vi "MAIN TASK TLB V1.vi"() -> ()   [LabVIEW 2018]
uses:
  TLB Type Definitions/Intruction Type Definitions.ctl
  TLB Type Definitions/State Type Definitions, for 0.26g versions and later 3.ctl
  <vilib>/Studica/Studica Toolkit/NavX/TypeDefs/Flags/Z900_navX_Flags_OpStatusTypeDef.ctl
  <vilib>/Studica/Studica Toolkit/NavX/TypeDefs/Flags/Z900_navX_Flags_CalibrationStatusTypeDef.ctl
  TLB Type Definitions/Vision cluster.ctl
  TLB Type Definitions/PING CLUSTER.ctl
  TLB Type Definitions/Encoder cluster.ctl
  TLB Type Definitions/Stepper cluster.ctl
  TLB Type Definitions/Yaw Cluster.ctl
  TLB Type Definitions/IR Sensor Type Def.ctl
  TLB Type Definitions/Line Sensor Cluster.ctl
  TLB Type Definitions/Time cluster.ctl
  TLB Type Definitions/Box Colour Detection Cluster (0.26d and above).ctl
  Underlying VI's/FGV's/Box FGV/Box Colour FGV Colours.ctl
  <vilib>/Studica/Studica Toolkit/Background/DIO Channel.ctl
  TLB Type Definitions/Y Stepper cluster.ctl
  TLB Type Definitions/Motor Speed Cluster.ctl
  <vilib>/Studica/Studica Toolkit/Background/PWM Channel.ctl
  Underlying VI's/NavX VI/navX type def.ctl
  <vilib>/Studica/Studica Toolkit/Background/I2C Channel.ctl
  Underlying VI's/I2C Master VI/Arduino_Interfacing.ctl
  Labview Training Phase 2/Enum Controls/States for Action Engine.ctl
  Underlying VI's/Motor Control VI with PID/MOTOR CONTROL WITH PID AE DATA MODE TYPE DEF.ctl
  Underlying VI's/Motor Control VI with PID/MOTOR CONTROL WITH PID AE DIRECTION TYPE DEF.ctl
  Experimental VI's/Archived VI's/MOTOR CONTROL NO PID Type Def.ctl
  <vilib>/myRIO/Common/Instrument Driver Framework/myRIO v1.0/AI/typedefs/AI Channels List.ctl
  <vilib>/myRIO/Common/Instrument Driver Framework/myRIO v1.0/AI/typedefs/AI Channels Enum.ctl
  Underlying VI's/Line Sensor AE/Line Sensor AE Type Def.ctl
  Underlying VI's/I2C Master VI/I2C MASTER Type Def.ctl
  Underlying VI's/Elasped Timer/Elapsed timer control.ctl
  Underlying VI's/IMAQ Create Reference AE/IMAQ Reference AE.ctl
  Underlying VI's/FGV's/Box FGV/Box Colour FGV States.ctl
  Underlying VI's/I2C Master VI/I2C_MASTER_WRITE_NEW Type Def.ctl
  Underlying VI's/FGV's/Servo State FGV/Servo States FGV Enum.ctl
  Underlying VI's/Modified webcam FGV/Webcam AE.ctl
  <vilib>/userdefined/High Color/IMAQdx.ctl
  <vilib>/Studica/Studica Toolkit/NavX/NavX.lvlib
panel:
  out "Same colour?":bool
  out "Distance to move":dbl
  out "Box Colour Detection":T1
  out "Errors detected":bool
  out "Robot ready":bool
  out "Time cluster":T3
  out "Table IR obstruct":bool
  out "Front IR obstruct":bool
  out "Line sensors":T4
  out "IR Sensors":T5
  out "NAVX Values":T6
  out "Stepper position values":T7
  out "Encoder values":T8
  out "Ultrasonic sensors":T9
  out "Selected Task":T10=enum."Start Task 9"
  out "Object recognition mode":enum16{"Ball", "Soap", "Gel", "Pipe", "None"}(ring)
  out "Image Processing Error":errorcluster
  out "Object Detection":T11
  out "Status":T14 {"OP Status" items=["INITIALIZING", "SELFTEST_IN_PROGRESS", "ERROR", "IMU_AUTOCAL_IN_PROGRESS", "NORMAL"]; "Calibration Status" items=["IMU_CAL_STATE_MASK"=3, "IMU_CAL_STATE_INPROGRESS"=0, "IMU_CAL_STATE_ACCUMULATE"=1, "IMU_CAL_STATE_COMPLETE"=2]}
  out "General Errors":errorcluster
  in  "Red LED":bool
  out "Front Ultrasonic obstruct":bool
  out "Speed & distance":T15
  out "Task selection":u8
  out "NavX Readings":T16
  out "Arduino Data":T17
  out "TASK ENABLE":bool
  out "Rising Edge":bool
  in  "Green LED":bool
  out "State Logic":T18=enum."Startup"
  out "elements":T10[](array[typedef])
  in  "STOP TASK":bool
  in  "OK Button":bool
  in  "STOP":bool
  out "Queue Errors":errorcluster
  out "Action Queue Items":i32
  out "State Logic Queue Items":i32
  out "Action Queues items":string[](array[string])=["Hardware reset", "Software reset", ""]
  out "Action State":string
  # "TLB FRAMEWORK STATUS"
  # "System Health Status Update"
  # "Test Programme written by Calvin Loke    Dated: 28 Aug 2019\nTest Programme revised by Dr Alex See   Dated 30 Aug 2019\n\nRevision date: 20/03/2020\nProgramme version:   TLB Native Dynamic Events ver 0.19a"
  # "0: Task 1\n1: Task 2\n2: Task 3\n3: Task 4\n4: Task 5\n5: Task 6\n6: Task 7\n7: Task 8 Ball\n8: Task 8 Soap\n9: Task 8 Gel\n10: Task 8 Pipe\n11: Task 9 Blue\n12: Task 9 Black\n13: Task 9 Green\n14: Task 9 Red\n15: Task 9 Yellow"
  # "Ball: Right\nSoap: Left\nGel: Reverse\nPipe: Forward"
  # "VISION"
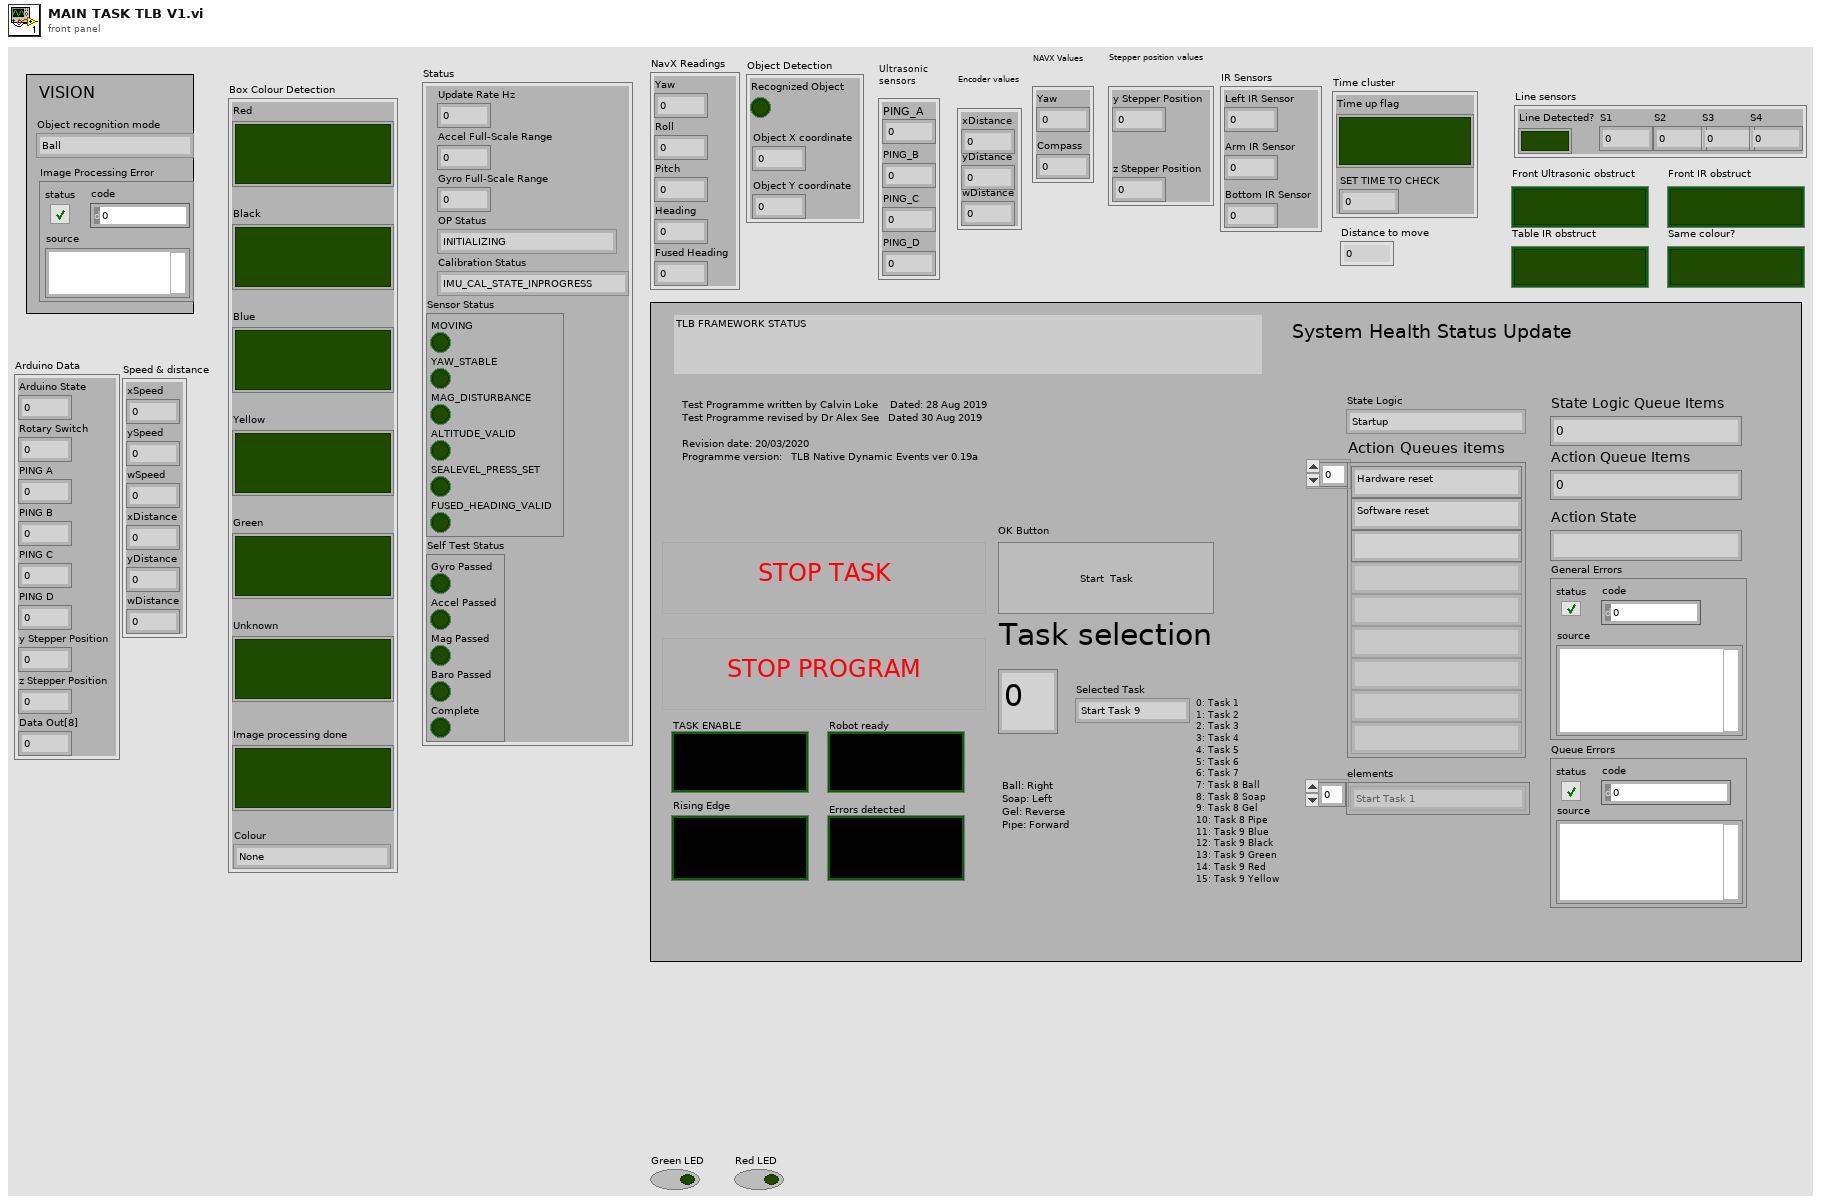
[diagram p1: front panel]
types:
  T1 = typedef "Box Colour Detection Cluster (0.26d and above).ctl" = cluster{"Red":bool, "Black":bool, "Blue":bool, "Yellow":bool, "Green":bool, "Unknown":bool, "Image processing done":bool, "Colour":T2}
  T2 = typedef "Box Colour FGV Colours.ctl" = enum16{"None", "Black", "Blue", "Green", "Red", "Yellow"}
  T3 = typedef "Time cluster.ctl" = cluster{"Time up flag":bool, "SET TIME TO CHECK":dbl}
  T4 = typedef "Line Sensor Cluster.ctl" = cluster{"Line Detected?":bool, "S1":dbl, "S2":dbl, "S3":dbl, "S4":dbl}
  T5 = typedef "IR Sensor Type Def.ctl" = cluster{"Left IR Sensor":dbl, "Arm IR Sensor":dbl, "Bottom IR Sensor":dbl}
  T6 = typedef "Yaw Cluster.ctl" = cluster{"Yaw":dbl, "Compass":dbl}
  T7 = typedef "Stepper cluster.ctl" = cluster{"y Stepper Position":u8, "z Stepper Position":u8}
  T8 = typedef "Encoder cluster.ctl" = cluster{"xDistance":dbl, "yDistance":dbl, "wDistance":dbl}
  T9 = typedef "PING CLUSTER.ctl" = cluster{"PING_A":u8, "PING_B":u8, "PING_C":u8, "PING_D":u8}
  T10 = typedef "Intruction Type Definitions.ctl" = enum16{"None", "Start Task 1", "Start Task 2", "Start Task 3", "Start Task 4", "Start Task 5", "Start Task 6", "Start Task 7", "Start Task 8 - BALL", "Start Task 8 - Gel", "Start Task 8 - Pipe", "Start Task 8 - Soap", "Start Task 9", "Start Task A", "Start Task B", "Exit"}
  T11 = typedef "Vision cluster.ctl" = cluster{"Recognized Object":bool, "Object X coordinate":dbl, "Object Y coordinate":dbl}
  T12 = typedef "NavX.lvlib/Z900_navX_Flags_OpStatusTypeDef.ctl" = u8
  T13 = typedef "NavX.lvlib/Z900_navX_Flags_CalibrationStatusTypeDef.ctl" = u8
  T14 = cluster{"Update Rate Hz":u8, "Accel Full-Scale Range":u8, "Gyro Full-Scale Range":u16, "OP Status":T12, "Calibration Status":T13, "Sensor Status":cluster{"MOVING":bool, "YAW_STABLE":bool, "MAG_DISTURBANCE":bool, "ALTITUDE_VALID":bool, "SEALEVEL_PRESS_SET":bool, "FUSED_HEADING_VALID":bool}, "Self Test Status":cluster{"Gyro Passed":bool, "Accel Passed":bool, "Mag Passed":bool, "Baro Passed":bool, "Complete":bool}}
  T15 = cluster{"xSpeed":dbl, "ySpeed":dbl, "wSpeed":dbl, "xDistance":dbl, "yDistance":dbl, "wDistance":dbl}
  T16 = cluster{"Yaw":dbl, "Roll":dbl, "Pitch":dbl, "Heading":dbl, "Fused Heading":dbl}
  T17 = cluster{"Arduino State":u8, "Rotary Switch":u8, "PING A":u8, "PING B":u8, "PING C":u8, "PING D":u8, "y Stepper Position":u8, "z Stepper Position":u8, "Data Out[8]":u8}
  T18 = typedef "State Type Definitions, for 0.26g versions and later 3.ctl" = enum16{"None", "Startup", "Move to Angle", "True Stop", "Idle", "Shutdown", "Task 1A", "Task 1B", "Task 2:Raise Arm", "Task 2:Sensor Mode", "Task 2:Reverse Mode", "Task 3: Rotate 360", "Task 4_A", "Task 4_B", "Task 4_C", "Task 4_D", "Task 5A: RAISING ARM", "Task 5B: STILL WAITING", "Task 5C: GOING DOWN", "Task 5D: GRAB", "Task 5E: GOING UP", "Task 5F: ARM GRAB HEIGHT", "Task 5G: CLOSE CLAW", "Task 5H: RAISE ARM", "Task 6A: RAISE ARM", "Task 6B: CAM BURST", "Task 6C: PROCESS IMAGE", "Task 6D: BALL BUSTER", "Task 6E: STILL WAITING", "Task 6F: CAM BURST 2", "Task 6G: PROCESS IMAGE 2", "Task 6H: SKADI SOAPS", "Task 6I: STILL WAITING 2", "Task 6J: CAM BURST 3", "Task 6K: PROCESS IMAGE 3", "Task 6L: JAM IT IN", "Task 6M: STILL WAITING 3", "Task 6N: CAM BURST 4", "Task 6O: PROCESS IMAGE 4", "Task 6P: PIPE BOMB", "Task 7", "Task 8A: RAISE ARM", "Task 8B: MOVE TO BOX", "Task 8C: CAM BURST", "Task 8D: PROCESS IMAGE", "Task 8E: ROBOT ADJUST", "Task 8F: CAM BURST 2", "Task 8G: PROCESS IMAGE 2", "Task 8H: ARM ADJUST", "Task 8I: ARM GRAB HEIGHT", "Task 8J: CLOSE CLAW", "Task 8K: RAISE MY SWORD", "Task 8I: STILL WAITING", "Task 8L: Return to position", "Task 9A: Raise Arm", "Task 9B: Rotate to Angle", "Task 9C: Detect Box", "Task 9D: MOVE FORWARD", "Task 9D2: ANGLE CORRECTION", "Task 9E: MOVE LEFT", "Task 9E2: MOVE RIGHT", "Task 9F: SCAN BOX", "Task 9G: MOVE RIGHT", "Task 9H: SCAN BOX 2", "Task 9I: ROTATE 90 CW", "Task 9J: FORWARD", "Task 9J2: ANGLE CORRECTION", "Task 9K: RAM WALL", "Task 9L: MOVE RIGHT", "Task 9M: SCAN BOX 3", "Task 9N: MOVE RIGHT", "Task 9O: SCAN BOX 4", "Task A1: RAISE ARM", "Task A2: ROTATE TO ANGLE", "Task A3: MOVE TO BL BOX", "Task A4: MOVE FORWARD", "Task A5: Stop", "Task A6: ROTATE CW 90", "Task A7: FORWARD", "Task A8: LEFT UNTIL LINE", "Task A9: REVERSE", "Task A10: ROTATE TO ANGLE", "Task A11: ARM DROP HEIGHT", "Task A12: EXTEND ARM", "Task A12: DROP"}
  T19 = typedef "PWM Channel.ctl" = enum16{"Not Connected", "A/PWM0", "A/PWM1", "A/PWM2", "A/PWM3", "A/PWM4", "B/PWM0", "B/PWM1", "B/PWM2", "B/PWM3", "B/PWM4", "C/PWM0", "C/PWM1"}
  T20 = typedef "Motor Speed Cluster.ctl" = cluster{"ySpeed":dbl, "xSpeed":dbl, "wSpeed":dbl}
  T21 = typedef "Y Stepper cluster.ctl" = cluster{"yStepper desired":u8}
  T22 = typedef "DIO Channel.ctl" = enum16{"Not Connected", "A/DIO1", "A/DIO2", "A/DIO3", "A/DIO4", "A/DIO5", "A/DIO6", "A/DIO7", "A/DIO13", "B/DIO1", "B/DIO2", "B/DIO3", "B/DIO4", "B/DIO5", "B/DIO6", "B/DIO7", "B/DIO13", "C/DIO0", "C/DIO1", "C/DIO2", "C/DIO3", "C/DIO4", "C/DIO5", "C/DIO6", "C/DIO7"}
  T23 = cluster{"PWM Channel":T19, "FPGA VI Reference Out":refnum<k20>}
  T24 = cluster{"DIO Channel":T22, "FPGA VI Reference Out":refnum<k20>}
  T25 = typedef "States for Action Engine.ctl" = enum16{"Initialize", "Write", "Read"}
  T26 = typedef "MOTOR CONTROL WITH PID AE DATA MODE TYPE DEF.ctl" = enum16{"Init AE", "Write to AE", "Read from AE"}
  T27 = typedef "navX type def.ctl" = enum16{"Get i2C reference", "Read Values", "Zero Yaw"}
  T28 = typedef "Arduino_Interfacing.ctl" = enum16{"Initialize", "Write to Arduino", "Read From Arduino"}
  T29 = typedef "I2C Channel.ctl" = enum16{"Not Connected", "A", "B"}
  T30 = cluster{"I2C Ref Out":cluster{"I2C Channel":T29, "FPGA VI Reference Out":refnum<k20>}, "Connected":bool, "Slave Address (7-bit)":u8, "Registry":u8[]}
  T31 = typedef "Box Colour FGV States.ctl" = enum16{"Initialize", "Read", "Write"}
  T32 = typedef "MOTOR CONTROL WITH PID AE DIRECTION TYPE DEF.ctl" = enum16{"y-axis movement", "x-axis movement", "rotation", "stop", "reset encoders"}
  T33 = typedef "Line Sensor AE Type Def.ctl" = enum16{"INIT AE", "READ FROM LINE SENSORS"}
  T34 = typedef "IMAQ Reference AE.ctl" = enum16{"Initialize AE", "Get IMAQ Reference", "Dispose Processing Buffer"}
  T35 = typedef "Elapsed timer control.ctl" = enum16{"Start", "Pause", "Initialize"}
  T36 = typedef "I2C_MASTER_WRITE_NEW Type Def.ctl" = enum16{"Ultrasonic sensors", "Stepper origin", "zStepper 13.3k", "zStepper 13k", "zStepper 12k", "zStepper 11k", "zStepper 10k", "zStepper 9k", "zStepper 8k", "zStepper 7k", "zStepper 6k", "zStepper 5k", "zStepper 4k", "zStepper 3k", "zStepper 2k", "zStepper 1k", "zStepper 900", "zStepper 800", "zStepper 700", "zStepper 600", "zStepper 500", "zStepper 400", "zStepper 300", "zStepper 200", "zStepper 100", "zStepper 0", "yStepper control", "Open Claw", "Close Claw", "Soft Reset"}
  T37 = typedef "Servo States FGV Enum.ctl" = enum16{"Open Claw", "Close claw"}
  T38 = typedef "Webcam AE.ctl" = enum16{"Initialize Camera", "Open Camera", "Continuous Acquisition", "Close Camera", "Retrieve Image", "Dispose Camera Image Buffer"}
  T39 = typedef "IMAQdx.ctl" = refnum<k21>
  T40 = typedef "MOTOR CONTROL NO PID Type Def.ctl" = enum16{"Init", "Front Back", "Left Right", "Rotate", "Stop", "Latch"}
  T41 = typedef "AI Channels List.ctl" = T42[]
  T42 = typedef "AI Channels Enum.ctl" = enum16{"Not Connected", "AudioIn/Left", "AudioIn/Right", "C/AI0", "C/AI1", "A/AI0", "A/AI1", "A/AI2", "A/AI3", "A/AI4", "A/AI5", "A/AI6", "A/AI7", "B/AI0", "B/AI1", "B/AI2", "B/AI3", "B/AI4", "B/AI5", "B/AI6", "B/AI7", "AI/AI0", "AI/AI1", "AI/AI2", "AI/AI3", "A/AI0 (DIFF)", "A/AI1 (DIFF)", "A/AI2 (DIFF)", "A/AI3 (DIFF)", "B/AI0 (DIFF)", "B/AI1 (DIFF)", "B/AI2 (DIFF)", "B/AI3 (DIFF)"}
  T43 = cluster{"S1":dbl, "S2":dbl, "S3":dbl, "S4":dbl, "Array[4]":dbl, "Array[5]":dbl, "Array[6]":dbl, "Array[7]":dbl, "Array[8]":dbl}
  T44 = typedef "I2C MASTER Type Def.ctl" = enum16{"Last State", "Mode 0", "Mode 1", "Mode 2", "Mode 3", "Mode 4", "Mode 5", "Mode 6", "Mode 7", "Mode 8", "Mode 9", "Mode 10"}
  T45 = typedef "IMAQ Image.ctl" = refnum<image>
  T46 = cluster{"Number of Matches":i32, "Object detected?":bool}
  T47 = cluster{"Red":bool, "Black":bool, "Blue":bool, "Yellow":bool, "Green":bool, "No recognizable coolour":bool}
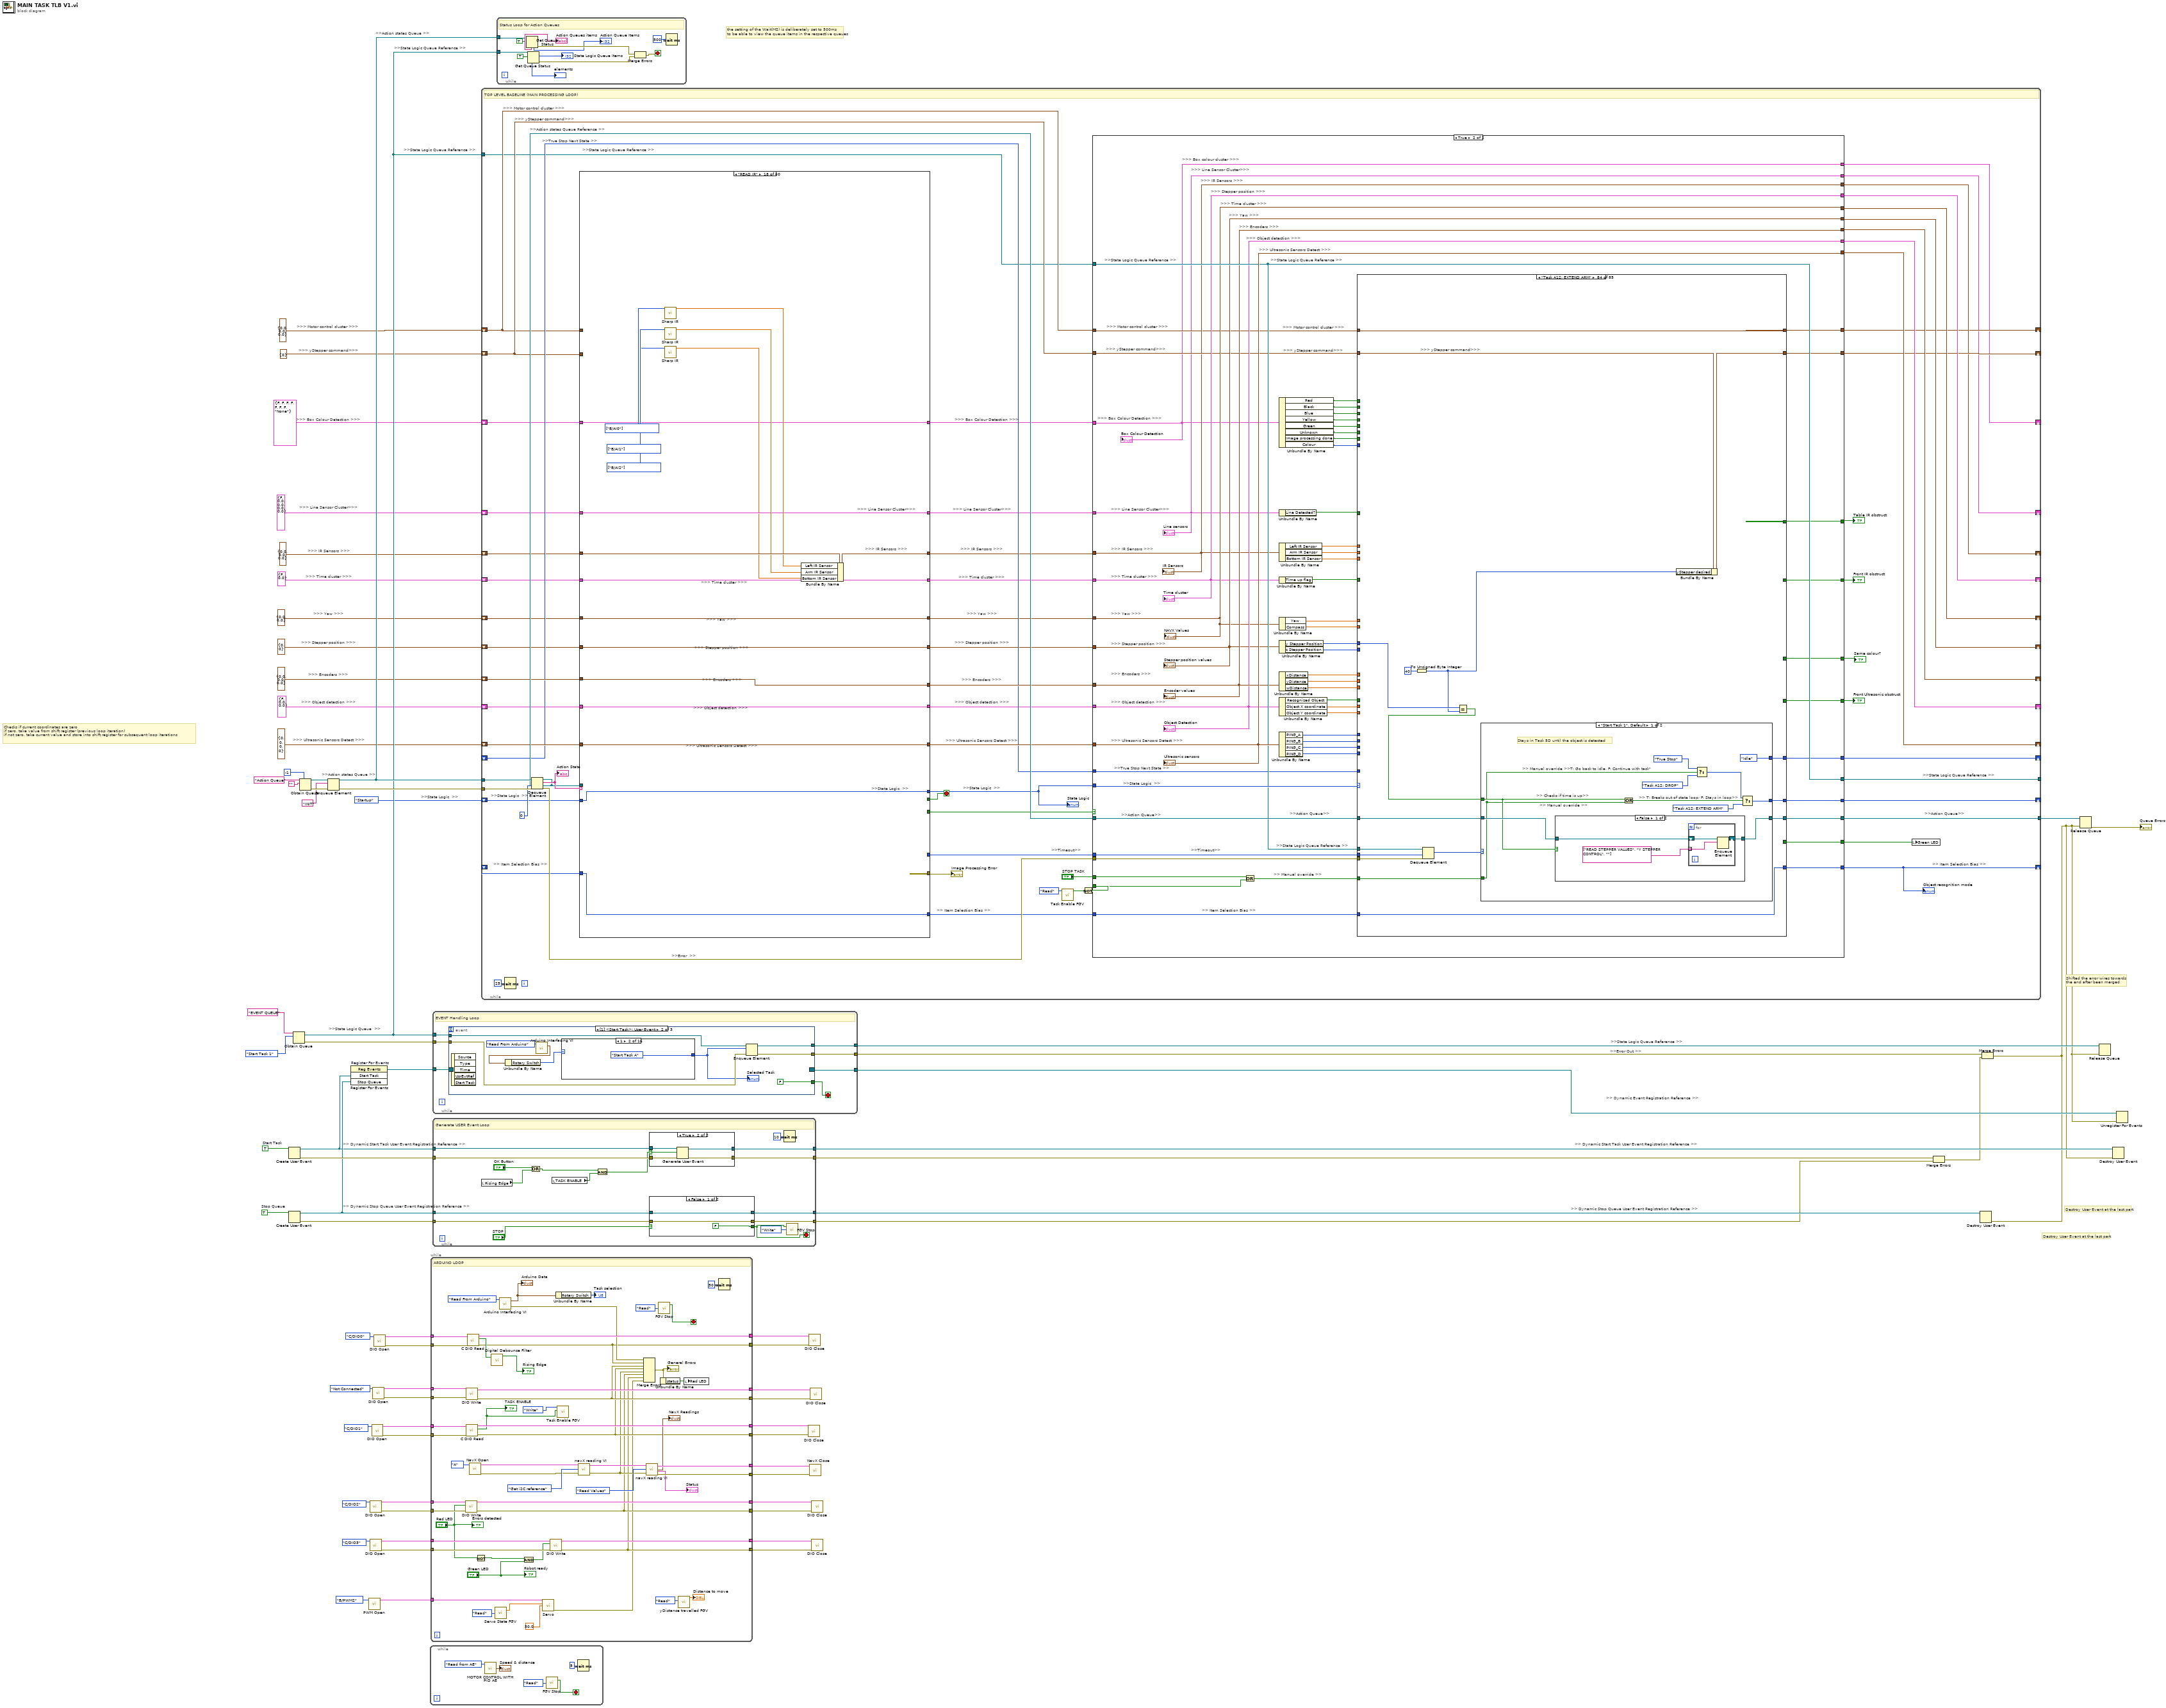
[diagram p0: block diagram]
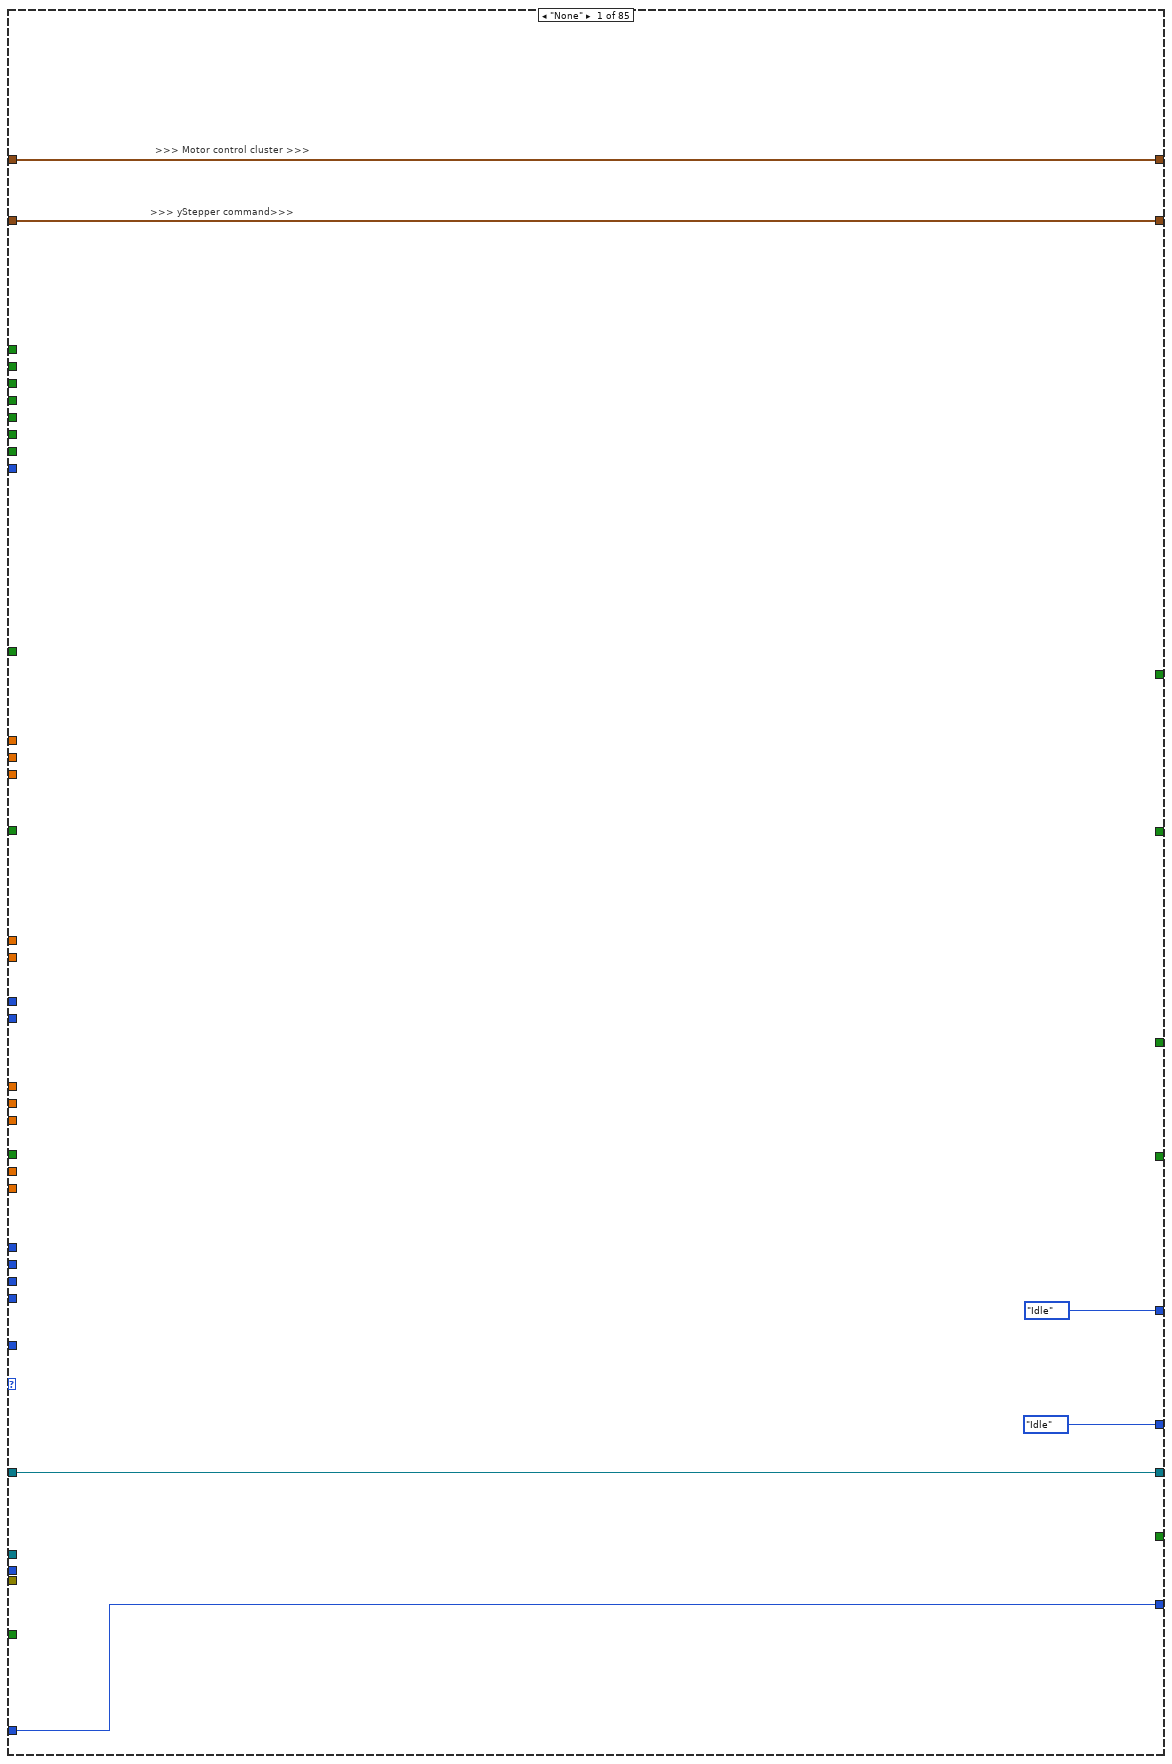
[diagram p3: hidden frame]
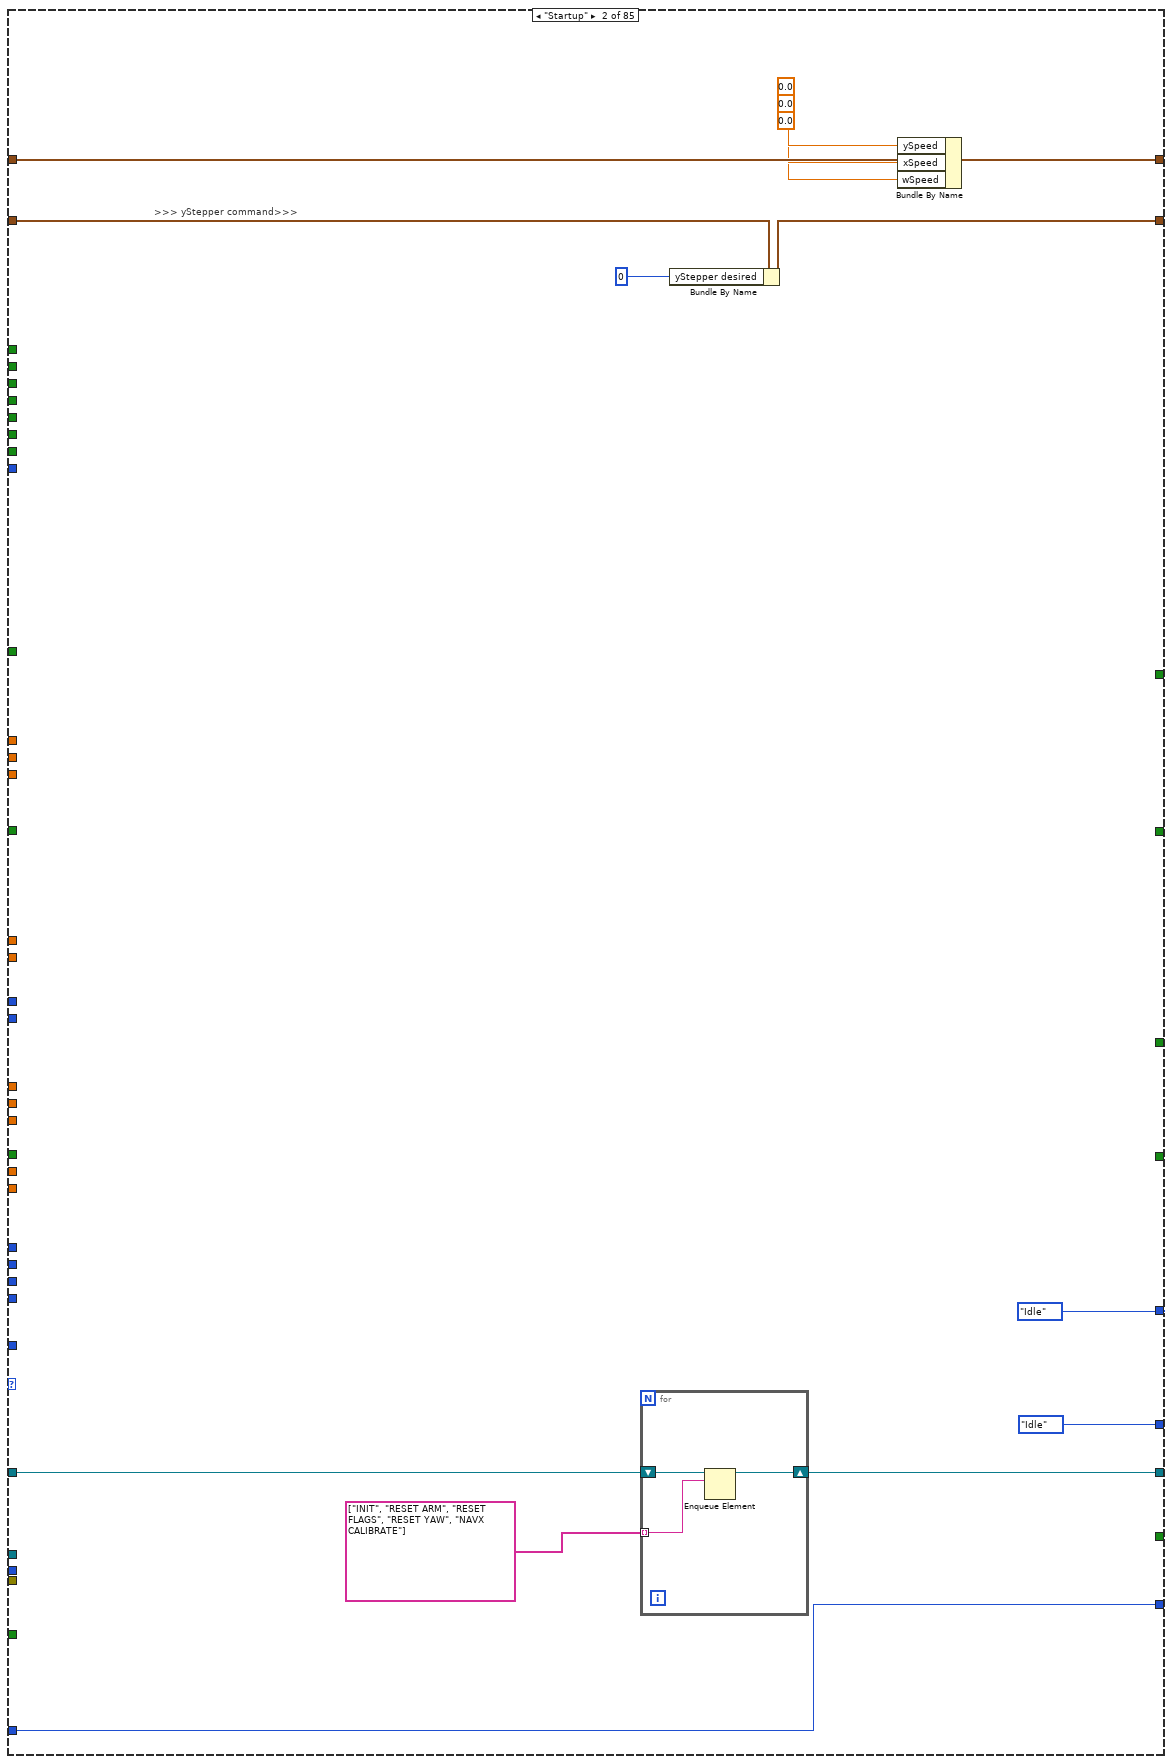
[diagram p4: hidden frame]
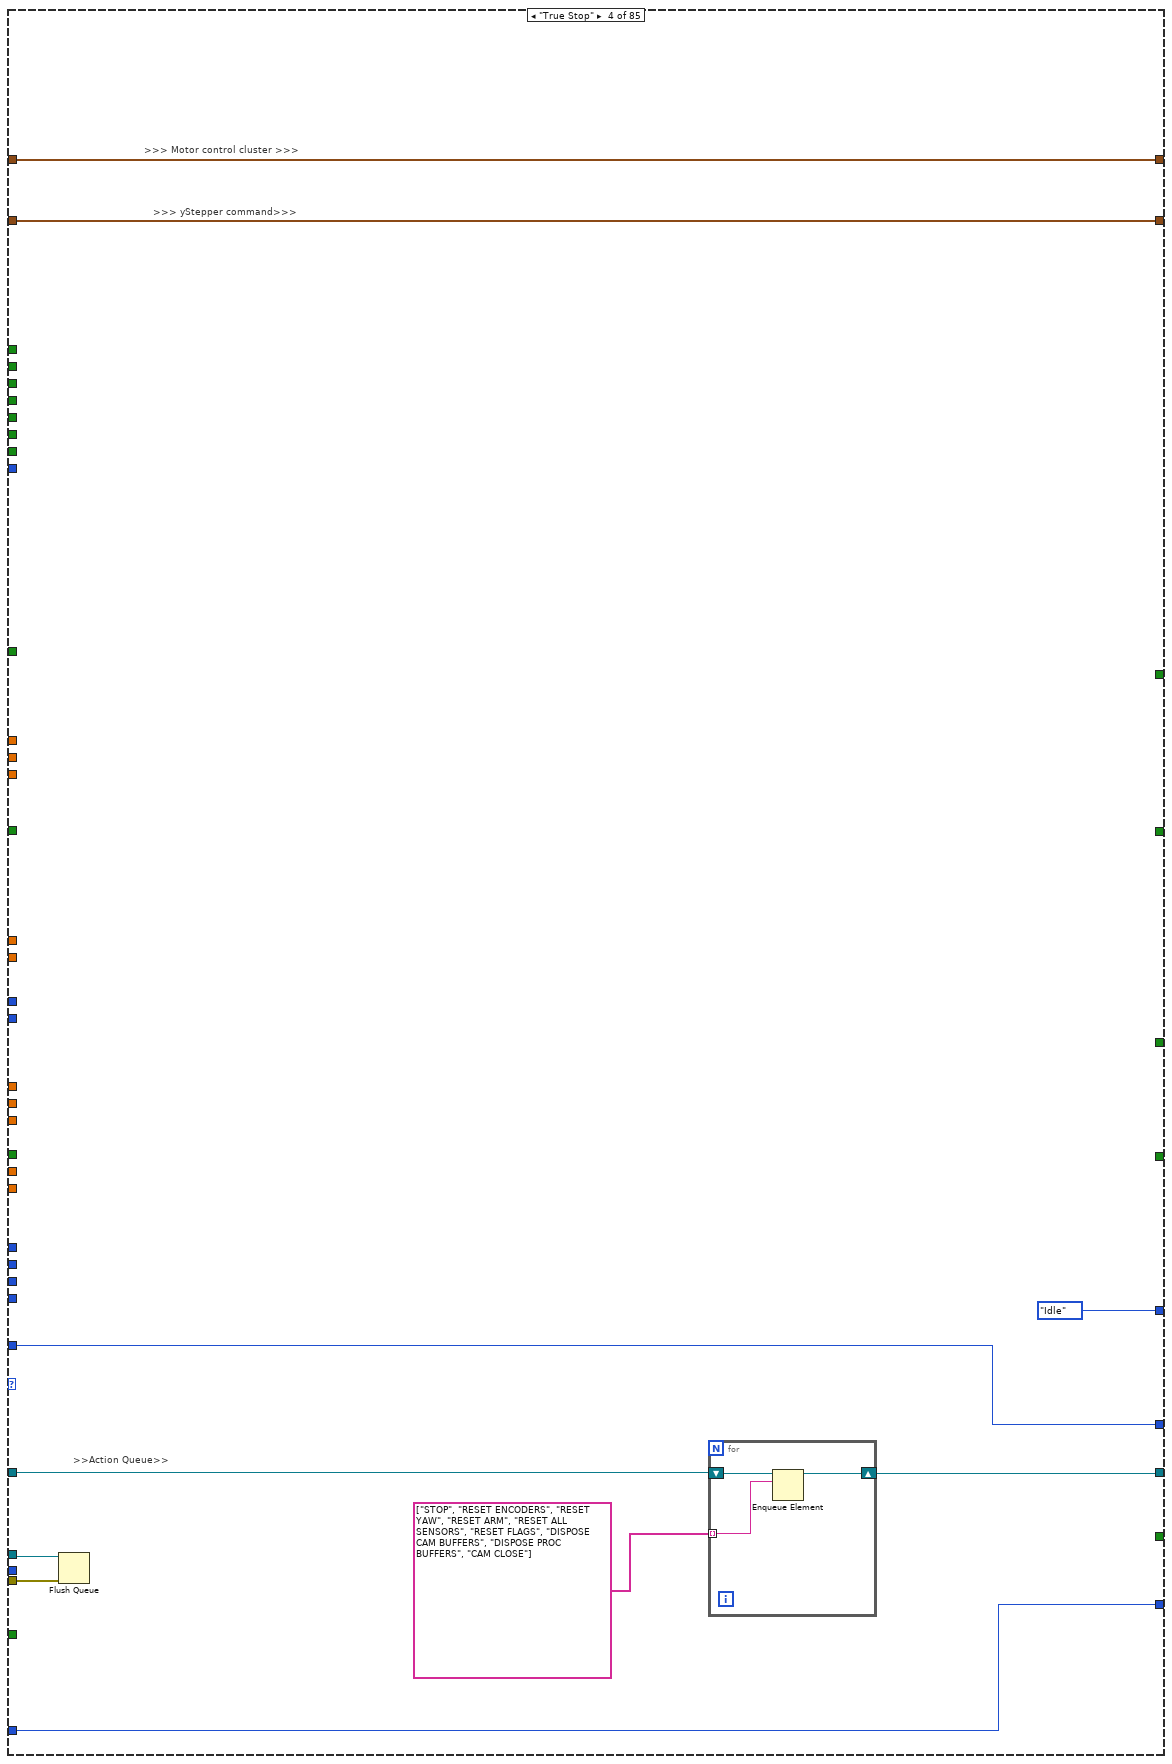
[diagram p6: hidden frame]
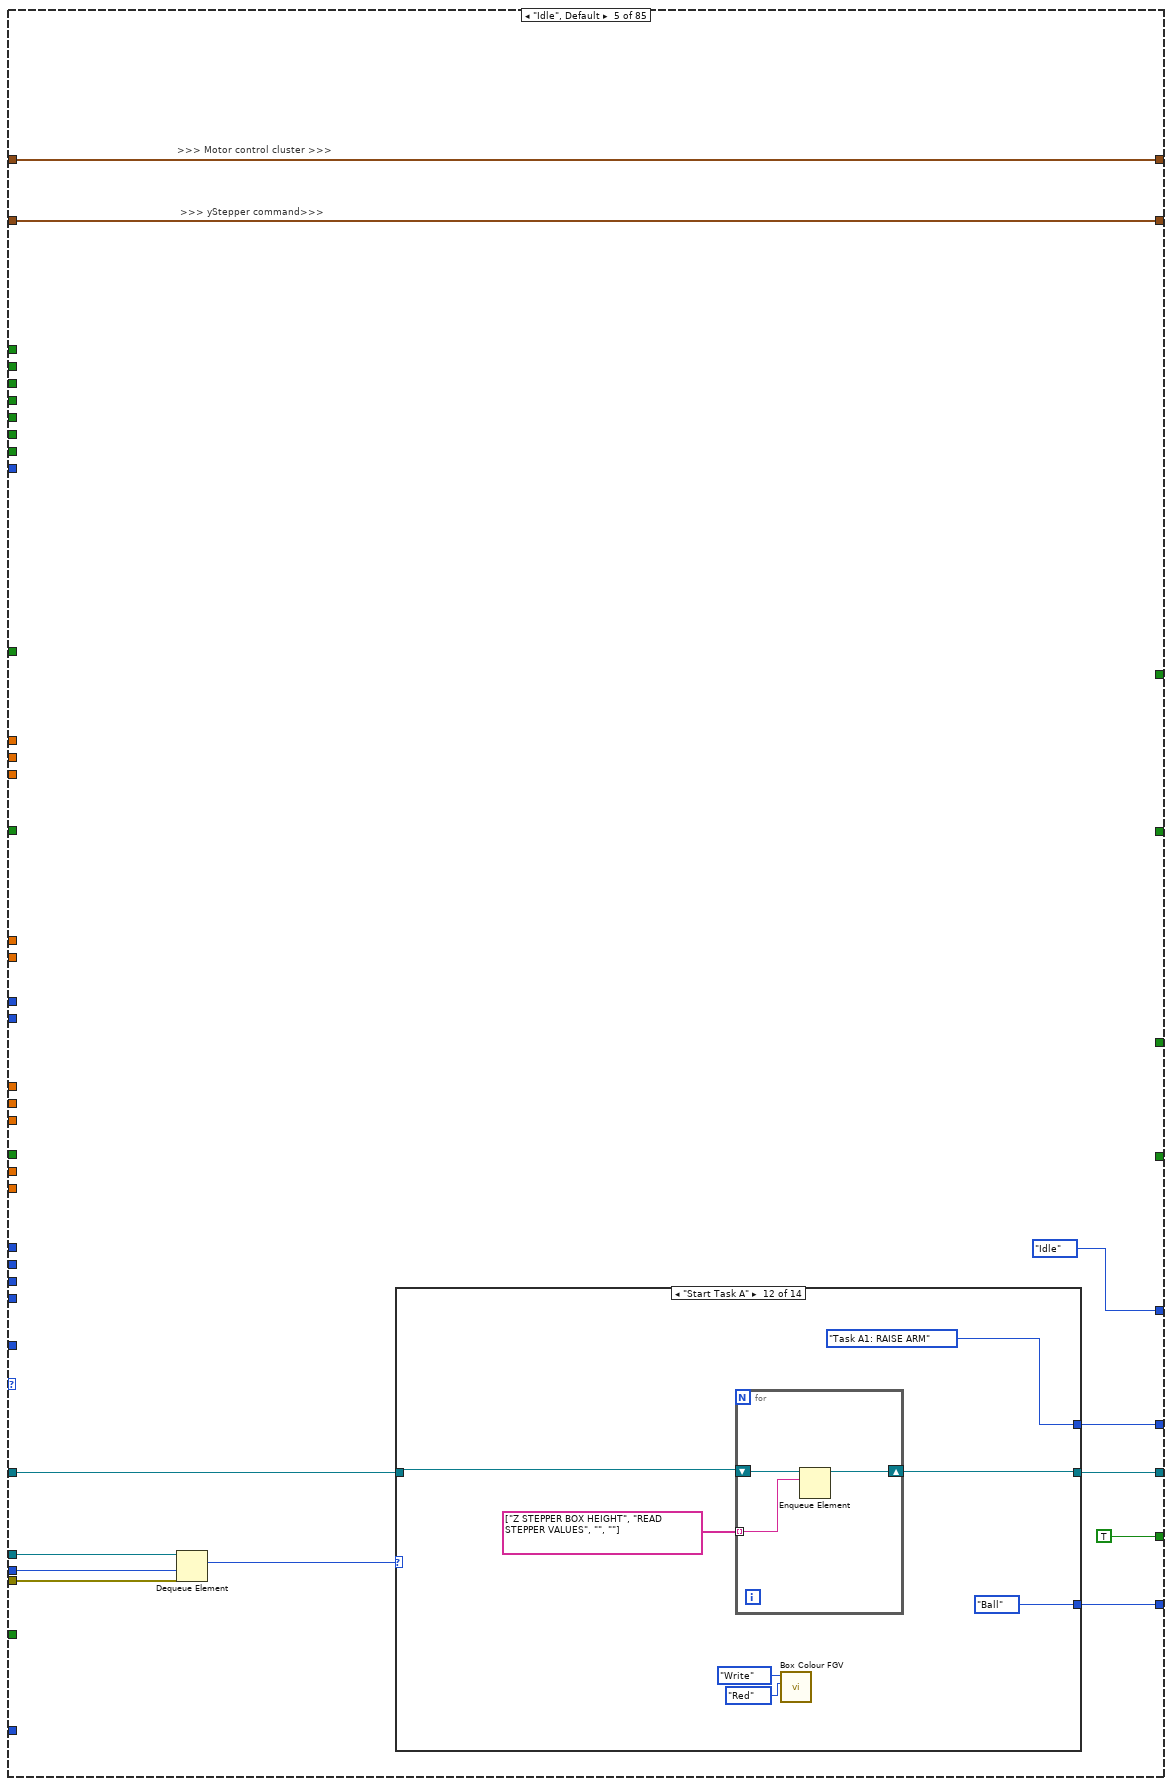
[diagram p7: hidden frame]
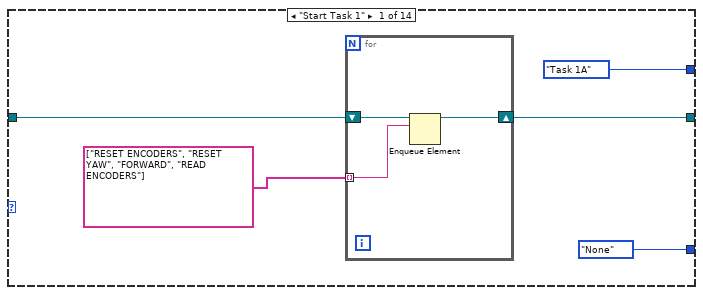
[diagram p8: hidden frame]
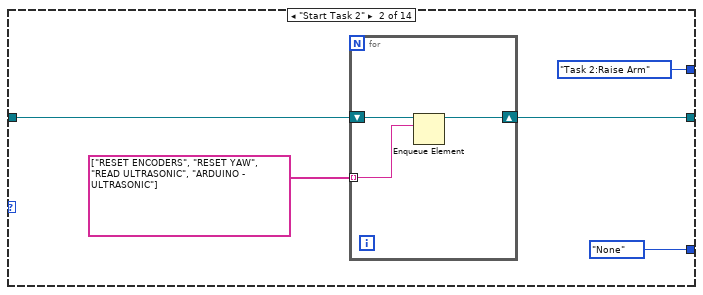
[diagram p9: hidden frame]
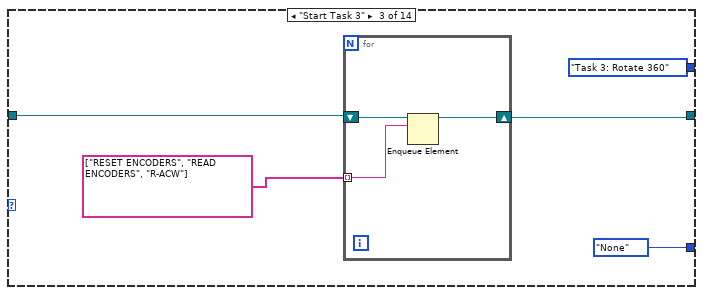
[diagram p10: hidden frame]
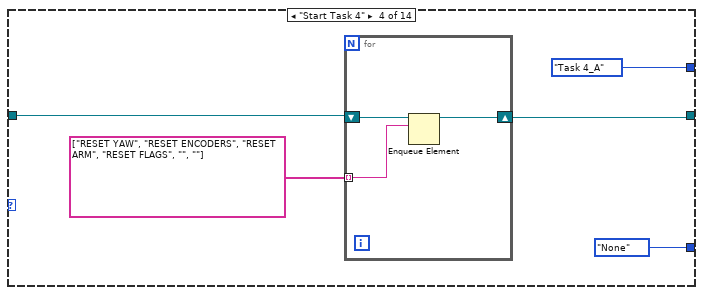
[diagram p11: hidden frame]
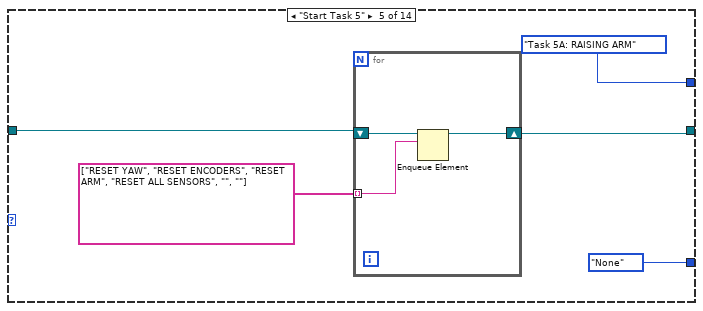
[diagram p12: hidden frame]
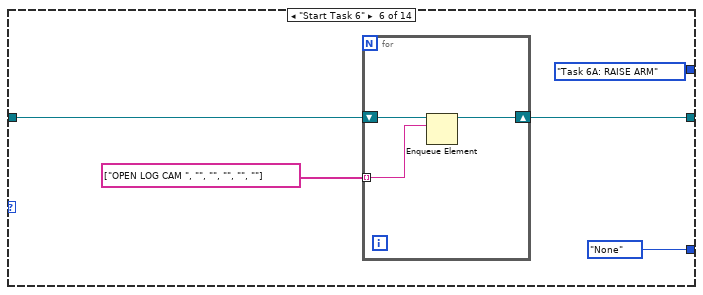
[diagram p13: hidden frame]
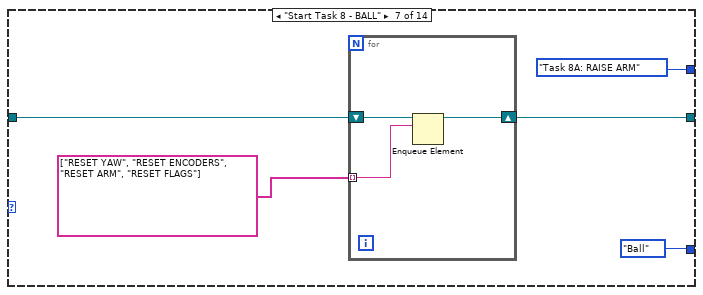
[diagram p14: hidden frame]
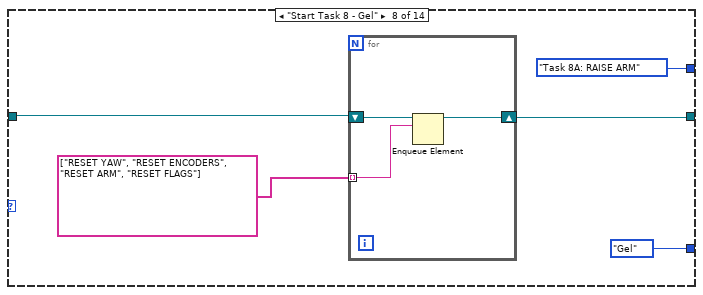
[diagram p15: hidden frame]
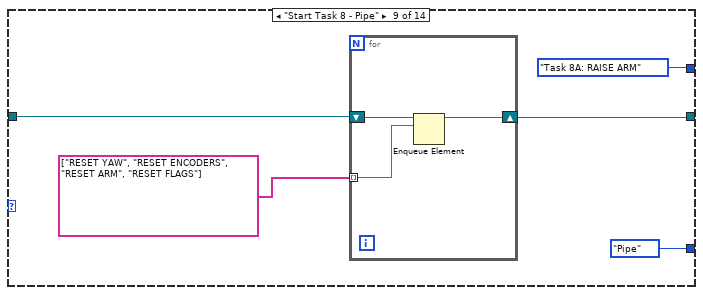
[diagram p16: hidden frame]
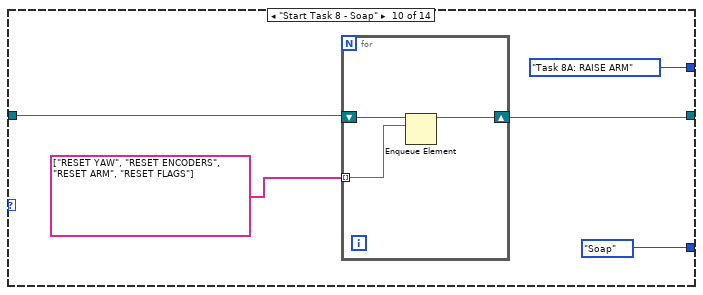
[diagram p17: hidden frame]
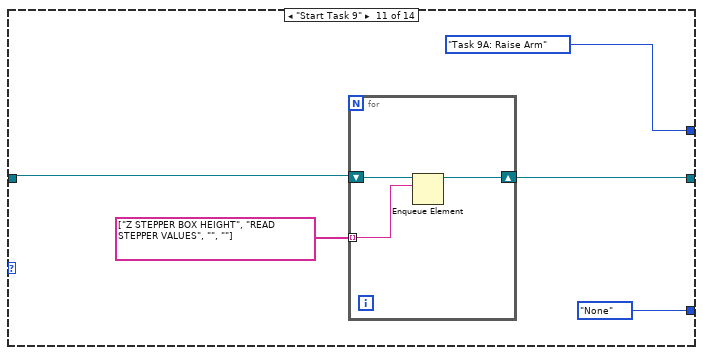
[diagram p18: hidden frame]
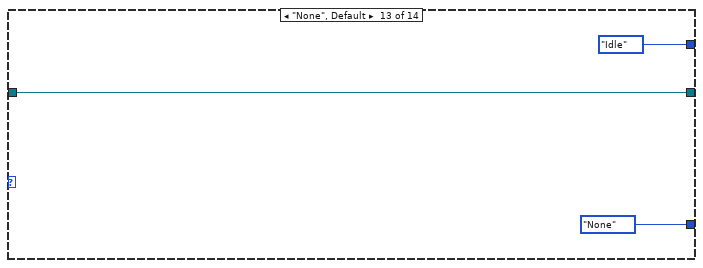
[diagram p19: hidden frame]
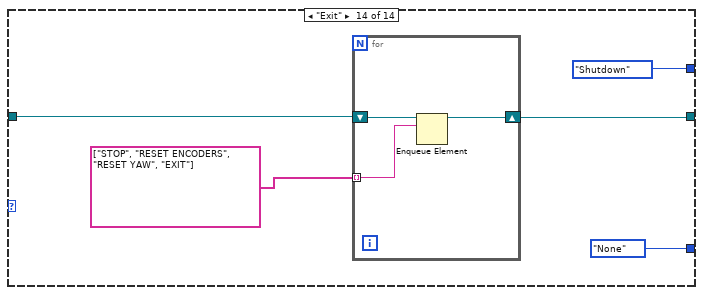
[diagram p20: hidden frame]
diagram:
  w71 = TRUE  # Stop Queue
  w70 = TRUE  # Start Task
  # ">>State Logic Queue Reference >>"
  # ">>Action states Queue >>"
  # ">>> Box Colour Detection >>>"
  # ">>State Logic Queue Reference >>"
  # ">>State Logic  >>"
  # ">>> Line Sensor Cluster>>>"
  # ">>> Motor control cluster >>>"
  # ">>> IR Sensors >>>"
  # "Checks if current coordinates are zero\nif zero, take value from shift register (previous loop iteration)\nif not zero, take current value and store into shift register for subsequent loop iterations"
  # ">>> yStepper command>>>"
  # ">>> Time cluster >>>"
  # ">>> Yaw >>>"
  # ">>> Stepper position >>>"
  # ">>> Encoders >>>"
  # ">>> Object detection >>>"
  # ">>> Ultrasonic Sensors Detect >>>"
  # "the setting of the Wait(MS) is deliberately set to 500ms\nto be able to view the queue items in the respective queues"
  # ">>Error Out >>"
  # ">> Dynamic Stop Queue User Event Registration Reference >>"
  # ">> Dynamic Start Task User Event Registration Reference >>"
  # ">> Dynamic Stop Queue User Event Registration Reference >>"
  # ">> Dynamic Start Task User Event Registration Reference >>"
  # ">> Dynamic Event Registration Reference >>"
  # ">>Action states Queue >>"
  # ">>State Logic Queue  >>"
  # ">>State Logic Queue Reference >>"
  # "Destroy User Event at the last part"
  # "Destroy User Event at the last part"
  # "Shifted the error wires towards\nthe end after been merged"
  n1 = Create User Event(user event datatype=w70) -> (user event=w62:refnum<user-event>, error out=w67:errorcluster)  [unwired: 1 in]
  n2 = Create User Event(user event datatype=w71) -> (user event=w63:refnum<user-event>, error out=w66:errorcluster)  [unwired: 1 in]
  n3 = Obtain Queue(name (unnamed)="EVENT QUEUE", element data type=Intruction_Type_Definitions."Start Task 1" ("Enum")) -> (queue out=w48:refnum<queue>, error out=w54:errorcluster)  [unwired: 3 in, 1 out]
  n4 = Obtain Queue(max queue size (-1, unlimited)=-1, name (unnamed)="Action Queue", element data type="") -> (queue out=w57:refnum<queue>, error out=w53:errorcluster)  [unwired: 2 in, 1 out]
  n5 = Enqueue Element(queue=w57, element="INIT", error in (no error)=w53) -> (queue out=w49:refnum<queue>, error out=w52:errorcluster)  [unwired: 1 in, 1 out]
  n6 = register-events "Register For Events"(w62, w63) -> (reference out=w61:refnum<event-registration>)  [unwired: 2 in, 1 out]
  n7 = call <vilib>:"PWM Open.vi"("PWM Channel"=PWM_Channel."B/PWM2") -> ("PWM Info Out"=w1:T23)  [unwired: 9 in, 1 out]
  n8 = call <vilib>:"DIO Open.vi"("DIO Channel"=DIO_Channel."C/DIO2") -> ("error out"=w21:errorcluster, "DIO Info Out"=w22:T24)  [unwired: 9 in]
  n9 = call <vilib>:"DIO Open.vi"("DIO Channel"=DIO_Channel."C/DIO3") -> ("error out"=w16:errorcluster, "DIO Info Out"=w17:T24)  [unwired: 9 in]
  n10 = call <vilib>:"DIO Open.vi"("DIO Channel"=DIO_Channel."C/DIO1") -> ("error out"=w26:errorcluster, "DIO Info Out"=w27:T24)  [unwired: 9 in]
  n11 = call <vilib>:"DIO Open.vi"("DIO Channel"=DIO_Channel."Not Connected") -> ("error out"=w31:errorcluster, "DIO Info Out"=w33:T24)  [unwired: 9 in]
  n12 = call <vilib>:"DIO Open.vi"("DIO Channel"=DIO_Channel."C/DIO0") -> ("error out"=w36:errorcluster, "DIO Info Out"=w39:T24)  [unwired: 9 in]
  n13 = while {
    stop <- w73 stop-if-true
    n14 = call "MOTOR CONTROL WITH PID AE.vi"("AE Mode"=MOTOR_CONTROL_WITH_PID_AE_DATA_MODE_TYPE_DEF."Read from AE") -> ("Speed & distance"=→"Speed & distance":T15)  [unwired: 3 in]
    n15 = call "FGV Stop.vi"("Init/Read/Write State"=States_for_Action_Engine."Read") -> ("Output node"=w73:bool)  [unwired: 2 in, 1 out]
    n16 = Wait (ms)(milliseconds to wait=u32 5) -> ()  [unwired: 1 out]
  }
  n17 = while {
    tunnel: w39 -> [w128]
    tunnel: [w127] -> w37
    tunnel: w36 -> [w126]
    tunnel: [w98] -> w35
    tunnel: w33 -> [w123]
    tunnel: [w122] -> w32
    tunnel: w31 -> [w121]
    tunnel: [w97] -> w30
    tunnel: [w120] -> w28
    tunnel: w27 -> [w119]
    tunnel: w26 -> [w118]
    tunnel: [w96] -> w25
    tunnel: w22 -> [w113]
    tunnel: w21 -> [w112]
    tunnel: [w111] -> w20
    tunnel: [w94] -> w19
    tunnel: w17 -> [w110]
    tunnel: w16 -> [w109]
    tunnel: [w108] -> w15
    tunnel: [w93] -> w14
    tunnel: [w105] -> w11
    tunnel: [w104] -> w12
    tunnel: w1 -> [w85]
    stop <- w130 stop-if-true
    # "ARDUINO LOOP"
    n18 = call <vilib>:"DIO Write.vi"("error in (no error)"=w112, "Input"="Red LED", "DIO Info In"=w113) -> ("error out"=w94:errorcluster, "DIO Info Out"=w111:T24)  [unwired: 7 in]
    n19 = call <vilib>:"DIO Write.vi"("error in (no error)"=w121, "DIO Info In"=w123) -> ("error out"=w97:errorcluster, "DIO Info Out"=w122:T24)  [unwired: 8 in]
    n20 = call <vilib>:"C DIO Read.vi"("error in (no error)"=w118, "DIO Info In in"=w119) -> ("error out"=w96:errorcluster, "IN"=w77:bool, "DIO Info In out"=w120:T24)  [unwired: 7 in]
    "TASK ENABLE" <- w77
    n21 = call <vilib>:"C DIO Read.vi"("error in (no error)"=w126, "DIO Info In in"=w128) -> ("error out"=w98:errorcluster, "IN"=w125:bool, "DIO Info In out"=w127:T24)  [unwired: 7 in]
    n22 = call <vilib>:"NavX Open.vi"("I2C Channel"=I2C_Channel."A") -> ("error out"=w115:errorcluster, "NavX Info"=w117:T30)  [unwired: 9 in]
    n23 = Not(x="Red LED") -> (.not. x?=w88:bool)
    n24 = call "Digital Debounce Filter.vi"("Boolean input"=w125) -> ("Rising Edge"=→"Rising Edge":bool)  [unwired: 1 in, 2 out]
    n25 = call "Servo State FGV.vi"("Init/Read/Write State"=States_for_Action_Engine."Read") -> ("Output"=w81:dbl)  [unwired: 2 in, 1 out]
    n26 = call "Arduino Interfacing VI.vi"("AE Mode"=Arduino_Interfacing."Read From Arduino") -> ("error out"=w99:errorcluster, "Arduino Data"=w101:T17)  [unwired: 3 in]
    "Arduino Data" <- w101
    n27 = And(x=w88, y="Green LED") -> (x .and. y?=w90:bool)
    n28 = call <vilib>:"Servo.vi"("PWM Info In"=w85, "Position"=w81, "Frequency [Hz]"=50.0) -> ("error out"=w84:errorcluster)  [unwired: 11 in, 1 out]
    n29 = call <vilib>:"DIO Write.vi"("error in (no error)"=w109, "Input"=w90, "DIO Info In"=w110) -> ("error out"=w93:errorcluster, "DIO Info Out"=w108:T24)  [unwired: 7 in]
    n30 = Unbundle By Name(w101) -> ("Rotary Switch"=→"Task selection":u8)
    n31 = call "Task Enable FGV.vi"("Task Enable Input"=w77, "Init/Read/Write State"=States_for_Action_Engine."Write") -> ()  [unwired: 8 in, 2 out]
    n32 = call "navX reading VI.vi"("NavX Info In"=w117, "Mode"=navX_type_def."Get i2C reference", "error in (no error)"=w115) -> ("NavX Info Out"=w106:T30, "Error Out"=w95:errorcluster)  [unwired: 2 out]
    n33 = Merge Errors(w99, w98, w97, w96, w95, w94, w93, w84) -> (w91:errorcluster)
    "General Errors" <- w91
    n34 = call "navX reading VI.vi"("NavX Info In"=w106, "Mode"=navX_type_def."Read Values", "error in (no error)"=w95) -> ("NavX Info Out"=w105:T30, "NavX Readings"=→"NavX Readings":T16, "Status"=→"Status":T14, "Error Out"=w104:errorcluster)
    n35 = call "FGV Stop.vi"("Init/Read/Write State"=States_for_Action_Engine."Read") -> ("Output node"=w130:bool)  [unwired: 2 in, 1 out]
    n36 = Unbundle By Name(w91) -> ("status"=w89:bool)
    n37 = call "yDistance travelled FGV.vi"("Init/Read/Write State"=States_for_Action_Engine."Read") -> ("Output"=→"Distance to move":dbl)  [unwired: 9 in, 1 out]
    n38 = local write "Red LED"(w89) -> ()
    n39 = Wait (ms)(milliseconds to wait=u32 50) -> ()  [unwired: 1 out]
    "Robot ready" <- "Green LED"
    "Errors detected" <- "Red LED"
  }
  n40 = while {
    tunnel: w62 -> [w148]
    tunnel: w63 -> [w147]
    tunnel: [w146] -> w69
    tunnel: [w145] -> w68
    tunnel: w67 -> [w144]
    tunnel: [w143] -> w65
    tunnel: w66 -> [w142]
    tunnel: [w141] -> w64
    stop <- w139 stop-if-true
    # "Generate USER Event Loop"
    n41 = local read "Rising Edge"() -> (w136:bool)
    n42 = Or(x="OK Button", y=w136) -> (x .or. y?=w135:bool)
    n43 = local read "TASK ENABLE"() -> (w134:bool)
    n44 = And(x=w135, y=w134) -> (x .and. y?=w133:bool)
    n45 = case shown="True" w133 {
      selector: w133 -> [_ w159]
      tunnel: w148 -> [w158 w163]
      tunnel: [w158 w162] -> w145
      tunnel: w144 -> [w157 w161]
      tunnel: [w157 w160] -> w143
      frame False {
      }
      frame True {
        n46 = Generate User Event(user event=w163, event data cluster=w159, error in=w161) -> (user event out=w162:refnum<user-event>, error out=w160:errorcluster)  [unwired: 1 in]
      }
    }
    n47 = case shown="False" "STOP" {
      selector: "STOP" -> [_ w152]
      tunnel: w147 -> [w151 w156]
      tunnel: [w151 w155] -> w146
      tunnel: w142 -> [w150 w154]
      tunnel: [w150 w153] -> w141
      tunnel: [FALSE w152] -> w139
      frame False {
      }
      frame True {
        n48 = Generate User Event(user event=w156, event data cluster=w152, error in=w154) -> (user event out=w155:refnum<user-event>, error out=w153:errorcluster)  [unwired: 1 in]
      }
    }
    n49 = Wait (ms)(milliseconds to wait=u32 10) -> ()  [unwired: 1 out]
    n50 = call "FGV Stop.vi"("Init/Read/Write State"=States_for_Action_Engine."Write", "Input Node"=w139) -> ()  [unwired: 1 in, 2 out]
  }
  n51 = while {
    tunnel: w61 -> [w170]
    tunnel: [w169] -> w60
    tunnel: w48 -> [w167]
    tunnel: [w166] -> w59
    tunnel: w54 -> [w165]
    tunnel: [w164] -> w51
    stop <- w168 stop-if-true
    # "EVENT Handling Loop"
    n52 = event shown="[1] <Start Task>: User Event" {
      selector: w170 -> [_ _ _]
      dyn-events: [_ _ _] -> w169
      timeout: _ -> [_ _ _]
      tunnel: [FALSE FALSE w217] -> w168
      tunnel: w167 -> [w175 w184 w215]
      tunnel: [w174 w183 w216] -> w166
      tunnel: w165 -> [w173 w182 w214]
      tunnel: [w172 w181 w213] -> w164
      event Timeout {
        n53 = event-data() -> ()  [unwired: 1 in, 3 out]
        n54 = Enqueue Element(queue=w175, element=Intruction_Type_Definitions."Start Task 1" ("Enum"), error in (no error)=w173) -> (queue out=w174:refnum<queue>, error out=w172:errorcluster)  [unwired: 1 in, 1 out]
      }
      event User Event {
        n55 = event-data() -> ()  [unwired: 1 in, 5 out]
        n56 = call "Arduino Interfacing VI.vi"("AE Mode"=Arduino_Interfacing."Read From Arduino") -> ("Arduino Data"=w178:T17)  [unwired: 3 in, 1 out]
        n57 = Unbundle By Name(w178) -> ("Rotary Switch"=w177:u8)
        n58 = case shown="1" w177 {
          tunnel: [Intruction_Type_Definitions."None" ("Enum") Intruction_Type_Definitions."Start Task A" ("Enum") Intruction_Type_Definitions."Start Task 3" ("Enum") Intruction_Type_Definitions."Start Task 4" ("Enum") Intruction_Type_Definitions."Start Task 5" ("Enum") Intruction_Type_Definitions."Start Task 6" ("Enum") Intruction_Type_Definitions."Start Task 7" ("Enum") Intruction_Type_Definitions."Start Task 8 - BALL" ("Enum") Intruction_Type_Definitions."Start Task 8 - Soap" ("Enum") Intruction_Type_Definitions."Start Task 8 - Gel" ("Enum") Intruction_Type_Definitions."Start Task 8 - Pipe" ("Enum") Intruction_Type_Definitions."Start Task 9" ("Enum") Intruction_Type_Definitions."Start Task 9" ("Enum") Intruction_Type_Definitions."Start Task 9" ("Enum") Intruction_Type_Definitions."Start Task 9" ("Enum") Intruction_Type_Definitions."Start Task 9" ("Enum")] -> w180
          frame 0, Default {
          }
          frame 1 {
          }
          frame 2 {
          }
          frame 3 {
          }
          frame 4 {
          }
          frame 5 {
          }
          frame 6 {
          }
          frame 7 {
          }
          frame 8 {
          }
          frame 9 {
          }
          frame 10 {
          }
          frame 11 {
            # "Task 9: Red Detection"
            n59 = call "Box Colour FGV.vi"("Colour to detect"=Box_Colour_FGV_Colours."Blue", "Init/R/W State"=Box_Colour_FGV_States."Write") -> ()  [unwired: 8 in, 2 out]
          }
          frame 12 {
            # "Task 9: Black Detection"
            n60 = call "Box Colour FGV.vi"("Colour to detect"=Box_Colour_FGV_Colours."Black", "Init/R/W State"=Box_Colour_FGV_States."Write") -> ()  [unwired: 8 in, 2 out]
          }
          frame 13 {
            # "Task 9: Blue Detection"
            n61 = call "Box Colour FGV.vi"("Colour to detect"=Box_Colour_FGV_Colours."Green", "Init/R/W State"=Box_Colour_FGV_States."Write") -> ()  [unwired: 8 in, 2 out]
          }
          frame 14 {
            # "Task 9: Yellow Detection"
            n62 = call "Box Colour FGV.vi"("Colour to detect"=Box_Colour_FGV_Colours."Red", "Init/R/W State"=Box_Colour_FGV_States."Write") -> ()  [unwired: 8 in, 2 out]
          }
          frame 15 {
            # "Task 9: Green Detection"
            n63 = call "Box Colour FGV.vi"("Colour to detect"=Box_Colour_FGV_Colours."Yellow", "Init/R/W State"=Box_Colour_FGV_States."Write") -> ()  [unwired: 8 in, 2 out]
          }
        }
        "Selected Task" <- w180
        n64 = Enqueue Element(queue=w184, element=w180, error in (no error)=w182) -> (queue out=w183:refnum<queue>, error out=w181:errorcluster)  [unwired: 1 in, 1 out]
      }
      event User Event {
        n65 = event-data() -> ("Stop Queue"=w217:bool)  [unwired: 1 in, 4 out]
        n66 = Enqueue Element At Opposite End(queue=w215, element=Intruction_Type_Definitions."Exit" ("Enum"), error in (no error)=w214) -> (queue out=w216:refnum<queue>, error out=w213:errorcluster)  [unwired: 1 in, 1 out]
      }
    }
  }
  n67 = while {
    tunnel: w48 -> [w222]
    tunnel: w49 -> [w279]
    tunnel: w52 -> [w277]
    tunnel: [w276] -> _
    tunnel: [w275] -> w42
    shift-right: [w268] -> _
    shift-left: T9 {"PING_A"=0, "PING_B"=0, "PING_C"=0, "PING_D"=0} -> [w270]
    shift-right: [w262] -> _
    shift-left: State_Type_Definitions,_for_0.26g_versions_and_later_3."Startup" ("Enum") -> [w265]
    shift-right: [w258] -> _
    shift-left: T8 {"xDistance"=0.0, "yDistance"=0.0, "wDistance"=0.0} -> [w260]
    shift-right: [w256] -> _
    shift-left: _ -> [w255]
    shift-right: [w252] -> _
    shift-left: T11 {"Recognized Object"=FALSE, "Object X coordinate"=0.0, "Object Y coordinate"=0.0} -> [w254]
    shift-right: [w249] -> _
    shift-left: T7 {"y Stepper Position"=0, "z Stepper Position"=0} -> [w251]
    shift-right: [w246] -> _
    shift-left: T6 {"Yaw"=0.0, "Compass"=0.0} -> [w248]
    shift-right: [w243] -> _
    shift-left: T3 {"Time up flag"=FALSE, "SET TIME TO CHECK"=0.0} -> [w245]
    shift-right: [w241] -> _
    shift-left: T21 {"yStepper desired"=0} -> [w242]
    shift-right: [w237] -> _
    shift-left: T5 {"Left IR Sensor"=0.0, "Arm IR Sensor"=0.0, "Bottom IR Sensor"=0.0} -> [w239]
    shift-right: [w235] -> _
    shift-left: T20 {"ySpeed"=0.0, "xSpeed"=0.0, "wSpeed"=0.0} -> [w236]
    shift-right: [w232] -> _
    shift-left: T4 {"Line Detected?"=FALSE, "S1"=0.0, "S2"=0.0, "S3"=0.0, "S4"=0.0} -> [w234]
    shift-right: [w230] -> _
    shift-left: _ -> [w229]
    shift-right: [w221] -> _
    shift-left: T1 {"Red"=FALSE, "Black"=FALSE, "Blue"=FALSE, "Yellow"=FALSE, "Green"=FALSE, "Unknown"=FALSE, "Image processing done"=FALSE, "Colour"=enum."None"} -> [w224]
    stop <- w267 stop-if-true
    # ">>> Box Colour Detection >>>"
    # ">>State Logic Queue Reference >>"
    # ">>Action Queue>>"
    # ">>State Logic Queue Reference >>"
    # ">>> Line Sensor Cluster>>>"
    # ">>> IR Sensors >>>"
    # ">>> Time cluster >>>"
    # ">>> Object detection >>>"
    # ">>> Yaw >>>"
    # ">>> Ultrasonic Sensors Detect >>>"
    # ">>> Encoders >>>"
    # ">>> Stepper position >>>"
    # ">>State Logic  >>"
    # ">> Item Selection Bias >>"
    # ">> Item Selection Bias >>"
    # ">> Item Selection Bias >>"
    # ">>State Logic  >>"
    # ">>> Motor control cluster >>>"
    # ">>> yStepper command>>>"
    # ">>True Stop Next State >>"
    # ">>Error  >>"
    # ">>Timeout>>"
    # ">>Action states Queue Reference >>"
    # "TOP LEVEL BASELINE (MAIN PROCESSING LOOP)"
    n68 = Wait (ms)(milliseconds to wait=u32 25) -> ()  [unwired: 1 out]
    n69 = Dequeue Element(queue=w279, timeout in ms (-1)=0, error in (no error)=w277) -> (queue out=w271:refnum<queue>, element=w278:string, error out=w272:errorcluster)  [unwired: 1 out]
    "Action State" <- w278
    n70 = case shown="\"READ IR\"" w278 {
      tunnel: [_ _ _ _ _ _ _ _ _ _ _ _ _ _ _ _ _ _ _ _ _ _ 0 w4514 _ _ _ _ _ _ _ _ _ _ _ _ _ _ _ _ _ _ _ _ _ _ _ _ _ _ _ _ _ _ _ _ _ _ _ _] -> w274
      tunnel: w271 -> [_ _ _ _ _ _ _ _ _ _ _ _ _ _ _ _ _ _ _ _ _ _ _ _ _ _ _ _ _ _ _ _ _ _ _ _ _ _ _ _ _ _ _ _ _ _ _ _ _ _ _ _ _ _ _ _ _ _ _ _]
      tunnel: w270 -> [w4155 w4167 w4182 w4196 w4216 w4231 w4245 w4259 w4273 w4287 w4303 w4318 w4332 w4342 w4360 w4377 w4392 w4407 w4431 w4441 w4475 w4488 w4502 w4515 w4527 w4540 w4560 w4595 w4632 w4646 w4659 w4671 w4684 w4699 w4715 w4727 w4739 w4759 w4782 w4793 w4809 w4840 w4850 w4863 w4876 w4889 w4899 w4917 w4930 w4940 w4959 w4968 w4984 w5000 w5016 w5032 w5048 w5062 w5077 w5097]
      tunnel: [w4155 w4167 w4182 w4196 w4216 w4231 w4245 w4259 w4273 w4287 w4303 w4318 w4332 w4342 w4360 w4378 w4392 w4407 w4431 w4441 w4476 w4488 w4502 w4515 w4527 w4540 w4560 w4594 w4631 w4646 w4659 w4671 w4684 w4699 w4715 w4727 w4739 w4759 w4782 w4793 w4809 w4840 w4850 w4863 w4876 w4889 w4899 w4917 w4930 w4940 w4959 w4968 w4984 w5000 w5016 w5032 w5048 w5062 w5077 w5097] -> w269
      tunnel: [TRUE TRUE _ _ _ _ _ _ _ _ _ _ _ _ _ _ _ _ _ _ _ _ _ _ _ _ _ _ _ _ _ _ _ _ _ _ _ _ _ _ _ _ _ _ _ _ _ _ _ _ _ _ _ _ _ _ _ _ _ _] -> w267
      tunnel: w265 -> [w4153 w4165 w4181 w4195 w4215 w4230 w4244 w4258 w4272 w4286 w4302 w4317 w4331 w4341 w4359 w4376 w4391 w4405 w4424 w4440 w4474 w4487 w4499 w4512 w4526 w4539 w4559 w4593 w4630 w4645 w4658 w4670 w4676 w4698 w4714 w4726 w4738 w4758 w4781 w4792 w4803 w4834 w4849 w4862 w4875 w4888 w4898 w4908 w4921 w4939 w4958 w4967 w4983 w4999 w5015 w5031 w5047 w5061 w5067 w5085]
      tunnel: [_ _ _ _ _ _ _ _ _ _ _ _ _ _ _ _ _ _ _ _ _ _ _ TRUE _ _ _ _ _ _ _ _ _ _ _ _ _ _ _ _ _ _ _ _ _ _ _ _ _ _ _ _ _ _ _ _ _ _ _ _] -> w264
      tunnel: [w4153 w4165 w4181 w4195 w4215 w4230 w4244 w4258 w4272 w4286 w4302 w4317 w4331 w4341 w4359 w4376 w4391 w4405 w4424 w4440 w4474 w4487 w4499 w4512 w4526 w4539 w4559 w4593 w4630 w4645 w4658 w4670 w4676 w4698 w4714 w4726 w4738 w4758 w4781 w4792 w4803 w4834 w4849 w4862 w4875 w4888 w4898 w4908 w4921 w4939 w4958 w4967 w4983 w4999 w5015 w5031 w5047 w5061 w5067 w5085] -> w263
      tunnel: w260 -> [w4152 w4164 w4180 w4198 w4214 w4229 w4243 w4257 w4271 w4285 w4301 w4316 w4330 w4343 w4358 w4375 w4393 w4409 w4426 w4442 w4473 w4489 w4498 w4511 w4528 w4541 w4555 w4584 w4620 w4644 w4661 w4672 w4681 w4700 w4716 w4728 w4740 w4760 w4783 w4795 w4807 w4838 w4852 w4865 w4878 w4891 w4901 w4912 w4925 w4942 w4961 w4970 w4986 w5002 w5018 w5034 w5050 w5064 w5069 w5090]
      tunnel: [w4152 w4164 w4180 w4198 w4214 w4229 w4243 w4257 w4271 w4285 w4301 w4316 w4330 w4343 w4357 w4375 w4393 w4409 w4426 w4442 w4472 w4489 w4498 w4511 w4528 w4541 w4555 w4583 w4619 w4644 w4661 w4672 w4681 w4700 w4716 w4728 w4740 w4760 w4783 w4795 w4807 w4838 w4852 w4865 w4878 w4891 w4901 w4912 w4925 w4942 w4961 w4970 w4986 w5002 w5018 w5034 w5050 w5064 w5069 w5090] -> w259
      tunnel: w254 -> [w4151 w4163 w4179 w4197 w4213 w4228 w4242 w4256 w4270 w4284 w4300 w4315 w4328 w4340 w4356 w4374 w4386 w4408 w4425 w4439 w4464 w4486 w4497 w4510 w4525 w4538 w4558 w4588 w4625 w4642 w4660 w4669 w4682 w4697 w4713 w4722 w4737 w4756 w4776 w4794 w4808 w4839 w4851 w4864 w4877 w4890 w4900 w4911 w4924 w4941 w4960 w4969 w4985 w5001 w5017 w5033 w5049 w5063 w5068 w5089]
      tunnel: [w4151 w4163 w4179 w4197 w4213 w4228 w4242 w4256 w4270 w4284 w4300 w4315 w4328 w4340 w4356 w4374 w4386 w4408 w4425 w4439 w4463 w4486 w4497 w4510 w4525 w4538 w4557 w4587 w4624 w4642 w4660 w4669 w4682 w4697 w4713 w4722 w4737 w4755 w4776 w4794 w4808 w4839 w4851 w4864 w4877 w4890 w4900 w4911 w4924 w4941 w4960 w4969 w4985 w5001 w5017 w5033 w5049 w5063 w5068 w5089] -> w253
      tunnel: w251 -> [w4150 w4162 w4178 w4199 w4212 w4227 w4241 w4255 w4269 w4283 w4299 w4314 w4327 w4339 w4355 w4373 w4394 w4410 w4427 w4438 w4469 w4485 w4496 w4509 w4524 w4537 w4554 w4579 w4615 w4641 w4657 w4668 w4680 w4696 w4712 w4725 w4736 w4761 w4784 w4796 w4806 w4837 w4848 w4861 w4874 w4887 w4902 w4913 w4926 w4943 w4957 w4971 w4987 w5003 w5019 w5035 w5051 w5065 w5070 w5091]
      tunnel: [w4150 w4162 w4178 w4199 w4212 w4227 w4241 w4255 w4269 w4283 w4299 w4314 w4327 w4339 w4355 w4373 w4394 w4410 w4427 w4438 w4468 w4485 w4496 w4509 w4524 w4537 w4554 w4578 w4614 w4641 w4657 w4668 w4680 w4696 w4712 w4725 w4736 w4761 w4784 w4796 w4806 w4837 w4848 w4861 w4874 w4887 w4902 w4913 w4926 w4943 w4956 w4971 w4987 w5003 w5019 w5035 w5051 w5065 w5070 w5091] -> w250
      tunnel: w248 -> [w4149 w4161 w4176 w4200 w4210 w4225 w4239 w4254 w4268 w4282 w4297 w4312 w4326 w4338 w4354 w4366 w4389 w4411 w4428 w4437 w4459 w4484 w4495 w4508 w4523 w4536 w4553 w4575 w4611 w4640 w4654 w4667 w4679 w4695 w4711 w4724 w4735 w4762 w4785 w4797 w4805 w4836 w4847 w4860 w4873 w4884 w4903 w4914 w4927 w4944 w4951 w4972 w4988 w5004 w5020 w5036 w5052 w5066 w5071 w5092]
      tunnel: [w4149 w4161 w4176 w4200 w4210 w4225 w4239 w4254 w4268 w4282 w4297 w4312 w4326 w4338 w4354 w4366 w4388 w4411 w4428 w4437 w4458 w4484 w4495 w4508 w4523 w4536 w4553 w4574 w4610 w4640 w4654 w4667 w4679 w4695 w4711 w4724 w4735 w4762 w4785 w4797 w4805 w4836 w4847 w4860 w4873 w4884 w4903 w4914 w4927 w4944 w4951 w4972 w4988 w5004 w5020 w5036 w5052 w5066 w5071 w5092] -> w247
      tunnel: w245 -> [w4147 w4160 w4177 w4201 w4211 w4226 w4240 w4253 w4267 w4281 w4298 w4313 w4325 w4337 w4353 w4365 w4385 w4412 w4429 w4436 w4455 w4481 w4494 w4507 w4522 w4535 w4552 w4572 w4608 w4638 w4653 w4666 w4678 w4694 w4710 w4723 w4734 w4763 w4786 w4798 w4804 w4835 w4846 w4859 w4872 w4883 w4904 w4915 w4928 w4945 w4950 w4966 w4982 w4998 w5014 w5030 w5046 w5060 w5072 w5093]
      tunnel: [w4147 w4160 w4177 w4201 w4211 w4226 w4240 w4253 w4267 w4281 w4298 w4313 w4325 w4337 w4353 w4365 w4385 w4412 w4429 w4436 w4455 w4481 w4494 w4507 w4522 w4535 w4551 w4571 w4607 w4638 w4653 w4666 w4678 w4694 w4710 w4723 w4734 w4763 w4786 w4798 w4804 w4835 w4846 w4859 w4872 w4883 w4904 w4915 w4928 w4945 w4950 w4966 w4980 w4996 w5012 w5028 w5045 w5059 w5072 w5093] -> w244
      tunnel: w242 -> [_ _ _ _ _ _ _ _ _ _ _ _ _ _ _ _ _ _ _ _ _ _ _ _ _ _ _ _ _ _ _ _ _ _ _ _ _ _ _ _ _ _ _ _ _ _ _ _ _ w4936 _ _ _ _ _ _ _ _ _ _]
      tunnel: [w4146 w4159 w4171 w4191 w4205 w4220 w4235 w4249 w4263 w4277 w4293 w4307 w4322 w4336 w4347 w4364 w4382 w4403 w4430 w4435 w4452 w4480 w4493 w4506 w4521 w4532 w4545 w4565 w4599 w4637 w4652 w4665 w4683 w4688 w4704 w4720 w4732 w4751 w4779 w4790 w4810 w4841 w4845 w4858 w4871 w4882 w4895 w4916 w4929 w4934 w4949 w4965 w4978 w4994 w5010 w5026 w5043 w5056 w5076 w5096] -> w238
      tunnel: w239 -> [w4146 w4159 w4171 w4191 w4205 w4220 w4235 w4249 w4263 w4277 w4293 w4307 w4322 w4336 w4347 w4364 w4382 w4404 w4430 w4435 w4452 w4480 w4493 w4506 w4521 w4532 w4545 w4566 w4600 w4637 w4652 w4665 w4683 w4688 w4704 w4720 w4732 w4751 w4779 w4790 w4810 w4841 w4845 w4858 w4871 w4882 w4895 w4916 w4929 w4934 w4949 w4965 w4978 w4994 w5010 w5026 w5043 w5056 w5076 w5096]
      tunnel: w236 -> [_ _ _ _ _ _ _ _ _ _ w4292 _ _ _ _ _ _ _ _ _ _ _ _ _ _ _ _ _ _ _ _ _ _ _ _ _ _ _ _ _ _ _ _ _ _ _ _ _ _ _ _ _ _ _ _ _ _ _ _ _]
      tunnel: w234 -> [w4145 w4158 w4170 w4185 w4204 w4219 w4234 w4248 w4262 w4276 w4290 w4306 w4321 w4335 w4346 w4363 w4381 w4399 w4423 w4434 w4450 w4479 w4492 w4505 w4520 w4531 w4548 w4568 w4603 w4636 w4651 w4664 w4675 w4687 w4703 w4719 w4731 w4749 w4778 w4789 w4801 w4833 w4844 w4857 w4870 w4881 w4894 w4907 w4920 w4933 w4948 w4964 w4977 w4993 w5009 w5025 w5042 w5055 w5075 w5095]
      tunnel: [w4145 w4158 w4170 w4185 w4204 w4219 w4234 w4248 w4262 w4276 w4290 w4306 w4321 w4335 w4346 w4363 w4381 w4399 w4422 w4434 w4450 w4479 w4492 w4505 w4520 w4531 w4547 w4567 w4602 w4636 w4651 w4664 w4675 w4687 w4703 w4719 w4731 w4749 w4778 w4789 w4801 w4833 w4844 w4857 w4870 w4881 w4894 w4907 w4920 w4933 w4948 w4964 w4977 w4993 w5009 w5025 w5042 w5055 w5075 w5095] -> w233
      tunnel: [_ _ _ _ _ _ _ _ _ _ _ _ _ _ _ _ _ _ _ _ _ _ _ _ _ _ _ _ _ _ _ _ _ _ _ _ _ w4743 w4773 _ _ _ _ _ _ _ _ _ _ _ _ _ _ _ _ _ _ _ _ _] -> w231
      tunnel: w229 -> [w4144 w4157 w4169 w4184 w4203 w4218 w4233 w4247 w4261 w4275 w4289 w4305 w4320 w4334 w4345 w4362 w4380 w4398 w4414 w4433 w4448 w4478 w4491 w4504 w4519 w4530 w4549 w4569 w4604 w4635 w4650 w4663 w4674 w4686 w4702 w4718 w4730 w4745 w4777 w4788 w4800 w4832 w4843 w4856 w4869 w4880 w4893 w4906 w4919 w4932 w4947 w4963 w4976 w4992 w5008 w5024 w5041 w5054 w5074 w5094]
      tunnel: [w4144 w4157 w4169 w4184 w4203 w4218 w4233 w4247 w4261 w4275 w4289 w4305 w4320 w4334 w4345 w4362 w4380 w4398 w4414 w4433 w4448 w4478 w4491 w4504 w4519 w4530 w4549 w4569 w4604 w4635 w4650 w4663 w4674 w4686 w4702 w4718 w4730 w4745 w4777 w4788 w4800 w4832 w4843 w4856 w4869 w4880 w4893 w4906 w4919 w4932 w4947 w4963 w4976 w4992 w5008 w5024 w5041 w5054 w5074 w5094] -> w228
      tunnel: w224 -> [w4143 w4156 w4168 w4183 w4202 w4217 w4232 w4246 w4260 w4274 w4288 w4304 w4319 w4333 w4344 w4361 w4379 w4395 w4413 w4432 w4447 w4477 w4490 w4503 w4518 w4529 w4544 w4562 w4598 w4634 w4649 w4662 w4673 w4685 w4701 w4717 w4729 w4748 w4771 w4787 w4799 w4831 w4842 w4855 w4868 w4879 w4892 w4905 w4918 w4931 w4946 w4962 w4975 w4991 w5007 w5023 w5040 w5053 w5073 w5088]
      tunnel: [w4143 w4156 w4168 w4183 w4202 w4217 w4232 w4246 w4260 w4274 w4288 w4304 w4319 w4333 w4344 w4361 w4379 w4395 w4413 w4432 w4447 w4477 w4490 w4503 w4518 w4529 w4543 w4562 w4598 w4634 w4649 w4662 w4673 w4685 w4701 w4717 w4729 w4748 w4764 w4787 w4799 w4830 w4842 w4855 w4868 w4879 w4892 w4905 w4918 w4931 w4946 w4962 w4975 w4991 w5007 w5023 w5040 w5053 w5073 w5087] -> w223
      frame "Exit" {
        # ">>State Logic  >>"
        # ">>> Time cluster >>>"
        # ">>> Yaw >>>"
        # ">>> Stepper position >>>"
        # ">>> Encoders >>>"
        # ">>> Object detection >>>"
        # ">>> Ultrasonic Sensors Detect >>>"
        n71 = call "Imaq Dispose"("All Images? (No)"=TRUE) -> ()  [unwired: 5 in, 1 out]
      }
      frame "----Movement States----" {
        # ">>State Logic  >>"
        # ">>> Time cluster >>>"
        # ">>> Yaw >>>"
        # ">>> Stepper position >>>"
        # ">>> Encoders >>>"
        # ">>> Object detection >>>"
        # ">>> Ultrasonic Sensors Detect >>>"
      }
      frame "FORWARD" {
        # "High voltage values: 30\nMid voltage values: 40\nLow voltage values: 50"
        # ">>State Logic  >>"
        # ">>> Time cluster >>>"
        # ">>> Yaw >>>"
        # ">>> Stepper position >>>"
        # ">>> Encoders >>>"
        # ">>> Object detection >>>"
        # ">>> Ultrasonic Sensors Detect >>>"
        n72 = Unbundle By Name(w4176) -> ("Yaw"=w4172:dbl)
        n73 = call "MOTOR CONTROL WITH PID AE.vi"("Yaw"=w4172, "Speed"=30.0, "Direction"=MOTOR_CONTROL_WITH_PID_AE_DIRECTION_TYPE_DEF."y-axis movement", "AE Mode"=MOTOR_CONTROL_WITH_PID_AE_DATA_MODE_TYPE_DEF."Write to AE") -> ()  [unwired: 1 out]
      }
      frame "FORWARD - IR ASSIST" {
        # "Algorithm sensitivity"
        # "Distance to maintain from wall"
        # ">>State Logic  >>"
        # ">>> Time cluster >>>"
        # ">>> Yaw >>>"
        # ">>> Stepper position >>>"
        # ">>> Encoders >>>"
        # ">>> Object detection >>>"
        # ">>> Ultrasonic Sensors Detect >>>"
        n74 = Unbundle By Name(w4191) -> ("Left IR Sensor"=w4190:dbl)
        n75 = Subtract(x=w4190, y=30.0) -> (x-y=w4188:dbl)
        n76 = Multiply(x=w4188, y=0.2) -> (x*y=w4186:dbl)
        n77 = call "MOTOR CONTROL WITH PID AE.vi"("Yaw"=w4186, "Speed"=35.0, "Direction"=MOTOR_CONTROL_WITH_PID_AE_DIRECTION_TYPE_DEF."y-axis movement", "AE Mode"=MOTOR_CONTROL_WITH_PID_AE_DATA_MODE_TYPE_DEF."Write to AE") -> ()  [unwired: 1 out]
      }
      frame "LEFT" {
        # ">>State Logic  >>"
        # ">>> Time cluster >>>"
        # ">>> Yaw >>>"
        # ">>> Stepper position >>>"
        # ">>> Encoders >>>"
        # ">>> Object detection >>>"
        # ">>> Ultrasonic Sensors Detect >>>"
        n78 = Unbundle By Name(w4210) -> ("Yaw"=w4207:dbl)
        n79 = call "MOTOR CONTROL WITH PID AE.vi"("Yaw"=w4207, "Speed"=-25.0, "Direction"=MOTOR_CONTROL_WITH_PID_AE_DIRECTION_TYPE_DEF."x-axis movement", "AE Mode"=MOTOR_CONTROL_WITH_PID_AE_DATA_MODE_TYPE_DEF."Write to AE") -> ()  [unwired: 1 out]
      }
      frame "RIGHT" {
        # ">>> Time cluster >>>"
        # ">>> Yaw >>>"
        # ">>> Stepper position >>>"
        # ">>> Encoders >>>"
        # ">>> Object detection >>>"
        # ">>> Ultrasonic Sensors Detect >>>"
        n80 = Unbundle By Name(w4225) -> ("Yaw"=w4221:dbl)
        n81 = call "MOTOR CONTROL WITH PID AE.vi"("Yaw"=w4221, "Speed"=25.0, "Direction"=MOTOR_CONTROL_WITH_PID_AE_DIRECTION_TYPE_DEF."x-axis movement", "AE Mode"=MOTOR_CONTROL_WITH_PID_AE_DATA_MODE_TYPE_DEF."Write to AE") -> ()  [unwired: 1 out]
      }
      frame "R-ACW" {
        # ">>> IR Sensors >>>"
        # ">>> Time cluster >>>"
        # ">>> Yaw >>>"
        # ">>> Stepper position >>>"
        # ">>> Encoders >>>"
        # ">>> Object detection >>>"
        # ">>> Ultrasonic Sensors Detect >>>"
        n82 = call "MOTOR CONTROL WITH PID AE.vi"("Speed"=10.0, "Direction"=MOTOR_CONTROL_WITH_PID_AE_DIRECTION_TYPE_DEF."rotation", "AE Mode"=MOTOR_CONTROL_WITH_PID_AE_DATA_MODE_TYPE_DEF."Write to AE") -> ()  [unwired: 1 in, 1 out]
      }
      frame "R-CW" {
        (unwired) -0.2 ("Speed")
        # ">>> Time cluster >>>"
        # ">>> Yaw >>>"
        # ">>> Stepper position >>>"
        # ">>> Encoders >>>"
        # ">>> Object detection >>>"
        # ">>> Ultrasonic Sensors Detect >>>"
        n83 = call "MOTOR CONTROL WITH PID AE.vi"("Speed"=-10.0, "Direction"=MOTOR_CONTROL_WITH_PID_AE_DIRECTION_TYPE_DEF."rotation", "AE Mode"=MOTOR_CONTROL_WITH_PID_AE_DATA_MODE_TYPE_DEF."Write to AE") -> ()  [unwired: 1 in, 1 out]
      }
      frame "R-ACW SLOW" {
        (unwired) -0.2 ("Speed")
        # ">>> Time cluster >>>"
        # ">>> Yaw >>>"
        # ">>> Stepper position >>>"
        # ">>> Encoders >>>"
        # ">>> Object detection >>>"
        # ">>> Ultrasonic Sensors Detect >>>"
        n84 = call "MOTOR CONTROL WITH PID AE.vi"("Speed"=5.0, "Direction"=MOTOR_CONTROL_WITH_PID_AE_DIRECTION_TYPE_DEF."rotation", "AE Mode"=MOTOR_CONTROL_WITH_PID_AE_DATA_MODE_TYPE_DEF."Write to AE") -> ()  [unwired: 1 in, 1 out]
      }
      frame "R-CW SLOW" {
        (unwired) -0.2 ("Speed")
        # ">>> Time cluster >>>"
        # ">>> Yaw >>>"
        # ">>> Stepper position >>>"
        # ">>> Encoders >>>"
        # ">>> Object detection >>>"
        # ">>> Ultrasonic Sensors Detect >>>"
        n85 = call "MOTOR CONTROL WITH PID AE.vi"("Speed"=-5.0, "Direction"=MOTOR_CONTROL_WITH_PID_AE_DIRECTION_TYPE_DEF."rotation", "AE Mode"=MOTOR_CONTROL_WITH_PID_AE_DATA_MODE_TYPE_DEF."Write to AE") -> ()  [unwired: 1 in, 1 out]
      }
      frame "X AXIS - SLOW" {
        # ">>> Line Sensor Cluster>>>"
        # ">>> IR Sensors >>>"
        # ">>> Time cluster >>>"
        # ">>> Yaw >>>"
        # ">>> Stepper position >>>"
        # ">>> Encoders >>>"
        # ">>> Object detection >>>"
        # ">>> Ultrasonic Sensors Detect >>>"
        n86 = Unbundle By Name(w4292) -> ("xSpeed"=w4291:dbl)
        n87 = Unbundle By Name(w4297) -> ("Yaw"=w4294:dbl)
        n88 = call "MOTOR CONTROL WITH PID AE.vi"("Yaw"=w4294, "Speed"=w4291, "Direction"=MOTOR_CONTROL_WITH_PID_AE_DIRECTION_TYPE_DEF."x-axis movement", "AE Mode"=MOTOR_CONTROL_WITH_PID_AE_DATA_MODE_TYPE_DEF."Write to AE") -> ()  [unwired: 1 out]
      }
      frame "REVERSE" {
        # ">>> Time cluster >>>"
        # ">>> Yaw >>>"
        # ">>> Stepper position >>>"
        # ">>> Encoders >>>"
        # ">>> Object detection >>>"
        # ">>> Ultrasonic Sensors Detect >>>"
        n89 = Unbundle By Name(w4312) -> ("Yaw"=w4308:dbl)
        n90 = call "MOTOR CONTROL WITH PID AE.vi"("Yaw"=w4308, "Speed"=-40.0, "Direction"=MOTOR_CONTROL_WITH_PID_AE_DIRECTION_TYPE_DEF."y-axis movement", "AE Mode"=MOTOR_CONTROL_WITH_PID_AE_DATA_MODE_TYPE_DEF."Write to AE") -> ()  [unwired: 1 out]
      }
      frame "STOP" {
        n91 = Wait (ms)(milliseconds to wait=u32 100) -> ()  [unwired: 1 out]
        n92 = call "MOTOR CONTROL WITH PID AE.vi"("Direction"=MOTOR_CONTROL_WITH_PID_AE_DIRECTION_TYPE_DEF."stop", "AE Mode"=MOTOR_CONTROL_WITH_PID_AE_DATA_MODE_TYPE_DEF."Write to AE") -> ()  [unwired: 2 in, 1 out]
      }
      frame "----SENSOR READING---- " {
      }
      frame "READ ENCODERS" {
        # ">>> Time cluster >>>"
        # ">>> Yaw >>>"
        # ">>> Stepper position >>>"
        # ">>> Object detection >>>"
        # ">>> Current encoder distance >>>"
        # ">>> Ultrasonic Sensors Detect >>>"
        n93 = call "MOTOR CONTROL WITH PID AE.vi"("AE Mode"=MOTOR_CONTROL_WITH_PID_AE_DATA_MODE_TYPE_DEF."Read from AE") -> ("Speed & distance"=w4351:T15)  [unwired: 3 in]
        n94 = Unbundle By Name(w4351) -> ("xDistance"=w4350:dbl, "yDistance"=w4349:dbl, "wDistance"=w4348:dbl)
        n95 = Bundle By Name(cluster=w4358, "xDistance"=w4350, "yDistance"=w4349, "wDistance"=w4348) -> (w4357:T8)
      }
      frame "READ ULTRASONIC" {
        (unwired) navX_type_def."Read Values" ("Mode")
        (unwired) MOTOR_CONTROL_NO_PID_Type_Def."Latch" ("Direction")
        # ">>> Line Sensor Cluster>>>"
        # ">>> IR Sensors >>>"
        # ">>State Logic  >>"
        # ">>> Time cluster >>>"
        # ">>> Ultrasonic Sensors Detect >>>"
        # ">>> Object detection >>>"
        # ">>> Encoders >>>"
        # ">>> Stepper position >>>"
        # ">>> Yaw >>>"
        n96 = call "Arduino Interfacing VI.vi"("AE Mode"=Arduino_Interfacing."Read From Arduino") -> ("Arduino Data"=w4371:T17)  [unwired: 3 in, 1 out]
        n97 = Unbundle By Name(w4371) -> ("PING A"=w4370:u8, "PING B"=w4369:u8, "PING C"=w4368:u8, "PING D"=w4367:u8)
        n98 = Bundle By Name(cluster=w4377, "PING_A"=w4370, "PING_B"=w4369, "PING_C"=w4368, "PING_D"=w4367) -> (w4378:T9)
      }
      frame "READ NAVX" {
        # ">> Item Selection Bias >>"
        # ">>State Logic  >>"
        # ">>> Line Sensor Cluster>>>"
        # ">>> IR Sensors >>>"
        # ">>> Time cluster >>>"
        # ">>> Yaw >>>"
        # ">>> Ultrasonic Sensors Detect >>>"
        # ">>> Object detection >>>"
        # ">>> Encoders >>>"
        # ">>> Stepper position >>>"
        n99 = call "navX reading VI.vi"("Mode"=navX_type_def."Read Values") -> ("NavX Readings"=w4384:T16)  [unwired: 2 in, 3 out]
        n100 = Unbundle By Name(w4384) -> ("Heading"=w4383:dbl)
        n101 = Unbundle By Name(w4384) -> ("Yaw"=w4387:dbl)
        n102 = Bundle By Name(cluster=w4389, "Yaw"=w4387, "Compass"=w4383) -> (w4388:T6)
      }
      frame "READ IR" {
        w4397 = T41 [enum."B/AI2"] items=["Not Connected", "AudioIn/Left", "AudioIn/Right", "C/AI0", "C/AI1", "A/AI0", "A/AI1", "A/AI2", "A/AI3", "A/AI4", "A/AI5", "A/AI6", "A/AI7", "B/AI0", "B/AI1", "B/AI2", "B/AI3", "B/AI4", "B/AI5", "B/AI6", "B/AI7", "AI/AI0", "AI/AI1", "AI/AI2", "AI/AI3", "A/AI0 (DIFF)", "A/AI1 (DIFF)", "A/AI2 (DIFF)", "A/AI3 (DIFF)", "B/AI0 (DIFF)", "B/AI1 (DIFF)", "B/AI2 (DIFF)", "B/AI3 (DIFF)"] ("AI Channel")
        w4401 = T41 [enum."B/AI1"] items=["Not Connected", "AudioIn/Left", "AudioIn/Right", "C/AI0", "C/AI1", "A/AI0", "A/AI1", "A/AI2", "A/AI3", "A/AI4", "A/AI5", "A/AI6", "A/AI7", "B/AI0", "B/AI1", "B/AI2", "B/AI3", "B/AI4", "B/AI5", "B/AI6", "B/AI7", "AI/AI0", "AI/AI1", "AI/AI2", "AI/AI3", "A/AI0 (DIFF)", "A/AI1 (DIFF)", "A/AI2 (DIFF)", "A/AI3 (DIFF)", "B/AI0 (DIFF)", "B/AI1 (DIFF)", "B/AI2 (DIFF)", "B/AI3 (DIFF)"] ("AI Channel")
        w4406 = T41 [enum."B/AI0"] items=["Not Connected", "AudioIn/Left", "AudioIn/Right", "C/AI0", "C/AI1", "A/AI0", "A/AI1", "A/AI2", "A/AI3", "A/AI4", "A/AI5", "A/AI6", "A/AI7", "B/AI0", "B/AI1", "B/AI2", "B/AI3", "B/AI4", "B/AI5", "B/AI6", "B/AI7", "AI/AI0", "AI/AI1", "AI/AI2", "AI/AI3", "A/AI0 (DIFF)", "A/AI1 (DIFF)", "A/AI2 (DIFF)", "A/AI3 (DIFF)", "B/AI0 (DIFF)", "B/AI1 (DIFF)", "B/AI2 (DIFF)", "B/AI3 (DIFF)"] ("AI Channel")
        # ">>> Line Sensor Cluster>>>"
        # ">>> IR Sensors >>>"
        # ">>State Logic  >>"
        # ">>> Time cluster >>>"
        # ">>> Ultrasonic Sensors Detect >>>"
        # ">>> Object detection >>>"
        # ">>> Encoders >>>"
        # ">>> Stepper position >>>"
        # ">>> Yaw >>>"
        n103 = call <vilib>:"Sharp IR.vi"("AI Channel"=w4406) -> ("Sharp IR Distance"=w4402:dbl)  [unwired: 8 in, 2 out]
        n104 = call <vilib>:"Sharp IR.vi"("AI Channel"=w4401) -> ("Sharp IR Distance"=w4400:dbl)  [unwired: 8 in, 2 out]
        n105 = call <vilib>:"Sharp IR.vi"("AI Channel"=w4397) -> ("Sharp IR Distance"=w4396:dbl)  [unwired: 8 in, 2 out]
        n106 = Bundle By Name(cluster=w4404, "Left IR Sensor"=w4402, "Arm IR Sensor"=w4400, "Bottom IR Sensor"=w4396) -> (w4403:T5)
      }
      frame "READ LINE SENSOR" {
        # ">>> IR Sensors >>>"
        # ">>> Line Sensor Cluster>>>"
        # ">>State Logic  >>"
        # ">>> Time cluster >>>"
        # ">>> Object detection >>>"
        # ">>> Yaw >>>"
        # ">>> Ultrasonic Sensors Detect >>>"
        # ">>> Encoders >>>"
        # ">>> Stepper position >>>"
        n107 = call "Line Sensor AE.vi"("AE State"=Line_Sensor_AE_Type_Def."READ FROM LINE SENSORS") -> ("Line Detected?"=w4420:bool, "Line Sensor Raw Values"=w4419:T43)
        n108 = Unbundle By Name(w4419) -> ("S1"=w4418:dbl, "S2"=w4417:dbl, "S3"=w4416:dbl, "S4"=w4415:dbl)
        n109 = Bundle By Name(cluster=w4423, "Line Detected?"=w4420, "S1"=w4418, "S2"=w4417, "S3"=w4416, "S4"=w4415) -> (w4422:T4)
      }
      frame "----SYSTEM MODES----" {
        (unwired) I2C_MASTER_Type_Def."Last State" ("Arduino Mode")
        # ">>> Object detection >>>"
        # ">>> Yaw >>>"
        # ">>> Ultrasonic Sensors Detect >>>"
        # ">>> Encoders >>>"
        # ">>> Stepper position >>>"
      }
      frame "INIT" {
        w4470 = u8 0
        w4471 = 0.0
        # ">>> Box Colour Detection >>>"
        # ">>> IR Sensors >>>"
        # ">>> IR Sensors >>>"
        # ">>> Line Sensor Cluster>>>"
        # ">>> Time cluster >>>"
        # ">>> Object detection >>>"
        # ">>> Yaw >>>"
        # ">>> Ultrasonic Sensors Detect >>>"
        # ">>> Encoders >>>"
        # ">>> Stepper position >>>"
        # ">>State Logic  >>"
        n110 = call "Arduino Interfacing VI.vi"("AE Mode"=Arduino_Interfacing."Initialize") -> ()  [unwired: 3 in, 2 out]
        n111 = call "FGV Stop.vi"("Init/Read/Write State"=States_for_Action_Engine."Initialize") -> ()  [unwired: 2 in, 2 out]
        n112 = call "Elasped Timer.vi"("Action"=Elapsed_timer_control."Initialize") -> ()  [unwired: 7 in, 4 out]
        n113 = call "MOTOR CONTROL WITH PID AE.vi"("AE Mode"=MOTOR_CONTROL_WITH_PID_AE_DATA_MODE_TYPE_DEF."Init AE") -> ()  [unwired: 3 in, 1 out]
        n114 = call "IMAQ Reference AE.vi"("IMAQ AE States"=IMAQ_Reference_AE."Initialize AE") -> ()  [unwired: 1 in, 2 out]
        n115 = call "Line Sensor AE.vi"("AE State"=Line_Sensor_AE_Type_Def."INIT AE") -> ()  [unwired: 2 out]
        n116 = Bundle By Name(cluster=w4464, "Recognized Object"=FALSE, "Object X coordinate"=0.0, "Object Y coordinate"=0.0) -> (w4463:T11)
        n117 = Bundle By Name(cluster=w4469, "y Stepper Position"=u8 0, "z Stepper Position"=u8 0) -> (w4468:T7)
        n118 = Bundle By Name(cluster=w4473, "xDistance"=w4471, "yDistance"=w4471, "wDistance"=w4471) -> (w4472:T8)
        n119 = Bundle By Name(cluster=w4475, "PING_A"=w4470, "PING_B"=w4470, "PING_C"=w4470, "PING_D"=w4470) -> (w4476:T9)
        n120 = invoke class="VI" method="Default Vals.Reinit All"() -> ()  [unwired: 3 in, 3 out]
        n121 = Bundle By Name(cluster=w4459, "Yaw"=0.0) -> (w4458:T6)
        n122 = call "Box Colour FGV.vi"("Init/R/W State"=Box_Colour_FGV_States."Initialize") -> ()  [unwired: 9 in, 2 out]
        n123 = call "Servo State FGV.vi"("Init/Read/Write State"=States_for_Action_Engine."Initialize") -> ()  [unwired: 2 in, 2 out]
        n124 = call "yDistance travelled FGV.vi"("Init/Read/Write State"=States_for_Action_Engine."Initialize") -> ()  [unwired: 9 in, 2 out]
        n125 = call "Task Enable FGV.vi"("Init/Read/Write State"=States_for_Action_Engine."Initialize") -> ()  [unwired: 9 in, 2 out]
      }
      frame "ARDUINO - ULTRASONIC" {
        # ">>> Time cluster >>>"
        # ">>> Line Sensor Cluster>>>"
        # ">>> Object detection >>>"
        # ">>> Yaw >>>"
        # ">>> Ultrasonic Sensors Detect >>>"
        # ">>> Encoders >>>"
        # ">>> Stepper position >>>"
        # ">>State Logic  >>"
        n126 = call "Arduino Interfacing VI.vi"("Data to Write"=I2C_MASTER_WRITE_NEW_Type_Def."Ultrasonic sensors", "AE Mode"=Arduino_Interfacing."Write to Arduino") -> ()  [unwired: 2 in, 2 out]
      }
      frame "NAVX CALIBRATE" {
        # ">>> Object detection >>>"
        # ">>> Yaw >>>"
        # ">>> Ultrasonic Sensors Detect >>>"
        # ">>> Encoders >>>"
        # ">>> Stepper position >>>"
        # ">>State Logic  >>"
        # "Adds a 15 second delay to the startup process \nfor the NavX to calibrate"
        n127 = Wait (ms)(milliseconds to wait=u32 1000) -> ()  [unwired: 1 out]
      }
      frame "NO ACTION", Default {
        (unwired) u8 0 ("y Stepper value")
        (unwired) TRUE ("Latch")
        (unwired) navX_type_def."Read Values" ("Mode")
        (unwired) MOTOR_CONTROL_NO_PID_Type_Def."Latch" ("Direction")
        # ">>> Object detection >>>"
        # ">>> Yaw >>>"
        # ">>> Ultrasonic Sensors Detect >>>"
        # ">>> Encoders >>>"
        # ">>> Stepper position >>>"
        # ">>State Logic  >>"
        n128 = case shown="\"Idle\"" w4512 {
          tunnel: [0 100] -> w4514
          frame "Startup", Default {
          }
          frame "Idle" {
          }
        }
      }
      frame "----RESET CASES----" {
        (unwired) I2C_MASTER_Type_Def."Last State" ("Arduino Mode")
        # ">>> Object detection >>>"
        # ">>> Yaw >>>"
        # ">>> Ultrasonic Sensors Detect >>>"
        # ">>> Encoders >>>"
        # ">>> Stepper position >>>"
        # ">>State Logic  >>"
      }
      frame "RESET ENCODERS" {
        # ">>> Object detection >>>"
        # ">>> Yaw >>>"
        # ">>> Ultrasonic Sensors Detect >>>"
        # ">>> Encoders >>>"
        # ">>> Stepper position >>>"
        # ">>State Logic  >>"
        n129 = call "MOTOR CONTROL WITH PID AE.vi"("Direction"=MOTOR_CONTROL_WITH_PID_AE_DIRECTION_TYPE_DEF."reset encoders", "AE Mode"=MOTOR_CONTROL_WITH_PID_AE_DATA_MODE_TYPE_DEF."Write to AE") -> ()  [unwired: 2 in, 1 out]
      }
      frame "RESET FLAGS" {
        w4542 = FALSE ("Line Detected?")
        # ">>> Line Sensor Cluster>>>"
        # ">>> IR Sensors >>>"
        # ">>> Time cluster >>>"
        # ">>> Object detection >>>"
        # ">>> Yaw >>>"
        # ">>> Ultrasonic Sensors Detect >>>"
        # ">>> Encoders >>>"
        # ">>> Stepper position >>>"
        # ">>> Line Sensor Cluster>>>"
        # ">>> IR Sensors >>>"
        # ">>> Time cluster >>>"
        # ">>> Object detection >>>"
        # ">>> Yaw >>>"
        # ">>> Ultrasonic Sensors Detect >>>"
        # ">>> Encoders >>>"
        # ">>> Stepper position >>>"
        # "Resets BOOLEAN FLAGS only"
        n130 = Wait (ms)(milliseconds to wait=u32 20) -> ()  [unwired: 1 out]
        n131 = Bundle By Name(cluster=w4558, "Recognized Object"=FALSE) -> (w4557:T11)
        n132 = Bundle By Name(cluster=w4548, "Line Detected?"=FALSE) -> (w4547:T4)
        n133 = Bundle By Name(cluster=w4552, "Time up flag"=FALSE) -> (w4551:T3)
        n134 = Bundle By Name(cluster=w4544, "Red"=w4542, "Black"=w4542, "Blue"=w4542, "Yellow"=w4542, "Green"=w4542, "Unknown"=w4542, "Image processing done"=w4542) -> (w4543:T1)
      }
      frame "RESET SENSOR VALUES" {
        w4563 = 0.0 ("S4")
        w4564 = 0.0 ("S4")
        # "Resets SENSOR VALUES only"
        # ">>> Line Sensor Cluster>>>"
        # ">>> IR Sensors >>>"
        # ">>> Time cluster >>>"
        # ">>> Object detection >>>"
        # ">>> Yaw >>>"
        # ">>> Ultrasonic Sensors Detect >>>"
        # ">>> Encoders >>>"
        # ">>> Stepper position >>>"
        # ">>> Line Sensor Cluster>>>"
        # ">>> IR Sensors >>>"
        # ">>> Time cluster >>>"
        # ">>> Object detection >>>"
        # ">>> Yaw >>>"
        # ">>> Ultrasonic Sensors Detect >>>"
        # ">>> Encoders >>>"
        # ">>> Stepper position >>>"
        # "Resets any software variables\nand/or non-critical states"
        n135 = Wait (ms)(milliseconds to wait=u32 20) -> ()  [unwired: 1 out]
        n136 = Bundle By Name(cluster=w4572, "SET TIME TO CHECK"=0.0) -> (w4571:T3)
        n137 = Bundle By Name(cluster=w4588, "Object X coordinate"=0.0, "Object Y coordinate"=0.0) -> (w4587:T11)
        n138 = Bundle By Name(cluster=w4579, "y Stepper Position"=u8 0, "z Stepper Position"=u8 0) -> (w4578:T7)
        n139 = Bundle By Name(cluster=w4566, "Left IR Sensor"=w4563, "Arm IR Sensor"=w4563) -> (w4565:T5)
        n140 = Bundle By Name(cluster=w4584, "xDistance"=0.0, "yDistance"=0.0, "wDistance"=0.0) -> (w4583:T8)
        n141 = Bundle By Name(cluster=w4595, "PING_A"=u8 0, "PING_B"=u8 0, "PING_C"=u8 0, "PING_D"=u8 0) -> (w4594:T9)
        n142 = Bundle By Name(cluster=w4575, "Yaw"=0.0) -> (w4574:T6)
        n143 = Bundle By Name(cluster=w4568, "S1"=w4564, "S2"=w4564, "S3"=w4564, "S4"=w4564) -> (w4567:T4)
      }
      frame "RESET ALL SENSORS" {
        w4597 = 0.0 ("SET TIME TO CHECK")
        # ">>> Line Sensor Cluster>>>"
        # ">>> IR Sensors >>>"
        # ">>> Time cluster >>>"
        # ">>> Object detection >>>"
        # ">>> Yaw >>>"
        # ">>> Ultrasonic Sensors Detect >>>"
        # ">>> Encoders >>>"
        # ">>> Stepper position >>>"
        # ">>> Line Sensor Cluster>>>"
        # ">>> IR Sensors >>>"
        # ">>> Time cluster >>>"
        # ">>> Object detection >>>"
        # ">>> Yaw >>>"
        # ">>> Ultrasonic Sensors Detect >>>"
        # ">>> Encoders >>>"
        # ">>> Stepper position >>>"
        # "Resets ALL SENSOR PARAMTERS"
        n144 = Wait (ms)(milliseconds to wait=u32 20) -> ()  [unwired: 1 out]
        n145 = Bundle By Name(cluster=w4608, "Time up flag"=FALSE, "SET TIME TO CHECK"=0.0) -> (w4607:T3)
        n146 = Bundle By Name(cluster=w4625, "Recognized Object"=FALSE, "Object X coordinate"=0.0, "Object Y coordinate"=0.0) -> (w4624:T11)
        n147 = Bundle By Name(cluster=w4615, "y Stepper Position"=u8 0, "z Stepper Position"=u8 0) -> (w4614:T7)
        n148 = Bundle By Name(cluster=w4600, "Left IR Sensor"=w4597, "Arm IR Sensor"=w4597, "Bottom IR Sensor"=w4597) -> (w4599:T5)
        n149 = Bundle By Name(cluster=w4603, "Line Detected?"=FALSE) -> (w4602:T4)
        n150 = Bundle By Name(cluster=w4620, "xDistance"=0.0, "yDistance"=0.0, "wDistance"=0.0) -> (w4619:T8)
        n151 = Bundle By Name(cluster=w4632, "PING_A"=u8 0, "PING_B"=u8 0, "PING_C"=u8 0, "PING_D"=u8 0) -> (w4631:T9)
        n152 = Bundle By Name(cluster=w4611, "Yaw"=0.0) -> (w4610:T6)
      }
      frame "RESET YAW" {
        n153 = Wait (ms)(milliseconds to wait=u32 100) -> ()  [unwired: 1 out]
        n154 = call "navX reading VI.vi"("Mode"=navX_type_def."Zero Yaw") -> ()  [unwired: 2 in, 4 out]
      }
      frame "RESET ARM" {
        n155 = call "Arduino Interfacing VI.vi"("Data to Write"=I2C_MASTER_WRITE_NEW_Type_Def."Soft Reset", "AE Mode"=Arduino_Interfacing."Write to Arduino") -> ()  [unwired: 2 in, 2 out]
        n156 = call "Servo State FGV.vi"("Init/Read/Write State"=States_for_Action_Engine."Write", "Servo State"=Servo_States_FGV_Enum."Open Claw") -> ()  [unwired: 1 in, 2 out]
      }
      frame "--------CAM STATES-------" {
      }
      frame "OPEN IMAQ REF" {
        # ">>> Line Sensor Cluster>>>"
        # ">>State Logic  >>"
        # ">>> Time cluster >>>"
        # ">>> Object detection >>>"
        # ">>> Yaw >>>"
        # ">>> Ultrasonic Sensors Detect >>>"
        # ">>> Encoders >>>"
        # ">>> Stepper position >>>"
        # ">>> IR Sensors >>>"
        n157 = call "IMAQ Reference AE.vi"("IMAQ AE States"=IMAQ_Reference_AE."Initialize AE") -> ()  [unwired: 1 in, 2 out]
      }
      frame "OPEN LOG CAM" {
        n158 = call "Webcam AE.vi"("Session In"=T39 "cam0", "Camera states"=Webcam_AE."Initialize Camera") -> ("error out"=w4691:errorcluster, "Session Out"=w4690:T39)  [unwired: 1 in, 1 out]
        n159 = call "Webcam AE.vi"("error in (no error)"=w4691, "Session In"=w4690, "Camera states"=Webcam_AE."Open Camera") -> ()  [unwired: 3 out]
      }
      frame "OPEN LIFE CAM" {
        n160 = call "Webcam AE.vi"("Session In"=T39 "cam1", "Camera states"=Webcam_AE."Initialize Camera") -> ("error out"=w4707:errorcluster, "Session Out"=w4706:T39)  [unwired: 1 in, 1 out]
        n161 = call "Webcam AE.vi"("error in (no error)"=w4707, "Session In"=w4706, "Camera states"=Webcam_AE."Open Camera") -> ()  [unwired: 3 out]
      }
      frame "CAM ACQ" {
        # ">>State Logic  >>"
        # ">>> Time cluster >>>"
        # ">>> Yaw >>>"
        # ">>> Stepper position >>>"
        # ">>> Encoders >>>"
        # ">>> Object detection >>>"
        # ">>> Ultrasonic Sensors Detect >>>"
        n162 = call "Webcam AE.vi"("Camera states"=Webcam_AE."Continuous Acquisition") -> ()  [unwired: 2 in, 3 out]
      }
      frame "CAM CLOSE" {
        # ">>> Box Colour Detection >>>"
        # ">>> Line Sensor Cluster>>>"
        # ">>> IR Sensors >>>"
        # ">>State Logic  >>"
        # ">>> Time cluster >>>"
        # ">>> Yaw >>>"
        # ">>> Stepper position >>>"
        # ">>> Encoders >>>"
        # ">>> Object detection >>>"
        # ">>> Ultrasonic Sensors Detect >>>"
        n163 = call "Webcam AE.vi"("Camera states"=Webcam_AE."Close Camera") -> ()  [unwired: 2 in, 3 out]
      }
      frame "PROCESS IMAGE" {
        # ">>> Line Sensor Cluster>>>"
        # ">>> IR Sensors >>>"
        # ">> Item Selection Bias >>"
        # ">> Item Selection Bias >>"
        # ">>State Logic  >>"
        # ">>> Time cluster >>>"
        # ">>> Yaw >>>"
        # ">>> Stepper position >>>"
        # ">>> Encoders >>>"
        # ">>> Object detection >>>"
        # ">>> Ultrasonic Sensors Detect >>>"
        n164 = call "Webcam AE.vi"("Camera states"=Webcam_AE."Retrieve Image") -> ("error out"=w4744:errorcluster, "Image Out"=w4747:T45)  [unwired: 2 in, 1 out]
        n165 = call "IMAQ Reference AE.vi"("IMAQ AE States"=IMAQ_Reference_AE."Get IMAQ Reference") -> ("Image Out"=w4746:T45)  [unwired: 1 in, 1 out]
        n166 = call "Object Detection SubVI v2.vi"("Error In"=w4744, "Mode"=w4745, "Image Dest"=w4746, "Image in"=w4747) -> ("Error out"=w4743:errorcluster, "Object Center Coordinates"=w4742:cluster{"x":sgl, "y":sgl}, "Object detection cluster"=w4741:T46)  [unwired: 1 out]
        n167 = Unbundle By Name(w4741) -> ("Object detected?"=w4752:bool)
        n168 = Unbundle By Name(w4742) -> ("x"=w4754:sgl, "y"=w4753:sgl)
        n169 = Bundle By Name(cluster=w4756, "Recognized Object"=w4752, "Object X coordinate"=w4754, "Object Y coordinate"=w4753) -> (w4755:T11)
      }
      frame "COLOUR PROCESSING" {
        # ">>> Box Colour Detection >>>"
        # ">>> Box Colour Detection >>>"
        # ">>> Line Sensor Cluster>>>"
        # ">>> IR Sensors >>>"
        # ">> Item Selection Bias >>"
        # ">> Item Selection Bias >>"
        # ">>State Logic  >>"
        # ">>> Time cluster >>>"
        # ">>> Yaw >>>"
        # ">>> Stepper position >>>"
        # ">>> Encoders >>>"
        # ">>> Object detection >>>"
        # ">>> Ultrasonic Sensors Detect >>>"
        n170 = call "Webcam AE.vi"("Camera states"=Webcam_AE."Retrieve Image") -> ("error out"=w4774:errorcluster, "Image Out"=w4775:T45)  [unwired: 2 in, 1 out]
        n171 = call "Box Colour Detection SubVI.vi"("Image In"=w4775, "Error In"=w4774) -> ("Colour output boolean cluster"=w4772:T47, "Error out"=w4773:errorcluster)  [unwired: 1 out]
        n172 = Unbundle By Name(w4772) -> ("Red"=w4770:bool, "Black"=w4769:bool, "Blue"=w4768:bool, "Yellow"=w4767:bool, "Green"=w4766:bool, "No recognizable coolour"=w4765:bool)
        n173 = Bundle By Name(cluster=w4771, "Red"=w4770, "Black"=w4769, "Blue"=w4768, "Yellow"=w4767, "Green"=w4766, "Unknown"=w4765) -> (w4764:T1)
      }
      frame "DISPOSE CAM BUFFERS" {
        # ">> Item Selection Bias >>"
        # ">>> Line Sensor Cluster>>>"
        # ">>> IR Sensors >>>"
        # ">>State Logic  >>"
        # ">>> Time cluster >>>"
        # ">>> Yaw >>>"
        # ">>> Stepper position >>>"
        # ">>> Encoders >>>"
        # ">>> Object detection >>>"
        # ">>> Ultrasonic Sensors Detect >>>"
        n174 = call "Webcam AE.vi"("Camera states"=Webcam_AE."Dispose Camera Image Buffer") -> ()  [unwired: 2 in, 3 out]
      }
      frame "DISPOSE PROC BUFFERS" {
        # ">>> Box Colour Detection >>>"
        # ">>> Line Sensor Cluster>>>"
        # ">>State Logic  >>"
        # ">>> IR Sensors >>>"
        # ">>> Time cluster >>>"
        # ">>> Object detection >>>"
        # ">>> Yaw >>>"
        # ">>> Ultrasonic Sensors Detect >>>"
        # ">>> Encoders >>>"
        # ">>> Stepper position >>>"
        n175 = call "IMAQ Reference AE.vi"("IMAQ AE States"=IMAQ_Reference_AE."Dispose Processing Buffer") -> ()  [unwired: 1 in, 2 out]
      }
      frame "BOX COLOUR" {
        # ">>> Box Colour Detection >>>"
        # ">>> Line Sensor Cluster>>>"
        # ">>State Logic  >>"
        # ">>> IR Sensors >>>"
        # ">>> Time cluster >>>"
        # ">>> Object detection >>>"
        # ">>> Yaw >>>"
        # ">>> Ultrasonic Sensors Detect >>>"
        # ">>> Encoders >>>"
        # ">>> Stepper position >>>"
        n176 = call "Box Colour Detection Sequence.vi"() -> ("Colour scan time out?"=w4827:bool, "Colour output boolean cluster"=w4829:T47)  [unwired: 9 in, 1 out]
        n177 = Unbundle By Name(w4829) -> ("Red"=w4826:bool, "Black"=w4822:bool, "Blue"=w4819:bool, "Yellow"=w4818:bool, "Green"=w4815:bool, "No recognizable coolour"=w4828:bool)
        n178 = Select(t=Box_Colour_FGV_Colours."Green" ("Colour"), s=w4815, f=Box_Colour_FGV_Colours."None" ("Colour")) -> (s? t:f=w4813:T2)
        n179 = Select(t=Box_Colour_FGV_Colours."Yellow" ("Colour"), s=w4818, f=w4813) -> (s? t:f=w4812:T2)
        n180 = Select(t=Box_Colour_FGV_Colours."Blue" ("Colour"), s=w4819, f=w4812) -> (s? t:f=w4821:T2)
        n181 = Select(t=Box_Colour_FGV_Colours."Black" ("Colour"), s=w4822, f=w4821) -> (s? t:f=w4824:T2)
        n182 = Select(t=Box_Colour_FGV_Colours."Red" ("Colour"), s=w4826, f=w4824) -> (s? t:f=w4811:T2)
        n183 = Bundle By Name(cluster=w4831, "Red"=w4826, "Black"=w4822, "Blue"=w4819, "Yellow"=w4818, "Green"=w4815, "Unknown"=w4828, "Image processing done"=w4827, "Colour"=w4811) -> (w4830:T1)
      }
      frame "-----ARM ACTIONS-----" {
      }
      frame "CLOSE CLAW" {
        n184 = call "Servo State FGV.vi"("Init/Read/Write State"=States_for_Action_Engine."Write", "Servo State"=Servo_States_FGV_Enum."Close claw") -> ()  [unwired: 1 in, 2 out]
      }
      frame "OPEN CLAW" {
        n185 = call "Servo State FGV.vi"("Init/Read/Write State"=States_for_Action_Engine."Write", "Servo State"=Servo_States_FGV_Enum."Open Claw") -> ()  [unwired: 1 in, 2 out]
      }
      frame "Z STEPPER CAM HEIGHT" {
        n186 = call "Arduino Interfacing VI.vi"("Data to Write"=I2C_MASTER_WRITE_NEW_Type_Def."zStepper 6k", "AE Mode"=Arduino_Interfacing."Write to Arduino") -> ()  [unwired: 2 in, 2 out]
      }
      frame "Z STEPPER GRAB HEIGHT" {
        # ">>State Logic  >>"
        # ">>> Time cluster >>>"
        # ">>> Yaw >>>"
        # ">>> Stepper position >>>"
        # ">>> Encoders >>>"
        # ">>> Object detection >>>"
        # ">>> Ultrasonic Sensors Detect >>>"
        n187 = call "Arduino Interfacing VI.vi"("Data to Write"=I2C_MASTER_WRITE_NEW_Type_Def."zStepper 100", "AE Mode"=Arduino_Interfacing."Write to Arduino") -> ()  [unwired: 2 in, 2 out]
      }
      frame "Z STEPPER BOX HEIGHT" {
        # ">>> IR Sensors >>>"
        # ">>> Time cluster >>>"
        # ">>> Yaw >>>"
        # ">>> Stepper position >>>"
        # ">>> Encoders >>>"
        # ">>> Object detection >>>"
        # ">>> Ultrasonic Sensors Detect >>>"
        n188 = call "Arduino Interfacing VI.vi"("Data to Write"=I2C_MASTER_WRITE_NEW_Type_Def."zStepper 4k", "AE Mode"=Arduino_Interfacing."Write to Arduino") -> ()  [unwired: 2 in, 2 out]
      }
      frame "Z STEPPER DROP HEIGHT" {
        # ">>> IR Sensors >>>"
        # ">>> Time cluster >>>"
        # ">>> Yaw >>>"
        # ">>> Stepper position >>>"
        # ">>> Encoders >>>"
        # ">>> Object detection >>>"
        # ">>> Ultrasonic Sensors Detect >>>"
        n189 = call "Arduino Interfacing VI.vi"("Data to Write"=I2C_MASTER_WRITE_NEW_Type_Def."zStepper 13.3k", "AE Mode"=Arduino_Interfacing."Write to Arduino") -> ()  [unwired: 2 in, 2 out]
      }
      frame "Y STEPPER CONTROL" {
        # ">>State Logic  >>"
        # ">>> yStepper command>>>"
        # ">>> Time cluster >>>"
        # ">>> Yaw >>>"
        # ">>> Stepper position >>>"
        # ">>> Encoders >>>"
        # ">>> Object detection >>>"
        # ">>> Ultrasonic Sensors Detect >>>"
        n190 = Unbundle By Name(w4936) -> ("yStepper desired"=w4935:u8)
        n191 = call "Arduino Interfacing VI.vi"("y Stepper value"=w4935, "Data to Write"=I2C_MASTER_WRITE_NEW_Type_Def."yStepper control", "AE Mode"=Arduino_Interfacing."Write to Arduino") -> ()  [unwired: 1 in, 2 out]
      }
      frame "READ STEPPER VALUES" {
        # ">>State Logic  >>"
        # ">>> Time cluster >>>"
        # ">>> Yaw >>>"
        # ">>> Stepper position >>>"
        # ">>> Encoders >>>"
        # ">>> Object detection >>>"
        # ">>> Ultrasonic Sensors Detect >>>"
        n192 = call "Arduino Interfacing VI.vi"("AE Mode"=Arduino_Interfacing."Read From Arduino") -> ("Arduino Data"=w4954:T17)  [unwired: 3 in, 1 out]
        n193 = Unbundle By Name(w4954) -> ("y Stepper Position"=w4953:u8, "z Stepper Position"=w4952:u8)
        n194 = Bundle By Name(cluster=w4957, "y Stepper Position"=w4953, "z Stepper Position"=w4952) -> (w4956:T7)
      }
      frame " -----TIMING-----" {
        # ">>State Logic  >>"
        # ">>> Time cluster >>>"
        # ">>> Yaw >>>"
        # ">>> Stepper position >>>"
        # ">>> Encoders >>>"
        # ">>> Object detection >>>"
        # ">>> Ultrasonic Sensors Detect >>>"
      }
      frame "SET TIMER 1" {
        w4973 = 1.0 ("Time Setting")
        # ">>State Logic  >>"
        # ">>> Time cluster >>>"
        # ">>> Yaw >>>"
        # ">>> Stepper position >>>"
        # ">>> Encoders >>>"
        # ">>> Object detection >>>"
        # ">>> Ultrasonic Sensors Detect >>>"
        n195 = Wait (ms)(milliseconds to wait=u32 250) -> ()  [unwired: 1 out]
        n196 = call "Elasped Timer.vi"("Time Setting"=w4973, "Action"=Elapsed_timer_control."Initialize") -> ()  [unwired: 6 in, 4 out]
        n197 = Bundle By Name(cluster=w4982, "Time up flag"=FALSE, "SET TIME TO CHECK"=w4973) -> (w4980:T3)
      }
      frame "SET TIMER 2" {
        w4989 = 2.0 ("Time Setting")
        # ">>State Logic  >>"
        # ">>> Time cluster >>>"
        # ">>> Yaw >>>"
        # ">>> Stepper position >>>"
        # ">>> Encoders >>>"
        # ">>> Object detection >>>"
        # ">>> Ultrasonic Sensors Detect >>>"
        n198 = Wait (ms)(milliseconds to wait=u32 250) -> ()  [unwired: 1 out]
        n199 = call "Elasped Timer.vi"("Time Setting"=w4989, "Action"=Elapsed_timer_control."Initialize") -> ()  [unwired: 6 in, 4 out]
        n200 = Bundle By Name(cluster=w4998, "Time up flag"=FALSE, "SET TIME TO CHECK"=w4989) -> (w4996:T3)
      }
      frame "SET TIMER 3" {
        w5005 = 3.0 ("Time Setting")
        # ">>State Logic  >>"
        # ">>> Time cluster >>>"
        # ">>> Yaw >>>"
        # ">>> Stepper position >>>"
        # ">>> Encoders >>>"
        # ">>> Object detection >>>"
        # ">>> Ultrasonic Sensors Detect >>>"
        n201 = Wait (ms)(milliseconds to wait=u32 250) -> ()  [unwired: 1 out]
        n202 = call "Elasped Timer.vi"("Time Setting"=w5005, "Action"=Elapsed_timer_control."Initialize") -> ()  [unwired: 6 in, 4 out]
        n203 = Bundle By Name(cluster=w5014, "Time up flag"=FALSE, "SET TIME TO CHECK"=w5005) -> (w5012:T3)
      }
      frame "SET TIMER 4" {
        w5021 = 4.0 ("Time Setting")
        # ">>State Logic  >>"
        # ">>> Time cluster >>>"
        # ">>> Yaw >>>"
        # ">>> Stepper position >>>"
        # ">>> Encoders >>>"
        # ">>> Object detection >>>"
        # ">>> Ultrasonic Sensors Detect >>>"
        n204 = call "Elasped Timer.vi"("Time Setting"=w5021, "Action"=Elapsed_timer_control."Initialize") -> ()  [unwired: 6 in, 4 out]
        n205 = Wait (ms)(milliseconds to wait=u32 250) -> ()  [unwired: 1 out]
        n206 = Bundle By Name(cluster=w5030, "Time up flag"=FALSE, "SET TIME TO CHECK"=w5021) -> (w5028:T3)
      }
      frame "SET TIMER 5" {
        w5038 = 5.0 ("Time Setting")
        # ">>State Logic  >>"
        # ">>> Time cluster >>>"
        # ">>> Yaw >>>"
        # ">>> Stepper position >>>"
        # ">>> Encoders >>>"
        # ">>> Object detection >>>"
        # ">>> Ultrasonic Sensors Detect >>>"
        n207 = call "Elasped Timer.vi"("Time Setting"=w5038, "Action"=Elapsed_timer_control."Initialize") -> ("Time Out?!"=w5037:bool)  [unwired: 6 in, 3 out]
        n208 = Wait (ms)(milliseconds to wait=u32 250) -> ()  [unwired: 1 out]
        n209 = Bundle By Name(cluster=w5046, "Time up flag"=w5037, "SET TIME TO CHECK"=w5038) -> (w5045:T3)
      }
      frame "START TIMER" {
        # ">>State Logic  >>"
        # ">>> Time cluster >>>"
        # ">>> Yaw >>>"
        # ">>> Stepper position >>>"
        # ">>> Encoders >>>"
        # ">>> Object detection >>>"
        # ">>> Ultrasonic Sensors Detect >>>"
        n210 = call "Elasped Timer.vi"("Action"=Elapsed_timer_control."Start") -> ("Time Out?!"=w5057:bool)  [unwired: 7 in, 3 out]
        n211 = Bundle By Name(cluster=w5060, "Time up flag"=w5057) -> (w5059:T3)
      }
      frame "-----MISC-----" {
        # ">>> Box Colour Detection >>>"
        # ">>> Line Sensor Cluster>>>"
        # ">>> IR Sensors >>>"
        # ">>> Time cluster >>>"
        # ">>> Object detection >>>"
        # ">>> Yaw >>>"
        # ">>> Ultrasonic Sensors Detect >>>"
        # ">>> Encoders >>>"
        # ">>> Stepper position >>>"
      }
      frame "Task 9" {
        # ">>> Box Colour Detection >>>"
        # ">>> Line Sensor Cluster>>>"
        # ">>> IR Sensors >>>"
        # ">>> Time cluster >>>"
        # ">>> Object detection >>>"
        # ">>> Yaw >>>"
        # ">>> Ultrasonic Sensors Detect >>>"
        # ">>> Encoders >>>"
        # ">>> Stepper position >>>"
        n212 = call "Colour Processing Test Env.vi"() -> ("Colour scan time out?"=w5086:bool, "Colour output boolean cluster"=w5084:T47)  [unwired: 10 in]
        n213 = Unbundle By Name(w5084) -> ("Red"=w5078:bool, "Black"=w5079:bool, "Blue"=w5080:bool, "Yellow"=w5081:bool, "Green"=w5082:bool, "No recognizable coolour"=w5083:bool)
        n214 = Bundle By Name(cluster=w5088, "Red"=w5078, "Black"=w5079, "Blue"=w5080, "Yellow"=w5081, "Green"=w5082, "Unknown"=w5083, "Image processing done"=w5086) -> (w5087:T1)
      }
    }
    "State Logic" <- w263
    "Image Processing Error" <- w231
    n215 = call "Task Enable FGV.vi"("Init/Read/Write State"=States_for_Action_Engine."Read") -> ("Output node"=w219:bool)  [unwired: 9 in, 1 out]
    n216 = Not(x=w219) -> (.not. x?=w257:bool)
    n217 = case shown="True" w264 {
      tunnel: w222 -> [w295 w349]
      tunnel: w271 -> [w291 w351]
      tunnel: [w295 w349] -> w276
      tunnel: [w291 w352] -> w275
      tunnel: w272 -> [_ w347]
      tunnel: w274 -> [_ w348]
      tunnel: w269 -> [w294 w354]
      tunnel: [w294 w354] -> w268
      tunnel: "STOP TASK" -> [_ w337]
      tunnel: w263 -> [w293 w353]
      tunnel: [w293 w350] -> w262
      tunnel: w259 -> [w292 w343]
      tunnel: [w292 w343] -> w258
      tunnel: w257 -> [_ w338]
      tunnel: [w290 w335] -> w256
      tunnel: w255 -> [w290 w334]
      tunnel: w253 -> [w289 w331]
      tunnel: [w289 w331] -> w252
      tunnel: w250 -> [w288 w327]
      tunnel: [w288 w327] -> w249
      tunnel: w247 -> [w287 w325]
      tunnel: [w287 w325] -> w246
      tunnel: w244 -> [w286 w323]
      tunnel: [w286 w323] -> w243
      tunnel: w242 -> [w285 w322]
      tunnel: [w285 w321] -> w241
      tunnel: [_ w319] -> w240
      tunnel: w238 -> [w284 w317]
      tunnel: [w284 w317] -> w237
      tunnel: w236 -> [w283 w316]
      tunnel: [w283 w315] -> w235
      tunnel: w233 -> [w282 w312]
      tunnel: [w282 w312] -> w232
      tunnel: [w281 w311] -> w230
      tunnel: w228 -> [w281 w310]
      tunnel: [_ w308] -> w227
      tunnel: [_ w307] -> w226
      tunnel: [_ w306] -> w225
      tunnel: w223 -> [w280 w305]
      tunnel: [w280 w305] -> w221
      tunnel: [_ w296] -> w218
      frame False {
        # ">>> Box Colour Detection >>>"
        # ">>> Line Sensor Cluster>>>"
        # ">> Item Selection Bias >>"
        # ">>State Logic Queue Reference >>"
        # ">>Action states Queue Reference >>"
        # ">>True Stop Next State >>"
        # ">>State Logic  >>"
        # ">>> IR Sensors >>>"
        # ">>> Line Sensor Cluster>>>"
        # ">>> Line Sensor Cluster>>>"
        # ">>> Motor control cluster >>>"
        # ">>> yStepper command>>>"
        # ">>> Motor control cluster >>>"
        # ">>> yStepper command>>>"
        # ">>> Motor control cluster >>>"
        # ">>> IR Sensors >>>"
        # ">>> IR Sensors >>>"
        # ">>> yStepper command>>>"
        # ">>> Time cluster >>>"
        # ">>> Yaw >>>"
        # ">>> Stepper position >>>"
        # ">>> Encoders >>>"
        # ">>> Object detection >>>"
        # ">>> Ultrasonic Sensors Detect >>>"
        # ">>> Time cluster >>>"
        # ">>> Yaw >>>"
        # ">>> Stepper position >>>"
        # ">>> Encoders >>>"
        # ">>> Object detection >>>"
        # ">>> Ultrasonic Sensors Detect >>>"
      }
      frame True {
        # ">>> Box colour cluster >>>"
        # ">>State Logic Queue Reference >>"
        # ">>> Box Colour Detection >>>"
        # ">> Item Selection Bias >>"
        # ">>> IR Sensors >>>"
        # ">>> Line Sensor Cluster>>>"
        # ">>> Line Sensor Cluster>>>"
        # ">>> Motor control cluster >>>"
        # ">>> yStepper command>>>"
        # ">>> IR Sensors >>>"
        # ">>> Motor control cluster >>>"
        # ">>State Logic Queue Reference >>"
        # ">>Timeout>>"
        # ">>> yStepper command>>>"
        # ">>> Time cluster >>>"
        # ">>> Object detection >>>"
        # ">>> Yaw >>>"
        # ">>> Ultrasonic Sensors Detect >>>"
        # ">>> Encoders >>>"
        # ">>> Stepper position >>>"
        # ">>State Logic  >>"
        # ">>True Stop Next State >>"
        # ">>Action Queue>>"
        # ">> Manual override >>"
        # ">>> Time cluster >>>"
        # ">>> Yaw >>>"
        # ">>> Stepper position >>>"
        # ">>> Encoders >>>"
        # ">>> Object detection >>>"
        # ">>> Ultrasonic Sensors Detect >>>"
        # ">>Action Queue>>"
        # ">>State Logic Queue Reference >>"
        n218 = Or(x=w337, y=w338) -> (x .or. y?=w336:bool)
        n219 = Unbundle By Name(w305) -> ("Red"=w304:bool, "Black"=w303:bool, "Blue"=w302:bool, "Yellow"=w301:bool, "Green"=w300:bool, "Unknown"=w299:bool, "Image processing done"=w298:bool, "Colour"=w297:T2)
        n220 = Unbundle By Name(w312) -> ("Line Detected?"=w313:bool)
        n221 = Unbundle By Name(w317) -> ("Left IR Sensor"=w318:dbl, "Arm IR Sensor"=w314:dbl, "Bottom IR Sensor"=w309:dbl)
        n222 = Unbundle By Name(w323) -> ("Time up flag"=w324:bool)
        n223 = Unbundle By Name(w325) -> ("Yaw"=w326:dbl, "Compass"=w320:dbl)
        n224 = Unbundle By Name(w327) -> ("y Stepper Position"=w329:u8, "z Stepper Position"=w328:u8)
        n225 = Unbundle By Name(w343) -> ("xDistance"=w340:dbl, "yDistance"=w341:dbl, "wDistance"=w342:dbl)
        n226 = Unbundle By Name(w331) -> ("Recognized Object"=w330:bool, "Object X coordinate"=w333:dbl, "Object Y coordinate"=w332:dbl)
        n227 = Unbundle By Name(w354) -> ("PING_A"=w346:u8, "PING_B"=w345:u8, "PING_C"=w344:u8, "PING_D"=w339:u8)
        n228 = case shown="\"Task A12: EXTEND ARM\"" w353 {
          tunnel: [w359 w371 w381 w389 w400 w520 w537 w583 w621 w675 w717 w766 w809 w864 w912 w956 w1016 w1057 w1100 w1149 w1189 w1242 w1280 w1332 w1378 w1424 w1465 w1514 w1558 w1604 w1645 w1694 w1738 w1784 w1825 w1874 w1918 w1964 w2005 w2054 w2089 w2107 w2155 w2196 w2246 w2303 w2342 w2391 w2434 w2487 w2525 w2577 w2620 w2665 w2700 w2748 w2791 w2845 w2893 w2936 w2989 w3030 w3086 w3127 w3179 w3227 w3276 w3319 w3363 w3411 w3462 w3505 w3554 w3602 w3645 w3691 w3739 w3785 w3827 w3878 w3917 w3965 w4018 w4059 w4104] -> w352
          tunnel: w351 -> [w359 w374 w381 w390 w403 w522 w538 w584 w630 w673 w721 w767 w815 w857 w915 w963 w1006 w1060 w1106 w1148 w1192 w1232 w1286 w1322 w1373 w1416 w1464 w1513 w1557 w1596 w1644 w1693 w1737 w1776 w1824 w1873 w1917 w1956 w2004 w2053 w2089 w2097 w2158 w2202 w2245 w2302 w2348 w2390 w2437 w2477 w2531 w2567 w2613 w2658 w2704 w2755 w2796 w2850 w2900 w2942 w2987 w3031 w3084 w3128 w3180 w3229 w3283 w3325 w3370 w3416 w3461 w3501 w3558 w3609 w3650 w3696 w3740 w3786 w3831 w3876 w3921 w3972 w4008 w4062 w4110]
          tunnel: [State_Type_Definitions,_for_0.26g_versions_and_later_3."Idle" ("Enum") State_Type_Definitions,_for_0.26g_versions_and_later_3."Idle" ("Enum") _ w385 w402 State_Type_Definitions,_for_0.26g_versions_and_later_3."Shutdown" ("Enum") w539 w585 w628 w676 w718 w765 w810 w863 w913 w958 w1015 w1058 w1107 w1150 w1191 w1241 w1287 w1331 w1379 w1417 w1466 w1515 w1559 w1597 w1646 w1695 w1739 w1777 w1826 w1875 w1919 w1957 w2006 w2055 State_Type_Definitions,_for_0.26g_versions_and_later_3."Idle" ("Enum") w2106 w2156 w2203 w2247 w2304 w2349 w2392 w2436 w2486 w2532 w2576 w2619 w2664 w2701 w2749 w2792 w2846 w2894 w2935 w2990 w3029 w3087 w3126 w3178 w3228 w3277 w3318 w3365 w3417 w3463 w3504 w3555 w3603 w3646 w3692 w3738 w3784 w3828 w3879 w3918 w3966 w4017 w4061 w4111] -> w350
          tunnel: w349 -> [_ _ _ w388 w406 _ w543 w590 w624 w672 w722 w773 w814 w861 w916 w962 w1013 w1055 w1105 w1146 w1193 w1239 w1285 w1329 w1376 w1423 w1462 w1511 w1555 w1603 w1642 w1691 w1735 w1783 w1822 w1871 w1915 w1963 w2002 w2051 _ w2104 w2153 w2201 w2243 w2300 w2347 w2388 w2438 w2484 w2530 w2574 w2617 w2662 w2708 w2754 w2799 w2853 w2899 w2941 w2986 w3039 w3083 w3129 w3173 w3230 w3282 w3324 w3369 w3415 w3460 w3510 w3562 w3608 w3653 w3699 w3733 w3779 w3832 w3875 w3922 w3971 w4015 w4063 w4109]
          tunnel: w348 -> [_ _ _ _ w405 _ w542 w589 w623 w671 w723 w772 w813 w860 w909 w961 w1012 w1054 w1104 w1145 w1194 w1238 w1284 w1328 w1375 w1421 w1461 w1510 w1554 w1601 w1641 w1690 w1734 w1781 w1821 w1870 w1914 w1961 w2001 w2050 _ w2103 w2152 w2200 w2242 w2299 w2346 w2387 w2439 w2483 w2529 w2573 w2616 w2661 w2703 w2753 w2798 w2852 w2898 w2940 w2985 w3037 w3082 w3130 w3174 w3231 w3281 w3323 w3368 w3414 w3459 w3509 w3557 w3607 w3652 w3698 w3734 w3780 w3833 w3874 w3923 w3970 w4014 w4064 w4108]
          tunnel: w347 -> [_ _ _ w387 w401 _ w541 w588 w622 w670 w724 w771 w812 w859 w908 w960 w1014 w1056 w1103 w1144 w1195 w1240 w1283 w1330 w1374 w1422 w1460 w1509 w1553 w1602 w1640 w1689 w1733 w1782 w1820 w1869 w1913 w1962 w2000 w2049 _ w2105 w2154 w2199 w2241 w2298 w2345 w2386 w2440 w2485 w2528 w2575 w2618 w2663 w2707 w2752 w2797 w2851 w2897 w2939 w2984 w3038 w3081 w3131 w3175 w3232 w3280 w3322 w3367 w3413 w3458 w3508 w3561 w3606 w3651 w3697 w3735 w3781 w3834 w3873 w3924 w3969 w4016 w4065 w4107]
          tunnel: w336 -> [_ _ _ _ _ _ w528 w582 w629 w669 w725 w768 w808 w862 w914 w964 w1007 w1061 w1101 w1147 w1196 w1233 w1281 w1323 w1377 w1419 w1463 w1512 w1556 w1599 w1643 w1692 w1736 w1779 w1823 w1872 w1916 w1959 w2003 w2052 _ w2098 w2159 w2197 w2244 w2301 w2343 w2389 w2441 w2478 w2526 w2568 w2614 w2659 w2706 w2747 w2795 w2849 w2892 w2938 w2983 w3033 w3080 w3132 w3176 w3233 w3275 w3321 w3366 w3412 w3457 w3507 w3560 w3601 w3649 w3695 w3736 w3782 w3835 w3872 w3925 w3964 w4009 w4066 w4105]
          tunnel: w346 -> [_ _ _ _ _ _ _ _ _ _ _ _ _ _ _ _ _ _ _ _ _ _ _ _ _ _ _ _ _ _ _ _ _ _ _ _ _ _ _ _ _ _ _ _ _ _ _ _ _ _ _ _ _ _ _ _ _ _ _ _ _ _ _ _ _ _ _ _ _ _ _ _ _ _ _ _ _ _ _ _ _ _ _ _ _]
          tunnel: w345 -> [_ _ _ _ _ _ _ _ _ w668 _ _ _ w853 w897 w954 _ _ _ _ _ _ _ _ _ _ _ _ _ _ _ _ _ _ _ _ _ _ _ _ _ _ w2145 _ _ _ _ _ _ _ _ _ _ _ _ _ _ _ _ _ _ _ _ _ _ _ _ _ _ _ _ _ _ _ _ _ _ _ _ _ _ _ _ _ _]
          tunnel: w344 -> [_ _ _ _ _ _ _ _ _ w667 _ _ _ w854 w898 w955 _ _ _ _ _ _ _ _ _ _ _ _ _ _ _ _ _ _ _ _ _ _ _ _ _ _ w2146 _ _ _ _ _ _ _ _ _ _ _ _ _ _ _ _ _ _ _ _ _ _ _ _ _ _ _ _ _ _ _ _ _ _ _ _ _ _ _ _ _ _]
          tunnel: w342 -> [_ _ _ _ _ _ _ _ _ _ _ w770 _ _ _ _ _ _ _ _ _ _ _ _ _ _ _ _ _ _ _ _ _ _ _ _ _ _ _ _ _ _ _ _ _ _ _ _ _ _ _ _ _ _ _ _ _ _ _ _ _ _ _ _ w3172 _ _ _ _ _ _ _ _ _ _ _ _ w3778 _ _ _ _ _ _ _]
          tunnel: w341 -> [_ _ _ _ _ _ w536 w581 _ _ w716 _ _ _ _ w959 _ _ _ _ _ _ _ _ _ _ _ _ _ _ _ _ _ _ _ w1862 _ _ _ w2042 _ _ _ _ _ _ _ _ _ _ _ _ _ _ _ _ _ w2836 _ _ _ _ _ _ _ _ _ _ _ _ _ _ _ _ _ w3688 _ _ w3822 _ w3916 _ _ _ _]
          tunnel: w340 -> [_ _ _ _ _ _ _ _ _ _ _ _ _ _ w903 _ _ _ _ _ _ _ _ _ _ _ _ w1502 _ _ _ w1682 _ _ _ _ _ _ _ _ _ _ _ _ _ w2289 _ _ _ _ _ _ _ w2651 _ _ _ _ _ _ _ _ w3073 _ _ _ _ _ _ _ _ _ _ _ _ _ _ _ _ _ _ _ _ _ _]
          tunnel: w339 -> [_ _ _ _ _ _ _ _ _ _ _ _ _ _ _ _ _ _ _ _ _ _ _ _ _ _ _ _ _ _ _ _ _ _ _ _ _ _ _ _ _ _ _ _ _ _ _ _ _ _ _ _ _ _ _ _ _ _ _ _ _ _ _ _ _ _ _ _ _ _ _ _ _ _ _ _ _ _ _ _ _ _ _ _ _]
          tunnel: [State_Type_Definitions,_for_0.26g_versions_and_later_3."Idle" ("Enum") State_Type_Definitions,_for_0.26g_versions_and_later_3."Idle" ("Enum") _ State_Type_Definitions,_for_0.26g_versions_and_later_3."Idle" ("Enum") State_Type_Definitions,_for_0.26g_versions_and_later_3."Idle" ("Enum") State_Type_Definitions,_for_0.26g_versions_and_later_3."Shutdown" ("Enum") w534 w579 w627 w674 w719 w762 w807 w856 w911 w957 w1017 w1059 w1099 w1151 w1190 w1243 w1279 w1333 w1380 w1418 w1467 w1516 w1560 w1598 w1647 w1696 w1740 w1778 w1827 w1876 w1920 w1958 w2007 w2056 w2091 w2108 w2157 w2195 w2248 w2305 w2341 w2393 w2435 w2488 w2524 w2578 w2621 w2666 w2702 w2750 w2794 w2848 w2895 w2934 w2988 w3028 w3085 w3125 w3177 w3226 w3278 w3317 w3364 w3418 w3464 w3503 w3556 w3604 w3648 w3694 w3737 w3783 w3829 w3877 w3919 w3967 w4019 w4060 w4103] -> w335
          tunnel: w334 -> [_ _ _ w385 _ _ _ _ _ _ _ _ _ _ _ _ _ _ _ _ _ _ _ _ _ _ _ _ _ _ _ _ _ _ _ _ _ _ _ _ w2091 _ _ _ _ _ _ _ _ _ _ _ _ _ _ _ _ _ _ _ _ _ _ _ _ _ _ _ _ _ _ _ _ _ _ _ _ _ _ _ _ _ _ _ _]
          tunnel: w330 -> [_ _ _ _ _ _ _ _ _ _ _ _ _ _ _ _ _ _ _ _ _ _ _ _ _ _ w1454 _ _ _ w1634 _ _ _ w1814 _ _ _ w1994 _ _ _ _ _ w2236 _ _ _ _ _ _ _ _ _ _ _ _ _ _ _ _ _ _ _ _ _ _ _ _ _ _ _ _ _ _ _ _ _ _ _ _ _ _ _ _]
          tunnel: w333 -> [_ _ _ _ _ _ _ _ _ _ _ _ _ _ _ _ _ _ _ _ _ _ _ _ _ _ _ _ _ _ _ _ _ _ _ _ _ _ _ _ _ _ _ _ _ w2295 _ _ _ _ _ _ _ _ _ _ _ _ _ _ _ _ _ _ _ _ _ _ _ _ _ _ _ _ _ _ _ _ _ _ _ _ _ _ _]
          tunnel: w332 -> [_ _ _ _ _ _ _ _ _ _ _ _ _ _ _ _ _ _ _ _ _ _ _ _ _ _ _ _ _ _ _ _ _ _ _ _ _ _ _ _ _ _ _ _ _ _ _ _ w2430 _ _ _ _ _ _ _ _ _ _ _ _ _ _ _ _ _ _ _ _ _ _ _ _ _ _ _ _ _ _ _ _ _ _ _ _]
          tunnel: w329 -> [_ _ _ _ _ _ _ _ _ _ _ _ _ _ _ _ _ _ _ _ _ _ _ _ _ _ _ _ _ _ _ _ _ _ _ _ _ _ _ _ _ _ _ _ _ _ _ _ w2429 _ _ _ _ _ _ _ _ _ _ _ _ _ _ _ _ _ _ _ _ _ _ _ _ _ _ _ _ _ _ _ _ _ _ w4056 _]
          tunnel: w328 -> [_ _ _ _ _ _ _ _ w626 _ _ _ w805 _ _ _ w1010 _ w1095 _ w1185 w1236 _ w1326 w1372 _ _ _ _ _ _ _ _ _ _ _ _ _ _ _ _ w2101 _ _ _ _ _ _ _ w2481 _ w2571 _ _ w2705 _ _ _ _ _ _ _ _ _ _ _ _ _ _ _ _ _ w3559 _ _ _ _ _ _ _ _ _ w4012 _ _]
          tunnel: w326 -> [_ _ _ _ _ _ _ _ _ _ _ _ _ _ _ _ _ _ _ _ _ _ _ _ _ _ _ _ _ _ _ _ _ _ _ _ _ _ _ _ _ _ _ _ _ _ _ _ _ _ _ _ _ _ _ _ _ _ _ _ _ _ _ _ _ _ _ _ _ _ _ _ _ _ _ _ _ _ _ _ _ _ _ _ _]
          tunnel: w324 -> [_ _ _ _ _ _ _ _ _ _ _ _ _ _ _ _ _ _ _ w1141 _ _ w1277 _ _ w1412 w1455 _ _ w1592 w1635 _ _ w1772 w1815 _ _ w1952 w1995 _ _ _ _ w2193 w2235 _ w2339 w2383 _ _ w2522 _ _ _ _ _ _ _ _ _ _ _ _ _ _ _ _ _ _ _ _ _ _ _ _ _ w3732 _ _ _ _ _ _ _ w4101]
          tunnel: w322 -> [w357 w369 w380 w384 w398 w518 w533 w578 w625 w666 w720 w761 w806 w855 w907 w953 w1005 w1052 w1098 w1142 w1186 w1231 w1278 w1321 w1370 w1415 w1458 w1507 w1551 w1595 w1638 w1687 w1731 w1775 w1818 w1867 w1911 w1955 w1998 w2047 w2092 w2096 w2150 w2194 w2239 w2296 w2340 w2384 w2432 w2476 w2523 w2566 w2612 w2657 w2699 w2751 w2793 w2847 w2896 w2946 w2982 w3036 w3079 w3134 w3182 w3235 w3279 w3329 w3372 w3420 w3466 w3515 w3553 w3605 w3647 w3693 w3742 w3788 w3830 w3871 w3920 w3968 w4007 w4058 w4102]
          tunnel: [w357 w368 w380 w384 w398 w518 w533 w578 w625 w666 w720 w761 w806 w855 w907 w953 w1005 w1052 w1098 w1142 w1186 w1231 w1278 w1321 w1370 w1415 w1458 w1507 w1551 w1595 w1638 w1687 w1731 w1775 w1818 w1867 w1911 w1955 w1998 w2047 w2092 w2096 w2150 w2194 w2239 w2296 w2340 w2384 w2431 w2476 w2523 w2566 w2612 w2657 w2699 w2751 w2793 w2847 w2896 w2946 w2982 w3036 w3079 w3134 w3182 w3235 w3279 w3329 w3372 w3420 w3466 w3515 w3553 w3605 w3647 w3693 w3742 w3788 w3830 w3871 w3920 w3968 w4007 w4057 w4102] -> w321
          tunnel: w320 -> [_ _ _ _ _ _ _ _ _ _ _ _ _ _ _ _ _ _ _ _ _ _ _ _ _ _ _ _ _ _ _ _ _ _ _ _ _ _ _ _ _ _ _ _ _ _ _ _ _ _ _ _ _ _ _ w2746 _ _ w2891 _ _ _ _ _ _ _ w3274 _ _ _ _ _ _ w3600 _ _ _ _ _ _ _ w3963 _ _ _]
          tunnel: [_ _ _ _ TRUE _ w527 w575 w618 w663 w712 w758 w801 _ _ _ _ _ _ _ _ _ _ _ w1366 _ w1455 _ _ _ w1635 _ _ _ w1815 _ _ _ w1995 _ _ _ _ _ w2235 w2285 _ _ _ _ _ _ _ _ w2696 w2741 w2788 w2837 w2886 _ w2979 w3023 w3072 w3120 w3170 w3217 w3269 _ _ _ w3456 w3500 w3550 w3595 w3642 _ w3732 w3776 w3823 w3868 w3912 w3958 _ _ _] -> w319
          tunnel: w318 -> [_ _ _ _ _ _ _ _ _ _ _ _ _ _ _ _ _ _ _ _ _ _ _ _ _ _ _ _ _ _ _ _ _ _ _ _ _ _ _ _ _ _ _ _ _ _ _ _ _ _ _ _ _ _ _ _ _ _ _ w2933 _ _ _ _ _ _ _ w3316 _ _ _ _ _ _ _ _ _ _ _ _ _ _ _ _ _]
          tunnel: w316 -> [w356 w366 w379 w383 w396 w517 w532 w577 w620 w665 w714 w760 w803 w848 w896 w952 w1004 w1051 w1097 w1140 w1188 w1230 w1276 w1320 w1369 w1414 w1457 w1506 w1550 w1594 w1637 w1686 w1730 w1774 w1817 w1866 w1910 w1954 w1997 w2046 w2093 w2095 w2144 w2192 w2238 w2292 w2338 w2382 w2426 w2475 w2521 w2565 w2611 w2656 w2698 w2743 w2790 w2844 w2888 w2947 w2981 w3035 w3078 w3136 w3184 w3237 w3271 w3330 w3374 w3422 w3468 w3516 w3552 w3597 w3644 w3690 w3744 w3790 w3825 w3870 w3914 w3960 w4006 w4053 w4100]
          tunnel: [w356 w365 w379 w383 w396 w517 w532 w577 w620 w665 w714 w760 w803 w848 w896 w952 w1004 w1051 w1097 w1140 w1188 w1230 w1276 w1320 w1369 w1414 w1457 w1506 w1550 w1594 w1637 w1686 w1730 w1774 w1817 w1866 w1910 w1954 w1997 w2046 w2093 w2095 w2144 w2192 w2238 w2291 w2338 w2382 w2426 w2475 w2521 w2565 w2611 w2656 w2698 w2743 w2790 w2844 w2888 w2947 w2981 w3035 w3078 w3136 w3184 w3237 w3271 w3330 w3374 w3422 w3468 w3516 w3552 w3597 w3644 w3690 w3744 w3790 w3825 w3870 w3914 w3960 w4006 w4053 w4100] -> w315
          tunnel: w314 -> [_ _ _ _ _ _ _ _ _ _ _ _ _ _ _ _ _ _ _ _ _ _ _ _ _ _ _ _ _ _ _ _ _ _ _ _ _ _ _ _ _ _ _ _ _ _ _ _ _ _ _ _ _ _ _ _ _ w2842 _ _ _ _ _ _ _ w3224 _ _ _ _ _ _ _ _ _ _ _ _ _ _ _ _ _ _ _]
          tunnel: w313 -> [_ _ _ _ _ _ w529 _ _ _ _ _ _ _ _ w950 _ _ _ _ _ _ _ _ _ _ _ _ _ _ _ _ _ _ _ _ _ _ _ _ _ _ _ _ _ _ _ _ _ _ _ _ _ _ _ _ w2788 _ _ _ w2979 _ w3074 _ _ _ _ _ w3362 _ w3456 _ _ _ w3642 _ _ _ _ w3868 _ _ _ _ _]
          tunnel: [w355 w361 w378 w382 w395 w516 w531 w576 w619 w664 w713 w759 w802 w847 w895 w951 w1003 w1050 w1096 w1139 w1187 w1229 w1275 w1319 w1368 enum16{"Ball", "Soap", "Gel", "Pipe", "None"}."Ball" ("Object recognition mode") w1456 w1505 enum16{"Ball", "Soap", "Gel", "Pipe", "None"}."Soap" ("Object recognition mode") enum16{"Ball", "Soap", "Gel", "Pipe", "None"}."Soap" ("Object recognition mode") w1636 w1685 enum16{"Ball", "Soap", "Gel", "Pipe", "None"}."Gel" ("Object recognition mode") enum16{"Ball", "Soap", "Gel", "Pipe", "None"}."Gel" ("Object recognition mode") w1816 w1865 enum16{"Ball", "Soap", "Gel", "Pipe", "None"}."Pipe" ("Object recognition mode") enum16{"Ball", "Soap", "Gel", "Pipe", "None"}."Pipe" ("Object recognition mode") w1996 w2045 w2088 w2094 w2143 w2191 w2237 w2286 w2337 w2381 w2425 w2474 w2520 w2564 w2610 w2655 w2697 w2742 w2789 w2841 w2887 w2937 w2980 w3034 w3077 w3135 w3183 w3236 w3270 w3320 w3373 w3421 w3467 w3506 w3551 w3596 w3643 w3689 w3743 w3789 w3824 w3869 w3913 w3959 w4005 w4052 w4099] -> w311
          tunnel: w310 -> [w355 w361 w378 w382 _ w516 w531 w576 w619 w664 w713 w759 w802 w847 w895 w951 w1003 w1050 w1096 w1139 w1187 w1229 w1275 w1319 w1368 _ w1456 w1505 _ _ w1636 w1685 _ _ w1816 w1865 _ _ w1996 w2045 w2088 w2094 w2143 w2191 w2237 w2286 w2337 w2381 w2425 w2474 w2520 w2564 w2610 w2655 w2697 w2742 w2789 w2841 w2887 w2937 w2980 w3034 w3077 w3135 w3183 w3236 w3270 w3320 w3373 w3421 w3467 w3506 w3551 w3596 w3643 w3689 w3743 w3789 w3824 w3869 w3913 w3959 w4005 w4052 w4099]
          tunnel: w309 -> [_ _ _ _ _ _ _ _ _ _ _ _ _ _ _ _ _ _ _ _ _ _ _ _ _ _ _ _ _ _ _ _ _ _ _ _ _ _ _ _ _ _ w2142 _ _ _ _ _ _ _ _ _ _ _ _ _ _ w2840 _ _ _ _ _ _ _ w3218 _ _ _ _ _ _ _ _ _ _ _ _ _ _ _ _ _ _ _]
          tunnel: [_ _ _ _ _ _ _ _ _ w663 _ _ _ _ _ _ _ _ _ _ _ _ _ _ _ _ _ _ _ _ _ _ _ _ _ _ _ _ _ _ _ _ _ _ _ _ _ _ _ _ _ _ _ _ _ _ _ w2837 _ _ _ _ _ _ _ _ _ _ _ _ _ _ _ _ _ _ _ _ _ _ _ _ _ _ _] -> w308
          tunnel: [_ _ _ _ _ _ _ _ _ _ _ _ _ _ _ _ _ _ _ _ _ _ _ _ _ _ _ _ _ _ _ _ _ _ _ _ _ _ _ _ _ _ _ _ _ _ _ _ _ _ _ _ _ _ _ _ _ w2834 _ _ _ _ _ _ _ w3216 _ _ _ _ _ _ _ _ _ _ _ _ _ _ _ _ _ _ _] -> w307
          tunnel: [_ _ _ _ _ _ _ _ _ _ _ _ _ _ _ _ _ _ _ _ _ _ _ _ _ _ _ _ _ _ _ _ _ _ _ _ _ _ _ _ _ _ _ _ _ _ _ _ _ _ _ _ _ _ _ _ _ w2838 _ _ _ _ _ _ _ w3216 _ _ _ _ _ _ _ _ _ _ _ _ _ _ _ _ _ _ _] -> w306
          tunnel: w304 -> [_ _ _ _ _ _ _ _ _ _ _ _ _ _ _ _ _ _ _ _ _ _ _ _ _ _ _ _ _ _ _ _ _ _ _ _ _ _ _ _ _ _ _ _ _ _ _ _ _ _ _ _ _ _ _ _ _ _ _ _ _ _ _ _ _ _ _ _ _ _ _ _ _ _ _ _ _ _ _ _ _ _ _ _ _]
          tunnel: w303 -> [_ _ _ _ _ _ _ _ _ _ _ _ _ _ _ _ _ _ _ _ _ _ _ _ _ _ _ _ _ _ _ _ _ _ _ _ _ _ _ _ _ _ _ _ _ _ _ _ _ _ _ _ _ _ _ _ _ _ _ _ _ _ _ _ _ _ _ _ _ _ _ _ _ _ _ _ _ _ _ _ _ _ _ _ _]
          tunnel: w302 -> [_ _ _ _ _ _ _ _ _ _ _ _ _ _ _ _ _ _ _ _ _ _ _ _ _ _ _ _ _ _ _ _ _ _ _ _ _ _ _ _ _ _ _ _ _ _ _ _ _ _ _ _ _ _ _ _ _ _ _ _ _ _ _ _ _ _ _ _ _ _ _ _ _ _ _ _ _ _ _ _ _ _ _ _ _]
          tunnel: w301 -> [_ _ _ _ _ _ _ _ _ _ _ _ _ _ _ _ _ _ _ _ _ _ _ _ _ _ _ _ _ _ _ _ _ _ _ _ _ _ _ _ _ _ _ _ _ _ _ _ _ _ _ _ _ _ _ _ _ _ _ _ _ _ _ _ _ _ _ _ _ _ _ _ _ _ _ _ _ _ _ _ _ _ _ _ _]
          tunnel: w300 -> [_ _ _ _ _ _ _ _ _ _ _ _ _ _ _ _ _ _ _ _ _ _ _ _ _ _ _ _ _ _ _ _ _ _ _ _ _ _ _ _ _ _ _ _ _ _ _ _ _ _ _ _ _ _ _ _ _ _ _ _ _ _ _ _ _ _ _ _ _ _ _ _ _ _ _ _ _ _ _ _ _ _ _ _ _]
          tunnel: w299 -> [_ _ _ _ _ _ _ _ _ _ _ _ _ _ _ _ _ _ _ _ _ _ _ _ _ _ _ _ _ _ _ _ _ _ _ _ _ _ _ _ _ _ _ _ _ _ _ _ _ _ _ _ _ _ _ _ _ _ _ _ _ _ _ _ _ _ _ _ _ _ _ _ _ _ _ _ _ _ _ _ _ _ _ _ _]
          tunnel: w298 -> [_ _ _ _ _ _ _ _ _ _ _ _ _ _ _ _ _ _ _ _ _ _ _ _ _ _ _ _ _ _ _ _ _ _ _ _ _ _ _ _ _ _ _ _ _ _ _ _ _ _ _ _ _ _ _ _ _ _ _ _ _ w3023 _ w3120 _ _ _ _ _ w3406 _ w3500 _ _ _ _ _ _ _ _ _ _ _ _ _]
          tunnel: w297 -> [_ _ _ _ _ _ _ _ _ _ _ _ _ _ _ _ _ _ _ _ _ _ _ _ _ _ _ _ _ _ _ _ _ _ _ _ _ _ _ _ _ _ _ _ _ _ _ _ _ _ _ _ _ _ _ _ _ _ _ _ _ w3026 _ w3122 _ _ _ _ _ w3408 _ w3502 _ _ _ _ _ _ _ _ _ _ _ _ _]
          tunnel: [_ _ _ _ _ _ _ _ _ _ _ _ _ _ _ _ _ _ _ _ _ _ _ _ _ _ _ _ _ _ _ _ _ _ _ _ _ _ _ _ _ _ _ _ _ _ _ _ _ _ _ _ _ _ _ _ _ _ _ _ _ w3024 _ w3121 _ _ _ _ _ _ _ _ _ _ _ _ _ _ _ _ _ _ _ _ _] -> w296
          frame "None" {
            # ">>> Motor control cluster >>>"
            # ">>> yStepper command>>>"
          }
          frame "Startup" {
            # ">>> yStepper command>>>"
            n229 = for {
              shift-right: [w377] -> w371
              shift-left: w374 -> [w376]
              tunnel: string[] ["INIT", "RESET ARM", "RESET FLAGS", "RESET YAW", "NAVX CALIBRATE"] -> [w375] mode=indexing
              n230 = Enqueue Element(queue=w376, element=w375) -> (queue out=w377:refnum<queue>)  [unwired: 2 in, 2 out]
            }
            n231 = Bundle By Name(cluster=w369, "yStepper desired"=u8 0) -> (w368:T21)
            n232 = Bundle By Name(cluster=w366, "ySpeed"=0.0, "xSpeed"=0.0, "wSpeed"=0.0) -> (w365:T20)
          }
          frame "Move to Angle" {
          }
          frame "True Stop" {
            # ">>Action Queue>>"
            # ">>> Motor control cluster >>>"
            # ">>> yStepper command>>>"
            n233 = Flush Queue(queue=w388, error in (no error)=w387) -> ()  [unwired: 3 out]
            n234 = for {
              shift-right: [w394] -> w389
              shift-left: w390 -> [w393]
              tunnel: string[] ["STOP", "RESET ENCODERS", "RESET YAW", "RESET ARM", "RESET ALL SENSORS", "RESET FLAGS", "DISPOSE CAM BUFFERS", "DISPOSE PROC BUFFERS", "CAM CLOSE"] -> [w392] mode=indexing
              n235 = Enqueue Element(queue=w393, element=w392) -> (queue out=w394:refnum<queue>)  [unwired: 2 in, 2 out]
            }
          }
          frame "Idle", Default {
            # ">>> Motor control cluster >>>"
            # ">>> yStepper command>>>"
            n236 = Dequeue Element(queue=w406, timeout in ms (-1)=w405, error in (no error)=w401) -> (element=w404:T10)  [unwired: 3 out]
            n237 = case shown="\"Start Task A\"" w404 {
              tunnel: [w409 w417 w425 w433 w441 w449 w457 w465 w473 w480 w490 w500 w507 w510] -> w400
              tunnel: w403 -> [w410 w418 w426 w434 w442 w450 w458 w466 w474 w481 w489 w499 w507 w511]
              tunnel: [State_Type_Definitions,_for_0.26g_versions_and_later_3."Task 1A" ("Enum") State_Type_Definitions,_for_0.26g_versions_and_later_3."Task 2:Raise Arm" ("Enum") State_Type_Definitions,_for_0.26g_versions_and_later_3."Task 3: Rotate 360" ("Enum") State_Type_Definitions,_for_0.26g_versions_and_later_3."Task 4_A" ("Enum") State_Type_Definitions,_for_0.26g_versions_and_later_3."Task 5A: RAISING ARM" ("Enum") State_Type_Definitions,_for_0.26g_versions_and_later_3."Task 6A: RAISE ARM" ("Enum") State_Type_Definitions,_for_0.26g_versions_and_later_3."Task 8A: RAISE ARM" ("Enum") State_Type_Definitions,_for_0.26g_versions_and_later_3."Task 8A: RAISE ARM" ("Enum") State_Type_Definitions,_for_0.26g_versions_and_later_3."Task 8A: RAISE ARM" ("Enum") State_Type_Definitions,_for_0.26g_versions_and_later_3."Task 8A: RAISE ARM" ("Enum") State_Type_Definitions,_for_0.26g_versions_and_later_3."Task 9A: Raise Arm" ("Enum") State_Type_Definitions,_for_0.26g_versions_and_later_3."Task A1: RAISE ARM" ("Enum") State_Type_Definitions,_for_0.26g_versions_and_later_3."Idle" ("Enum") State_Type_Definitions,_for_0.26g_versions_and_later_3."Shutdown" ("Enum")] -> w402
              tunnel: [enum16{"Ball", "Soap", "Gel", "Pipe", "None"}."None" ("Object recognition mode") enum16{"Ball", "Soap", "Gel", "Pipe", "None"}."None" ("Object recognition mode") enum16{"Ball", "Soap", "Gel", "Pipe", "None"}."None" ("Object recognition mode") enum16{"Ball", "Soap", "Gel", "Pipe", "None"}."None" ("Object recognition mode") enum16{"Ball", "Soap", "Gel", "Pipe", "None"}."None" ("Object recognition mode") enum16{"Ball", "Soap", "Gel", "Pipe", "None"}."None" ("Object recognition mode") enum16{"Ball", "Soap", "Gel", "Pipe", "None"}."Ball" ("Object recognition mode") enum16{"Ball", "Soap", "Gel", "Pipe", "None"}."Gel" ("Object recognition mode") enum16{"Ball", "Soap", "Gel", "Pipe", "None"}."Pipe" ("Object recognition mode") enum16{"Ball", "Soap", "Gel", "Pipe", "None"}."Soap" ("Object recognition mode") enum16{"Ball", "Soap", "Gel", "Pipe", "None"}."None" ("Object recognition mode") enum16{"Ball", "Soap", "Gel", "Pipe", "None"}."Ball" ("Object recognition mode") enum16{"Ball", "Soap", "Gel", "Pipe", "None"}."None" ("Object recognition mode") enum16{"Ball", "Soap", "Gel", "Pipe", "None"}."None" ("Object recognition mode")] -> w395
              frame "Start Task 1" {
                n238 = for {
                  shift-right: [w414] -> w409
                  shift-left: w410 -> [w413]
                  tunnel: string[] ["RESET ENCODERS", "RESET YAW", "FORWARD", "READ ENCODERS"] -> [w412] mode=indexing
                  n239 = Enqueue Element(queue=w413, element=w412) -> (queue out=w414:refnum<queue>)  [unwired: 2 in, 2 out]
                }
              }
              frame "Start Task 2" {
                n240 = for {
                  shift-right: [w422] -> w417
                  shift-left: w418 -> [w421]
                  tunnel: string[] ["RESET ENCODERS", "RESET YAW", "READ ULTRASONIC", "ARDUINO - ULTRASONIC"] -> [w420] mode=indexing
                  n241 = Enqueue Element(queue=w421, element=w420) -> (queue out=w422:refnum<queue>)  [unwired: 2 in, 2 out]
                }
              }
              frame "Start Task 3" {
                n242 = for {
                  shift-right: [w430] -> w425
                  shift-left: w426 -> [w429]
                  tunnel: string[] ["RESET ENCODERS", "READ ENCODERS", "R-ACW"] -> [w428] mode=indexing
                  n243 = Enqueue Element(queue=w429, element=w428) -> (queue out=w430:refnum<queue>)  [unwired: 2 in, 2 out]
                }
              }
              frame "Start Task 4" {
                n244 = for {
                  shift-right: [w438] -> w433
                  shift-left: w434 -> [w437]
                  tunnel: string[] ["RESET YAW", "RESET ENCODERS", "RESET ARM", "RESET FLAGS", "", ""] -> [w436] mode=indexing
                  n245 = Enqueue Element(queue=w437, element=w436) -> (queue out=w438:refnum<queue>)  [unwired: 2 in, 2 out]
                }
              }
              frame "Start Task 5" {
                n246 = for {
                  shift-right: [w446] -> w441
                  shift-left: w442 -> [w445]
                  tunnel: string[] ["RESET YAW", "RESET ENCODERS", "RESET ARM", "RESET ALL SENSORS", "", ""] -> [w444] mode=indexing
                  n247 = Enqueue Element(queue=w445, element=w444) -> (queue out=w446:refnum<queue>)  [unwired: 2 in, 2 out]
                }
              }
              frame "Start Task 6" {
                n248 = for {
                  shift-right: [w454] -> w449
                  shift-left: w450 -> [w453]
                  tunnel: string[] ["OPEN LOG CAM ", "", "", "", "", ""] -> [w452] mode=indexing
                  n249 = Enqueue Element(queue=w453, element=w452) -> (queue out=w454:refnum<queue>)  [unwired: 2 in, 2 out]
                }
              }
              frame "Start Task 8 - BALL" {
                n250 = for {
                  shift-right: [w462] -> w457
                  shift-left: w458 -> [w461]
                  tunnel: string[] ["RESET YAW", "RESET ENCODERS", "RESET ARM", "RESET FLAGS"] -> [w460] mode=indexing
                  n251 = Enqueue Element(queue=w461, element=w460) -> (queue out=w462:refnum<queue>)  [unwired: 2 in, 2 out]
                }
              }
              frame "Start Task 8 - Gel" {
                n252 = for {
                  shift-right: [w470] -> w465
                  shift-left: w466 -> [w469]
                  tunnel: string[] ["RESET YAW", "RESET ENCODERS", "RESET ARM", "RESET FLAGS"] -> [w468] mode=indexing
                  n253 = Enqueue Element(queue=w469, element=w468) -> (queue out=w470:refnum<queue>)  [unwired: 2 in, 2 out]
                }
              }
              frame "Start Task 8 - Pipe" {
                n254 = for {
                  shift-right: [w478] -> w473
                  shift-left: w474 -> [w477]
                  tunnel: string[] ["RESET YAW", "RESET ENCODERS", "RESET ARM", "RESET FLAGS"] -> [w476] mode=indexing
                  n255 = Enqueue Element(queue=w477, element=w476) -> (queue out=w478:refnum<queue>)  [unwired: 2 in, 2 out]
                }
              }
              frame "Start Task 8 - Soap" {
                n256 = for {
                  shift-right: [w486] -> w480
                  shift-left: w481 -> [w485]
                  tunnel: string[] ["RESET YAW", "RESET ENCODERS", "RESET ARM", "RESET FLAGS"] -> [w484] mode=indexing
                  n257 = Enqueue Element(queue=w485, element=w484) -> (queue out=w486:refnum<queue>)  [unwired: 2 in, 2 out]
                }
              }
              frame "Start Task 9" {
                n258 = for {
                  shift-right: [w494] -> w490
                  shift-left: w489 -> [w493]
                  tunnel: string[] ["Z STEPPER BOX HEIGHT", "READ STEPPER VALUES", "", ""] -> [w492] mode=indexing
                  n259 = Enqueue Element(queue=w493, element=w492) -> (queue out=w494:refnum<queue>)  [unwired: 2 in, 2 out]
                }
              }
              frame "Start Task A" {
                n260 = for {
                  shift-right: [w504] -> w500
                  shift-left: w499 -> [w503]
                  tunnel: string[] ["Z STEPPER BOX HEIGHT", "READ STEPPER VALUES", "", ""] -> [w502] mode=indexing
                  n261 = Enqueue Element(queue=w503, element=w502) -> (queue out=w504:refnum<queue>)  [unwired: 2 in, 2 out]
                }
                n262 = call "Box Colour FGV.vi"("Colour to detect"=Box_Colour_FGV_Colours."Red", "Init/R/W State"=Box_Colour_FGV_States."Write") -> ()  [unwired: 8 in, 2 out]
              }
              frame "None", Default {
              }
              frame "Exit" {
                n263 = for {
                  shift-right: [w515] -> w510
                  shift-left: w511 -> [w514]
                  tunnel: string[] ["STOP", "RESET ENCODERS", "RESET YAW", "EXIT"] -> [w513] mode=indexing
                  n264 = Enqueue Element(queue=w514, element=w513) -> (queue out=w515:refnum<queue>)  [unwired: 2 in, 2 out]
                }
              }
            }
          }
          frame "Shutdown" {
            # ">> Item Selection Bias >>"
            # ">>> yStepper command>>>"
            n265 = for {
              shift-right: [w526] -> w520
              shift-left: w522 -> [w525]
              tunnel: string[] ["INIT", "RESET ENCODERS", "RESET FLAGS", "CAM CLOSE", "DISPOSE BUFFERS", "EXIT", ""] -> [w524] mode=indexing
              n266 = Enqueue Element(queue=w525, element=w524) -> (queue out=w526:refnum<queue>)  [unwired: 2 in, 2 out]
            }
          }
          frame "Task 1A" {
            # ">>> Motor control cluster >>>"
            # ">> Line detection >>"
            # ">> Checks if 1 metre moved >>"
            # ">>> yStepper command>>>"
            # "Use 250"
            n267 = Greater?(x=w536, y=265.0) -> (0:w530:bool)
            n268 = Dequeue Element(queue=w543, timeout in ms (-1)=w542, error in (no error)=w541) -> (element=w540:T10)  [unwired: 3 out]
            n269 = And(x=w529, y=w530) -> (x .and. y?=w527:bool)
            n270 = case shown="\"Start Task 1\", Default" w540 {
              tunnel: w528 -> [w544 _]
              tunnel: [w554 State_Type_Definitions,_for_0.26g_versions_and_later_3."True Stop" ("Enum")] -> w539
              tunnel: w538 -> [w552 w569]
              tunnel: [w551 w568] -> w537
              tunnel: [State_Type_Definitions,_for_0.26g_versions_and_later_3."Idle" ("Enum") State_Type_Definitions,_for_0.26g_versions_and_later_3."Shutdown" ("Enum")] -> w534
              tunnel: w527 -> [w545 _]
              frame "Start Task 1", Default {
                n271 = Or(x=w545, y=w544) -> (x .or. y?=w546:bool)
                n272 = case shown="True" w546 {
                  tunnel: w552 -> [w557 w563]
                  tunnel: [w556 w561] -> w551
                  frame False {
                    n273 = for {
                      shift-right: [w559] -> w556
                      shift-left: w557 -> [w560]
                      tunnel: string[] ["READ ENCODERS", "READ NAVX", "FORWARD", "READ LINE SENSOR"] ("element") -> [w558] mode=indexing
                      n274 = Enqueue Element(queue=w560, element=w558) -> (queue out=w559:refnum<queue>)  [unwired: 2 in, 2 out]
                    }
                  }
                  frame True {
                    n275 = for {
                      shift-right: [w565] -> w561
                      shift-left: w563 -> [w566]
                      tunnel: string[] ["RESET YAW", "RESET ENCODERS", "STOP", ""] -> [w564] mode=indexing
                      n276 = Enqueue Element(queue=w566, element=w564) -> (queue out=w565:refnum<queue>)  [unwired: 2 in, 2 out]
                    }
                  }
                }
                n277 = Select(t=State_Type_Definitions,_for_0.26g_versions_and_later_3."True Stop" ("Enum"), s=w544, f=State_Type_Definitions,_for_0.26g_versions_and_later_3."Task 1B" ("Enum")) -> (s? t:f=w549:T18)
                n278 = Select(t=w549, s=w545, f=State_Type_Definitions,_for_0.26g_versions_and_later_3."Task 1A" ("Enum")) -> (s? t:f=w554:T18)
              }
              frame "Exit" {
                n279 = for {
                  shift-right: [w573] -> w568
                  shift-left: w569 -> [w574]
                  tunnel: string[] ["STOP", "RESET ENCODERS", "RESET YAW", ""] -> [w572] mode=indexing
                  n280 = Enqueue Element(queue=w574, element=w572) -> (queue out=w573:refnum<queue>)  [unwired: 2 in, 2 out]
                }
              }
            }
          }
          frame "Task 1B" {
            # ">>> Motor control cluster >>>"
            # ">> Line detection >>"
            # ">> Adds small distance overhead after 1M >>"
            # ">>> yStepper command>>>"
            n281 = Greater?(x=w581, y=50.0) -> (0:w575:bool)
            n282 = Dequeue Element(queue=w590, timeout in ms (-1)=w589, error in (no error)=w588) -> (element=w587:T10)  [unwired: 3 out]
            n283 = Or(x=w575, y=w582) -> (x .or. y?=w586:bool)
            n284 = case shown="\"Start Task 1\", Default" w587 {
              tunnel: w586 -> [w593 _]
              tunnel: [w597 State_Type_Definitions,_for_0.26g_versions_and_later_3."True Stop" ("Enum")] -> w585
              tunnel: w584 -> [w594 w612]
              tunnel: [w592 w611] -> w583
              tunnel: [State_Type_Definitions,_for_0.26g_versions_and_later_3."Idle" ("Enum") State_Type_Definitions,_for_0.26g_versions_and_later_3."Shutdown" ("Enum")] -> w579
              frame "Start Task 1", Default {
                n285 = case shown="True" w593 {
                  tunnel: w594 -> [w600 w606]
                  tunnel: [w599 w604] -> w592
                  frame False {
                    n286 = for {
                      shift-right: [w602] -> w599
                      shift-left: w600 -> [w603]
                      tunnel: string[] ["READ ENCODERS", "READ NAVX", "FORWARD", "READ LINE SENSOR"] ("element") -> [w601] mode=indexing
                      n287 = Enqueue Element(queue=w603, element=w601) -> (queue out=w602:refnum<queue>)  [unwired: 2 in, 2 out]
                    }
                  }
                  frame True {
                    n288 = for {
                      shift-right: [w608] -> w604
                      shift-left: w606 -> [w609]
                      tunnel: string[] ["RESET YAW", "RESET ENCODERS", "STOP", ""] -> [w607] mode=indexing
                      n289 = Enqueue Element(queue=w609, element=w607) -> (queue out=w608:refnum<queue>)  [unwired: 2 in, 2 out]
                    }
                  }
                }
                n290 = Select(t=State_Type_Definitions,_for_0.26g_versions_and_later_3."True Stop" ("Enum"), s=w593, f=State_Type_Definitions,_for_0.26g_versions_and_later_3."Task 1B" ("Enum")) -> (s? t:f=w597:T18)
              }
              frame "Exit" {
                n291 = for {
                  shift-right: [w616] -> w611
                  shift-left: w612 -> [w617]
                  tunnel: string[] ["STOP", "RESET ENCODERS", "RESET YAW", ""] -> [w615] mode=indexing
                  n292 = Enqueue Element(queue=w617, element=w615) -> (queue out=w616:refnum<queue>)  [unwired: 2 in, 2 out]
                }
              }
            }
          }
          frame "Task 2:Raise Arm" {
            # ">>> Motor control cluster >>>"
            # ">> Stepper height reeached >>"
            # ">>> yStepper command>>>"
            # ">> Manual override >>"
            n293 = Dequeue Element(queue=w624, timeout in ms (-1)=w623, error in (no error)=w622) -> (element=w632:T10)  [unwired: 3 out]
            n294 = Equal?(x=w626, y=u8 60) -> (x = y?=w618:bool)
            n295 = case shown="\"Start Task 1\", Default" w632 {
              tunnel: [w643 State_Type_Definitions,_for_0.26g_versions_and_later_3."True Stop" ("Enum")] -> w628
              tunnel: [w641 w658] -> w621
              tunnel: w630 -> [w640 _]
              tunnel: w629 -> [w634 _]
              tunnel: [State_Type_Definitions,_for_0.26g_versions_and_later_3."Idle" ("Enum") State_Type_Definitions,_for_0.26g_versions_and_later_3."Shutdown" ("Enum")] -> w627
              tunnel: w618 -> [w633 _]
              frame "Start Task 1", Default {
                # ">> WIill proceed to part ii if not manual override >>"
                # ">>If ENABLE or Trigger is set to true>>"
                n296 = Or(x=w633, y=w634) -> (x .or. y?=w635:bool)
                n297 = case shown="True" w633 {
                  tunnel: [w646 w652] -> w641
                  tunnel: w640 -> [w645 w651]
                  frame False {
                    n298 = for {
                      shift-right: [w648] -> w646
                      shift-left: w645 -> [w649]
                      tunnel: string[] ["Z STEPPER CAM HEIGHT", "READ STEPPER VALUES"] ("element") -> [w647] mode=indexing
                      n299 = Enqueue Element(queue=w649, element=w647) -> (queue out=w648:refnum<queue>)  [unwired: 2 in, 2 out]
                    }
                  }
                  frame True {
                    n300 = for {
                      shift-right: [w654] -> w652
                      shift-left: w651 -> [w655]
                      tunnel: string[] ["ARDUINO - ULTRASONIC", "READ ULTRASONIC", "", "", "", ""] -> [w653] mode=indexing
                      n301 = Enqueue Element(queue=w655, element=w653) -> (queue out=w654:refnum<queue>)  [unwired: 2 in, 2 out]
                    }
                  }
                }
                n302 = Select(t=State_Type_Definitions,_for_0.26g_versions_and_later_3."True Stop" ("Enum"), s=w634, f=State_Type_Definitions,_for_0.26g_versions_and_later_3."Task 2:Sensor Mode" ("Enum")) -> (s? t:f=w637:T18)
                n303 = Select(t=w637, s=w635, f=State_Type_Definitions,_for_0.26g_versions_and_later_3."Task 2:Raise Arm" ("Enum")) -> (s? t:f=w643:T18)
              }
              frame "Exit" {
                n304 = for {
                  shift-right: [w661] -> w658
                  shift-left: _ -> [w662]
                  tunnel: string[] ["STOP", "RESET ENCODERS", "RESET YAW", ""] -> [w660] mode=indexing
                  n305 = Enqueue Element(queue=w662, element=w660) -> (queue out=w661:refnum<queue>)  [unwired: 2 in, 2 out]
                }
              }
            }
          }
          frame "Task 2:Sensor Mode" {
            w679 = u8 20 ("y")
            # ">>> Motor control cluster >>>"
            # ">>> yStepper command>>>"
            # ">>Object detected>>"
            n306 = Dequeue Element(queue=w672, timeout in ms (-1)=w671, error in (no error)=w670) -> (element=w680:T10)  [unwired: 3 out]
            n307 = Less?(x=w668, y=w679) -> (x < y?=w678:bool)
            n308 = Less?(x=w667, y=w679) -> (x < y?=w677:bool)
            n309 = Or(x=w678, y=w677) -> (x .or. y?=w663:bool)
            n310 = case shown="\"Start Task 1\", Default" w680 {
              tunnel: w663 -> [w683 _]
              tunnel: [w690 State_Type_Definitions,_for_0.26g_versions_and_later_3."True Stop" ("Enum")] -> w676
              tunnel: w669 -> [w682 _]
              tunnel: w673 -> [w689 w706]
              tunnel: [w688 w707] -> w675
              tunnel: [State_Type_Definitions,_for_0.26g_versions_and_later_3."Idle" ("Enum") State_Type_Definitions,_for_0.26g_versions_and_later_3."Shutdown" ("Enum")] -> w674
              frame "Start Task 1", Default {
                n311 = case shown="True" w683 {
                  tunnel: w689 -> [w693 w700]
                  tunnel: [w694 w699] -> w688
                  frame False {
                    n312 = for {
                      tunnel: string[] ["READ ULTRASONIC", "STOP"] ("element") -> [w695] mode=indexing
                      shift-right: [w697] -> w694
                      shift-left: w693 -> [w696]
                      n313 = Enqueue Element(queue=w696, element=w695) -> (queue out=w697:refnum<queue>)  [unwired: 2 in, 2 out]
                    }
                  }
                  frame True {
                    n314 = for {
                      shift-right: [w702] -> w699
                      shift-left: w700 -> [w703]
                      tunnel: string[] ["RESET ENCODERS", "READ NAVX", "READ ENCODERS"] -> [w701] mode=indexing
                      n315 = Enqueue Element(queue=w703, element=w701) -> (queue out=w702:refnum<queue>)  [unwired: 2 in, 2 out]
                    }
                  }
                }
                n316 = Or(x=w683, y=w682) -> (x .or. y?=w681:bool)
                n317 = Select(t=State_Type_Definitions,_for_0.26g_versions_and_later_3."True Stop" ("Enum"), s=w682, f=State_Type_Definitions,_for_0.26g_versions_and_later_3."Task 2:Reverse Mode" ("Enum")) -> (s? t:f=w684:T18)
                n318 = Select(t=w684, s=w681, f=State_Type_Definitions,_for_0.26g_versions_and_later_3."Task 2:Sensor Mode" ("Enum")) -> (s? t:f=w690:T18)
              }
              frame "Exit" {
                n319 = for {
                  shift-right: [w710] -> w707
                  shift-left: w706 -> [w711]
                  tunnel: string[] ["STOP", "RESET ENCODERS", "RESET YAW", "ARDUINO MODE 0"] -> [w709] mode=indexing
                  n320 = Enqueue Element(queue=w711, element=w709) -> (queue out=w710:refnum<queue>)  [unwired: 2 in, 2 out]
                }
              }
            }
          }
          frame "Task 2:Reverse Mode" {
            # ">>> yStepper command>>>"
            n321 = Dequeue Element(queue=w722, timeout in ms (-1)=w723, error in (no error)=w724) -> (element=w726:T10)  [unwired: 3 out]
            n322 = Less?(x=w716, y=-30.0) -> (x < y?=w712:bool)
            n323 = case shown="\"Start Task 1\", Default" w726 {
              tunnel: [w736 State_Type_Definitions,_for_0.26g_versions_and_later_3."True Stop" ("Enum")] -> w718
              tunnel: w725 -> [w729 _]
              tunnel: w721 -> [w735 w752]
              tunnel: [w734 w753] -> w717
              tunnel: [State_Type_Definitions,_for_0.26g_versions_and_later_3."Idle" ("Enum") State_Type_Definitions,_for_0.26g_versions_and_later_3."Shutdown" ("Enum")] -> w719
              tunnel: w712 -> [w727 _]
              frame "Start Task 1", Default {
                n324 = case shown="True" w727 {
                  tunnel: w735 -> [w739 w746]
                  tunnel: [w740 w745] -> w734
                  frame False {
                    n325 = for {
                      tunnel: string[] ["READ ENCODERS", "REVERSE", "READ NAVX"] ("element") -> [w741] mode=indexing
                      shift-right: [w743] -> w740
                      shift-left: w739 -> [w742]
                      n326 = Enqueue Element(queue=w742, element=w741) -> (queue out=w743:refnum<queue>)  [unwired: 2 in, 2 out]
                    }
                  }
                  frame True {
                    n327 = for {
                      shift-right: [w748] -> w745
                      shift-left: w746 -> [w749]
                      tunnel: string[] ["STOP", "ARDUINO - ULTRASONIC", "READ ULTRASONIC", "RESET ENCODERS"] -> [w747] mode=indexing
                      n328 = Enqueue Element(queue=w749, element=w747) -> (queue out=w748:refnum<queue>)  [unwired: 2 in, 2 out]
                    }
                  }
                }
                n329 = Or(x=w727, y=w729) -> (x .or. y?=w728:bool)
                n330 = Select(t=State_Type_Definitions,_for_0.26g_versions_and_later_3."True Stop" ("Enum"), s=w729, f=State_Type_Definitions,_for_0.26g_versions_and_later_3."Task 2:Sensor Mode" ("Enum")) -> (s? t:f=w730:T18)
                n331 = Select(t=w730, s=w728, f=State_Type_Definitions,_for_0.26g_versions_and_later_3."Task 2:Reverse Mode" ("Enum")) -> (s? t:f=w736:T18)
              }
              frame "Exit" {
                n332 = for {
                  shift-right: [w756] -> w753
                  shift-left: w752 -> [w757]
                  tunnel: string[] ["STOP", "RESET ENCODERS", "RESET YAW", "ARDUINO MODE 0"] -> [w755] mode=indexing
                  n333 = Enqueue Element(queue=w757, element=w755) -> (queue out=w756:refnum<queue>)  [unwired: 2 in, 2 out]
                }
              }
            }
          }
          frame "Task 3: Rotate 360" {
            # ">>> Motor control cluster >>>"
            # ">>> yStepper command>>>"
            n334 = Dequeue Element(queue=w773, timeout in ms (-1)=w772, error in (no error)=w771) -> (element=w763:T10)  [unwired: 3 out]
            n335 = Less?(x=w770, y=-160.0) -> (x < y?=w758:bool)
            n336 = Or(x=w758, y=w768) -> (x .or. y?=w764:bool)
            n337 = case shown="\"Start Task 1\", Default" w763 {
              tunnel: w764 -> [w776 _]
              tunnel: [w780 State_Type_Definitions,_for_0.26g_versions_and_later_3."True Stop" ("Enum")] -> w765
              tunnel: w767 -> [w777 w796]
              tunnel: [w775 w795] -> w766
              tunnel: [State_Type_Definitions,_for_0.26g_versions_and_later_3."Idle" ("Enum") State_Type_Definitions,_for_0.26g_versions_and_later_3."Shutdown" ("Enum")] -> w762
              frame "Start Task 1", Default {
                n338 = case shown="False" w776 {
                  tunnel: w777 -> [w783 w789]
                  tunnel: [w782 w787] -> w775
                  frame False {
                    n339 = for {
                      shift-right: [w785] -> w782
                      shift-left: w783 -> [w786]
                      tunnel: string[] ["READ ENCODERS", "R-CW"] ("element") -> [w784] mode=indexing
                      n340 = Enqueue Element(queue=w786, element=w784) -> (queue out=w785:refnum<queue>)  [unwired: 2 in, 2 out]
                    }
                  }
                  frame True {
                    n341 = for {
                      shift-right: [w791] -> w787
                      shift-left: w789 -> [w792]
                      tunnel: string[] ["RESET YAW", "RESET ENCODERS", "STOP", "ARDUINO MODE 0"] -> [w790] mode=indexing
                      n342 = Enqueue Element(queue=w792, element=w790) -> (queue out=w791:refnum<queue>)  [unwired: 2 in, 2 out]
                    }
                  }
                }
                n343 = Select(t=State_Type_Definitions,_for_0.26g_versions_and_later_3."True Stop" ("Enum"), s=w776, f=State_Type_Definitions,_for_0.26g_versions_and_later_3."Task 3: Rotate 360" ("Enum")) -> (s? t:f=w780:T18)
              }
              frame "Exit" {
                n344 = for {
                  shift-right: [w799] -> w795
                  shift-left: w796 -> [w800]
                  tunnel: string[] ["STOP", "RESET ENCODERS", "RESET YAW", ""] -> [w798] mode=indexing
                  n345 = Enqueue Element(queue=w800, element=w798) -> (queue out=w799:refnum<queue>)  [unwired: 2 in, 2 out]
                }
              }
            }
          }
          frame "Task 4_A" {
            # ">> Stepper height reeached >>"
            # ">>> yStepper command>>>"
            # ">> Manual override >>"
            n346 = Dequeue Element(queue=w814, timeout in ms (-1)=w813, error in (no error)=w812) -> (element=w811:T10)  [unwired: 3 out]
            n347 = Equal?(x=w805, y=u8 60) -> (x = y?=w801:bool)
            n348 = case shown="\"Start Task 1\", Default" w811 {
              tunnel: [w826 State_Type_Definitions,_for_0.26g_versions_and_later_3."True Stop" ("Enum")] -> w810
              tunnel: [w824 w842] -> w809
              tunnel: w815 -> [w823 w839]
              tunnel: w808 -> [w817 _]
              tunnel: [State_Type_Definitions,_for_0.26g_versions_and_later_3."Idle" ("Enum") State_Type_Definitions,_for_0.26g_versions_and_later_3."Shutdown" ("Enum")] -> w807
              tunnel: w801 -> [w816 _]
              frame "Start Task 1", Default {
                # ">> WIill proceed to part ii if not manual override >>"
                # ">>If ENABLE or Trigger is set to true>>"
                n349 = Or(x=w816, y=w817) -> (x .or. y?=w818:bool)
                n350 = case shown="False" w816 {
                  tunnel: [w829 w835] -> w824
                  tunnel: w823 -> [w828 w834]
                  frame False {
                    n351 = for {
                      shift-right: [w831] -> w829
                      shift-left: w828 -> [w832]
                      tunnel: string[] ["Z STEPPER CAM HEIGHT", "READ STEPPER VALUES"] ("element") -> [w830] mode=indexing
                      n352 = Enqueue Element(queue=w832, element=w830) -> (queue out=w831:refnum<queue>)  [unwired: 2 in, 2 out]
                    }
                  }
                  frame True {
                    n353 = for {
                      shift-right: [w837] -> w835
                      shift-left: w834 -> [w838]
                      tunnel: string[] ["ARDUINO - ULTRASONIC", "READ ULTRASONIC", "FORWARD", "", "", ""] -> [w836] mode=indexing
                      n354 = Enqueue Element(queue=w838, element=w836) -> (queue out=w837:refnum<queue>)  [unwired: 2 in, 2 out]
                    }
                  }
                }
                n355 = Select(t=State_Type_Definitions,_for_0.26g_versions_and_later_3."True Stop" ("Enum"), s=w817, f=State_Type_Definitions,_for_0.26g_versions_and_later_3."Task 4_B" ("Enum")) -> (s? t:f=w820:T18)
                n356 = Select(t=w820, s=w818, f=State_Type_Definitions,_for_0.26g_versions_and_later_3."Task 4_A" ("Enum")) -> (s? t:f=w826:T18)
              }
              frame "Exit" {
                n357 = for {
                  shift-right: [w845] -> w842
                  shift-left: w839 -> [w846]
                  tunnel: string[] ["STOP", "RESET ENCODERS", "RESET YAW", ""] -> [w844] mode=indexing
                  n358 = Enqueue Element(queue=w846, element=w844) -> (queue out=w845:refnum<queue>)  [unwired: 2 in, 2 out]
                }
              }
            }
          }
          frame "Task 4_B" {
            w852 = u8 20
            # ">> Path blocked >>"
            # ">>> yStepper command>>>"
            # ">> Manual override >>"
            n359 = Dequeue Element(queue=w861, timeout in ms (-1)=w860, error in (no error)=w859) -> (element=w858:T10)  [unwired: 3 out]
            n360 = Less?(x=w854, y=w852) -> (x < y?=w849:bool)
            n361 = Less?(x=w853, y=w852) -> (x < y?=w850:bool)
            n362 = And(x=w850, y=w849) -> (x .and. y?=w851:bool)
            n363 = case shown="\"Start Task 1\", Default" w858 {
              tunnel: [w875 State_Type_Definitions,_for_0.26g_versions_and_later_3."True Stop" ("Enum")] -> w863
              tunnel: [w873 w890] -> w864
              tunnel: w857 -> [w872 _]
              tunnel: w862 -> [w866 _]
              tunnel: [State_Type_Definitions,_for_0.26g_versions_and_later_3."Idle" ("Enum") State_Type_Definitions,_for_0.26g_versions_and_later_3."Shutdown" ("Enum")] -> w856
              tunnel: w851 -> [w865 _]
              frame "Start Task 1", Default {
                # ">> Manual override forces program to true stop >>"
                # ">>If ENABLE or Trigger is set to true>>"
                n364 = Or(x=w865, y=w866) -> (x .or. y?=w871:bool)
                n365 = case shown="False" w865 {
                  tunnel: [w878 w883] -> w873
                  tunnel: w872 -> [w877 w882]
                  frame False {
                    n366 = for {
                      shift-right: [w880] -> w878
                      shift-left: w877 -> [w881]
                      tunnel: string[] ["FORWARD", "READ ULTRASONIC", "READ NAVX"] ("element") -> [w879] mode=indexing
                      n367 = Enqueue Element(queue=w881, element=w879) -> (queue out=w880:refnum<queue>)  [unwired: 2 in, 2 out]
                    }
                  }
                  frame True {
                    n368 = for {
                      shift-right: [w886] -> w883
                      shift-left: w882 -> [w887]
                      tunnel: string[] ["STOP", "RESET YAW", "RESET ENCODERS", "RESET FLAGS"] -> [w885] mode=indexing
                      n369 = Enqueue Element(queue=w887, element=w885) -> (queue out=w886:refnum<queue>)  [unwired: 2 in, 2 out]
                    }
                  }
                }
                n370 = Select(t=State_Type_Definitions,_for_0.26g_versions_and_later_3."True Stop" ("Enum"), s=w866, f=State_Type_Definitions,_for_0.26g_versions_and_later_3."Task 4_C" ("Enum")) -> (s? t:f=w868:T18)
                n371 = Select(t=w868, s=w871, f=State_Type_Definitions,_for_0.26g_versions_and_later_3."Task 4_B" ("Enum")) -> (s? t:f=w875:T18)
              }
              frame "Exit" {
                n372 = for {
                  shift-right: [w893] -> w890
                  shift-left: _ -> [w894]
                  tunnel: string[] ["STOP", "RESET ENCODERS", "RESET YAW", ""] -> [w892] mode=indexing
                  n373 = Enqueue Element(queue=w894, element=w892) -> (queue out=w893:refnum<queue>)  [unwired: 2 in, 2 out]
                }
              }
            }
          }
          frame "Task 4_C" {
            w906 = u8 20
            # ">> xDistance travelled>>"
            # ">> Path NOT blocked >>"
            # ">>> yStepper command>>>"
            # ">> Manual override >>"
            n374 = Dequeue Element(queue=w916, timeout in ms (-1)=w909, error in (no error)=w908) -> (element=w910:T10)  [unwired: 3 out]
            n375 = Greater?(x=w898, y=w906) -> (0:w904:bool)
            n376 = Greater?(x=w903, y=80.0) -> (0:w901:bool)
            n377 = Greater?(x=w897, y=w906) -> (0:w905:bool)
            n378 = And(x=w905, y=w904) -> (x .and. y?=w900:bool)
            n379 = And(x=w901, y=w900) -> (x .and. y?=w899:bool)
            n380 = case shown="\"Start Task 1\", Default" w910 {
              tunnel: [w927 State_Type_Definitions,_for_0.26g_versions_and_later_3."True Stop" ("Enum")] -> w913
              tunnel: [w925 w943] -> w912
              tunnel: w915 -> [w924 w940]
              tunnel: w914 -> [w918 _]
              tunnel: [State_Type_Definitions,_for_0.26g_versions_and_later_3."Idle" ("t") State_Type_Definitions,_for_0.26g_versions_and_later_3."Shutdown" ("Enum")] -> w911
              tunnel: w899 -> [w917 _]
              frame "Start Task 1", Default {
                # ">> Manual override forces program to true stop >>"
                # ">>If ENABLE or Trigger is set to true>>"
                n381 = Or(x=w917, y=w918) -> (x .or. y?=w923:bool)
                n382 = case shown="False" w917 {
                  tunnel: [w930 w935] -> w925
                  tunnel: w924 -> [w928 w934]
                  frame False {
                    n383 = for {
                      shift-right: [w932] -> w930
                      shift-left: w928 -> [w933]
                      tunnel: string[] ["RIGHT", "READ NAVX", "READ ENCODERS", "READ ULTRASONIC"] ("element") -> [w931] mode=indexing
                      n384 = Enqueue Element(queue=w933, element=w931) -> (queue out=w932:refnum<queue>)  [unwired: 2 in, 2 out]
                    }
                  }
                  frame True {
                    n385 = for {
                      shift-right: [w938] -> w935
                      shift-left: w934 -> [w939]
                      tunnel: string[] ["STOP", "RESET YAW", "RESET ENCODERS", "ARDUINO - ULTRASONIC"] -> [w937] mode=indexing
                      n386 = Enqueue Element(queue=w939, element=w937) -> (queue out=w938:refnum<queue>)  [unwired: 2 in, 2 out]
                    }
                  }
                }
                n387 = Select(t=State_Type_Definitions,_for_0.26g_versions_and_later_3."True Stop" ("Enum"), s=w918, f=State_Type_Definitions,_for_0.26g_versions_and_later_3."Task 4_D" ("Enum")) -> (s? t:f=w919:T18)
                n388 = Select(t=w919, s=w923, f=State_Type_Definitions,_for_0.26g_versions_and_later_3."Task 4_C" ("Enum")) -> (s? t:f=w927:T18)
              }
              frame "Exit" {
                n389 = for {
                  shift-right: [w946] -> w943
                  shift-left: w940 -> [w947]
                  tunnel: string[] ["STOP", "RESET ENCODERS", "RESET YAW", ""] -> [w945] mode=indexing
                  n390 = Enqueue Element(queue=w947, element=w945) -> (queue out=w946:refnum<queue>)  [unwired: 2 in, 2 out]
                }
              }
            }
          }
          frame "Task 4_D" {
            w970 = u8 20
            # ">>> Motor control cluster >>>"
            # ">> Line detected >>"
            # ">> yDistance travelled>>"
            # ">> Path blocked >>"
            # ">>> yStepper command>>>"
            # ">> Manual override >>"
            n391 = Less?(x=w955, y=w970) -> (x < y?=w968:bool)
            n392 = Greater?(x=w959, y=200.0) -> (0:w966:bool)
            n393 = Less?(x=w954, y=w970) -> (x < y?=w969:bool)
            n394 = And(x=w969, y=w968) -> (x .and. y?=w965:bool)
            n395 = Dequeue Element(queue=w962, timeout in ms (-1)=w961, error in (no error)=w960) -> (element=w971:T10)  [unwired: 3 out]
            n396 = Or(x=w966, y=w965) -> (x .or. y?=w949:bool)
            n397 = And(x=w950, y=w949) -> (x .and. y?=w948:bool)
            n398 = case shown="\"Start Task 1\", Default" w971 {
              tunnel: [w982 State_Type_Definitions,_for_0.26g_versions_and_later_3."True Stop" ("Enum")] -> w958
              tunnel: [w980 w998] -> w956
              tunnel: w963 -> [w979 w995]
              tunnel: w964 -> [w973 _]
              tunnel: [State_Type_Definitions,_for_0.26g_versions_and_later_3."Idle" ("t") State_Type_Definitions,_for_0.26g_versions_and_later_3."Shutdown" ("Enum")] -> w957
              tunnel: w948 -> [w972 _]
              frame "Start Task 1", Default {
                # ">> Manual override forces program to true stop >>"
                # ">>If ENABLE or Trigger is set to true>>"
                n399 = Or(x=w972, y=w973) -> (x .or. y?=w978:bool)
                n400 = case shown="False" w972 {
                  tunnel: [w985 w990] -> w980
                  tunnel: w979 -> [w983 w989]
                  frame False {
                    n401 = for {
                      shift-right: [w987] -> w985
                      shift-left: w983 -> [w988]
                      tunnel: string[] ["FORWARD", "READ NAVX", "READ ENCODERS", "READ ULTRASONIC", "READ LINE SENSOR"] ("element") -> [w986] mode=indexing
                      n402 = Enqueue Element(queue=w988, element=w986) -> (queue out=w987:refnum<queue>)  [unwired: 2 in, 2 out]
                    }
                  }
                  frame True {
                    n403 = for {
                      shift-right: [w993] -> w990
                      shift-left: w989 -> [w994]
                      tunnel: string[] ["STOP", "RESET YAW", "RESET ENCODERS", "RESET FLAGS"] -> [w992] mode=indexing
                      n404 = Enqueue Element(queue=w994, element=w992) -> (queue out=w993:refnum<queue>)  [unwired: 2 in, 2 out]
                    }
                  }
                }
                n405 = Select(t=State_Type_Definitions,_for_0.26g_versions_and_later_3."True Stop" ("Enum"), s=w973, f=State_Type_Definitions,_for_0.26g_versions_and_later_3."True Stop" ("Enum")) -> (s? t:f=w974:T18)
                n406 = Select(t=w974, s=w978, f=State_Type_Definitions,_for_0.26g_versions_and_later_3."Task 4_D" ("Enum")) -> (s? t:f=w982:T18)
              }
              frame "Exit" {
                n407 = for {
                  shift-right: [w1001] -> w998
                  shift-left: w995 -> [w1002]
                  tunnel: string[] ["STOP", "RESET ENCODERS", "RESET YAW", ""] -> [w1000] mode=indexing
                  n408 = Enqueue Element(queue=w1002, element=w1000) -> (queue out=w1001:refnum<queue>)  [unwired: 2 in, 2 out]
                }
              }
            }
          }
          frame "Task 5A: RAISING ARM" {
            # "Stays in Task 5_A until stepper reaches desired \nheight"
            # ">>> Motor control cluster >>>"
            # ">>> yStepper command>>>"
            # ">> Manual override >>"
            n409 = Dequeue Element(queue=w1013, timeout in ms (-1)=w1012, error in (no error)=w1014) -> (element=w1011:T10)  [unwired: 3 out]
            n410 = Equal?(x=w1010, y=u8 60) -> (x = y?=w1008:bool)
            n411 = case shown="\"Start Task 1\", Default" w1011 {
              tunnel: [w1024 State_Type_Definitions,_for_0.26g_versions_and_later_3."True Stop" ("Enum")] -> w1015
              tunnel: [w1027 w1044] -> w1016
              tunnel: [State_Type_Definitions,_for_0.26g_versions_and_later_3."Idle" ("Enum") State_Type_Definitions,_for_0.26g_versions_and_later_3."Shutdown" ("Enum")] -> w1017
              tunnel: w1008 -> [w1023 _]
              tunnel: w1007 -> [w1022 _]
              tunnel: w1006 -> [w1018 w1041]
              frame "Start Task 1", Default {
                # "T: Go back to idle, F: Continue with task\""
                # ">> Manual override >>"
                n412 = case shown="False" w1023 {
                  tunnel: [w1031 w1037] -> w1027
                  tunnel: w1018 -> [w1029 w1035]
                  frame False {
                    n413 = for {
                      tunnel: string[] ["Z STEPPER CAM HEIGHT", "READ STEPPER VALUES"] ("element") -> [w1032] mode=indexing
                      shift-right: [w1034] -> w1031
                      shift-left: w1029 -> [w1033]
                      n414 = Enqueue Element(queue=w1033, element=w1032) -> (queue out=w1034:refnum<queue>)  [unwired: 2 in, 2 out]
                    }
                  }
                  frame True {
                    n415 = for {
                      shift-right: [w1039] -> w1037
                      shift-left: w1035 -> [w1040]
                      tunnel: string[] ["RESET FLAGS", "RESET YAW", "RESET ENCODERS"] -> [w1038] mode=indexing
                      n416 = Enqueue Element(queue=w1040, element=w1038) -> (queue out=w1039:refnum<queue>)  [unwired: 2 in, 2 out]
                    }
                  }
                }
                n417 = Or(x=w1023, y=w1022) -> (x .or. y?=w1025:bool)
                n418 = Select(t=State_Type_Definitions,_for_0.26g_versions_and_later_3."True Stop" ("Enum"), s=w1022, f=State_Type_Definitions,_for_0.26g_versions_and_later_3."Task 5B: STILL WAITING" ("Enum")) -> (s? t:f=w1019:T18)
                n419 = Select(t=w1019, s=w1025, f=State_Type_Definitions,_for_0.26g_versions_and_later_3."Task 5A: RAISING ARM" ("Enum")) -> (s? t:f=w1024:T18)
              }
              frame "Exit" {
                n420 = for {
                  shift-right: [w1047] -> w1044
                  shift-left: w1041 -> [w1048]
                  tunnel: string[] ["STOP", "RESET ENCODERS", "RESET YAW", "ARDUINO MODE 0"] -> [w1046] mode=indexing
                  n421 = Enqueue Element(queue=w1048, element=w1046) -> (queue out=w1047:refnum<queue>)  [unwired: 2 in, 2 out]
                }
              }
            }
          }
          frame "Task 5B: STILL WAITING" {
            # ">>> yStepper command>>>"
            n422 = Dequeue Element(queue=w1055, timeout in ms (-1)=w1054, error in (no error)=w1056) -> (element=w1053:T10)  [unwired: 3 out]
            n423 = local read "Rising Edge"() -> (w1049:bool)
            n424 = case shown="\"Start Task 1\", Default" w1053 {
              tunnel: [w1068 State_Type_Definitions,_for_0.26g_versions_and_later_3."True Stop" ("Enum")] -> w1058
              tunnel: [w1071 w1088] -> w1057
              tunnel: [State_Type_Definitions,_for_0.26g_versions_and_later_3."Idle" ("Enum") State_Type_Definitions,_for_0.26g_versions_and_later_3."Shutdown" ("Enum")] -> w1059
              tunnel: w1061 -> [w1067 _]
              tunnel: w1060 -> [w1063 w1085]
              tunnel: w1049 -> [w1062 _]
              frame "Start Task 1", Default {
                # "T: Go back to idle, F: Continue with task\""
                # ">> Manual override >>"
                n425 = case shown="False" w1062 {
                  tunnel: [w1075 w1081] -> w1071
                  tunnel: w1063 -> [w1073 w1079]
                  frame False {
                    n426 = for {
                      tunnel: string[] ["READ IR", "READ NAVX", ""] ("element") -> [w1076] mode=indexing
                      shift-right: [w1078] -> w1075
                      shift-left: w1073 -> [w1077]
                      n427 = Enqueue Element(queue=w1077, element=w1076) -> (queue out=w1078:refnum<queue>)  [unwired: 2 in, 2 out]
                    }
                  }
                  frame True {
                    n428 = for {
                      shift-right: [w1083] -> w1081
                      shift-left: w1079 -> [w1084]
                      tunnel: string[] ["Z STEPPER GRAB HEIGHT", "READ STEPPER VALUES", "", ""] -> [w1082] mode=indexing
                      n429 = Enqueue Element(queue=w1084, element=w1082) -> (queue out=w1083:refnum<queue>)  [unwired: 2 in, 2 out]
                    }
                  }
                }
                n430 = Or(x=w1062, y=w1067) -> (x .or. y?=w1069:bool)
                n431 = Select(t=State_Type_Definitions,_for_0.26g_versions_and_later_3."True Stop" ("Enum"), s=w1067, f=State_Type_Definitions,_for_0.26g_versions_and_later_3."Task 5C: GOING DOWN" ("Enum")) -> (s? t:f=w1064:T18)
                n432 = Select(t=w1064, s=w1069, f=State_Type_Definitions,_for_0.26g_versions_and_later_3."Task 5B: STILL WAITING" ("Enum")) -> (s? t:f=w1068:T18)
              }
              frame "Exit" {
                n433 = for {
                  shift-right: [w1091] -> w1088
                  shift-left: w1085 -> [w1092]
                  tunnel: string[] ["STOP", "RESET ENCODERS", "RESET YAW", "ARDUINO MODE 0"] -> [w1090] mode=indexing
                  n434 = Enqueue Element(queue=w1092, element=w1090) -> (queue out=w1091:refnum<queue>)  [unwired: 2 in, 2 out]
                }
              }
            }
          }
          frame "Task 5C: GOING DOWN" {
            # ">>> Motor control cluster >>>"
            # ">>> yStepper command>>>"
            # ">> Manual override >>"
            n435 = Equal?(x=w1095, y=u8 1) -> (x = y?=w1093:bool)
            n436 = Dequeue Element(queue=w1105, timeout in ms (-1)=w1104, error in (no error)=w1103) -> (element=w1102:T10)  [unwired: 3 out]
            n437 = case shown="\"Start Task 1\", Default" w1102 {
              tunnel: [w1114 State_Type_Definitions,_for_0.26g_versions_and_later_3."True Stop" ("Enum")] -> w1107
              tunnel: [w1117 w1134] -> w1100
              tunnel: [State_Type_Definitions,_for_0.26g_versions_and_later_3."Idle" ("Enum") State_Type_Definitions,_for_0.26g_versions_and_later_3."Shutdown" ("Enum")] -> w1099
              tunnel: w1101 -> [w1108 _]
              tunnel: w1106 -> [w1113 w1131]
              tunnel: w1093 -> [w1112 _]
              frame "Start Task 1", Default {
                # ">> Is time up? >>"
                # "Determines if object is in range to pick up"
                # ">> Manual override >>"
                n438 = case shown="False" w1112 {
                  tunnel: [w1121 w1127] -> w1117
                  tunnel: w1113 -> [w1120 w1125]
                  frame False {
                    n439 = for {
                      tunnel: string[] ["READ STEPPER VALUES", "Z STEPPER GRAB HEIGHT", "", ""] -> [w1122] mode=indexing
                      shift-right: [w1124] -> w1121
                      shift-left: w1120 -> [w1123]
                      n440 = Enqueue Element(queue=w1123, element=w1122) -> (queue out=w1124:refnum<queue>)  [unwired: 2 in, 2 out]
                    }
                  }
                  frame True {
                    n441 = for {
                      shift-right: [w1129] -> w1127
                      shift-left: w1125 -> [w1130]
                      tunnel: string[] ["RESET FLAGS", "RESET YAW", "SET TIMER 5"] -> [w1128] mode=indexing
                      n442 = Enqueue Element(queue=w1130, element=w1128) -> (queue out=w1129:refnum<queue>)  [unwired: 2 in, 2 out]
                    }
                  }
                }
                n443 = Or(x=w1112, y=w1108) -> (x .or. y?=w1115:bool)
                n444 = Select(t=State_Type_Definitions,_for_0.26g_versions_and_later_3."True Stop" ("Enum"), s=w1108, f=State_Type_Definitions,_for_0.26g_versions_and_later_3."Task 5D: GRAB" ("Enum")) -> (s? t:f=w1110:T18)
                n445 = Select(t=w1110, s=w1115, f=State_Type_Definitions,_for_0.26g_versions_and_later_3."Task 5C: GOING DOWN" ("Enum")) -> (s? t:f=w1114:T18)
              }
              frame "Exit" {
                n446 = for {
                  shift-right: [w1137] -> w1134
                  shift-left: w1131 -> [w1138]
                  tunnel: string[] ["STOP", "RESET ENCODERS", "RESET YAW", "ARDUINO MODE 0"] -> [w1136] mode=indexing
                  n447 = Enqueue Element(queue=w1138, element=w1136) -> (queue out=w1137:refnum<queue>)  [unwired: 2 in, 2 out]
                }
              }
            }
          }
          frame "Task 5D: GRAB" {
            # ">>> Motor control cluster >>>"
            # ">>> yStepper command>>>"
            n448 = Dequeue Element(queue=w1146, timeout in ms (-1)=w1145, error in (no error)=w1144) -> (element=w1143:T10)  [unwired: 3 out]
            n449 = case shown="\"Start Task 1\", Default" w1143 {
              tunnel: [w1158 State_Type_Definitions,_for_0.26g_versions_and_later_3."True Stop" ("Enum")] -> w1150
              tunnel: [w1161 w1178] -> w1149
              tunnel: [State_Type_Definitions,_for_0.26g_versions_and_later_3."Idle" ("Enum") State_Type_Definitions,_for_0.26g_versions_and_later_3."Shutdown" ("Enum")] -> w1151
              tunnel: w1147 -> [w1157 _]
              tunnel: w1148 -> [w1153 w1175]
              tunnel: w1141 -> [w1152 _]
              frame "Start Task 1", Default {
                # ">> T: Breaks out of state loop; F: Stays in loop>>"
                # ">> Manual override >>"
                # ">> Checks if time is up>>"
                # "Stays in Task 5D until the object is detected"
                # "T: Go back to idle, F: Continue with task\""
                # ">> Manual override >>"
                n450 = case shown="True" w1152 {
                  tunnel: [w1165 w1171] -> w1161
                  tunnel: w1153 -> [w1163 w1169]
                  frame False {
                    n451 = for {
                      tunnel: string[] ["START TIMER", "CLOSE CLAW", ""] ("element") -> [w1166] mode=indexing
                      shift-right: [w1168] -> w1165
                      shift-left: w1163 -> [w1167]
                      n452 = Enqueue Element(queue=w1167, element=w1166) -> (queue out=w1168:refnum<queue>)  [unwired: 2 in, 2 out]
                    }
                  }
                  frame True {
                    n453 = for {
                      shift-right: [w1173] -> w1171
                      shift-left: w1169 -> [w1174]
                      tunnel: string[] ["READ STEPPER VALUES", "ZSTEPPER BOX HEIGHT", ""] -> [w1172] mode=indexing
                      n454 = Enqueue Element(queue=w1174, element=w1172) -> (queue out=w1173:refnum<queue>)  [unwired: 2 in, 2 out]
                    }
                  }
                }
                n455 = Or(x=w1152, y=w1157) -> (x .or. y?=w1159:bool)
                n456 = Select(t=State_Type_Definitions,_for_0.26g_versions_and_later_3."True Stop" ("Enum"), s=w1157, f=State_Type_Definitions,_for_0.26g_versions_and_later_3."Task 5E: GOING UP" ("Enum")) -> (s? t:f=w1154:T18)
                n457 = Select(t=w1154, s=w1159, f=State_Type_Definitions,_for_0.26g_versions_and_later_3."Task 5D: GRAB" ("Enum")) -> (s? t:f=w1158:T18)
              }
              frame "Exit" {
                n458 = for {
                  shift-right: [w1181] -> w1178
                  shift-left: w1175 -> [w1182]
                  tunnel: string[] ["STOP", "RESET ENCODERS", "RESET YAW", "ARDUINO MODE 0"] -> [w1180] mode=indexing
                  n459 = Enqueue Element(queue=w1182, element=w1180) -> (queue out=w1181:refnum<queue>)  [unwired: 2 in, 2 out]
                }
              }
            }
          }
          frame "Task 5E: GOING UP" {
            # ">>> Motor control cluster >>>"
            # ">>> yStepper command>>>"
            n460 = Equal?(x=w1185, y=u8 50) -> (x = y?=w1183:bool)
            n461 = Dequeue Element(queue=w1193, timeout in ms (-1)=w1194, error in (no error)=w1195) -> (element=w1197:T10)  [unwired: 3 out]
            n462 = case shown="\"Start Task 1\", Default" w1197 {
              tunnel: [w1205 State_Type_Definitions,_for_0.26g_versions_and_later_3."True Stop" ("Enum")] -> w1191
              tunnel: [w1207 w1224] -> w1189
              tunnel: [State_Type_Definitions,_for_0.26g_versions_and_later_3."Idle" ("Enum") State_Type_Definitions,_for_0.26g_versions_and_later_3."Shutdown" ("Enum")] -> w1190
              tunnel: w1196 -> [w1204 _]
              tunnel: w1192 -> [w1200 w1221]
              tunnel: w1183 -> [w1199 _]
              frame "Start Task 1", Default {
                # ">> T: Breaks out of state loop; F: Stays in loop>>"
                # ">> Manual override >>"
                # ">> Checks if time is up>>"
                # "Stays in Task 5D until the object is detected"
                # "T: Go back to idle, F: Continue with task\""
                # ">> Manual override >>"
                n463 = Or(x=w1199, y=w1204) -> (x .or. y?=w1198:bool)
                n464 = case shown="False" w1198 {
                  tunnel: [w1211 w1217] -> w1207
                  tunnel: w1200 -> [w1209 w1215]
                  frame False {
                    n465 = for {
                      tunnel: string[] ["READ STEPPER VALUES", "ZSTEPPER BOX HEIGHT", ""] ("element") -> [w1212] mode=indexing
                      shift-right: [w1214] -> w1211
                      shift-left: w1209 -> [w1213]
                      n466 = Enqueue Element(queue=w1213, element=w1212) -> (queue out=w1214:refnum<queue>)  [unwired: 2 in, 2 out]
                    }
                  }
                  frame True {
                    n467 = for {
                      shift-right: [w1219] -> w1217
                      shift-left: w1215 -> [w1220]
                      tunnel: string[] ["CAM CLOSE", "DISPOSE BUFFERS", ""] -> [w1218] mode=indexing
                      n468 = Enqueue Element(queue=w1220, element=w1218) -> (queue out=w1219:refnum<queue>)  [unwired: 2 in, 2 out]
                    }
                  }
                }
                n469 = Select(t=State_Type_Definitions,_for_0.26g_versions_and_later_3."True Stop" ("Enum"), s=w1204, f=State_Type_Definitions,_for_0.26g_versions_and_later_3."True Stop" ("Enum")) -> (s? t:f=w1201:T18)
                n470 = Select(t=w1201, s=w1198, f=State_Type_Definitions,_for_0.26g_versions_and_later_3."Task 5E: GOING UP" ("Enum")) -> (s? t:f=w1205:T18)
              }
              frame "Exit" {
                n471 = for {
                  shift-right: [w1227] -> w1224
                  shift-left: w1221 -> [w1228]
                  tunnel: string[] ["STOP", "RESET ENCODERS", "RESET YAW", "ARDUINO MODE 0"] -> [w1226] mode=indexing
                  n472 = Enqueue Element(queue=w1228, element=w1226) -> (queue out=w1227:refnum<queue>)  [unwired: 2 in, 2 out]
                }
              }
            }
          }
          frame "Task 5F: ARM GRAB HEIGHT" {
            # ">>> Motor control cluster >>>"
            # ">>> yStepper command>>>"
            # ">> Manual override >>"
            n473 = Dequeue Element(queue=w1239, timeout in ms (-1)=w1238, error in (no error)=w1240) -> (element=w1237:T10)  [unwired: 3 out]
            n474 = Equal?(x=w1236, y=u8 1) -> (x = y?=w1234:bool)
            n475 = case shown="\"Start Task 1\", Default" w1237 {
              tunnel: [w1250 State_Type_Definitions,_for_0.26g_versions_and_later_3."True Stop" ("Enum")] -> w1241
              tunnel: [w1253 w1270] -> w1242
              tunnel: [State_Type_Definitions,_for_0.26g_versions_and_later_3."Idle" ("Enum") State_Type_Definitions,_for_0.26g_versions_and_later_3."Shutdown" ("Enum")] -> w1243
              tunnel: w1234 -> [w1249 _]
              tunnel: w1233 -> [w1248 _]
              tunnel: w1232 -> [w1244 w1267]
              frame "Start Task 1", Default {
                # "Stays in Task 5F until stepper reaches desired \nheight"
                # "T: Go back to idle, F: Continue with task\""
                # ">> Manual override >>"
                n476 = case shown="True" w1249 {
                  tunnel: [w1257 w1263] -> w1253
                  tunnel: w1244 -> [w1255 w1261]
                  frame False {
                    n477 = for {
                      tunnel: string[] ["Z STEPPER GRAB HEIGHT", "READ STEPPER VALUES"] ("element") -> [w1258] mode=indexing
                      shift-right: [w1260] -> w1257
                      shift-left: w1255 -> [w1259]
                      n478 = Enqueue Element(queue=w1259, element=w1258) -> (queue out=w1260:refnum<queue>)  [unwired: 2 in, 2 out]
                    }
                  }
                  frame True {
                    n479 = for {
                      shift-right: [w1265] -> w1263
                      shift-left: w1261 -> [w1266]
                      tunnel: string[] ["RESET YAW", "RESET ENCODERS", "RESET FLAGS"] -> [w1264] mode=indexing
                      n480 = Enqueue Element(queue=w1266, element=w1264) -> (queue out=w1265:refnum<queue>)  [unwired: 2 in, 2 out]
                    }
                  }
                }
                n481 = Or(x=w1249, y=w1248) -> (x .or. y?=w1251:bool)
                n482 = Select(t=State_Type_Definitions,_for_0.26g_versions_and_later_3."True Stop" ("Enum"), s=w1248, f=State_Type_Definitions,_for_0.26g_versions_and_later_3."True Stop" ("Enum")) -> (s? t:f=w1245:T18)
                n483 = Select(t=w1245, s=w1251, f=State_Type_Definitions,_for_0.26g_versions_and_later_3."Task 5F: ARM GRAB HEIGHT" ("Enum")) -> (s? t:f=w1250:T18)
              }
              frame "Exit" {
                n484 = for {
                  shift-right: [w1273] -> w1270
                  shift-left: w1267 -> [w1274]
                  tunnel: string[] ["STOP", "RESET ENCODERS", "RESET YAW", "ARDUINO MODE 0"] -> [w1272] mode=indexing
                  n485 = Enqueue Element(queue=w1274, element=w1272) -> (queue out=w1273:refnum<queue>)  [unwired: 2 in, 2 out]
                }
              }
            }
          }
          frame "Task 5G: CLOSE CLAW" {
            # ">>> yStepper command>>>"
            # ">> Manual override >>"
            n486 = Dequeue Element(queue=w1285, timeout in ms (-1)=w1284, error in (no error)=w1283) -> (element=w1282:T10)  [unwired: 3 out]
            n487 = case shown="\"Start Task 1\", Default" w1282 {
              tunnel: [w1294 State_Type_Definitions,_for_0.26g_versions_and_later_3."True Stop" ("Enum")] -> w1287
              tunnel: [w1297 w1314] -> w1280
              tunnel: [State_Type_Definitions,_for_0.26g_versions_and_later_3."Idle" ("Enum") State_Type_Definitions,_for_0.26g_versions_and_later_3."Shutdown" ("Enum")] -> w1279
              tunnel: w1281 -> [w1288 _]
              tunnel: w1286 -> [w1293 w1311]
              tunnel: w1277 -> [w1292 _]
              frame "Start Task 1", Default {
                # ">> Is time up? >>"
                # "Determines if object is in range to pick up"
                # ">> Manual override >>"
                n488 = case shown="True" w1292 {
                  tunnel: [w1301 w1307] -> w1297
                  tunnel: w1293 -> [w1299 w1305]
                  frame False {
                    n489 = for {
                      tunnel: string[] ["CLOSE CLAW", "START TIMER"] ("element") -> [w1302] mode=indexing
                      shift-right: [w1304] -> w1301
                      shift-left: w1299 -> [w1303]
                      n490 = Enqueue Element(queue=w1303, element=w1302) -> (queue out=w1304:refnum<queue>)  [unwired: 2 in, 2 out]
                    }
                  }
                  frame True {
                    n491 = for {
                      shift-right: [w1309] -> w1307
                      shift-left: w1305 -> [w1310]
                      tunnel: string[] ["READ STEPPER VALUES", "", ""] -> [w1308] mode=indexing
                      n492 = Enqueue Element(queue=w1310, element=w1308) -> (queue out=w1309:refnum<queue>)  [unwired: 2 in, 2 out]
                    }
                  }
                }
                n493 = Or(x=w1292, y=w1288) -> (x .or. y?=w1295:bool)
                n494 = Select(t=State_Type_Definitions,_for_0.26g_versions_and_later_3."True Stop" ("Enum"), s=w1288, f=State_Type_Definitions,_for_0.26g_versions_and_later_3."Task 5H: RAISE ARM" ("Enum")) -> (s? t:f=w1290:T18)
                n495 = Select(t=w1290, s=w1295, f=State_Type_Definitions,_for_0.26g_versions_and_later_3."Task 5G: CLOSE CLAW" ("Enum")) -> (s? t:f=w1294:T18)
              }
              frame "Exit" {
                n496 = for {
                  shift-right: [w1317] -> w1314
                  shift-left: w1311 -> [w1318]
                  tunnel: string[] ["STOP", "RESET ENCODERS", "RESET YAW", "ARDUINO MODE 0"] -> [w1316] mode=indexing
                  n497 = Enqueue Element(queue=w1318, element=w1316) -> (queue out=w1317:refnum<queue>)  [unwired: 2 in, 2 out]
                }
              }
            }
          }
          frame "Task 5H: RAISE ARM" {
            # ">>> yStepper command>>>"
            # ">> Manual override >>"
            n498 = Dequeue Element(queue=w1329, timeout in ms (-1)=w1328, error in (no error)=w1330) -> (element=w1327:T10)  [unwired: 3 out]
            n499 = Equal?(x=w1326, y=u8 60) -> (x = y?=w1324:bool)
            n500 = case shown="\"Start Task 1\", Default" w1327 {
              tunnel: [w1340 State_Type_Definitions,_for_0.26g_versions_and_later_3."True Stop" ("Enum")] -> w1331
              tunnel: [w1343 w1360] -> w1332
              tunnel: [State_Type_Definitions,_for_0.26g_versions_and_later_3."Idle" ("Enum") State_Type_Definitions,_for_0.26g_versions_and_later_3."Shutdown" ("Enum")] -> w1333
              tunnel: w1324 -> [w1339 _]
              tunnel: w1323 -> [w1338 _]
              tunnel: w1322 -> [w1334 w1357]
              frame "Start Task 1", Default {
                # "Stays in Task 5_A until stepper reaches desired \nheight"
                # "T: Go back to idle, F: Continue with task\""
                # ">> Manual override >>"
                n501 = case shown="False" w1339 {
                  tunnel: [w1347 w1353] -> w1343
                  tunnel: w1334 -> [w1345 w1351]
                  frame False {
                    n502 = for {
                      tunnel: string[] ["Z STEPPER CAM HEIGHT", "READ STEPPER VALUES"] ("element") -> [w1348] mode=indexing
                      shift-right: [w1350] -> w1347
                      shift-left: w1345 -> [w1349]
                      n503 = Enqueue Element(queue=w1349, element=w1348) -> (queue out=w1350:refnum<queue>)  [unwired: 2 in, 2 out]
                    }
                  }
                  frame True {
                    n504 = for {
                      shift-right: [w1355] -> w1353
                      shift-left: w1351 -> [w1356]
                      tunnel: string[] ["ARDUINO - ULTRASONIC", "READ ULTRASONIC", ""] -> [w1354] mode=indexing
                      n505 = Enqueue Element(queue=w1356, element=w1354) -> (queue out=w1355:refnum<queue>)  [unwired: 2 in, 2 out]
                    }
                  }
                }
                n506 = Or(x=w1339, y=w1338) -> (x .or. y?=w1341:bool)
                n507 = Select(t=State_Type_Definitions,_for_0.26g_versions_and_later_3."True Stop" ("Enum"), s=w1338, f=State_Type_Definitions,_for_0.26g_versions_and_later_3."True Stop" ("Enum")) -> (s? t:f=w1335:T18)
                n508 = Select(t=w1335, s=w1341, f=State_Type_Definitions,_for_0.26g_versions_and_later_3."Task 5H: RAISE ARM" ("Enum")) -> (s? t:f=w1340:T18)
              }
              frame "Exit" {
                n509 = for {
                  shift-right: [w1363] -> w1360
                  shift-left: w1357 -> [w1364]
                  tunnel: string[] ["STOP", "RESET ENCODERS", "RESET YAW", "ARDUINO MODE 0"] -> [w1362] mode=indexing
                  n510 = Enqueue Element(queue=w1364, element=w1362) -> (queue out=w1363:refnum<queue>)  [unwired: 2 in, 2 out]
                }
              }
            }
          }
          frame "Task 6A: RAISE ARM" {
            # ">>> Motor control cluster >>>"
            # ">>> yStepper command>>>"
            n511 = Equal?(x=w1372, y=u8 60) -> (x = y?=w1366:bool)
            n512 = Dequeue Element(queue=w1376, timeout in ms (-1)=w1375, error in (no error)=w1374) -> (element=w1381:T10)  [unwired: 3 out]
            n513 = local read "Rising Edge"() -> (w1367:bool)
            n514 = And(x=w1367, y=w1366) -> (x .and. y?=w1365:bool)
            n515 = case shown="\"Start Task 1\", Default" w1381 {
              tunnel: [w1391 State_Type_Definitions,_for_0.26g_versions_and_later_3."True Stop" ("Enum")] -> w1379
              tunnel: [w1390 w1407] -> w1378
              tunnel: [State_Type_Definitions,_for_0.26g_versions_and_later_3."Idle" ("Enum") State_Type_Definitions,_for_0.26g_versions_and_later_3."Shutdown" ("Enum")] -> w1380
              tunnel: w1377 -> [w1387 _]
              tunnel: w1373 -> [w1388 _]
              tunnel: w1365 -> [w1385 _]
              frame "Start Task 1", Default {
                n516 = Or(x=w1385, y=w1387) -> (x .or. y?=w1382:bool)
                n517 = case shown="False" w1382 {
                  tunnel: [w1395 w1401] -> w1390
                  tunnel: w1388 -> [w1393 w1400]
                  frame False {
                    n518 = for {
                      tunnel: string[] ["Z STEPPER CAM HEIGHT", "READ STEPPER VALUES"] ("element") -> [w1396] mode=indexing
                      shift-right: [w1398] -> w1395
                      shift-left: w1393 -> [w1397]
                      n519 = Enqueue Element(queue=w1397, element=w1396) -> (queue out=w1398:refnum<queue>)  [unwired: 2 in, 2 out]
                    }
                  }
                  frame True {
                    n520 = for {
                      shift-right: [w1403] -> w1401
                      shift-left: w1400 -> [w1404]
                      tunnel: string[] ["OPEN LOG CAM", "SET TIMER 2", "OPEN IMAQ REF", "", ""] -> [w1402] mode=indexing
                      n521 = Enqueue Element(queue=w1404, element=w1402) -> (queue out=w1403:refnum<queue>)  [unwired: 2 in, 2 out]
                    }
                  }
                }
                n522 = Select(t=State_Type_Definitions,_for_0.26g_versions_and_later_3."Task 6B: CAM BURST" ("Enum"), s=w1385, f=State_Type_Definitions,_for_0.26g_versions_and_later_3."True Stop" ("Enum")) -> (s? t:f=w1383:T18)
                n523 = Select(t=w1383, s=w1382, f=State_Type_Definitions,_for_0.26g_versions_and_later_3."Task 6A: RAISE ARM" ("Enum")) -> (s? t:f=w1391:T18)
              }
              frame "Exit" {
                n524 = for {
                  shift-right: [w1410] -> w1407
                  shift-left: _ -> [w1411]
                  tunnel: string[] ["STOP", "RESET ENCODERS", "RESET YAW", "ARDUINO MODE 0"] -> [w1409] mode=indexing
                  n525 = Enqueue Element(queue=w1411, element=w1409) -> (queue out=w1410:refnum<queue>)  [unwired: 2 in, 2 out]
                }
              }
            }
          }
          frame "Task 6B: CAM BURST" {
            # ">> Manual override >>"
            # ">>> Motor control cluster >>>"
            # ">>> yStepper command>>>"
            n526 = Dequeue Element(queue=w1423, timeout in ms (-1)=w1421, error in (no error)=w1422) -> (element=w1420:T10)  [unwired: 3 out]
            n527 = case shown="\"Start Task 1\", Default" w1420 {
              tunnel: [w1431 State_Type_Definitions,_for_0.26g_versions_and_later_3."True Stop" ("Enum")] -> w1417
              tunnel: [w1429 w1449] -> w1424
              tunnel: [State_Type_Definitions,_for_0.26g_versions_and_later_3."Idle" ("Enum") State_Type_Definitions,_for_0.26g_versions_and_later_3."Shutdown" ("Enum")] -> w1418
              tunnel: w1419 -> [w1427 _]
              tunnel: w1416 -> [w1428 w1446]
              tunnel: w1412 -> [w1425 _]
              frame "Start Task 1", Default {
                n528 = Or(x=w1425, y=w1427) -> (x .or. y?=w1426:bool)
                n529 = case shown="True" w1426 {
                  tunnel: [w1436 w1442] -> w1429
                  tunnel: w1428 -> [w1434 w1440]
                  frame False {
                    n530 = for {
                      tunnel: string[] ["CAM ACQ", "START TIMER"] ("element") -> [w1437] mode=indexing
                      shift-right: [w1439] -> w1436
                      shift-left: w1434 -> [w1438]
                      n531 = Enqueue Element(queue=w1438, element=w1437) -> (queue out=w1439:refnum<queue>)  [unwired: 2 in, 2 out]
                    }
                  }
                  frame True {
                    n532 = for {
                      shift-right: [w1444] -> w1442
                      shift-left: w1440 -> [w1445]
                      tunnel: string[] ["CAM CLOSE", "PROCESS IMAGE", "SET TIMER 2", "RESET ENCODERS"] -> [w1443] mode=indexing
                      n533 = Enqueue Element(queue=w1445, element=w1443) -> (queue out=w1444:refnum<queue>)  [unwired: 2 in, 2 out]
                    }
                  }
                }
                n534 = Select(t=State_Type_Definitions,_for_0.26g_versions_and_later_3."Task 6C: PROCESS IMAGE" ("Enum"), s=w1426, f=State_Type_Definitions,_for_0.26g_versions_and_later_3."Task 6B: CAM BURST" ("Enum")) -> (s? t:f=w1431:T18)
              }
              frame "Exit" {
                # ">> State after true stop >>"
                # ">> Goes to true stop >>"
                n535 = for {
                  shift-right: [w1452] -> w1449
                  shift-left: w1446 -> [w1453]
                  tunnel: string[] ["STOP", "RESET ENCODERS", "RESET YAW", ""] -> [w1451] mode=indexing
                  n536 = Enqueue Element(queue=w1453, element=w1451) -> (queue out=w1452:refnum<queue>)  [unwired: 2 in, 2 out]
                }
              }
            }
          }
          frame "Task 6C: PROCESS IMAGE" {
            # "Ball > Soap > Gel > Pipe"
            # ">>> Motor control cluster >>>"
            # ">>> yStepper command>>>"
            n537 = Dequeue Element(queue=w1462, timeout in ms (-1)=w1461, error in (no error)=w1460) -> (element=w1459:T10)  [unwired: 3 out]
            n538 = case shown="\"Start Task 1\", Default" w1459 {
              tunnel: [w1478 State_Type_Definitions,_for_0.26g_versions_and_later_3."True Stop" ("Enum")] -> w1466
              tunnel: [w1480 w1497] -> w1465
              tunnel: [State_Type_Definitions,_for_0.26g_versions_and_later_3."Idle" ("Enum") State_Type_Definitions,_for_0.26g_versions_and_later_3."Shutdown" ("Enum")] -> w1467
              tunnel: w1463 -> [w1469 _]
              tunnel: w1464 -> [w1475 w1494]
              tunnel: w1455 -> [w1473 _]
              tunnel: w1454 -> [w1474 _]
              frame "Start Task 1", Default {
                # "Stays in Task 5D until the object is detected"
                n539 = Or(x=w1473, y=w1469) -> (x .or. y?=w1472:bool)
                n540 = case shown="True" w1472 {
                  tunnel: [w1484 w1490] -> w1480
                  tunnel: w1475 -> [w1482 w1488]
                  frame False {
                    n541 = for {
                      tunnel: string[] ["START TIMER", "PROCESS IMAGE", ""] ("element") -> [w1485] mode=indexing
                      shift-right: [w1487] -> w1484
                      shift-left: w1482 -> [w1486]
                      n542 = Enqueue Element(queue=w1486, element=w1485) -> (queue out=w1487:refnum<queue>)  [unwired: 2 in, 2 out]
                    }
                  }
                  frame True {
                    n543 = for {
                      shift-right: [w1492] -> w1490
                      shift-left: w1488 -> [w1493]
                      tunnel: string[] ["RESET ENCODERS", "RESET YAW", ""] -> [w1491] mode=indexing
                      n544 = Enqueue Element(queue=w1493, element=w1491) -> (queue out=w1492:refnum<queue>)  [unwired: 2 in, 2 out]
                    }
                  }
                }
                n545 = Select(t=State_Type_Definitions,_for_0.26g_versions_and_later_3."Task 6D: BALL BUSTER" ("Enum"), s=w1474, f=State_Type_Definitions,_for_0.26g_versions_and_later_3."Task 6F: CAM BURST 2" ("Enum")) -> (s? t:f=w1470:T18)
                n546 = Select(t=State_Type_Definitions,_for_0.26g_versions_and_later_3."True Stop" ("Enum"), s=w1469, f=w1470) -> (s? t:f=w1476:T18)
                n547 = Select(t=w1476, s=w1472, f=State_Type_Definitions,_for_0.26g_versions_and_later_3."Task 6C: PROCESS IMAGE" ("Enum")) -> (s? t:f=w1478:T18)
              }
              frame "Exit" {
                n548 = for {
                  shift-right: [w1500] -> w1497
                  shift-left: w1494 -> [w1501]
                  tunnel: string[] ["STOP", "RESET ENCODERS", "RESET YAW", "ARDUINO MODE 0"] -> [w1499] mode=indexing
                  n549 = Enqueue Element(queue=w1501, element=w1499) -> (queue out=w1500:refnum<queue>)  [unwired: 2 in, 2 out]
                }
              }
            }
          }
          frame "Task 6D: BALL BUSTER" {
            # "Ball > Soap > Gel > Pipe"
            # ">>> Motor control cluster >>>"
            # ">>> yStepper command>>>"
            n550 = Greater Or Equal?(x=w1502, y=20.0) -> (x >= y?=w1503:bool)
            n551 = Dequeue Element(queue=w1511, timeout in ms (-1)=w1510, error in (no error)=w1509) -> (element=w1508:T10)  [unwired: 3 out]
            n552 = case shown="\"Start Task 1\", Default" w1508 {
              tunnel: [w1524 State_Type_Definitions,_for_0.26g_versions_and_later_3."True Stop" ("Enum")] -> w1515
              tunnel: [w1526 w1543] -> w1514
              tunnel: [State_Type_Definitions,_for_0.26g_versions_and_later_3."Idle" ("Enum") State_Type_Definitions,_for_0.26g_versions_and_later_3."Shutdown" ("Enum")] -> w1516
              tunnel: w1512 -> [w1519 _]
              tunnel: w1513 -> [w1521 w1540]
              tunnel: w1503 -> [w1518 _]
              frame "Start Task 1", Default {
                # "Stays in Task 5D until the object is detected"
                n553 = Or(x=w1518, y=w1519) -> (x .or. y?=w1520:bool)
                n554 = case shown="False" w1520 {
                  tunnel: [w1530 w1536] -> w1526
                  tunnel: w1521 -> [w1528 w1534]
                  frame False {
                    n555 = for {
                      tunnel: string[] ["RIGHT", "READ NAVX", "READ ENCODERS"] ("element") -> [w1531] mode=indexing
                      shift-right: [w1533] -> w1530
                      shift-left: w1528 -> [w1532]
                      n556 = Enqueue Element(queue=w1532, element=w1531) -> (queue out=w1533:refnum<queue>)  [unwired: 2 in, 2 out]
                    }
                  }
                  frame True {
                    n557 = for {
                      shift-right: [w1538] -> w1536
                      shift-left: w1534 -> [w1539]
                      tunnel: string[] ["RESET ENCODERS", "RESET YAW", "RESET FLAGS"] -> [w1537] mode=indexing
                      n558 = Enqueue Element(queue=w1539, element=w1537) -> (queue out=w1538:refnum<queue>)  [unwired: 2 in, 2 out]
                    }
                  }
                }
                n559 = Select(t=State_Type_Definitions,_for_0.26g_versions_and_later_3."True Stop" ("Enum"), s=w1519, f=State_Type_Definitions,_for_0.26g_versions_and_later_3."Task 6E: STILL WAITING" ("Enum")) -> (s? t:f=w1522:T18)
                n560 = Select(t=w1522, s=w1520, f=State_Type_Definitions,_for_0.26g_versions_and_later_3."Task 6D: BALL BUSTER" ("Enum")) -> (s? t:f=w1524:T18)
              }
              frame "Exit" {
                n561 = for {
                  shift-right: [w1546] -> w1543
                  shift-left: w1540 -> [w1547]
                  tunnel: string[] ["STOP", "RESET ENCODERS", "RESET YAW", "ARDUINO MODE 0"] -> [w1545] mode=indexing
                  n562 = Enqueue Element(queue=w1547, element=w1545) -> (queue out=w1546:refnum<queue>)  [unwired: 2 in, 2 out]
                }
              }
            }
          }
          frame "Task 6E: STILL WAITING" {
            # "Ball > Soap > Gel > Pipe"
            # ">>> Motor control cluster >>>"
            # ">>> yStepper command>>>"
            n563 = local read "Rising Edge"() -> (w1549:bool)
            n564 = Dequeue Element(queue=w1555, timeout in ms (-1)=w1554, error in (no error)=w1553) -> (element=w1552:T10)  [unwired: 3 out]
            n565 = case shown="\"Start Task 1\", Default" w1552 {
              tunnel: [w1569 State_Type_Definitions,_for_0.26g_versions_and_later_3."True Stop" ("Enum")] -> w1559
              tunnel: [w1562 w1587] -> w1558
              tunnel: [State_Type_Definitions,_for_0.26g_versions_and_later_3."Idle" ("Enum") State_Type_Definitions,_for_0.26g_versions_and_later_3."Shutdown" ("Enum")] -> w1560
              tunnel: w1556 -> [w1566 _]
              tunnel: w1557 -> [w1563 w1584]
              tunnel: w1549 -> [w1564 _]
              frame "Start Task 1", Default {
                # "Stays in Task 5D until the object is detected"
                n566 = Or(x=w1564, y=w1566) -> (x .or. y?=w1561:bool)
                n567 = case shown="False" w1561 {
                  tunnel: [w1574 w1580] -> w1562
                  tunnel: w1563 -> [w1572 w1579]
                  frame False {
                    n568 = for {
                      tunnel: string[] ["Z STEPPER CAM HEIGHT", "READ STEPPER VALUES"] ("element") -> [w1575] mode=indexing
                      shift-right: [w1577] -> w1574
                      shift-left: w1572 -> [w1576]
                      n569 = Enqueue Element(queue=w1576, element=w1575) -> (queue out=w1577:refnum<queue>)  [unwired: 2 in, 2 out]
                    }
                  }
                  frame True {
                    n570 = for {
                      shift-right: [w1582] -> w1580
                      shift-left: w1579 -> [w1583]
                      tunnel: string[] ["OPEN LOG CAM", "SET TIMER 2", "OPEN IMAQ REF", "", ""] -> [w1581] mode=indexing
                      n571 = Enqueue Element(queue=w1583, element=w1581) -> (queue out=w1582:refnum<queue>)  [unwired: 2 in, 2 out]
                    }
                  }
                }
                n572 = Select(t=State_Type_Definitions,_for_0.26g_versions_and_later_3."True Stop" ("Enum"), s=w1566, f=State_Type_Definitions,_for_0.26g_versions_and_later_3."Task 6F: CAM BURST 2" ("Enum")) -> (s? t:f=w1567:T18)
                n573 = Select(t=w1567, s=w1561, f=State_Type_Definitions,_for_0.26g_versions_and_later_3."Task 6E: STILL WAITING" ("Enum")) -> (s? t:f=w1569:T18)
              }
              frame "Exit" {
                n574 = for {
                  shift-right: [w1590] -> w1587
                  shift-left: w1584 -> [w1591]
                  tunnel: string[] ["STOP", "RESET ENCODERS", "RESET YAW", "ARDUINO MODE 0"] -> [w1589] mode=indexing
                  n575 = Enqueue Element(queue=w1591, element=w1589) -> (queue out=w1590:refnum<queue>)  [unwired: 2 in, 2 out]
                }
              }
            }
          }
          frame "Task 6F: CAM BURST 2" {
            # ">> Manual override >>"
            # ">>> Motor control cluster >>>"
            # ">>> yStepper command>>>"
            n576 = Dequeue Element(queue=w1603, timeout in ms (-1)=w1601, error in (no error)=w1602) -> (element=w1600:T10)  [unwired: 3 out]
            n577 = case shown="\"Start Task 1\", Default" w1600 {
              tunnel: [w1611 State_Type_Definitions,_for_0.26g_versions_and_later_3."True Stop" ("Enum")] -> w1597
              tunnel: [w1609 w1629] -> w1604
              tunnel: [State_Type_Definitions,_for_0.26g_versions_and_later_3."Idle" ("Enum") State_Type_Definitions,_for_0.26g_versions_and_later_3."Shutdown" ("Enum")] -> w1598
              tunnel: w1599 -> [w1607 _]
              tunnel: w1596 -> [w1608 w1626]
              tunnel: w1592 -> [w1605 _]
              frame "Start Task 1", Default {
                n578 = Or(x=w1605, y=w1607) -> (x .or. y?=w1606:bool)
                n579 = case shown="True" w1606 {
                  tunnel: [w1616 w1622] -> w1609
                  tunnel: w1608 -> [w1614 w1620]
                  frame False {
                    n580 = for {
                      tunnel: string[] ["CAM ACQ", "START TIMER"] ("element") -> [w1617] mode=indexing
                      shift-right: [w1619] -> w1616
                      shift-left: w1614 -> [w1618]
                      n581 = Enqueue Element(queue=w1618, element=w1617) -> (queue out=w1619:refnum<queue>)  [unwired: 2 in, 2 out]
                    }
                  }
                  frame True {
                    n582 = for {
                      shift-right: [w1624] -> w1622
                      shift-left: w1620 -> [w1625]
                      tunnel: string[] ["CAM CLOSE", "PROCESS IMAGE", "SET TIMER 2", "RESET ENCODERS"] -> [w1623] mode=indexing
                      n583 = Enqueue Element(queue=w1625, element=w1623) -> (queue out=w1624:refnum<queue>)  [unwired: 2 in, 2 out]
                    }
                  }
                }
                n584 = Select(t=State_Type_Definitions,_for_0.26g_versions_and_later_3."Task 6G: PROCESS IMAGE 2" ("Enum"), s=w1606, f=State_Type_Definitions,_for_0.26g_versions_and_later_3."Task 6F: CAM BURST 2" ("Enum")) -> (s? t:f=w1611:T18)
              }
              frame "Exit" {
                # ">> State after true stop >>"
                # ">> Goes to true stop >>"
                n585 = for {
                  shift-right: [w1632] -> w1629
                  shift-left: w1626 -> [w1633]
                  tunnel: string[] ["STOP", "RESET ENCODERS", "RESET YAW", ""] -> [w1631] mode=indexing
                  n586 = Enqueue Element(queue=w1633, element=w1631) -> (queue out=w1632:refnum<queue>)  [unwired: 2 in, 2 out]
                }
              }
            }
          }
          frame "Task 6G: PROCESS IMAGE 2" {
            # "Ball > Soap > Gel > Pipe"
            # ">>> Motor control cluster >>>"
            # ">>> yStepper command>>>"
            n587 = Dequeue Element(queue=w1642, timeout in ms (-1)=w1641, error in (no error)=w1640) -> (element=w1639:T10)  [unwired: 3 out]
            n588 = case shown="\"Start Task 1\", Default" w1639 {
              tunnel: [w1658 State_Type_Definitions,_for_0.26g_versions_and_later_3."True Stop" ("Enum")] -> w1646
              tunnel: [w1660 w1677] -> w1645
              tunnel: [State_Type_Definitions,_for_0.26g_versions_and_later_3."Idle" ("Enum") State_Type_Definitions,_for_0.26g_versions_and_later_3."Shutdown" ("Enum")] -> w1647
              tunnel: w1643 -> [w1649 _]
              tunnel: w1644 -> [w1655 w1674]
              tunnel: w1635 -> [w1653 _]
              tunnel: w1634 -> [w1654 _]
              frame "Start Task 1", Default {
                # "Stays in Task 5D until the object is detected"
                n589 = Or(x=w1653, y=w1649) -> (x .or. y?=w1652:bool)
                n590 = case shown="True" w1652 {
                  tunnel: [w1664 w1670] -> w1660
                  tunnel: w1655 -> [w1662 w1668]
                  frame False {
                    n591 = for {
                      tunnel: string[] ["START TIMER", "PROCESS IMAGE", ""] ("element") -> [w1665] mode=indexing
                      shift-right: [w1667] -> w1664
                      shift-left: w1662 -> [w1666]
                      n592 = Enqueue Element(queue=w1666, element=w1665) -> (queue out=w1667:refnum<queue>)  [unwired: 2 in, 2 out]
                    }
                  }
                  frame True {
                    n593 = for {
                      shift-right: [w1672] -> w1670
                      shift-left: w1668 -> [w1673]
                      tunnel: string[] ["RESET ENCODERS", "RESET YAW", ""] -> [w1671] mode=indexing
                      n594 = Enqueue Element(queue=w1673, element=w1671) -> (queue out=w1672:refnum<queue>)  [unwired: 2 in, 2 out]
                    }
                  }
                }
                n595 = Select(t=State_Type_Definitions,_for_0.26g_versions_and_later_3."Task 6H: SKADI SOAPS" ("Enum"), s=w1654, f=State_Type_Definitions,_for_0.26g_versions_and_later_3."Task 6J: CAM BURST 3" ("Enum")) -> (s? t:f=w1650:T18)
                n596 = Select(t=State_Type_Definitions,_for_0.26g_versions_and_later_3."True Stop" ("Enum"), s=w1649, f=w1650) -> (s? t:f=w1656:T18)
                n597 = Select(t=w1656, s=w1652, f=State_Type_Definitions,_for_0.26g_versions_and_later_3."Task 6G: PROCESS IMAGE 2" ("Enum")) -> (s? t:f=w1658:T18)
              }
              frame "Exit" {
                n598 = for {
                  shift-right: [w1680] -> w1677
                  shift-left: w1674 -> [w1681]
                  tunnel: string[] ["STOP", "RESET ENCODERS", "RESET YAW", "ARDUINO MODE 0"] -> [w1679] mode=indexing
                  n599 = Enqueue Element(queue=w1681, element=w1679) -> (queue out=w1680:refnum<queue>)  [unwired: 2 in, 2 out]
                }
              }
            }
          }
          frame "Task 6H: SKADI SOAPS" {
            # "Ball > Soap > Gel > Pipe"
            # ">>> Motor control cluster >>>"
            # ">>> yStepper command>>>"
            n600 = Less Or Equal?(x=w1682, y=-20.0) -> (x <= y?=w1683:bool)
            n601 = Dequeue Element(queue=w1691, timeout in ms (-1)=w1690, error in (no error)=w1689) -> (element=w1688:T10)  [unwired: 3 out]
            n602 = case shown="\"Start Task 1\", Default" w1688 {
              tunnel: [w1704 State_Type_Definitions,_for_0.26g_versions_and_later_3."True Stop" ("Enum")] -> w1695
              tunnel: [w1706 w1723] -> w1694
              tunnel: [State_Type_Definitions,_for_0.26g_versions_and_later_3."Idle" ("Enum") State_Type_Definitions,_for_0.26g_versions_and_later_3."Shutdown" ("Enum")] -> w1696
              tunnel: w1692 -> [w1699 _]
              tunnel: w1693 -> [w1701 w1720]
              tunnel: w1683 -> [w1698 _]
              frame "Start Task 1", Default {
                # "Stays in Task 5D until the object is detected"
                n603 = Or(x=w1698, y=w1699) -> (x .or. y?=w1700:bool)
                n604 = case shown="False" w1700 {
                  tunnel: [w1710 w1716] -> w1706
                  tunnel: w1701 -> [w1708 w1714]
                  frame False {
                    n605 = for {
                      tunnel: string[] ["LEFT", "READ NAVX", "READ ENCODERS"] ("element") -> [w1711] mode=indexing
                      shift-right: [w1713] -> w1710
                      shift-left: w1708 -> [w1712]
                      n606 = Enqueue Element(queue=w1712, element=w1711) -> (queue out=w1713:refnum<queue>)  [unwired: 2 in, 2 out]
                    }
                  }
                  frame True {
                    n607 = for {
                      shift-right: [w1718] -> w1716
                      shift-left: w1714 -> [w1719]
                      tunnel: string[] ["RESET ENCODERS", "RESET YAW", "RESET FLAGS"] -> [w1717] mode=indexing
                      n608 = Enqueue Element(queue=w1719, element=w1717) -> (queue out=w1718:refnum<queue>)  [unwired: 2 in, 2 out]
                    }
                  }
                }
                n609 = Select(t=State_Type_Definitions,_for_0.26g_versions_and_later_3."True Stop" ("Enum"), s=w1699, f=State_Type_Definitions,_for_0.26g_versions_and_later_3."Task 6I: STILL WAITING 2" ("Enum")) -> (s? t:f=w1702:T18)
                n610 = Select(t=w1702, s=w1700, f=State_Type_Definitions,_for_0.26g_versions_and_later_3."Task 6H: SKADI SOAPS" ("Enum")) -> (s? t:f=w1704:T18)
              }
              frame "Exit" {
                n611 = for {
                  shift-right: [w1726] -> w1723
                  shift-left: w1720 -> [w1727]
                  tunnel: string[] ["STOP", "RESET ENCODERS", "RESET YAW", "ARDUINO MODE 0"] -> [w1725] mode=indexing
                  n612 = Enqueue Element(queue=w1727, element=w1725) -> (queue out=w1726:refnum<queue>)  [unwired: 2 in, 2 out]
                }
              }
            }
          }
          frame "Task 6I: STILL WAITING 2" {
            # "Ball > Soap > Gel > Pipe"
            # ">>> Motor control cluster >>>"
            # ">>> yStepper command>>>"
            n613 = local read "Rising Edge"() -> (w1729:bool)
            n614 = Dequeue Element(queue=w1735, timeout in ms (-1)=w1734, error in (no error)=w1733) -> (element=w1732:T10)  [unwired: 3 out]
            n615 = case shown="\"Start Task 1\", Default" w1732 {
              tunnel: [w1749 State_Type_Definitions,_for_0.26g_versions_and_later_3."True Stop" ("Enum")] -> w1739
              tunnel: [w1742 w1767] -> w1738
              tunnel: [State_Type_Definitions,_for_0.26g_versions_and_later_3."Idle" ("Enum") State_Type_Definitions,_for_0.26g_versions_and_later_3."Shutdown" ("Enum")] -> w1740
              tunnel: w1736 -> [w1746 _]
              tunnel: w1737 -> [w1743 w1764]
              tunnel: w1729 -> [w1744 _]
              frame "Start Task 1", Default {
                # "Stays in Task 5D until the object is detected"
                n616 = Or(x=w1744, y=w1746) -> (x .or. y?=w1741:bool)
                n617 = case shown="False" w1741 {
                  tunnel: [w1754 w1760] -> w1742
                  tunnel: w1743 -> [w1752 w1759]
                  frame False {
                    n618 = for {
                      tunnel: string[] ["Z STEPPER CAM HEIGHT", "READ STEPPER VALUES"] ("element") -> [w1755] mode=indexing
                      shift-right: [w1757] -> w1754
                      shift-left: w1752 -> [w1756]
                      n619 = Enqueue Element(queue=w1756, element=w1755) -> (queue out=w1757:refnum<queue>)  [unwired: 2 in, 2 out]
                    }
                  }
                  frame True {
                    n620 = for {
                      shift-right: [w1762] -> w1760
                      shift-left: w1759 -> [w1763]
                      tunnel: string[] ["OPEN LOG CAM", "SET TIMER 2", "OPEN IMAQ REF", "", ""] -> [w1761] mode=indexing
                      n621 = Enqueue Element(queue=w1763, element=w1761) -> (queue out=w1762:refnum<queue>)  [unwired: 2 in, 2 out]
                    }
                  }
                }
                n622 = Select(t=State_Type_Definitions,_for_0.26g_versions_and_later_3."True Stop" ("Enum"), s=w1746, f=State_Type_Definitions,_for_0.26g_versions_and_later_3."Task 6J: CAM BURST 3" ("Enum")) -> (s? t:f=w1747:T18)
                n623 = Select(t=w1747, s=w1741, f=State_Type_Definitions,_for_0.26g_versions_and_later_3."Task 6I: STILL WAITING 2" ("Enum")) -> (s? t:f=w1749:T18)
              }
              frame "Exit" {
                n624 = for {
                  shift-right: [w1770] -> w1767
                  shift-left: w1764 -> [w1771]
                  tunnel: string[] ["STOP", "RESET ENCODERS", "RESET YAW", "ARDUINO MODE 0"] -> [w1769] mode=indexing
                  n625 = Enqueue Element(queue=w1771, element=w1769) -> (queue out=w1770:refnum<queue>)  [unwired: 2 in, 2 out]
                }
              }
            }
          }
          frame "Task 6J: CAM BURST 3" {
            # ">> Manual override >>"
            # ">>> Motor control cluster >>>"
            # ">>> yStepper command>>>"
            n626 = Dequeue Element(queue=w1783, timeout in ms (-1)=w1781, error in (no error)=w1782) -> (element=w1780:T10)  [unwired: 3 out]
            n627 = case shown="\"Start Task 1\", Default" w1780 {
              tunnel: [w1791 State_Type_Definitions,_for_0.26g_versions_and_later_3."True Stop" ("Enum")] -> w1777
              tunnel: [w1789 w1809] -> w1784
              tunnel: [State_Type_Definitions,_for_0.26g_versions_and_later_3."Idle" ("Enum") State_Type_Definitions,_for_0.26g_versions_and_later_3."Shutdown" ("Enum")] -> w1778
              tunnel: w1779 -> [w1787 _]
              tunnel: w1776 -> [w1788 w1806]
              tunnel: w1772 -> [w1785 _]
              frame "Start Task 1", Default {
                n628 = Or(x=w1785, y=w1787) -> (x .or. y?=w1786:bool)
                n629 = case shown="True" w1786 {
                  tunnel: [w1796 w1802] -> w1789
                  tunnel: w1788 -> [w1794 w1800]
                  frame False {
                    n630 = for {
                      tunnel: string[] ["CAM ACQ", "START TIMER"] ("element") -> [w1797] mode=indexing
                      shift-right: [w1799] -> w1796
                      shift-left: w1794 -> [w1798]
                      n631 = Enqueue Element(queue=w1798, element=w1797) -> (queue out=w1799:refnum<queue>)  [unwired: 2 in, 2 out]
                    }
                  }
                  frame True {
                    n632 = for {
                      shift-right: [w1804] -> w1802
                      shift-left: w1800 -> [w1805]
                      tunnel: string[] ["CAM CLOSE", "PROCESS IMAGE", "SET TIMER 2", "RESET ENCODERS"] -> [w1803] mode=indexing
                      n633 = Enqueue Element(queue=w1805, element=w1803) -> (queue out=w1804:refnum<queue>)  [unwired: 2 in, 2 out]
                    }
                  }
                }
                n634 = Select(t=State_Type_Definitions,_for_0.26g_versions_and_later_3."Task 6K: PROCESS IMAGE 3" ("Enum"), s=w1786, f=State_Type_Definitions,_for_0.26g_versions_and_later_3."Task 6J: CAM BURST 3" ("Enum")) -> (s? t:f=w1791:T18)
              }
              frame "Exit" {
                # ">> State after true stop >>"
                # ">> Goes to true stop >>"
                n635 = for {
                  shift-right: [w1812] -> w1809
                  shift-left: w1806 -> [w1813]
                  tunnel: string[] ["STOP", "RESET ENCODERS", "RESET YAW", ""] -> [w1811] mode=indexing
                  n636 = Enqueue Element(queue=w1813, element=w1811) -> (queue out=w1812:refnum<queue>)  [unwired: 2 in, 2 out]
                }
              }
            }
          }
          frame "Task 6K: PROCESS IMAGE 3" {
            # "Ball > Soap > Gel > Pipe"
            # ">>> Motor control cluster >>>"
            # ">>> yStepper command>>>"
            n637 = Dequeue Element(queue=w1822, timeout in ms (-1)=w1821, error in (no error)=w1820) -> (element=w1819:T10)  [unwired: 3 out]
            n638 = case shown="\"Start Task 1\", Default" w1819 {
              tunnel: [w1838 State_Type_Definitions,_for_0.26g_versions_and_later_3."True Stop" ("Enum")] -> w1826
              tunnel: [w1840 w1857] -> w1825
              tunnel: [State_Type_Definitions,_for_0.26g_versions_and_later_3."Idle" ("Enum") State_Type_Definitions,_for_0.26g_versions_and_later_3."Shutdown" ("Enum")] -> w1827
              tunnel: w1823 -> [w1829 _]
              tunnel: w1824 -> [w1835 w1854]
              tunnel: w1815 -> [w1833 _]
              tunnel: w1814 -> [w1834 _]
              frame "Start Task 1", Default {
                # "Stays in Task 5D until the object is detected"
                n639 = Or(x=w1833, y=w1829) -> (x .or. y?=w1832:bool)
                n640 = case shown="True" w1832 {
                  tunnel: [w1844 w1850] -> w1840
                  tunnel: w1835 -> [w1842 w1848]
                  frame False {
                    n641 = for {
                      tunnel: string[] ["START TIMER", "PROCESS IMAGE", ""] ("element") -> [w1845] mode=indexing
                      shift-right: [w1847] -> w1844
                      shift-left: w1842 -> [w1846]
                      n642 = Enqueue Element(queue=w1846, element=w1845) -> (queue out=w1847:refnum<queue>)  [unwired: 2 in, 2 out]
                    }
                  }
                  frame True {
                    n643 = for {
                      shift-right: [w1852] -> w1850
                      shift-left: w1848 -> [w1853]
                      tunnel: string[] ["RESET ENCODERS", "RESET YAW", ""] -> [w1851] mode=indexing
                      n644 = Enqueue Element(queue=w1853, element=w1851) -> (queue out=w1852:refnum<queue>)  [unwired: 2 in, 2 out]
                    }
                  }
                }
                n645 = Select(t=State_Type_Definitions,_for_0.26g_versions_and_later_3."Task 6L: JAM IT IN" ("Enum"), s=w1834, f=State_Type_Definitions,_for_0.26g_versions_and_later_3."Task 6N: CAM BURST 4" ("Enum")) -> (s? t:f=w1830:T18)
                n646 = Select(t=State_Type_Definitions,_for_0.26g_versions_and_later_3."True Stop" ("Enum"), s=w1829, f=w1830) -> (s? t:f=w1836:T18)
                n647 = Select(t=w1836, s=w1832, f=State_Type_Definitions,_for_0.26g_versions_and_later_3."Task 6K: PROCESS IMAGE 3" ("Enum")) -> (s? t:f=w1838:T18)
              }
              frame "Exit" {
                n648 = for {
                  shift-right: [w1860] -> w1857
                  shift-left: w1854 -> [w1861]
                  tunnel: string[] ["STOP", "RESET ENCODERS", "RESET YAW", "ARDUINO MODE 0"] -> [w1859] mode=indexing
                  n649 = Enqueue Element(queue=w1861, element=w1859) -> (queue out=w1860:refnum<queue>)  [unwired: 2 in, 2 out]
                }
              }
            }
          }
          frame "Task 6L: JAM IT IN" {
            # "Ball > Soap > Gel > Pipe"
            # ">>> Motor control cluster >>>"
            # ">>> yStepper command>>>"
            n650 = Less Or Equal?(x=w1862, y=-20.0) -> (x <= y?=w1863:bool)
            n651 = Dequeue Element(queue=w1871, timeout in ms (-1)=w1870, error in (no error)=w1869) -> (element=w1868:T10)  [unwired: 3 out]
            n652 = case shown="\"Start Task 1\", Default" w1868 {
              tunnel: [w1884 State_Type_Definitions,_for_0.26g_versions_and_later_3."True Stop" ("Enum")] -> w1875
              tunnel: [w1886 w1903] -> w1874
              tunnel: [State_Type_Definitions,_for_0.26g_versions_and_later_3."Idle" ("Enum") State_Type_Definitions,_for_0.26g_versions_and_later_3."Shutdown" ("Enum")] -> w1876
              tunnel: w1872 -> [w1879 _]
              tunnel: w1873 -> [w1881 w1900]
              tunnel: w1863 -> [w1878 _]
              frame "Start Task 1", Default {
                # "Stays in Task 5D until the object is detected"
                n653 = Or(x=w1878, y=w1879) -> (x .or. y?=w1880:bool)
                n654 = case shown="False" w1880 {
                  tunnel: [w1890 w1896] -> w1886
                  tunnel: w1881 -> [w1888 w1894]
                  frame False {
                    n655 = for {
                      tunnel: string[] ["REVERSE", "READ NAVX", "READ ENCODERS"] ("element") -> [w1891] mode=indexing
                      shift-right: [w1893] -> w1890
                      shift-left: w1888 -> [w1892]
                      n656 = Enqueue Element(queue=w1892, element=w1891) -> (queue out=w1893:refnum<queue>)  [unwired: 2 in, 2 out]
                    }
                  }
                  frame True {
                    n657 = for {
                      shift-right: [w1898] -> w1896
                      shift-left: w1894 -> [w1899]
                      tunnel: string[] ["RESET ENCODERS", "RESET YAW", "RESET FLAGS"] -> [w1897] mode=indexing
                      n658 = Enqueue Element(queue=w1899, element=w1897) -> (queue out=w1898:refnum<queue>)  [unwired: 2 in, 2 out]
                    }
                  }
                }
                n659 = Select(t=State_Type_Definitions,_for_0.26g_versions_and_later_3."True Stop" ("Enum"), s=w1879, f=State_Type_Definitions,_for_0.26g_versions_and_later_3."Task 6M: STILL WAITING 3" ("Enum")) -> (s? t:f=w1882:T18)
                n660 = Select(t=w1882, s=w1880, f=State_Type_Definitions,_for_0.26g_versions_and_later_3."Task 6L: JAM IT IN" ("Enum")) -> (s? t:f=w1884:T18)
              }
              frame "Exit" {
                n661 = for {
                  shift-right: [w1906] -> w1903
                  shift-left: w1900 -> [w1907]
                  tunnel: string[] ["STOP", "RESET ENCODERS", "RESET YAW", "ARDUINO MODE 0"] -> [w1905] mode=indexing
                  n662 = Enqueue Element(queue=w1907, element=w1905) -> (queue out=w1906:refnum<queue>)  [unwired: 2 in, 2 out]
                }
              }
            }
          }
          frame "Task 6M: STILL WAITING 3" {
            # "Ball > Soap > Gel > Pipe"
            # ">>> Motor control cluster >>>"
            # ">>> yStepper command>>>"
            n663 = local read "Rising Edge"() -> (w1909:bool)
            n664 = Dequeue Element(queue=w1915, timeout in ms (-1)=w1914, error in (no error)=w1913) -> (element=w1912:T10)  [unwired: 3 out]
            n665 = case shown="\"Start Task 1\", Default" w1912 {
              tunnel: [w1929 State_Type_Definitions,_for_0.26g_versions_and_later_3."True Stop" ("Enum")] -> w1919
              tunnel: [w1922 w1947] -> w1918
              tunnel: [State_Type_Definitions,_for_0.26g_versions_and_later_3."Idle" ("Enum") State_Type_Definitions,_for_0.26g_versions_and_later_3."Shutdown" ("Enum")] -> w1920
              tunnel: w1916 -> [w1926 _]
              tunnel: w1917 -> [w1923 w1944]
              tunnel: w1909 -> [w1924 _]
              frame "Start Task 1", Default {
                # "Stays in Task 5D until the object is detected"
                n666 = Or(x=w1924, y=w1926) -> (x .or. y?=w1921:bool)
                n667 = case shown="False" w1921 {
                  tunnel: [w1934 w1940] -> w1922
                  tunnel: w1923 -> [w1932 w1939]
                  frame False {
                    n668 = for {
                      tunnel: string[] ["Z STEPPER CAM HEIGHT", "READ STEPPER VALUES"] ("element") -> [w1935] mode=indexing
                      shift-right: [w1937] -> w1934
                      shift-left: w1932 -> [w1936]
                      n669 = Enqueue Element(queue=w1936, element=w1935) -> (queue out=w1937:refnum<queue>)  [unwired: 2 in, 2 out]
                    }
                  }
                  frame True {
                    n670 = for {
                      shift-right: [w1942] -> w1940
                      shift-left: w1939 -> [w1943]
                      tunnel: string[] ["OPEN LOG CAM", "SET TIMER 2", "OPEN IMAQ REF", "", ""] -> [w1941] mode=indexing
                      n671 = Enqueue Element(queue=w1943, element=w1941) -> (queue out=w1942:refnum<queue>)  [unwired: 2 in, 2 out]
                    }
                  }
                }
                n672 = Select(t=State_Type_Definitions,_for_0.26g_versions_and_later_3."True Stop" ("Enum"), s=w1926, f=State_Type_Definitions,_for_0.26g_versions_and_later_3."Task 6N: CAM BURST 4" ("Enum")) -> (s? t:f=w1927:T18)
                n673 = Select(t=w1927, s=w1921, f=State_Type_Definitions,_for_0.26g_versions_and_later_3."Task 6M: STILL WAITING 3" ("Enum")) -> (s? t:f=w1929:T18)
              }
              frame "Exit" {
                n674 = for {
                  shift-right: [w1950] -> w1947
                  shift-left: w1944 -> [w1951]
                  tunnel: string[] ["STOP", "RESET ENCODERS", "RESET YAW", "ARDUINO MODE 0"] -> [w1949] mode=indexing
                  n675 = Enqueue Element(queue=w1951, element=w1949) -> (queue out=w1950:refnum<queue>)  [unwired: 2 in, 2 out]
                }
              }
            }
          }
          frame "Task 6N: CAM BURST 4" {
            # ">> Manual override >>"
            # ">>> Motor control cluster >>>"
            # ">>> yStepper command>>>"
            n676 = Dequeue Element(queue=w1963, timeout in ms (-1)=w1961, error in (no error)=w1962) -> (element=w1960:T10)  [unwired: 3 out]
            n677 = case shown="\"Start Task 1\", Default" w1960 {
              tunnel: [w1971 State_Type_Definitions,_for_0.26g_versions_and_later_3."True Stop" ("Enum")] -> w1957
              tunnel: [w1969 w1989] -> w1964
              tunnel: [State_Type_Definitions,_for_0.26g_versions_and_later_3."Idle" ("Enum") State_Type_Definitions,_for_0.26g_versions_and_later_3."Shutdown" ("Enum")] -> w1958
              tunnel: w1959 -> [w1967 _]
              tunnel: w1956 -> [w1968 w1986]
              tunnel: w1952 -> [w1965 _]
              frame "Start Task 1", Default {
                n678 = Or(x=w1965, y=w1967) -> (x .or. y?=w1966:bool)
                n679 = case shown="True" w1966 {
                  tunnel: [w1976 w1982] -> w1969
                  tunnel: w1968 -> [w1974 w1980]
                  frame False {
                    n680 = for {
                      tunnel: string[] ["CAM ACQ", "START TIMER"] ("element") -> [w1977] mode=indexing
                      shift-right: [w1979] -> w1976
                      shift-left: w1974 -> [w1978]
                      n681 = Enqueue Element(queue=w1978, element=w1977) -> (queue out=w1979:refnum<queue>)  [unwired: 2 in, 2 out]
                    }
                  }
                  frame True {
                    n682 = for {
                      shift-right: [w1984] -> w1982
                      shift-left: w1980 -> [w1985]
                      tunnel: string[] ["CAM CLOSE", "PROCESS IMAGE", "SET TIMER 2", "RESET ENCODERS"] -> [w1983] mode=indexing
                      n683 = Enqueue Element(queue=w1985, element=w1983) -> (queue out=w1984:refnum<queue>)  [unwired: 2 in, 2 out]
                    }
                  }
                }
                n684 = Select(t=State_Type_Definitions,_for_0.26g_versions_and_later_3."Task 6O: PROCESS IMAGE 4" ("Enum"), s=w1966, f=State_Type_Definitions,_for_0.26g_versions_and_later_3."Task 6N: CAM BURST 4" ("Enum")) -> (s? t:f=w1971:T18)
              }
              frame "Exit" {
                # ">> State after true stop >>"
                # ">> Goes to true stop >>"
                n685 = for {
                  shift-right: [w1992] -> w1989
                  shift-left: w1986 -> [w1993]
                  tunnel: string[] ["STOP", "RESET ENCODERS", "RESET YAW", ""] -> [w1991] mode=indexing
                  n686 = Enqueue Element(queue=w1993, element=w1991) -> (queue out=w1992:refnum<queue>)  [unwired: 2 in, 2 out]
                }
              }
            }
          }
          frame "Task 6O: PROCESS IMAGE 4" {
            # "Ball > Soap > Gel > Pipe"
            # ">>> Motor control cluster >>>"
            # ">>> yStepper command>>>"
            n687 = Dequeue Element(queue=w2002, timeout in ms (-1)=w2001, error in (no error)=w2000) -> (element=w1999:T10)  [unwired: 3 out]
            n688 = case shown="\"Start Task 1\", Default" w1999 {
              tunnel: [w2018 State_Type_Definitions,_for_0.26g_versions_and_later_3."True Stop" ("Enum")] -> w2006
              tunnel: [w2020 w2037] -> w2005
              tunnel: [State_Type_Definitions,_for_0.26g_versions_and_later_3."Idle" ("Enum") State_Type_Definitions,_for_0.26g_versions_and_later_3."Shutdown" ("Enum")] -> w2007
              tunnel: w2003 -> [w2009 _]
              tunnel: w2004 -> [w2015 w2034]
              tunnel: w1995 -> [w2013 _]
              tunnel: w1994 -> [w2014 _]
              frame "Start Task 1", Default {
                # "Stays in Task 5D until the object is detected"
                n689 = Or(x=w2013, y=w2009) -> (x .or. y?=w2012:bool)
                n690 = case shown="True" w2012 {
                  tunnel: [w2024 w2030] -> w2020
                  tunnel: w2015 -> [w2022 w2028]
                  frame False {
                    n691 = for {
                      tunnel: string[] ["START TIMER", "PROCESS IMAGE", ""] ("element") -> [w2025] mode=indexing
                      shift-right: [w2027] -> w2024
                      shift-left: w2022 -> [w2026]
                      n692 = Enqueue Element(queue=w2026, element=w2025) -> (queue out=w2027:refnum<queue>)  [unwired: 2 in, 2 out]
                    }
                  }
                  frame True {
                    n693 = for {
                      shift-right: [w2032] -> w2030
                      shift-left: w2028 -> [w2033]
                      tunnel: string[] ["RESET ENCODERS", "RESET YAW", ""] -> [w2031] mode=indexing
                      n694 = Enqueue Element(queue=w2033, element=w2031) -> (queue out=w2032:refnum<queue>)  [unwired: 2 in, 2 out]
                    }
                  }
                }
                n695 = Select(t=State_Type_Definitions,_for_0.26g_versions_and_later_3."Task 6P: PIPE BOMB" ("Enum"), s=w2014, f=State_Type_Definitions,_for_0.26g_versions_and_later_3."Task 6B: CAM BURST" ("Enum")) -> (s? t:f=w2010:T18)
                n696 = Select(t=State_Type_Definitions,_for_0.26g_versions_and_later_3."True Stop" ("Enum"), s=w2009, f=w2010) -> (s? t:f=w2016:T18)
                n697 = Select(t=w2016, s=w2012, f=State_Type_Definitions,_for_0.26g_versions_and_later_3."Task 6O: PROCESS IMAGE 4" ("Enum")) -> (s? t:f=w2018:T18)
              }
              frame "Exit" {
                n698 = for {
                  shift-right: [w2040] -> w2037
                  shift-left: w2034 -> [w2041]
                  tunnel: string[] ["STOP", "RESET ENCODERS", "RESET YAW", "ARDUINO MODE 0"] -> [w2039] mode=indexing
                  n699 = Enqueue Element(queue=w2041, element=w2039) -> (queue out=w2040:refnum<queue>)  [unwired: 2 in, 2 out]
                }
              }
            }
          }
          frame "Task 6P: PIPE BOMB" {
            # "Ball > Soap > Gel > Pipe"
            # ">>> Motor control cluster >>>"
            # ">>> yStepper command>>>"
            n700 = Greater Or Equal?(x=w2042, y=20.0) -> (x >= y?=w2043:bool)
            n701 = Dequeue Element(queue=w2051, timeout in ms (-1)=w2050, error in (no error)=w2049) -> (element=w2048:T10)  [unwired: 3 out]
            n702 = case shown="\"Start Task 1\", Default" w2048 {
              tunnel: [w2064 State_Type_Definitions,_for_0.26g_versions_and_later_3."True Stop" ("Enum")] -> w2055
              tunnel: [w2066 w2083] -> w2054
              tunnel: [State_Type_Definitions,_for_0.26g_versions_and_later_3."Idle" ("Enum") State_Type_Definitions,_for_0.26g_versions_and_later_3."Shutdown" ("Enum")] -> w2056
              tunnel: w2052 -> [w2059 _]
              tunnel: w2053 -> [w2061 w2080]
              tunnel: w2043 -> [w2058 _]
              frame "Start Task 1", Default {
                # "Stays in Task 5D until the object is detected"
                n703 = Or(x=w2058, y=w2059) -> (x .or. y?=w2060:bool)
                n704 = case shown="False" w2060 {
                  tunnel: [w2070 w2076] -> w2066
                  tunnel: w2061 -> [w2068 w2074]
                  frame False {
                    n705 = for {
                      tunnel: string[] ["FORWARD", "READ NAVX", "READ ENCODERS"] ("element") -> [w2071] mode=indexing
                      shift-right: [w2073] -> w2070
                      shift-left: w2068 -> [w2072]
                      n706 = Enqueue Element(queue=w2072, element=w2071) -> (queue out=w2073:refnum<queue>)  [unwired: 2 in, 2 out]
                    }
                  }
                  frame True {
                    n707 = for {
                      shift-right: [w2078] -> w2076
                      shift-left: w2074 -> [w2079]
                      tunnel: string[] ["RESET ENCODERS", "RESET YAW", "RESET FLAGS"] -> [w2077] mode=indexing
                      n708 = Enqueue Element(queue=w2079, element=w2077) -> (queue out=w2078:refnum<queue>)  [unwired: 2 in, 2 out]
                    }
                  }
                }
                n709 = Select(t=State_Type_Definitions,_for_0.26g_versions_and_later_3."True Stop" ("Enum"), s=w2059, f=State_Type_Definitions,_for_0.26g_versions_and_later_3."Task 5F: ARM GRAB HEIGHT" ("Enum")) -> (s? t:f=w2062:T18)
                n710 = Select(t=w2062, s=w2060, f=State_Type_Definitions,_for_0.26g_versions_and_later_3."Task 6P: PIPE BOMB" ("Enum")) -> (s? t:f=w2064:T18)
              }
              frame "Exit" {
                n711 = for {
                  shift-right: [w2086] -> w2083
                  shift-left: w2080 -> [w2087]
                  tunnel: string[] ["STOP", "RESET ENCODERS", "RESET YAW", "ARDUINO MODE 0"] -> [w2085] mode=indexing
                  n712 = Enqueue Element(queue=w2087, element=w2085) -> (queue out=w2086:refnum<queue>)  [unwired: 2 in, 2 out]
                }
              }
            }
          }
          frame "Task 7" {
          }
          frame "Task 8A: RAISE ARM" {
            # ">>> Motor control cluster >>>"
            # ">>> yStepper command>>>"
            # ">> Manual override >>"
            n713 = Dequeue Element(queue=w2104, timeout in ms (-1)=w2103, error in (no error)=w2105) -> (element=w2102:T10)  [unwired: 3 out]
            n714 = Equal?(x=w2101, y=u8 60) -> (x = y?=w2099:bool)
            n715 = case shown="\"Start Task 1\", Default" w2102 {
              tunnel: [w2115 State_Type_Definitions,_for_0.26g_versions_and_later_3."True Stop" ("Enum")] -> w2106
              tunnel: [w2118 w2135] -> w2107
              tunnel: [State_Type_Definitions,_for_0.26g_versions_and_later_3."Idle" ("Enum") State_Type_Definitions,_for_0.26g_versions_and_later_3."Shutdown" ("Enum")] -> w2108
              tunnel: w2099 -> [w2114 _]
              tunnel: w2098 -> [w2113 _]
              tunnel: w2097 -> [w2109 w2132]
              frame "Start Task 1", Default {
                # "Stays in Task 5_A until stepper reaches desired \nheight"
                # "T: Go back to idle, F: Continue with task\""
                # ">> Manual override >>"
                n716 = case shown="False" w2114 {
                  tunnel: [w2122 w2128] -> w2118
                  tunnel: w2109 -> [w2120 w2126]
                  frame False {
                    n717 = for {
                      tunnel: string[] ["Z STEPPER CAM HEIGHT", "READ STEPPER VALUES", "READ IR"] ("element") -> [w2123] mode=indexing
                      shift-right: [w2125] -> w2122
                      shift-left: w2120 -> [w2124]
                      n718 = Enqueue Element(queue=w2124, element=w2123) -> (queue out=w2125:refnum<queue>)  [unwired: 2 in, 2 out]
                    }
                  }
                  frame True {
                    n719 = for {
                      shift-right: [w2130] -> w2128
                      shift-left: w2126 -> [w2131]
                      tunnel: string[] ["RESET YAW", "RESET ENCODERS", "READ IR"] -> [w2129] mode=indexing
                      n720 = Enqueue Element(queue=w2131, element=w2129) -> (queue out=w2130:refnum<queue>)  [unwired: 2 in, 2 out]
                    }
                  }
                }
                n721 = Or(x=w2114, y=w2113) -> (x .or. y?=w2116:bool)
                n722 = Select(t=State_Type_Definitions,_for_0.26g_versions_and_later_3."True Stop" ("Enum"), s=w2113, f=State_Type_Definitions,_for_0.26g_versions_and_later_3."Task 8B: MOVE TO BOX" ("Enum")) -> (s? t:f=w2110:T18)
                n723 = Select(t=w2110, s=w2116, f=State_Type_Definitions,_for_0.26g_versions_and_later_3."Task 8A: RAISE ARM" ("Enum")) -> (s? t:f=w2115:T18)
              }
              frame "Exit" {
                n724 = for {
                  shift-right: [w2138] -> w2135
                  shift-left: w2132 -> [w2139]
                  tunnel: string[] ["STOP", "RESET ENCODERS", "RESET YAW", "ARDUINO MODE 0"] -> [w2137] mode=indexing
                  n725 = Enqueue Element(queue=w2139, element=w2137) -> (queue out=w2138:refnum<queue>)  [unwired: 2 in, 2 out]
                }
              }
            }
          }
          frame "Task 8B: MOVE TO BOX" {
            w2149 = u8 15 ("y")
            # "High voltage: 70"
            # ">>> yStepper command>>>"
            n726 = Less?(x=w2146, y=w2149) -> (x < y?=w2147:bool)
            n727 = Less?(x=w2145, y=w2149) -> (x < y?=w2148:bool)
            n728 = And(x=w2148, y=w2147) -> ()  [unwired: 1 out]
            n729 = Dequeue Element(queue=w2153, timeout in ms (-1)=w2152, error in (no error)=w2154) -> (element=w2151:T10)  [unwired: 3 out]
            n730 = Less?(x=w2142, y=40.0) -> (x < y?=w2140:bool)
            n731 = case shown="\"Start Task 1\", Default" w2151 {
              tunnel: [w2166 State_Type_Definitions,_for_0.26g_versions_and_later_3."True Stop" ("Enum")] -> w2156
              tunnel: [w2169 w2186] -> w2155
              tunnel: [State_Type_Definitions,_for_0.26g_versions_and_later_3."Idle" ("Enum") State_Type_Definitions,_for_0.26g_versions_and_later_3."Shutdown" ("Enum")] -> w2157
              tunnel: w2159 -> [w2165 _]
              tunnel: w2158 -> [w2161 w2183]
              tunnel: w2140 -> [w2160 _]
              frame "Start Task 1", Default {
                # "Stays in Task 5_B to capture image over 5 seconds"
                # "T: Go back to idle, F: Continue with task\""
                # ">> Manual override >>"
                n732 = case shown="True" w2160 {
                  tunnel: [w2173 w2179] -> w2169
                  tunnel: w2161 -> [w2171 w2177]
                  frame False {
                    n733 = for {
                      tunnel: string[] ["FORWARD", "READ IR", "READ NAVX"] ("element") -> [w2174] mode=indexing
                      shift-right: [w2176] -> w2173
                      shift-left: w2171 -> [w2175]
                      n734 = Enqueue Element(queue=w2175, element=w2174) -> (queue out=w2176:refnum<queue>)  [unwired: 2 in, 2 out]
                    }
                  }
                  frame True {
                    n735 = for {
                      shift-right: [w2181] -> w2179
                      shift-left: w2177 -> [w2182]
                      tunnel: string[] ["STOP", "RESET ENCODERS", "OPEN LOG CAM", "SET TIMER 2", "OPEN IMAQ REF"] -> [w2180] mode=indexing
                      n736 = Enqueue Element(queue=w2182, element=w2180) -> (queue out=w2181:refnum<queue>)  [unwired: 2 in, 2 out]
                    }
                  }
                }
                n737 = Or(x=w2160, y=w2165) -> (x .or. y?=w2167:bool)
                n738 = Select(t=State_Type_Definitions,_for_0.26g_versions_and_later_3."True Stop" ("Enum"), s=w2165, f=State_Type_Definitions,_for_0.26g_versions_and_later_3."Task 8C: CAM BURST" ("Enum")) -> (s? t:f=w2162:T18)
                n739 = Select(t=w2162, s=w2167, f=State_Type_Definitions,_for_0.26g_versions_and_later_3."Task 8B: MOVE TO BOX" ("Enum")) -> (s? t:f=w2166:T18)
              }
              frame "Exit" {
                n740 = for {
                  shift-right: [w2189] -> w2186
                  shift-left: w2183 -> [w2190]
                  tunnel: string[] ["STOP", "RESET ENCODERS", "RESET YAW", "ARDUINO MODE 0"] -> [w2188] mode=indexing
                  n741 = Enqueue Element(queue=w2190, element=w2188) -> (queue out=w2189:refnum<queue>)  [unwired: 2 in, 2 out]
                }
              }
            }
          }
          frame "Task 8C: CAM BURST" {
            # ">>> Motor control cluster >>>"
            # ">>> yStepper command>>>"
            # ">> Manual override >>"
            n742 = Dequeue Element(queue=w2201, timeout in ms (-1)=w2200, error in (no error)=w2199) -> (element=w2198:T10)  [unwired: 3 out]
            n743 = case shown="\"Start Task 1\", Default" w2198 {
              tunnel: [w2210 State_Type_Definitions,_for_0.26g_versions_and_later_3."True Stop" ("Enum")] -> w2203
              tunnel: [w2213 w2230] -> w2196
              tunnel: [State_Type_Definitions,_for_0.26g_versions_and_later_3."Idle" ("Enum") State_Type_Definitions,_for_0.26g_versions_and_later_3."Shutdown" ("Enum")] -> w2195
              tunnel: w2197 -> [w2204 _]
              tunnel: w2202 -> [w2209 w2227]
              tunnel: w2193 -> [w2208 _]
              frame "Start Task 1", Default {
                # ">> Is time up? >>"
                # "Determines if object is in range to pick up"
                # ">> Manual override >>"
                n744 = case shown="True" w2208 {
                  tunnel: [w2217 w2223] -> w2213
                  tunnel: w2209 -> [w2215 w2221]
                  frame False {
                    n745 = for {
                      tunnel: string[] ["CAM ACQ", "START TIMER"] ("element") -> [w2218] mode=indexing
                      shift-right: [w2220] -> w2217
                      shift-left: w2215 -> [w2219]
                      n746 = Enqueue Element(queue=w2219, element=w2218) -> (queue out=w2220:refnum<queue>)  [unwired: 2 in, 2 out]
                    }
                  }
                  frame True {
                    n747 = for {
                      shift-right: [w2225] -> w2223
                      shift-left: w2221 -> [w2226]
                      tunnel: string[] ["CAM CLOSE", "PROCESS IMAGE", "SET TIMER 2"] -> [w2224] mode=indexing
                      n748 = Enqueue Element(queue=w2226, element=w2224) -> (queue out=w2225:refnum<queue>)  [unwired: 2 in, 2 out]
                    }
                  }
                }
                n749 = Or(x=w2208, y=w2204) -> (x .or. y?=w2211:bool)
                n750 = Select(t=State_Type_Definitions,_for_0.26g_versions_and_later_3."True Stop" ("Enum"), s=w2204, f=State_Type_Definitions,_for_0.26g_versions_and_later_3."Task 8D: PROCESS IMAGE" ("Enum")) -> (s? t:f=w2206:T18)
                n751 = Select(t=w2206, s=w2211, f=State_Type_Definitions,_for_0.26g_versions_and_later_3."Task 8C: CAM BURST" ("Enum")) -> (s? t:f=w2210:T18)
              }
              frame "Exit" {
                n752 = for {
                  shift-right: [w2233] -> w2230
                  shift-left: w2227 -> [w2234]
                  tunnel: string[] ["STOP", "RESET ENCODERS", "RESET YAW", "ARDUINO MODE 0"] -> [w2232] mode=indexing
                  n753 = Enqueue Element(queue=w2234, element=w2232) -> (queue out=w2233:refnum<queue>)  [unwired: 2 in, 2 out]
                }
              }
            }
          }
          frame "Task 8D: PROCESS IMAGE" {
            # ">>> Motor control cluster >>>"
            # ">>> yStepper command>>>"
            n754 = Dequeue Element(queue=w2243, timeout in ms (-1)=w2242, error in (no error)=w2241) -> (element=w2240:T10)  [unwired: 3 out]
            n755 = case shown="\"Start Task 1\", Default" w2240 {
              tunnel: [w2258 State_Type_Definitions,_for_0.26g_versions_and_later_3."True Stop" ("Enum")] -> w2247
              tunnel: [w2261 w2278] -> w2246
              tunnel: [State_Type_Definitions,_for_0.26g_versions_and_later_3."Idle" ("Enum") State_Type_Definitions,_for_0.26g_versions_and_later_3."Shutdown" ("Enum")] -> w2248
              tunnel: w2244 -> [w2257 _]
              tunnel: w2245 -> [w2254 w2275]
              tunnel: w2235 -> [w2253 _]
              tunnel: w2236 -> [w2252 _]
              frame "Start Task 1", Default {
                # ">> T: Breaks out of state loop; F: Stays in loop>>"
                # ">> Manual override >>"
                # ">> Checks if time is up>>"
                # "Stays in Task 5D until the object is detected"
                # "T: Go back to idle, F: Continue with task\""
                # ">> Manual override >>"
                n756 = case shown="False" w2253 {
                  tunnel: [w2265 w2271] -> w2261
                  tunnel: w2254 -> [w2263 w2269]
                  frame False {
                    n757 = for {
                      tunnel: string[] ["START TIMER", "PROCESS IMAGE", ""] ("element") -> [w2266] mode=indexing
                      shift-right: [w2268] -> w2265
                      shift-left: w2263 -> [w2267]
                      n758 = Enqueue Element(queue=w2267, element=w2266) -> (queue out=w2268:refnum<queue>)  [unwired: 2 in, 2 out]
                    }
                  }
                  frame True {
                    n759 = for {
                      shift-right: [w2273] -> w2271
                      shift-left: w2269 -> [w2274]
                      tunnel: string[] ["RESET ENCODERS", "", ""] -> [w2272] mode=indexing
                      n760 = Enqueue Element(queue=w2274, element=w2272) -> (queue out=w2273:refnum<queue>)  [unwired: 2 in, 2 out]
                    }
                  }
                }
                n761 = Or(x=w2253, y=w2257) -> (x .or. y?=w2259:bool)
                n762 = Select(t=State_Type_Definitions,_for_0.26g_versions_and_later_3."Task 8E: ROBOT ADJUST" ("Enum"), s=w2252, f=State_Type_Definitions,_for_0.26g_versions_and_later_3."True Stop" ("Enum")) -> (s? t:f=w2249:T18)
                n763 = Select(t=State_Type_Definitions,_for_0.26g_versions_and_later_3."True Stop" ("Enum"), s=w2257, f=w2249) -> (s? t:f=w2255:T18)
                n764 = Select(t=w2255, s=w2259, f=State_Type_Definitions,_for_0.26g_versions_and_later_3."Task 8D: PROCESS IMAGE" ("Enum")) -> (s? t:f=w2258:T18)
              }
              frame "Exit" {
                n765 = for {
                  shift-right: [w2281] -> w2278
                  shift-left: w2275 -> [w2282]
                  tunnel: string[] ["STOP", "RESET ENCODERS", "RESET YAW", "ARDUINO MODE 0"] -> [w2280] mode=indexing
                  n766 = Enqueue Element(queue=w2282, element=w2280) -> (queue out=w2281:refnum<queue>)  [unwired: 2 in, 2 out]
                }
              }
            }
          }
          frame "Task 8E: ROBOT ADJUST" {
            # ">>> Motor control cluster >>>"
            # ">>> yStepper command>>>"
            n767 = Dequeue Element(queue=w2300, timeout in ms (-1)=w2299, error in (no error)=w2298) -> (element=w2297:T10)  [unwired: 3 out]
            n768 = Subtract(x=w2295, y=150.0) -> (x-y=w2293:dbl)
            n769 = formula code="if (error <= -100 && error < -80){\n    distance = -20;\n    xSpeed = -30;\n}\n\nelse if (error <= -80 && error < -60){\n    distance = -18;\n    xSpeed = -30;\n}\n\nelse if (error <= -60 && error < -40){\n    distance = -15;\n    xSpeed = -30;\n}\n\nelse if (error <= -40 && error < -20){\n    distance = -10;\n    xSpeed = -30;\n}\n\nelse if (error <= -20 && error < -10){\n    distance = 5;\n    xSpeed = -30;\n}\n\nelse if (error <= -10 && error <= 10){\n    distance = 0;\n    xSpeed = 0;\n}\n\nelse if (error <= 20 && error < 40){\n    distance = 5;\n    xSpeed = 30;\n}\n\nelse if (error <= 40 && error < 60){\n    distance = 10;\n    xSpeed = 30;\n}\n\nelse if (error <= 60 && error < 80){\n    distance = 15;\n    xSpeed = 30;\n}\n\nelse if (error <= 80 && error < 100){\n    distance = 18;\n    xSpeed = 30;\n}\n\nelse if (error <= 100){\n    distance = 20;\n    xSpeed = 30;\n}\n\nelse {\n    distance = 0;\n    xSpeed = 0;\n}"("error"=w2293) -> ("distance"=w2283:dbl, "xSpeed"=w2290:dbl)
            n770 = formula code="if (target > 0){\nif (current  >= target)\noutput = 1;\n\nelse if (current != target)\noutput = 0;\n}\n\nelse if (target == 0){\nif (current == target)\noutput = 1;\n\nelse if (current != target)\noutput = 0;\n}\n\nelse if (target < 0){\nif (current <= target)\noutput = 1;\n\nelse if (current != target)\noutput = 0;\n}\n\nelse if (current != target)\noutput = 0;"("target"=w2283, "current"=w2289) -> ("output"=w2288:dbl)
            n771 = call "yDistance travelled FGV.vi"("Init/Read/Write State"=States_for_Action_Engine."Write", "yDistance travelled"=w2283) -> ()  [unwired: 8 in, 2 out]
            n772 = Bundle By Name(cluster=w2292, "xSpeed"=w2290) -> (w2291:T20)
            n773 = Equal?(x=w2288, y=1.0) -> (x = y?=w2285:bool)
            n774 = case shown="\"Start Task 1\", Default" w2297 {
              tunnel: [w2312 State_Type_Definitions,_for_0.26g_versions_and_later_3."True Stop" ("Enum")] -> w2304
              tunnel: [w2315 w2332] -> w2303
              tunnel: [State_Type_Definitions,_for_0.26g_versions_and_later_3."Idle" ("Enum") State_Type_Definitions,_for_0.26g_versions_and_later_3."Shutdown" ("Enum")] -> w2305
              tunnel: w2301 -> [w2311 _]
              tunnel: w2302 -> [w2307 w2329]
              tunnel: w2285 -> [w2306 _]
              frame "Start Task 1", Default {
                # ">> T: Breaks out of state loop; F: Stays in loop>>"
                # ">> Manual override >>"
                # ">> Checks if time is up>>"
                # "Stays in Task 5D until the object is detected"
                # "T: Go back to idle, F: Continue with task\""
                # ">> Manual override >>"
                n775 = case shown="True" w2306 {
                  tunnel: [w2319 w2325] -> w2315
                  tunnel: w2307 -> [w2317 w2323]
                  frame False {
                    n776 = for {
                      tunnel: string[] ["X AXIS - SLOW", "READ ENCODERS", "READ NAVX"] ("element") -> [w2320] mode=indexing
                      shift-right: [w2322] -> w2319
                      shift-left: w2317 -> [w2321]
                      n777 = Enqueue Element(queue=w2321, element=w2320) -> (queue out=w2322:refnum<queue>)  [unwired: 2 in, 2 out]
                    }
                  }
                  frame True {
                    n778 = for {
                      shift-right: [w2327] -> w2325
                      shift-left: w2323 -> [w2328]
                      tunnel: string[] ["SET TIMER 2", "STOP", "READ STEPPER VALUES", ""] -> [w2326] mode=indexing
                      n779 = Enqueue Element(queue=w2328, element=w2326) -> (queue out=w2327:refnum<queue>)  [unwired: 2 in, 2 out]
                    }
                  }
                }
                n780 = Or(x=w2306, y=w2311) -> (x .or. y?=w2313:bool)
                n781 = Select(t=State_Type_Definitions,_for_0.26g_versions_and_later_3."True Stop" ("Enum"), s=w2311, f=State_Type_Definitions,_for_0.26g_versions_and_later_3."Task 8H: ARM ADJUST" ("Enum")) -> (s? t:f=w2308:T18)
                n782 = Select(t=w2308, s=w2313, f=State_Type_Definitions,_for_0.26g_versions_and_later_3."Task 8E: ROBOT ADJUST" ("Enum")) -> (s? t:f=w2312:T18)
              }
              frame "Exit" {
                n783 = for {
                  shift-right: [w2335] -> w2332
                  shift-left: w2329 -> [w2336]
                  tunnel: string[] ["STOP", "RESET ENCODERS", "RESET YAW", "ARDUINO MODE 0"] -> [w2334] mode=indexing
                  n784 = Enqueue Element(queue=w2336, element=w2334) -> (queue out=w2335:refnum<queue>)  [unwired: 2 in, 2 out]
                }
              }
            }
          }
          frame "Task 8F: CAM BURST 2" {
            # ">>> Motor control cluster >>>"
            # ">>> yStepper command>>>"
            # ">> Manual override >>"
            n785 = Dequeue Element(queue=w2347, timeout in ms (-1)=w2346, error in (no error)=w2345) -> (element=w2344:T10)  [unwired: 3 out]
            n786 = case shown="\"Start Task 1\", Default" w2344 {
              tunnel: [w2356 State_Type_Definitions,_for_0.26g_versions_and_later_3."True Stop" ("Enum")] -> w2349
              tunnel: [w2359 w2376] -> w2342
              tunnel: [State_Type_Definitions,_for_0.26g_versions_and_later_3."Idle" ("Enum") State_Type_Definitions,_for_0.26g_versions_and_later_3."Shutdown" ("Enum")] -> w2341
              tunnel: w2343 -> [w2350 _]
              tunnel: w2348 -> [w2355 w2373]
              tunnel: w2339 -> [w2354 _]
              frame "Start Task 1", Default {
                # ">> Is time up? >>"
                # "Determines if object is in range to pick up"
                # ">> Manual override >>"
                n787 = case shown="False" w2354 {
                  tunnel: [w2363 w2369] -> w2359
                  tunnel: w2355 -> [w2361 w2367]
                  frame False {
                    n788 = for {
                      tunnel: string[] ["CAM ACQ", "START TIMER"] ("element") -> [w2364] mode=indexing
                      shift-right: [w2366] -> w2363
                      shift-left: w2361 -> [w2365]
                      n789 = Enqueue Element(queue=w2365, element=w2364) -> (queue out=w2366:refnum<queue>)  [unwired: 2 in, 2 out]
                    }
                  }
                  frame True {
                    n790 = for {
                      shift-right: [w2371] -> w2369
                      shift-left: w2367 -> [w2372]
                      tunnel: string[] ["CAM CLOSE", "PROCESS IMAGE", "SET TIMER 3"] -> [w2370] mode=indexing
                      n791 = Enqueue Element(queue=w2372, element=w2370) -> (queue out=w2371:refnum<queue>)  [unwired: 2 in, 2 out]
                    }
                  }
                }
                n792 = Or(x=w2354, y=w2350) -> (x .or. y?=w2357:bool)
                n793 = Select(t=State_Type_Definitions,_for_0.26g_versions_and_later_3."True Stop" ("Enum"), s=w2350, f=State_Type_Definitions,_for_0.26g_versions_and_later_3."Task 8G: PROCESS IMAGE 2" ("Enum")) -> (s? t:f=w2352:T18)
                n794 = Select(t=w2352, s=w2357, f=State_Type_Definitions,_for_0.26g_versions_and_later_3."Task 8F: CAM BURST 2" ("Enum")) -> (s? t:f=w2356:T18)
              }
              frame "Exit" {
                n795 = for {
                  shift-right: [w2379] -> w2376
                  shift-left: w2373 -> [w2380]
                  tunnel: string[] ["STOP", "RESET ENCODERS", "RESET YAW", "ARDUINO MODE 0"] -> [w2378] mode=indexing
                  n796 = Enqueue Element(queue=w2380, element=w2378) -> (queue out=w2379:refnum<queue>)  [unwired: 2 in, 2 out]
                }
              }
            }
          }
          frame "Task 8G: PROCESS IMAGE 2" {
            # ">>> yStepper command>>>"
            n797 = Dequeue Element(queue=w2388, timeout in ms (-1)=w2387, error in (no error)=w2386) -> (element=w2385:T10)  [unwired: 3 out]
            n798 = case shown="\"Start Task 1\", Default" w2385 {
              tunnel: [w2400 State_Type_Definitions,_for_0.26g_versions_and_later_3."True Stop" ("Enum")] -> w2392
              tunnel: [w2403 w2420] -> w2391
              tunnel: [State_Type_Definitions,_for_0.26g_versions_and_later_3."Idle" ("Enum") State_Type_Definitions,_for_0.26g_versions_and_later_3."Shutdown" ("Enum")] -> w2393
              tunnel: w2389 -> [w2399 _]
              tunnel: w2390 -> [w2395 w2417]
              tunnel: w2383 -> [w2394 _]
              frame "Start Task 1", Default {
                # ">> T: Breaks out of state loop; F: Stays in loop>>"
                # ">> Manual override >>"
                # ">> Checks if time is up>>"
                # "Stays in Task 5D until the object is detected"
                # "T: Go back to idle, F: Continue with task\""
                # ">> Manual override >>"
                n799 = case shown="False" w2394 {
                  tunnel: [w2407 w2413] -> w2403
                  tunnel: w2395 -> [w2405 w2411]
                  frame False {
                    n800 = for {
                      tunnel: string[] ["START TIMER", "PROCESS IMAGE", ""] ("element") -> [w2408] mode=indexing
                      shift-right: [w2410] -> w2407
                      shift-left: w2405 -> [w2409]
                      n801 = Enqueue Element(queue=w2409, element=w2408) -> (queue out=w2410:refnum<queue>)  [unwired: 2 in, 2 out]
                    }
                  }
                  frame True {
                    n802 = for {
                      shift-right: [w2415] -> w2413
                      shift-left: w2411 -> [w2416]
                      tunnel: string[] ["READ STEPPER VALUES", "Y STEPPER CONTROL", ""] -> [w2414] mode=indexing
                      n803 = Enqueue Element(queue=w2416, element=w2414) -> (queue out=w2415:refnum<queue>)  [unwired: 2 in, 2 out]
                    }
                  }
                }
                n804 = Or(x=w2394, y=w2399) -> (x .or. y?=w2401:bool)
                n805 = Select(t=State_Type_Definitions,_for_0.26g_versions_and_later_3."True Stop" ("Enum"), s=w2399, f=State_Type_Definitions,_for_0.26g_versions_and_later_3."Task 8H: ARM ADJUST" ("Enum")) -> (s? t:f=w2396:T18)
                n806 = Select(t=w2396, s=w2401, f=State_Type_Definitions,_for_0.26g_versions_and_later_3."Task 8G: PROCESS IMAGE 2" ("Enum")) -> (s? t:f=w2400:T18)
              }
              frame "Exit" {
                n807 = for {
                  shift-right: [w2423] -> w2420
                  shift-left: w2417 -> [w2424]
                  tunnel: string[] ["STOP", "RESET ENCODERS", "RESET YAW", "ARDUINO MODE 0"] -> [w2422] mode=indexing
                  n808 = Enqueue Element(queue=w2424, element=w2422) -> (queue out=w2423:refnum<queue>)  [unwired: 2 in, 2 out]
                }
              }
            }
          }
          frame "Task 8H: ARM ADJUST" {
            # ">>> yStepper command>>>"
            n809 = Dequeue Element(queue=w2438, timeout in ms (-1)=w2439, error in (no error)=w2440) -> (element=w2442:T10)  [unwired: 3 out]
            n810 = formula code="if (pos >= 40 && pos < 80)\ny = 40;\n\nelse if (pos >= 80 && pos < 100)\ny = 35;\n\nelse if (pos >= 100 && pos < 120)\ny = 20;\n\nelse if (pos >= 120 && pos < 140)\ny = 15;\n\nelse if (pos >= 140 && pos < 150)\ny = 10;\n\nelse if (pos >= 150 && 170)\ny = 5;\n\nelse \ny = 0;"("pos"=w2430) -> ("y"=w2433:dbl)
            n811 = To Unsigned Byte Integer(number=w2433) -> (unsigned 8bit integer=w2428:u8)
            n812 = Equal?(x=w2429, y=w2428) -> (x = y?=w2427:bool)
            n813 = case shown="\"Start Task 1\", Default" w2442 {
              tunnel: [w2449 State_Type_Definitions,_for_0.26g_versions_and_later_3."True Stop" ("Enum")] -> w2436
              tunnel: [w2452 w2469] -> w2434
              tunnel: [State_Type_Definitions,_for_0.26g_versions_and_later_3."Idle" ("Enum") State_Type_Definitions,_for_0.26g_versions_and_later_3."Shutdown" ("Enum")] -> w2435
              tunnel: w2441 -> [w2443 _]
              tunnel: w2437 -> [w2445 w2466]
              tunnel: w2427 -> [w2444 _]
              frame "Start Task 1", Default {
                # ">> T: Breaks out of state loop; F: Stays in loop>>"
                # ">> Manual override >>"
                # ">> Checks if time is up>>"
                # "Stays in Task 5D until the object is detected"
                # "T: Go back to idle, F: Continue with task\""
                # ">> Manual override >>"
                n814 = case shown="False" w2444 {
                  tunnel: [w2456 w2462] -> w2452
                  tunnel: w2445 -> [w2454 w2460]
                  frame False {
                    n815 = for {
                      tunnel: string[] ["READ STEPPER VALUES", "Y STEPPER CONTROL", ""] ("element") -> [w2457] mode=indexing
                      shift-right: [w2459] -> w2456
                      shift-left: w2454 -> [w2458]
                      n816 = Enqueue Element(queue=w2458, element=w2457) -> (queue out=w2459:refnum<queue>)  [unwired: 2 in, 2 out]
                    }
                  }
                  frame True {
                    n817 = for {
                      shift-right: [w2464] -> w2462
                      shift-left: w2460 -> [w2465]
                      tunnel: string[] ["DISPOSE BUFFERS", "READ STEPPER VALUES", ""] -> [w2463] mode=indexing
                      n818 = Enqueue Element(queue=w2465, element=w2463) -> (queue out=w2464:refnum<queue>)  [unwired: 2 in, 2 out]
                    }
                  }
                }
                n819 = Or(x=w2444, y=w2443) -> (x .or. y?=w2450:bool)
                n820 = Select(t=State_Type_Definitions,_for_0.26g_versions_and_later_3."True Stop" ("Enum"), s=w2443, f=State_Type_Definitions,_for_0.26g_versions_and_later_3."Task 8I: ARM GRAB HEIGHT" ("Enum")) -> (s? t:f=w2446:T18)
                n821 = Select(t=w2446, s=w2450, f=State_Type_Definitions,_for_0.26g_versions_and_later_3."Task 8H: ARM ADJUST" ("Enum")) -> (s? t:f=w2449:T18)
              }
              frame "Exit" {
                n822 = for {
                  shift-right: [w2472] -> w2469
                  shift-left: w2466 -> [w2473]
                  tunnel: string[] ["STOP", "RESET ENCODERS", "RESET YAW", "ARDUINO MODE 0"] -> [w2471] mode=indexing
                  n823 = Enqueue Element(queue=w2473, element=w2471) -> (queue out=w2472:refnum<queue>)  [unwired: 2 in, 2 out]
                }
              }
            }
            n824 = Bundle By Name(cluster=w2432, "yStepper desired"=w2428) -> (w2431:T21)
          }
          frame "Task 8I: ARM GRAB HEIGHT" {
            # ">>> Motor control cluster >>>"
            # ">>> yStepper command>>>"
            # ">> Manual override >>"
            n825 = Dequeue Element(queue=w2484, timeout in ms (-1)=w2483, error in (no error)=w2485) -> (element=w2482:T10)  [unwired: 3 out]
            n826 = Equal?(x=w2481, y=u8 1) -> (x = y?=w2479:bool)
            n827 = case shown="\"Start Task 1\", Default" w2482 {
              tunnel: [w2495 State_Type_Definitions,_for_0.26g_versions_and_later_3."True Stop" ("Enum")] -> w2486
              tunnel: [w2498 w2515] -> w2487
              tunnel: [State_Type_Definitions,_for_0.26g_versions_and_later_3."Idle" ("Enum") State_Type_Definitions,_for_0.26g_versions_and_later_3."Shutdown" ("Enum")] -> w2488
              tunnel: w2479 -> [w2494 _]
              tunnel: w2478 -> [w2493 _]
              tunnel: w2477 -> [w2489 w2512]
              frame "Start Task 1", Default {
                # "Stays in Task 5F until stepper reaches desired \nheight"
                # "T: Go back to idle, F: Continue with task\""
                # ">> Manual override >>"
                n828 = case shown="True" w2494 {
                  tunnel: [w2502 w2508] -> w2498
                  tunnel: w2489 -> [w2500 w2506]
                  frame False {
                    n829 = for {
                      tunnel: string[] ["Z STEPPER GRAB HEIGHT", "READ STEPPER VALUES"] ("element") -> [w2503] mode=indexing
                      shift-right: [w2505] -> w2502
                      shift-left: w2500 -> [w2504]
                      n830 = Enqueue Element(queue=w2504, element=w2503) -> (queue out=w2505:refnum<queue>)  [unwired: 2 in, 2 out]
                    }
                  }
                  frame True {
                    n831 = for {
                      shift-right: [w2510] -> w2508
                      shift-left: w2506 -> [w2511]
                      tunnel: string[] ["SET TIMER 2", "CLOSE CLAW", ""] -> [w2509] mode=indexing
                      n832 = Enqueue Element(queue=w2511, element=w2509) -> (queue out=w2510:refnum<queue>)  [unwired: 2 in, 2 out]
                    }
                  }
                }
                n833 = Or(x=w2494, y=w2493) -> (x .or. y?=w2496:bool)
                n834 = Select(t=State_Type_Definitions,_for_0.26g_versions_and_later_3."True Stop" ("Enum"), s=w2493, f=State_Type_Definitions,_for_0.26g_versions_and_later_3."Task 8J: CLOSE CLAW" ("Enum")) -> (s? t:f=w2490:T18)
                n835 = Select(t=w2490, s=w2496, f=State_Type_Definitions,_for_0.26g_versions_and_later_3."Task 8I: ARM GRAB HEIGHT" ("Enum")) -> (s? t:f=w2495:T18)
              }
              frame "Exit" {
                n836 = for {
                  shift-right: [w2518] -> w2515
                  shift-left: w2512 -> [w2519]
                  tunnel: string[] ["STOP", "RESET ENCODERS", "RESET YAW", "ARDUINO MODE 0"] -> [w2517] mode=indexing
                  n837 = Enqueue Element(queue=w2519, element=w2517) -> (queue out=w2518:refnum<queue>)  [unwired: 2 in, 2 out]
                }
              }
            }
          }
          frame "Task 8J: CLOSE CLAW" {
            # ">>> yStepper command>>>"
            # ">> Manual override >>"
            n838 = Dequeue Element(queue=w2530, timeout in ms (-1)=w2529, error in (no error)=w2528) -> (element=w2527:T10)  [unwired: 3 out]
            n839 = case shown="\"Start Task 1\", Default" w2527 {
              tunnel: [w2539 State_Type_Definitions,_for_0.26g_versions_and_later_3."True Stop" ("Enum")] -> w2532
              tunnel: [w2542 w2559] -> w2525
              tunnel: [State_Type_Definitions,_for_0.26g_versions_and_later_3."Idle" ("Enum") State_Type_Definitions,_for_0.26g_versions_and_later_3."Shutdown" ("Enum")] -> w2524
              tunnel: w2526 -> [w2533 _]
              tunnel: w2531 -> [w2538 w2556]
              tunnel: w2522 -> [w2537 _]
              frame "Start Task 1", Default {
                # ">> Is time up? >>"
                # "Determines if object is in range to pick up"
                # ">> Manual override >>"
                n840 = case shown="True" w2537 {
                  tunnel: [w2546 w2552] -> w2542
                  tunnel: w2538 -> [w2544 w2550]
                  frame False {
                    n841 = for {
                      tunnel: string[] ["CLOSE CLAW", "START TIMER"] ("element") -> [w2547] mode=indexing
                      shift-right: [w2549] -> w2546
                      shift-left: w2544 -> [w2548]
                      n842 = Enqueue Element(queue=w2548, element=w2547) -> (queue out=w2549:refnum<queue>)  [unwired: 2 in, 2 out]
                    }
                  }
                  frame True {
                    n843 = for {
                      shift-right: [w2554] -> w2552
                      shift-left: w2550 -> [w2555]
                      tunnel: string[] ["READ STEPPER VALUES", "", ""] -> [w2553] mode=indexing
                      n844 = Enqueue Element(queue=w2555, element=w2553) -> (queue out=w2554:refnum<queue>)  [unwired: 2 in, 2 out]
                    }
                  }
                }
                n845 = Or(x=w2537, y=w2533) -> (x .or. y?=w2540:bool)
                n846 = Select(t=State_Type_Definitions,_for_0.26g_versions_and_later_3."True Stop" ("Enum"), s=w2533, f=State_Type_Definitions,_for_0.26g_versions_and_later_3."Task 8K: RAISE MY SWORD" ("Enum")) -> (s? t:f=w2535:T18)
                n847 = Select(t=w2535, s=w2540, f=State_Type_Definitions,_for_0.26g_versions_and_later_3."Task 8J: CLOSE CLAW" ("Enum")) -> (s? t:f=w2539:T18)
              }
              frame "Exit" {
                n848 = for {
                  shift-right: [w2562] -> w2559
                  shift-left: w2556 -> [w2563]
                  tunnel: string[] ["STOP", "RESET ENCODERS", "RESET YAW", "ARDUINO MODE 0"] -> [w2561] mode=indexing
                  n849 = Enqueue Element(queue=w2563, element=w2561) -> (queue out=w2562:refnum<queue>)  [unwired: 2 in, 2 out]
                }
              }
            }
          }
          frame "Task 8K: RAISE MY SWORD" {
            # ">>> Motor control cluster >>>"
            # ">>> yStepper command>>>"
            # ">> Manual override >>"
            n850 = Dequeue Element(queue=w2574, timeout in ms (-1)=w2573, error in (no error)=w2575) -> (element=w2572:T10)  [unwired: 3 out]
            n851 = Equal?(x=w2571, y=u8 40) -> (x = y?=w2569:bool)
            n852 = case shown="\"Start Task 1\", Default" w2572 {
              tunnel: [w2585 State_Type_Definitions,_for_0.26g_versions_and_later_3."True Stop" ("Enum")] -> w2576
              tunnel: [w2588 w2605] -> w2577
              tunnel: [State_Type_Definitions,_for_0.26g_versions_and_later_3."Idle" ("Enum") State_Type_Definitions,_for_0.26g_versions_and_later_3."Shutdown" ("Enum")] -> w2578
              tunnel: w2569 -> [w2584 _]
              tunnel: w2568 -> [w2583 _]
              tunnel: w2567 -> [w2579 w2602]
              frame "Start Task 1", Default {
                # "Stays in Task 5_A until stepper reaches desired \nheight"
                # "T: Go back to idle, F: Continue with task\""
                # ">> Manual override >>"
                n853 = case shown="False" w2584 {
                  tunnel: [w2592 w2598] -> w2588
                  tunnel: w2579 -> [w2590 w2596]
                  frame False {
                    n854 = for {
                      tunnel: string[] ["Z STEPPER BOX HEIGHT", "READ STEPPER VALUES"] ("element") -> [w2593] mode=indexing
                      shift-right: [w2595] -> w2592
                      shift-left: w2590 -> [w2594]
                      n855 = Enqueue Element(queue=w2594, element=w2593) -> (queue out=w2595:refnum<queue>)  [unwired: 2 in, 2 out]
                    }
                  }
                  frame True {
                    n856 = for {
                      shift-right: [w2600] -> w2598
                      shift-left: w2596 -> [w2601]
                      tunnel: string[] ["CAM CLOSE", "DISPOSE CAM BUFFERS", "DISPOSE PROC BUFFERS", "RESET FLAGS"] -> [w2599] mode=indexing
                      n857 = Enqueue Element(queue=w2601, element=w2599) -> (queue out=w2600:refnum<queue>)  [unwired: 2 in, 2 out]
                    }
                  }
                }
                n858 = Or(x=w2584, y=w2583) -> (x .or. y?=w2586:bool)
                n859 = Select(t=State_Type_Definitions,_for_0.26g_versions_and_later_3."True Stop" ("Enum"), s=w2583, f=State_Type_Definitions,_for_0.26g_versions_and_later_3."Task A9: REVERSE" ("Enum")) -> (s? t:f=w2580:T18)
                n860 = Select(t=w2580, s=w2586, f=State_Type_Definitions,_for_0.26g_versions_and_later_3."Task 8K: RAISE MY SWORD" ("Enum")) -> (s? t:f=w2585:T18)
              }
              frame "Exit" {
                n861 = for {
                  shift-right: [w2608] -> w2605
                  shift-left: w2602 -> [w2609]
                  tunnel: string[] ["STOP", "RESET ENCODERS", "RESET YAW", "ARDUINO MODE 0"] -> [w2607] mode=indexing
                  n862 = Enqueue Element(queue=w2609, element=w2607) -> (queue out=w2608:refnum<queue>)  [unwired: 2 in, 2 out]
                }
              }
            }
          }
          frame "Task 8I: STILL WAITING" {
            # ">>> Motor control cluster >>>"
            # ">>> yStepper command>>>"
            # ">> Manual override >>"
            n863 = Dequeue Element(queue=w2617, timeout in ms (-1)=w2616, error in (no error)=w2618) -> (element=w2615:T10)  [unwired: 3 out]
            n864 = case shown="\"Start Task 1\", Default" w2615 {
              tunnel: [w2625 State_Type_Definitions,_for_0.26g_versions_and_later_3."True Stop" ("Enum")] -> w2619
              tunnel: [w2627 w2644] -> w2620
              tunnel: [State_Type_Definitions,_for_0.26g_versions_and_later_3."Idle" ("Enum") State_Type_Definitions,_for_0.26g_versions_and_later_3."Shutdown" ("Enum")] -> w2621
              tunnel: w2614 -> [w2622 _]
              tunnel: w2613 -> [w2623 w2641]
              frame "Start Task 1", Default {
                # "Stays in Task 5_A until stepper reaches desired \nheight"
                # "T: Go back to idle, F: Continue with task\""
                # ">> Manual override >>"
                n865 = case shown="True" w2622 {
                  tunnel: [w2631 w2637] -> w2627
                  tunnel: w2623 -> [w2629 w2635]
                  frame False {
                    n866 = for {
                      tunnel: string[] ["READ NAVX", "READ IR"] ("element") -> [w2632] mode=indexing
                      shift-right: [w2634] -> w2631
                      shift-left: w2629 -> [w2633]
                      n867 = Enqueue Element(queue=w2633, element=w2632) -> (queue out=w2634:refnum<queue>)  [unwired: 2 in, 2 out]
                    }
                  }
                  frame True {
                    n868 = for {
                      shift-right: [w2639] -> w2637
                      shift-left: w2635 -> [w2640]
                      tunnel: string[] ["RESET ENCODERS", "RESET YAW", "RESET FLAGS", ""] -> [w2638] mode=indexing
                      n869 = Enqueue Element(queue=w2640, element=w2638) -> (queue out=w2639:refnum<queue>)  [unwired: 2 in, 2 out]
                    }
                  }
                }
                n870 = Select(t=State_Type_Definitions,_for_0.26g_versions_and_later_3."True Stop" ("Enum"), s=w2622, f=State_Type_Definitions,_for_0.26g_versions_and_later_3."Task 8I: STILL WAITING" ("Enum")) -> (s? t:f=w2625:T18)
              }
              frame "Exit" {
                n871 = for {
                  shift-right: [w2647] -> w2644
                  shift-left: w2641 -> [w2648]
                  tunnel: string[] ["STOP", "RESET ENCODERS", "RESET YAW", "ARDUINO MODE 0"] -> [w2646] mode=indexing
                  n872 = Enqueue Element(queue=w2648, element=w2646) -> (queue out=w2647:refnum<queue>)  [unwired: 2 in, 2 out]
                }
              }
            }
          }
          frame "Task 8L: Return to position" {
            # ">>> Motor control cluster >>>"
            # ">>> yStepper command>>>"
            # ">> Manual override >>"
            n873 = call "yDistance travelled FGV.vi"("Init/Read/Write State"=States_for_Action_Engine."Read") -> ("Output"=w2653:dbl)  [unwired: 9 in, 1 out]
            n874 = Dequeue Element(queue=w2662, timeout in ms (-1)=w2661, error in (no error)=w2663) -> (element=w2660:T10)  [unwired: 3 out]
            n875 = Multiply(x=w2653, y=-1.0) -> (x*y=w2650:dbl)
            n876 = Less Or Equal?(x=w2651, y=w2650) -> (x <= y?=w2649:bool)
            n877 = case shown="\"Start Task 1\", Default" w2660 {
              tunnel: [w2672 State_Type_Definitions,_for_0.26g_versions_and_later_3."True Stop" ("Enum")] -> w2664
              tunnel: [w2674 w2691] -> w2665
              tunnel: [State_Type_Definitions,_for_0.26g_versions_and_later_3."Idle" ("Enum") State_Type_Definitions,_for_0.26g_versions_and_later_3."Shutdown" ("Enum")] -> w2666
              tunnel: w2659 -> [w2668 _]
              tunnel: w2658 -> [w2670 w2688]
              tunnel: w2649 -> [w2669 _]
              frame "Start Task 1", Default {
                # "Stays in Task 5_A until stepper reaches desired \nheight"
                # "T: Go back to idle, F: Continue with task\""
                # ">> Manual override >>"
                n878 = Or(x=w2669, y=w2668) -> (x .or. y?=w2667:bool)
                n879 = case shown="False" w2667 {
                  tunnel: [w2678 w2684] -> w2674
                  tunnel: w2670 -> [w2676 w2682]
                  frame False {
                    n880 = for {
                      tunnel: string[] ["READ NAVX", "LEFT"] ("element") -> [w2679] mode=indexing
                      shift-right: [w2681] -> w2678
                      shift-left: w2676 -> [w2680]
                      n881 = Enqueue Element(queue=w2680, element=w2679) -> (queue out=w2681:refnum<queue>)  [unwired: 2 in, 2 out]
                    }
                  }
                  frame True {
                    n882 = for {
                      shift-right: [w2686] -> w2684
                      shift-left: w2682 -> [w2687]
                      tunnel: string[] ["RESET ENCODERS", "RESET YAW", "RESET FLAGS", ""] -> [w2685] mode=indexing
                      n883 = Enqueue Element(queue=w2687, element=w2685) -> (queue out=w2686:refnum<queue>)  [unwired: 2 in, 2 out]
                    }
                  }
                }
                n884 = Select(t=State_Type_Definitions,_for_0.26g_versions_and_later_3."True Stop" ("Enum"), s=w2667, f=State_Type_Definitions,_for_0.26g_versions_and_later_3."Task 8L: Return to position" ("Enum")) -> (s? t:f=w2672:T18)
              }
              frame "Exit" {
                n885 = for {
                  shift-right: [w2694] -> w2691
                  shift-left: w2688 -> [w2695]
                  tunnel: string[] ["STOP", "RESET ENCODERS", "RESET YAW", "ARDUINO MODE 0"] -> [w2693] mode=indexing
                  n886 = Enqueue Element(queue=w2695, element=w2693) -> (queue out=w2694:refnum<queue>)  [unwired: 2 in, 2 out]
                }
              }
            }
          }
          frame "Task 9A: Raise Arm" {
            # ">>> Motor control cluster >>>"
            # ">> Stepper height reeached >>"
            # ">>> yStepper command>>>"
            # ">> Manual override >>"
            n887 = Dequeue Element(queue=w2708, timeout in ms (-1)=w2703, error in (no error)=w2707) -> (element=w2710:T10)  [unwired: 3 out]
            n888 = Equal?(x=w2705, y=u8 40) -> (x = y?=w2696:bool)
            n889 = case shown="\"Start Task 1\", Default" w2710 {
              tunnel: [w2721 State_Type_Definitions,_for_0.26g_versions_and_later_3."True Stop" ("Enum")] -> w2701
              tunnel: [w2719 w2736] -> w2700
              tunnel: w2704 -> [w2718 _]
              tunnel: w2706 -> [w2712 _]
              tunnel: [State_Type_Definitions,_for_0.26g_versions_and_later_3."Idle" ("Enum") State_Type_Definitions,_for_0.26g_versions_and_later_3."Shutdown" ("Enum")] -> w2702
              tunnel: w2696 -> [w2711 _]
              frame "Start Task 1", Default {
                # ">> WIill proceed to part ii if not manual override >>"
                # ">>If ENABLE or Trigger is set to true>>"
                n890 = Or(x=w2711, y=w2712) -> (x .or. y?=w2713:bool)
                n891 = case shown="False" w2711 {
                  tunnel: [w2724 w2730] -> w2719
                  tunnel: w2718 -> [w2723 w2729]
                  frame False {
                    n892 = for {
                      shift-right: [w2726] -> w2724
                      shift-left: w2723 -> [w2727]
                      tunnel: string[] ["Z STEPPER BOX HEIGHT", "READ STEPPER VALUES"] ("element") -> [w2725] mode=indexing
                      n893 = Enqueue Element(queue=w2727, element=w2725) -> (queue out=w2726:refnum<queue>)  [unwired: 2 in, 2 out]
                    }
                  }
                  frame True {
                    n894 = for {
                      shift-right: [w2732] -> w2730
                      shift-left: w2729 -> [w2733]
                      tunnel: string[] ["READ NAVX", "RESET FLAGS", "RESET YAW", "", "", ""] -> [w2731] mode=indexing
                      n895 = Enqueue Element(queue=w2733, element=w2731) -> (queue out=w2732:refnum<queue>)  [unwired: 2 in, 2 out]
                    }
                  }
                }
                n896 = Select(t=State_Type_Definitions,_for_0.26g_versions_and_later_3."True Stop" ("Enum"), s=w2712, f=State_Type_Definitions,_for_0.26g_versions_and_later_3."Task 9B: Rotate to Angle" ("Enum")) -> (s? t:f=w2715:T18)
                n897 = Select(t=w2715, s=w2713, f=State_Type_Definitions,_for_0.26g_versions_and_later_3."Task 9A: Raise Arm" ("Enum")) -> (s? t:f=w2721:T18)
              }
              frame "Exit" {
                n898 = for {
                  shift-right: [w2739] -> w2736
                  shift-left: _ -> [w2740]
                  tunnel: string[] ["STOP", "RESET ENCODERS", "RESET YAW", ""] -> [w2738] mode=indexing
                  n899 = Enqueue Element(queue=w2740, element=w2738) -> (queue out=w2739:refnum<queue>)  [unwired: 2 in, 2 out]
                }
              }
            }
          }
          frame "Task 9B: Rotate to Angle" {
            # ">>> Motor control cluster >>>"
            # ">>> yStepper command>>>"
            n900 = Dequeue Element(queue=w2754, timeout in ms (-1)=w2753, error in (no error)=w2752) -> (element=w2756:T10)  [unwired: 3 out]
            n901 = In Range and Coerce(upper limit=65.0, x=w2746, lower limit=58.0) -> (In Range?=w2741:bool)  [unwired: 1 out]
            n902 = case shown="\"Start Task 1\", Default" w2756 {
              tunnel: w2747 -> [w2759 _]
              tunnel: [w2767 State_Type_Definitions,_for_0.26g_versions_and_later_3."True Stop" ("Enum")] -> w2749
              tunnel: w2755 -> [w2765 w2783]
              tunnel: [w2764 w2782] -> w2748
              tunnel: [State_Type_Definitions,_for_0.26g_versions_and_later_3."Idle" ("Enum") State_Type_Definitions,_for_0.26g_versions_and_later_3."Shutdown" ("Enum")] -> w2750
              tunnel: w2741 -> [w2757 _]
              frame "Start Task 1", Default {
                n903 = Or(x=w2757, y=w2759) -> (x .or. y?=w2758:bool)
                n904 = case shown="False" w2757 {
                  tunnel: w2765 -> [w2770 w2776]
                  tunnel: [w2769 w2774] -> w2764
                  frame False {
                    n905 = for {
                      shift-right: [w2772] -> w2769
                      shift-left: w2770 -> [w2773]
                      tunnel: string[] ["READ NAVX", "R-CW", ""] ("element") -> [w2771] mode=indexing
                      n906 = Enqueue Element(queue=w2773, element=w2771) -> (queue out=w2772:refnum<queue>)  [unwired: 2 in, 2 out]
                    }
                  }
                  frame True {
                    n907 = for {
                      shift-right: [w2778] -> w2774
                      shift-left: w2776 -> [w2779]
                      tunnel: string[] ["STOP", "RESET ENCODERS", "RESET YAW", "", ""] -> [w2777] mode=indexing
                      n908 = Enqueue Element(queue=w2779, element=w2777) -> (queue out=w2778:refnum<queue>)  [unwired: 2 in, 2 out]
                    }
                  }
                }
                n909 = Select(t=State_Type_Definitions,_for_0.26g_versions_and_later_3."True Stop" ("Enum"), s=w2759, f=State_Type_Definitions,_for_0.26g_versions_and_later_3."Task 9D: MOVE FORWARD") -> (s? t:f=w2761:T18)
                n910 = Select(t=w2761, s=w2758, f=State_Type_Definitions,_for_0.26g_versions_and_later_3."Task 9B: Rotate to Angle" ("Enum")) -> (s? t:f=w2767:T18)
              }
              frame "Exit" {
                n911 = for {
                  shift-right: [w2786] -> w2782
                  shift-left: w2783 -> [w2787]
                  tunnel: string[] ["STOP", "RESET ENCODERS", "RESET YAW", ""] -> [w2785] mode=indexing
                  n912 = Enqueue Element(queue=w2787, element=w2785) -> (queue out=w2786:refnum<queue>)  [unwired: 2 in, 2 out]
                }
              }
            }
          }
          frame "Task 9C: Detect Box" {
            # ">>> Motor control cluster >>>"
            # ">>Line Detected>>"
            # ">>Action Queue>>"
            # ">>> yStepper command>>>"
            n913 = Dequeue Element(queue=w2799, timeout in ms (-1)=w2798, error in (no error)=w2797) -> (element=w2800:T10)  [unwired: 3 out]
            n914 = case shown="\"Start Task 1\", Default" w2800 {
              tunnel: w2795 -> [w2801 _]
              tunnel: [w2811 State_Type_Definitions,_for_0.26g_versions_and_later_3."True Stop" ("Enum")] -> w2792
              tunnel: w2796 -> [w2809 w2827]
              tunnel: [w2808 w2826] -> w2791
              tunnel: [State_Type_Definitions,_for_0.26g_versions_and_later_3."Idle" ("Enum") State_Type_Definitions,_for_0.26g_versions_and_later_3."Shutdown" ("Enum")] -> w2794
              tunnel: w2788 -> [w2802 _]
              frame "Start Task 1", Default {
                n915 = Or(x=w2801, y=w2802) -> (x .or. y?=w2803:bool)
                n916 = case shown="True" w2802 {
                  tunnel: w2809 -> [w2814 w2820]
                  tunnel: [w2813 w2818] -> w2808
                  frame False {
                    n917 = for {
                      shift-right: [w2816] -> w2813
                      shift-left: w2814 -> [w2817]
                      tunnel: string[] ["READ IR", "READ LINE SENSOR", "FORWARD - IR ASSIST"] ("element") -> [w2815] mode=indexing
                      n918 = Enqueue Element(queue=w2817, element=w2815) -> (queue out=w2816:refnum<queue>)  [unwired: 2 in, 2 out]
                    }
                  }
                  frame True {
                    n919 = for {
                      shift-right: [w2822] -> w2818
                      shift-left: w2820 -> [w2823]
                      tunnel: string[] ["STOP", "RESET ENCODERS", "RESET YAW", "RESET FLAGS", "ARDUINO - ULTRASONIC"] -> [w2821] mode=indexing
                      n920 = Enqueue Element(queue=w2823, element=w2821) -> (queue out=w2822:refnum<queue>)  [unwired: 2 in, 2 out]
                    }
                  }
                }
                n921 = Select(t=State_Type_Definitions,_for_0.26g_versions_and_later_3."True Stop" ("Enum"), s=w2801, f=State_Type_Definitions,_for_0.26g_versions_and_later_3."Task 9D: MOVE FORWARD") -> (s? t:f=w2805:T18)
                n922 = Select(t=w2805, s=w2803, f=State_Type_Definitions,_for_0.26g_versions_and_later_3."Task 9C: Detect Box" ("Enum")) -> (s? t:f=w2811:T18)
              }
              frame "Exit" {
                n923 = for {
                  shift-right: [w2830] -> w2826
                  shift-left: w2827 -> [w2831]
                  tunnel: string[] ["STOP", "RESET ENCODERS", "RESET YAW", ""] -> [w2829] mode=indexing
                  n924 = Enqueue Element(queue=w2831, element=w2829) -> (queue out=w2830:refnum<queue>)  [unwired: 2 in, 2 out]
                }
              }
            }
          }
          frame "Task 9D: MOVE FORWARD" {
            (unwired) u8 50 ("y")
            # "Use 20 low voltage\nUse 25 high voltage"
            # ">> Item Selection Bias >>"
            # ">> Wall detected >>"
            # ">> Manual override >>"
            # ">>Table Detected>>"
            # ">>> Motor control cluster >>>"
            # ">>Table or wall detectected>>"
            # ">>Action Queue>>"
            # ">>> yStepper command>>>"
            n925 = Dequeue Element(queue=w2853, timeout in ms (-1)=w2852, error in (no error)=w2851) -> (element=w2854:T10)  [unwired: 3 out]
            n926 = Less Or Equal?(x=w2842, y=25.0) -> (x <= y?=w2838:bool)
            n927 = Less?(x=w2840, y=600.0) -> (x < y?=w2834:bool)
            n928 = Greater Or Equal?(x=w2836, y=620.0) -> (x >= y?=w2835:bool)
            n929 = And(x=w2834, y=w2835) -> (x .and. y?=w2833:bool)
            n930 = Or(x=w2838, y=w2833) -> (x .or. y?=w2837:bool)
            n931 = case shown="\"Start Task 1\", Default" w2854 {
              tunnel: w2849 -> [w2855 _]
              tunnel: [w2865 State_Type_Definitions,_for_0.26g_versions_and_later_3."True Stop" ("Enum")] -> w2846
              tunnel: w2850 -> [w2863 w2881]
              tunnel: [w2862 w2880] -> w2845
              tunnel: [State_Type_Definitions,_for_0.26g_versions_and_later_3."Idle" ("Enum") State_Type_Definitions,_for_0.26g_versions_and_later_3."Shutdown" ("Enum")] -> w2848
              tunnel: w2837 -> [w2856 _]
              frame "Start Task 1", Default {
                n932 = Or(x=w2855, y=w2856) -> (x .or. y?=w2857:bool)
                n933 = case shown="True" w2856 {
                  tunnel: w2863 -> [w2868 w2874]
                  tunnel: [w2867 w2872] -> w2862
                  frame False {
                    n934 = for {
                      shift-right: [w2870] -> w2867
                      shift-left: w2868 -> [w2871]
                      tunnel: string[] ["READ IR", "FORWARD - IR ASSIST", "READ ENCODERS"] ("element") -> [w2869] mode=indexing
                      n935 = Enqueue Element(queue=w2871, element=w2869) -> (queue out=w2870:refnum<queue>)  [unwired: 2 in, 2 out]
                    }
                  }
                  frame True {
                    n936 = for {
                      shift-right: [w2876] -> w2872
                      shift-left: w2874 -> [w2877]
                      tunnel: string[] ["STOP", "RESET ENCODERS", "RESET YAW", "RESET FLAGS"] -> [w2875] mode=indexing
                      n937 = Enqueue Element(queue=w2877, element=w2875) -> (queue out=w2876:refnum<queue>)  [unwired: 2 in, 2 out]
                    }
                  }
                }
                n938 = Select(t=State_Type_Definitions,_for_0.26g_versions_and_later_3."True Stop" ("Enum"), s=w2855, f=State_Type_Definitions,_for_0.26g_versions_and_later_3."Task 9E: MOVE LEFT") -> (s? t:f=w2859:T18)
                n939 = Select(t=w2859, s=w2857, f=State_Type_Definitions,_for_0.26g_versions_and_later_3."Task 9D: MOVE FORWARD" ("Enum")) -> (s? t:f=w2865:T18)
              }
              frame "Exit" {
                n940 = for {
                  shift-right: [w2884] -> w2880
                  shift-left: w2881 -> [w2885]
                  tunnel: string[] ["STOP", "RESET ENCODERS", "RESET YAW", ""] -> [w2883] mode=indexing
                  n941 = Enqueue Element(queue=w2885, element=w2883) -> (queue out=w2884:refnum<queue>)  [unwired: 2 in, 2 out]
                }
              }
            }
          }
          frame "Task 9D2: ANGLE CORRECTION" {
            # "Min: 48 ~ 50\nMax: 52 ~ 54"
            # ">>> Motor control cluster >>>"
            # ">>> yStepper command>>>"
            n942 = Dequeue Element(queue=w2899, timeout in ms (-1)=w2898, error in (no error)=w2897) -> (element=w2901:T10)  [unwired: 3 out]
            n943 = In Range and Coerce(upper limit=54.0, x=w2891, lower limit=50.0) -> (In Range?=w2886:bool)  [unwired: 1 out]
            n944 = case shown="\"Start Task 1\", Default" w2901 {
              tunnel: w2892 -> [w2904 _]
              tunnel: [w2912 State_Type_Definitions,_for_0.26g_versions_and_later_3."True Stop" ("Enum")] -> w2894
              tunnel: w2900 -> [w2910 w2928]
              tunnel: [w2909 w2927] -> w2893
              tunnel: [State_Type_Definitions,_for_0.26g_versions_and_later_3."Idle" ("Enum") State_Type_Definitions,_for_0.26g_versions_and_later_3."Shutdown" ("Enum")] -> w2895
              tunnel: w2886 -> [w2902 _]
              frame "Start Task 1", Default {
                n945 = Or(x=w2902, y=w2904) -> (x .or. y?=w2903:bool)
                n946 = case shown="False" w2902 {
                  tunnel: w2910 -> [w2915 w2921]
                  tunnel: [w2914 w2919] -> w2909
                  frame False {
                    n947 = for {
                      shift-right: [w2917] -> w2914
                      shift-left: w2915 -> [w2918]
                      tunnel: string[] ["READ NAVX", "R-ACW", ""] ("element") -> [w2916] mode=indexing
                      n948 = Enqueue Element(queue=w2918, element=w2916) -> (queue out=w2917:refnum<queue>)  [unwired: 2 in, 2 out]
                    }
                  }
                  frame True {
                    n949 = for {
                      shift-right: [w2923] -> w2919
                      shift-left: w2921 -> [w2924]
                      tunnel: string[] ["STOP", "RESET ENCODERS", "RESET YAW", "", ""] -> [w2922] mode=indexing
                      n950 = Enqueue Element(queue=w2924, element=w2922) -> (queue out=w2923:refnum<queue>)  [unwired: 2 in, 2 out]
                    }
                  }
                }
                n951 = Select(t=State_Type_Definitions,_for_0.26g_versions_and_later_3."True Stop" ("Enum"), s=w2904, f=State_Type_Definitions,_for_0.26g_versions_and_later_3."Task 9E: MOVE LEFT") -> (s? t:f=w2906:T18)
                n952 = Select(t=w2906, s=w2903, f=State_Type_Definitions,_for_0.26g_versions_and_later_3."Task 9D2: ANGLE CORRECTION" ("Enum")) -> (s? t:f=w2912:T18)
              }
              frame "Exit" {
                n953 = for {
                  shift-right: [w2931] -> w2927
                  shift-left: w2928 -> [w2932]
                  tunnel: string[] ["STOP", "RESET ENCODERS", "RESET YAW", ""] -> [w2930] mode=indexing
                  n954 = Enqueue Element(queue=w2932, element=w2930) -> (queue out=w2931:refnum<queue>)  [unwired: 2 in, 2 out]
                }
              }
            }
          }
          frame "Task 9E: MOVE LEFT" {
            # "High battery voltage: 15"
            # ">> Item Selection Bias >>"
            # ">>Stops if either table or wall is obstructing >>"
            n955 = Less?(x=w2933, y=15.0) -> (x < y?=w2943:bool)
            n956 = Dequeue Element(queue=w2941, timeout in ms (-1)=w2940, error in (no error)=w2939) -> (element=w2945:T10)  [unwired: 3 out]
            n957 = case shown="\"Start Task 1\", Default" w2945 {
              tunnel: w2943 -> [w2950 _]
              tunnel: [w2957 State_Type_Definitions,_for_0.26g_versions_and_later_3."True Stop" ("Enum")] -> w2935
              tunnel: w2938 -> [w2949 _]
              tunnel: w2942 -> [w2956 w2973]
              tunnel: [w2955 w2974] -> w2936
              tunnel: [State_Type_Definitions,_for_0.26g_versions_and_later_3."Idle" ("Enum") State_Type_Definitions,_for_0.26g_versions_and_later_3."Shutdown" ("Enum")] -> w2934
              frame "Start Task 1", Default {
                n958 = case shown="False" w2950 {
                  tunnel: w2956 -> [w2960 w2967]
                  tunnel: [w2961 w2966] -> w2955
                  frame False {
                    n959 = for {
                      tunnel: string[] ["LEFT", "READ NAVX", "READ IR", ""] ("element") -> [w2962] mode=indexing
                      shift-right: [w2964] -> w2961
                      shift-left: w2960 -> [w2963]
                      n960 = Enqueue Element(queue=w2963, element=w2962) -> (queue out=w2964:refnum<queue>)  [unwired: 2 in, 2 out]
                    }
                  }
                  frame True {
                    n961 = for {
                      shift-right: [w2969] -> w2966
                      shift-left: w2967 -> [w2970]
                      tunnel: string[] ["STOP", "RESET ENCODERS", "RESET FLAGS", "RESET YAW", "READ IR", ""] -> [w2968] mode=indexing
                      n962 = Enqueue Element(queue=w2970, element=w2968) -> (queue out=w2969:refnum<queue>)  [unwired: 2 in, 2 out]
                    }
                  }
                }
                n963 = Or(x=w2950, y=w2949) -> (x .or. y?=w2948:bool)
                n964 = Select(t=State_Type_Definitions,_for_0.26g_versions_and_later_3."True Stop" ("Enum"), s=w2949, f=State_Type_Definitions,_for_0.26g_versions_and_later_3."Task 9E2: MOVE RIGHT" ("Enum")) -> (s? t:f=w2951:T18)
                n965 = Select(t=w2951, s=w2948, f=State_Type_Definitions,_for_0.26g_versions_and_later_3."Task 9E: MOVE LEFT" ("Enum")) -> (s? t:f=w2957:T18)
              }
              frame "Exit" {
                n966 = for {
                  shift-right: [w2977] -> w2974
                  shift-left: w2973 -> [w2978]
                  tunnel: string[] ["STOP", "RESET ENCODERS", "RESET YAW", "ARDUINO MODE 0"] -> [w2976] mode=indexing
                  n967 = Enqueue Element(queue=w2978, element=w2976) -> (queue out=w2977:refnum<queue>)  [unwired: 2 in, 2 out]
                }
              }
            }
          }
          frame "Task 9E2: MOVE RIGHT" {
            # ">>> Motor control cluster >>>"
            # ">>> yStepper command>>>"
            n968 = Dequeue Element(queue=w2986, timeout in ms (-1)=w2985, error in (no error)=w2984) -> (element=w2991:T10)  [unwired: 3 out]
            n969 = case shown="\"Start Task 1\", Default" w2991 {
              tunnel: w2979 -> [w2994 _]
              tunnel: [w3001 State_Type_Definitions,_for_0.26g_versions_and_later_3."True Stop" ("Enum")] -> w2990
              tunnel: w2983 -> [w2993 _]
              tunnel: w2987 -> [w3000 w3017]
              tunnel: [w2999 w3018] -> w2989
              tunnel: [State_Type_Definitions,_for_0.26g_versions_and_later_3."Idle" ("Enum") State_Type_Definitions,_for_0.26g_versions_and_later_3."Shutdown" ("Enum")] -> w2988
              frame "Start Task 1", Default {
                n970 = case shown="True" w2994 {
                  tunnel: w3000 -> [w3004 w3011]
                  tunnel: [w3005 w3010] -> w2999
                  frame False {
                    n971 = for {
                      tunnel: string[] ["READ LINE SENSOR", "READ NAVX", "RIGHT", "READ ENCODERS"] ("element") -> [w3006] mode=indexing
                      shift-right: [w3008] -> w3005
                      shift-left: w3004 -> [w3007]
                      n972 = Enqueue Element(queue=w3007, element=w3006) -> (queue out=w3008:refnum<queue>)  [unwired: 2 in, 2 out]
                    }
                  }
                  frame True {
                    n973 = for {
                      shift-right: [w3013] -> w3010
                      shift-left: w3011 -> [w3014]
                      tunnel: string[] ["RESET ENCODERS", "RESET YAW", "RESET FLAGS", "STOP", "BOX COLOUR"] -> [w3012] mode=indexing
                      n974 = Enqueue Element(queue=w3014, element=w3012) -> (queue out=w3013:refnum<queue>)  [unwired: 2 in, 2 out]
                    }
                  }
                }
                n975 = Or(x=w2994, y=w2993) -> (x .or. y?=w2992:bool)
                n976 = Select(t=State_Type_Definitions,_for_0.26g_versions_and_later_3."True Stop" ("Enum"), s=w2993, f=State_Type_Definitions,_for_0.26g_versions_and_later_3."Task 9F: SCAN BOX" ("Enum")) -> (s? t:f=w2995:T18)
                n977 = Select(t=w2995, s=w2992, f=State_Type_Definitions,_for_0.26g_versions_and_later_3."Task 9E2: MOVE RIGHT" ("Enum")) -> (s? t:f=w3001:T18)
              }
              frame "Exit" {
                n978 = for {
                  shift-right: [w3021] -> w3018
                  shift-left: w3017 -> [w3022]
                  tunnel: string[] ["STOP", "RESET ENCODERS", "RESET YAW", "ARDUINO MODE 0"] -> [w3020] mode=indexing
                  n979 = Enqueue Element(queue=w3022, element=w3020) -> (queue out=w3021:refnum<queue>)  [unwired: 2 in, 2 out]
                }
              }
            }
          }
          frame "Task 9F: SCAN BOX" {
            # ">>> Motor control cluster >>>"
            # ">>Colour detection >>"
            # ">>> yStepper command>>>"
            # ">> Manual override >>"
            n980 = Dequeue Element(queue=w3039, timeout in ms (-1)=w3037, error in (no error)=w3038) -> (element=w3032:T10)  [unwired: 3 out]
            n981 = call "Box Colour FGV.vi"("Init/R/W State"=Box_Colour_FGV_States."Read") -> ("Colour to detect (output)"=w3025:T2)  [unwired: 9 in, 1 out]
            n982 = Equal?(x=w3026, y=w3025) -> (x = y?=w3024:bool)
            n983 = case shown="\"Start Task 1\", Default" w3032 {
              tunnel: [w3052 State_Type_Definitions,_for_0.26g_versions_and_later_3."True Stop" ("Enum")] -> w3029
              tunnel: [w3050 w3067] -> w3030
              tunnel: w3031 -> [w3049 _]
              tunnel: w3033 -> [w3042 _]
              tunnel: [State_Type_Definitions,_for_0.26g_versions_and_later_3."Idle" ("Enum") State_Type_Definitions,_for_0.26g_versions_and_later_3."Shutdown" ("Enum")] -> w3028
              tunnel: w3023 -> [w3043 _]
              tunnel: w3024 -> [w3041 _]
              frame "Start Task 1", Default {
                # ">> Will stop either due to manual override or is same box colour >>"
                # ">> WIill proceed to part ii if not manual override >>"
                # ">>If ENABLE or Trigger is set to true>>"
                n984 = Or(x=w3043, y=w3042) -> (x .or. y?=w3044:bool)
                n985 = case shown="True" w3043 {
                  tunnel: [w3055 w3061] -> w3050
                  tunnel: w3049 -> [w3054 w3060]
                  frame False {
                    n986 = for {
                      shift-right: [w3057] -> w3055
                      shift-left: w3054 -> [w3058]
                      tunnel: string[] ["", ""] ("element") -> [w3056] mode=indexing
                      n987 = Enqueue Element(queue=w3058, element=w3056) -> (queue out=w3057:refnum<queue>)  [unwired: 2 in, 2 out]
                    }
                  }
                  frame True {
                    n988 = for {
                      shift-right: [w3063] -> w3061
                      shift-left: w3060 -> [w3064]
                      tunnel: string[] ["RESET ENCODER", "RESET FLAGS", "RESET YAW", "", "", ""] -> [w3062] mode=indexing
                      n989 = Enqueue Element(queue=w3064, element=w3062) -> (queue out=w3063:refnum<queue>)  [unwired: 2 in, 2 out]
                    }
                  }
                }
                n990 = Or(x=w3042, y=w3041) -> (x .or. y?=w3040:bool)
                n991 = Select(t=State_Type_Definitions,_for_0.26g_versions_and_later_3."Task A11: ARM DROP HEIGHT" ("Enum"), s=w3040, f=State_Type_Definitions,_for_0.26g_versions_and_later_3."Task 9G: MOVE RIGHT" ("Enum")) -> (s? t:f=w3046:T18)
                n992 = Select(t=w3046, s=w3044, f=State_Type_Definitions,_for_0.26g_versions_and_later_3."Task 9F: SCAN BOX" ("Enum")) -> (s? t:f=w3052:T18)
              }
              frame "Exit" {
                n993 = for {
                  shift-right: [w3070] -> w3067
                  shift-left: _ -> [w3071]
                  tunnel: string[] ["STOP", "RESET ENCODERS", "RESET YAW", ""] -> [w3069] mode=indexing
                  n994 = Enqueue Element(queue=w3071, element=w3069) -> (queue out=w3070:refnum<queue>)  [unwired: 2 in, 2 out]
                }
              }
            }
          }
          frame "Task 9G: MOVE RIGHT" {
            # ">>> Motor control cluster >>>"
            # ">>> yStepper command>>>"
            n995 = Dequeue Element(queue=w3083, timeout in ms (-1)=w3082, error in (no error)=w3081) -> (element=w3088:T10)  [unwired: 3 out]
            n996 = Greater?(x=w3073, y=50.0) -> (0:w3076:bool)
            n997 = And(x=w3074, y=w3076) -> (x .and. y?=w3072:bool)
            n998 = case shown="\"Start Task 1\", Default" w3088 {
              tunnel: w3072 -> [w3091 _]
              tunnel: [w3098 State_Type_Definitions,_for_0.26g_versions_and_later_3."True Stop" ("Enum")] -> w3087
              tunnel: w3080 -> [w3090 _]
              tunnel: w3084 -> [w3097 w3114]
              tunnel: [w3096 w3115] -> w3086
              tunnel: [State_Type_Definitions,_for_0.26g_versions_and_later_3."Idle" ("Enum") State_Type_Definitions,_for_0.26g_versions_and_later_3."Shutdown" ("Enum")] -> w3085
              frame "Start Task 1", Default {
                n999 = case shown="True" w3091 {
                  tunnel: w3097 -> [w3101 w3108]
                  tunnel: [w3102 w3107] -> w3096
                  frame False {
                    n1000 = for {
                      tunnel: string[] ["READ LINE SENSOR", "READ NAVX", "RIGHT", "READ ENCODERS"] ("element") -> [w3103] mode=indexing
                      shift-right: [w3105] -> w3102
                      shift-left: w3101 -> [w3104]
                      n1001 = Enqueue Element(queue=w3104, element=w3103) -> (queue out=w3105:refnum<queue>)  [unwired: 2 in, 2 out]
                    }
                  }
                  frame True {
                    n1002 = for {
                      shift-right: [w3110] -> w3107
                      shift-left: w3108 -> [w3111]
                      tunnel: string[] ["RESET ENCODERS", "RESET YAW", "RESET FLAGS", "STOP", "BOX COLOUR"] -> [w3109] mode=indexing
                      n1003 = Enqueue Element(queue=w3111, element=w3109) -> (queue out=w3110:refnum<queue>)  [unwired: 2 in, 2 out]
                    }
                  }
                }
                n1004 = Or(x=w3091, y=w3090) -> (x .or. y?=w3089:bool)
                n1005 = Select(t=State_Type_Definitions,_for_0.26g_versions_and_later_3."True Stop" ("Enum"), s=w3090, f=State_Type_Definitions,_for_0.26g_versions_and_later_3."Task 9H: SCAN BOX 2" ("Enum")) -> (s? t:f=w3092:T18)
                n1006 = Select(t=w3092, s=w3089, f=State_Type_Definitions,_for_0.26g_versions_and_later_3."Task 9G: MOVE RIGHT" ("Enum")) -> (s? t:f=w3098:T18)
              }
              frame "Exit" {
                n1007 = for {
                  shift-right: [w3118] -> w3115
                  shift-left: w3114 -> [w3119]
                  tunnel: string[] ["STOP", "RESET ENCODERS", "RESET YAW", "ARDUINO MODE 0"] -> [w3117] mode=indexing
                  n1008 = Enqueue Element(queue=w3119, element=w3117) -> (queue out=w3118:refnum<queue>)  [unwired: 2 in, 2 out]
                }
              }
            }
          }
          frame "Task 9H: SCAN BOX 2" {
            # ">> Item Selection Bias >>"
            # ">>> Motor control cluster >>>"
            # ">>> yStepper command>>>"
            n1009 = Dequeue Element(queue=w3129, timeout in ms (-1)=w3130, error in (no error)=w3131) -> (element=w3133:T10)  [unwired: 3 out]
            n1010 = call "Box Colour FGV.vi"("Init/R/W State"=Box_Colour_FGV_States."Read") -> ("Colour to detect (output)"=w3123:T2)  [unwired: 9 in, 1 out]
            n1011 = Equal?(x=w3122, y=w3123) -> (x = y?=w3121:bool)
            n1012 = case shown="\"Start Task 1\", Default" w3133 {
              tunnel: w3120 -> [w3141 _]
              tunnel: [w3148 State_Type_Definitions,_for_0.26g_versions_and_later_3."True Stop" ("Enum")] -> w3126
              tunnel: w3132 -> [w3138 _]
              tunnel: w3128 -> [w3147 w3164]
              tunnel: [w3146 w3165] -> w3127
              tunnel: [State_Type_Definitions,_for_0.26g_versions_and_later_3."Idle" ("Enum") State_Type_Definitions,_for_0.26g_versions_and_later_3."Shutdown" ("Enum")] -> w3125
              tunnel: w3121 -> [w3139 _]
              frame "Start Task 1", Default {
                n1013 = Or(x=w3141, y=w3138) -> (x .or. y?=w3140:bool)
                n1014 = Or(x=w3139, y=w3138) -> (x .or. y?=w3137:bool)
                n1015 = case shown="True" w3141 {
                  tunnel: w3147 -> [w3151 w3158]
                  tunnel: [w3152 w3157] -> w3146
                  frame False {
                    n1016 = for {
                      tunnel: string[] ["", "", "", ""] ("element") -> [w3153] mode=indexing
                      shift-right: [w3155] -> w3152
                      shift-left: w3151 -> [w3154]
                      n1017 = Enqueue Element(queue=w3154, element=w3153) -> (queue out=w3155:refnum<queue>)  [unwired: 2 in, 2 out]
                    }
                  }
                  frame True {
                    n1018 = for {
                      shift-right: [w3160] -> w3157
                      shift-left: w3158 -> [w3161]
                      tunnel: string[] ["READ NAVX", "RESET FLAGS", "RESET ENCODERS", "", "", ""] -> [w3159] mode=indexing
                      n1019 = Enqueue Element(queue=w3161, element=w3159) -> (queue out=w3160:refnum<queue>)  [unwired: 2 in, 2 out]
                    }
                  }
                }
                n1020 = Select(t=State_Type_Definitions,_for_0.26g_versions_and_later_3."Task A11: ARM DROP HEIGHT" ("Enum"), s=w3137, f=State_Type_Definitions,_for_0.26g_versions_and_later_3."Task 9I: ROTATE 90 CW" ("Enum")) -> (s? t:f=w3142:T18)
                n1021 = Select(t=w3142, s=w3140, f=State_Type_Definitions,_for_0.26g_versions_and_later_3."Task 9H: SCAN BOX 2" ("Enum")) -> (s? t:f=w3148:T18)
              }
              frame "Exit" {
                n1022 = for {
                  shift-right: [w3168] -> w3165
                  shift-left: w3164 -> [w3169]
                  tunnel: string[] ["STOP", "RESET ENCODERS", "RESET YAW", "ARDUINO MODE 0"] -> [w3167] mode=indexing
                  n1023 = Enqueue Element(queue=w3169, element=w3167) -> (queue out=w3168:refnum<queue>)  [unwired: 2 in, 2 out]
                }
              }
            }
          }
          frame "Task 9I: ROTATE 90 CW" {
            # "High battery voltage: -36\nMid voltage: -38 \nLow voltage: -40"
            # ">> Item Selection Bias >>"
            n1024 = Less Or Equal?(x=w3172, y=-38.0) -> (x <= y?=w3170:bool)
            n1025 = Dequeue Element(queue=w3173, timeout in ms (-1)=w3174, error in (no error)=w3175) -> (element=w3181:T10)  [unwired: 3 out]
            n1026 = case shown="\"Start Task 1\", Default" w3181 {
              tunnel: w3170 -> [w3187 _]
              tunnel: [w3194 State_Type_Definitions,_for_0.26g_versions_and_later_3."True Stop" ("Enum")] -> w3178
              tunnel: w3176 -> [w3186 _]
              tunnel: w3180 -> [w3193 w3210]
              tunnel: [w3192 w3211] -> w3179
              tunnel: [State_Type_Definitions,_for_0.26g_versions_and_later_3."Idle" ("Enum") State_Type_Definitions,_for_0.26g_versions_and_later_3."Shutdown" ("Enum")] -> w3177
              frame "Start Task 1", Default {
                n1027 = case shown="False" w3187 {
                  tunnel: w3193 -> [w3197 w3204]
                  tunnel: [w3198 w3203] -> w3192
                  frame False {
                    n1028 = for {
                      tunnel: string[] ["R-CW", "READ ENCODERS", "READ IR", "READ NAVX"] ("element") -> [w3199] mode=indexing
                      shift-right: [w3201] -> w3198
                      shift-left: w3197 -> [w3200]
                      n1029 = Enqueue Element(queue=w3200, element=w3199) -> (queue out=w3201:refnum<queue>)  [unwired: 2 in, 2 out]
                    }
                  }
                  frame True {
                    n1030 = for {
                      shift-right: [w3206] -> w3203
                      shift-left: w3204 -> [w3207]
                      tunnel: string[] ["STOP", "RESET ENCODERS", "RESET YAW", "RESET FLAGS", "READ IR", ""] -> [w3205] mode=indexing
                      n1031 = Enqueue Element(queue=w3207, element=w3205) -> (queue out=w3206:refnum<queue>)  [unwired: 2 in, 2 out]
                    }
                  }
                }
                n1032 = Or(x=w3187, y=w3186) -> (x .or. y?=w3185:bool)
                n1033 = Select(t=State_Type_Definitions,_for_0.26g_versions_and_later_3."True Stop" ("Enum"), s=w3186, f=State_Type_Definitions,_for_0.26g_versions_and_later_3."Task 9J: FORWARD" ("Enum")) -> (s? t:f=w3188:T18)
                n1034 = Select(t=w3188, s=w3185, f=State_Type_Definitions,_for_0.26g_versions_and_later_3."Task 9I: ROTATE 90 CW" ("Enum")) -> (s? t:f=w3194:T18)
              }
              frame "Exit" {
                n1035 = for {
                  shift-right: [w3214] -> w3211
                  shift-left: w3210 -> [w3215]
                  tunnel: string[] ["STOP", "RESET ENCODERS", "RESET YAW", "ARDUINO MODE 0"] -> [w3213] mode=indexing
                  n1036 = Enqueue Element(queue=w3215, element=w3213) -> (queue out=w3214:refnum<queue>)  [unwired: 2 in, 2 out]
                }
              }
            }
          }
          frame "Task 9J: FORWARD" {
            # "Max: 25\nMin: 18"
            # "Tried values: 70, 150"
            # ">>Stops if either table or wall is obstructing >>"
            # ">> Item Selection Bias >>"
            n1037 = Less?(x=w3218, y=150.0) -> (x < y?=w3221:bool)
            n1038 = Greater Than 0?(x=w3218) -> (x > 0?=w3220:bool)
            n1039 = Less Or Equal?(x=w3224, y=25.0) -> (x <= y?=w3222:bool)
            n1040 = Greater Than 0?(x=w3224) -> (x > 0?=w3223:bool)
            n1041 = And(x=w3220, y=w3221) -> ()  [unwired: 1 out]
            n1042 = Dequeue Element(queue=w3230, timeout in ms (-1)=w3231, error in (no error)=w3232) -> (element=w3234:T10)  [unwired: 3 out]
            n1043 = And(x=w3223, y=w3222) -> (x .and. y?=w3216:bool)
            n1044 = Or(x=w3216, y=w3216) -> (x .or. y?=w3217:bool)
            n1045 = case shown="\"Start Task 1\", Default" w3234 {
              tunnel: w3217 -> [w3240 _]
              tunnel: [w3247 State_Type_Definitions,_for_0.26g_versions_and_later_3."True Stop" ("Enum")] -> w3228
              tunnel: w3233 -> [w3239 _]
              tunnel: w3229 -> [w3246 w3263]
              tunnel: [w3245 w3264] -> w3227
              tunnel: [State_Type_Definitions,_for_0.26g_versions_and_later_3."Idle" ("Enum") State_Type_Definitions,_for_0.26g_versions_and_later_3."Shutdown" ("Enum")] -> w3226
              frame "Start Task 1", Default {
                n1046 = case shown="True" w3240 {
                  tunnel: w3246 -> [w3250 w3257]
                  tunnel: [w3251 w3256] -> w3245
                  frame False {
                    n1047 = for {
                      tunnel: string[] ["READ IR", "READ NAVX", "FORWARD"] ("element") -> [w3252] mode=indexing
                      shift-right: [w3254] -> w3251
                      shift-left: w3250 -> [w3253]
                      n1048 = Enqueue Element(queue=w3253, element=w3252) -> (queue out=w3254:refnum<queue>)  [unwired: 2 in, 2 out]
                    }
                  }
                  frame True {
                    n1049 = for {
                      shift-right: [w3259] -> w3256
                      shift-left: w3257 -> [w3260]
                      tunnel: string[] ["STOP", "RESET ENCODERS", "RESET YAW", "RESET FLAGS", "READ IR", ""] -> [w3258] mode=indexing
                      n1050 = Enqueue Element(queue=w3260, element=w3258) -> (queue out=w3259:refnum<queue>)  [unwired: 2 in, 2 out]
                    }
                  }
                }
                n1051 = Or(x=w3240, y=w3239) -> (x .or. y?=w3238:bool)
                n1052 = Select(t=State_Type_Definitions,_for_0.26g_versions_and_later_3."True Stop" ("Enum"), s=w3239, f=State_Type_Definitions,_for_0.26g_versions_and_later_3."Task 9J2: ANGLE CORRECTION" ("Enum")) -> (s? t:f=w3241:T18)
                n1053 = Select(t=w3241, s=w3238, f=State_Type_Definitions,_for_0.26g_versions_and_later_3."Task 9J: FORWARD" ("Enum")) -> (s? t:f=w3247:T18)
              }
              frame "Exit" {
                n1054 = for {
                  shift-right: [w3267] -> w3264
                  shift-left: w3263 -> [w3268]
                  tunnel: string[] ["STOP", "RESET ENCODERS", "RESET YAW", "ARDUINO MODE 0"] -> [w3266] mode=indexing
                  n1055 = Enqueue Element(queue=w3268, element=w3266) -> (queue out=w3267:refnum<queue>)  [unwired: 2 in, 2 out]
                }
              }
            }
          }
          frame "Task 9J2: ANGLE CORRECTION" {
            # "Ngee Ann Values: Min 100, Max 110"
            # ">>> Motor control cluster >>>"
            # ">>> yStepper command>>>"
            n1056 = Dequeue Element(queue=w3282, timeout in ms (-1)=w3281, error in (no error)=w3280) -> (element=w3284:T10)  [unwired: 3 out]
            n1057 = In Range and Coerce(upper limit=110.0, x=w3274, lower limit=100.0) -> (In Range?=w3269:bool)  [unwired: 1 out]
            n1058 = case shown="\"Start Task 1\", Default" w3284 {
              tunnel: w3275 -> [w3287 _]
              tunnel: [w3295 State_Type_Definitions,_for_0.26g_versions_and_later_3."True Stop" ("Enum")] -> w3277
              tunnel: w3283 -> [w3293 w3311]
              tunnel: [w3292 w3310] -> w3276
              tunnel: [State_Type_Definitions,_for_0.26g_versions_and_later_3."Idle" ("Enum") State_Type_Definitions,_for_0.26g_versions_and_later_3."Shutdown" ("Enum")] -> w3278
              tunnel: w3269 -> [w3285 _]
              frame "Start Task 1", Default {
                n1059 = Or(x=w3285, y=w3287) -> (x .or. y?=w3286:bool)
                n1060 = case shown="False" w3285 {
                  tunnel: w3293 -> [w3298 w3304]
                  tunnel: [w3297 w3302] -> w3292
                  frame False {
                    n1061 = for {
                      shift-right: [w3300] -> w3297
                      shift-left: w3298 -> [w3301]
                      tunnel: string[] ["READ NAVX", "R-ACW SLOW", ""] ("element") -> [w3299] mode=indexing
                      n1062 = Enqueue Element(queue=w3301, element=w3299) -> (queue out=w3300:refnum<queue>)  [unwired: 2 in, 2 out]
                    }
                  }
                  frame True {
                    n1063 = for {
                      shift-right: [w3306] -> w3302
                      shift-left: w3304 -> [w3307]
                      tunnel: string[] ["STOP", "RESET ENCODERS", "RESET YAW", "", ""] -> [w3305] mode=indexing
                      n1064 = Enqueue Element(queue=w3307, element=w3305) -> (queue out=w3306:refnum<queue>)  [unwired: 2 in, 2 out]
                    }
                  }
                }
                n1065 = Select(t=State_Type_Definitions,_for_0.26g_versions_and_later_3."True Stop" ("Enum"), s=w3287, f=State_Type_Definitions,_for_0.26g_versions_and_later_3."Task 9K: RAM WALL") -> (s? t:f=w3289:T18)
                n1066 = Select(t=w3289, s=w3286, f=State_Type_Definitions,_for_0.26g_versions_and_later_3."Task 9J2: ANGLE CORRECTION" ("Enum")) -> (s? t:f=w3295:T18)
              }
              frame "Exit" {
                n1067 = for {
                  shift-right: [w3314] -> w3310
                  shift-left: w3311 -> [w3315]
                  tunnel: string[] ["STOP", "RESET ENCODERS", "RESET YAW", ""] -> [w3313] mode=indexing
                  n1068 = Enqueue Element(queue=w3315, element=w3313) -> (queue out=w3314:refnum<queue>)  [unwired: 2 in, 2 out]
                }
              }
            }
          }
          frame "Task 9K: RAM WALL" {
            # "High battery voltage: 15"
            # ">> Item Selection Bias >>"
            # ">>Stops if either table or wall is obstructing >>"
            n1069 = Less?(x=w3316, y=15.0) -> (x < y?=w3326:bool)
            n1070 = Dequeue Element(queue=w3324, timeout in ms (-1)=w3323, error in (no error)=w3322) -> (element=w3328:T10)  [unwired: 3 out]
            n1071 = case shown="\"Start Task 1\", Default" w3328 {
              tunnel: w3326 -> [w3333 _]
              tunnel: [w3340 State_Type_Definitions,_for_0.26g_versions_and_later_3."True Stop" ("Enum")] -> w3318
              tunnel: w3321 -> [w3332 _]
              tunnel: w3325 -> [w3339 w3356]
              tunnel: [w3338 w3357] -> w3319
              tunnel: [State_Type_Definitions,_for_0.26g_versions_and_later_3."Idle" ("Enum") State_Type_Definitions,_for_0.26g_versions_and_later_3."Shutdown" ("Enum")] -> w3317
              frame "Start Task 1", Default {
                n1072 = case shown="True" w3333 {
                  tunnel: w3339 -> [w3343 w3350]
                  tunnel: [w3344 w3349] -> w3338
                  frame False {
                    n1073 = for {
                      tunnel: string[] ["LEFT", "READ NAVX", "READ IR", ""] ("element") -> [w3345] mode=indexing
                      shift-right: [w3347] -> w3344
                      shift-left: w3343 -> [w3346]
                      n1074 = Enqueue Element(queue=w3346, element=w3345) -> (queue out=w3347:refnum<queue>)  [unwired: 2 in, 2 out]
                    }
                  }
                  frame True {
                    n1075 = for {
                      shift-right: [w3352] -> w3349
                      shift-left: w3350 -> [w3353]
                      tunnel: string[] ["STOP", "RESET ENCODERS", "RESET FLAGS", "RESET YAW", "READ IR", ""] -> [w3351] mode=indexing
                      n1076 = Enqueue Element(queue=w3353, element=w3351) -> (queue out=w3352:refnum<queue>)  [unwired: 2 in, 2 out]
                    }
                  }
                }
                n1077 = Or(x=w3333, y=w3332) -> (x .or. y?=w3331:bool)
                n1078 = Select(t=State_Type_Definitions,_for_0.26g_versions_and_later_3."True Stop" ("Enum"), s=w3332, f=State_Type_Definitions,_for_0.26g_versions_and_later_3."Task 9L: MOVE RIGHT" ("Enum")) -> (s? t:f=w3334:T18)
                n1079 = Select(t=w3334, s=w3331, f=State_Type_Definitions,_for_0.26g_versions_and_later_3."Task 9K: RAM WALL" ("Enum")) -> (s? t:f=w3340:T18)
              }
              frame "Exit" {
                n1080 = for {
                  shift-right: [w3360] -> w3357
                  shift-left: w3356 -> [w3361]
                  tunnel: string[] ["STOP", "RESET ENCODERS", "RESET YAW", "ARDUINO MODE 0"] -> [w3359] mode=indexing
                  n1081 = Enqueue Element(queue=w3361, element=w3359) -> (queue out=w3360:refnum<queue>)  [unwired: 2 in, 2 out]
                }
              }
            }
          }
          frame "Task 9L: MOVE RIGHT" {
            # "High battery voltage: 15"
            # ">>> Motor control cluster >>>"
            # ">>> yStepper command>>>"
            # ">> Item Selection Bias >>"
            n1082 = Dequeue Element(queue=w3369, timeout in ms (-1)=w3368, error in (no error)=w3367) -> (element=w3371:T10)  [unwired: 3 out]
            n1083 = case shown="\"Start Task 1\", Default" w3371 {
              tunnel: w3362 -> [w3377 _]
              tunnel: [w3384 State_Type_Definitions,_for_0.26g_versions_and_later_3."True Stop" ("Enum")] -> w3365
              tunnel: w3366 -> [w3376 _]
              tunnel: w3370 -> [w3383 w3400]
              tunnel: [w3382 w3401] -> w3363
              tunnel: [State_Type_Definitions,_for_0.26g_versions_and_later_3."Idle" ("Enum") State_Type_Definitions,_for_0.26g_versions_and_later_3."Shutdown" ("Enum")] -> w3364
              frame "Start Task 1", Default {
                n1084 = case shown="True" w3377 {
                  tunnel: w3383 -> [w3387 w3394]
                  tunnel: [w3388 w3393] -> w3382
                  frame False {
                    n1085 = for {
                      tunnel: string[] ["RIGHT", "READ NAVX", "READ LINE SENSOR", ""] ("element") -> [w3389] mode=indexing
                      shift-right: [w3391] -> w3388
                      shift-left: w3387 -> [w3390]
                      n1086 = Enqueue Element(queue=w3390, element=w3389) -> (queue out=w3391:refnum<queue>)  [unwired: 2 in, 2 out]
                    }
                  }
                  frame True {
                    n1087 = for {
                      shift-right: [w3396] -> w3393
                      shift-left: w3394 -> [w3397]
                      tunnel: string[] ["STOP", "RESET ENCODERS", "RESET FLAGS", "RESET YAW", "BOX COLOUR", ""] -> [w3395] mode=indexing
                      n1088 = Enqueue Element(queue=w3397, element=w3395) -> (queue out=w3396:refnum<queue>)  [unwired: 2 in, 2 out]
                    }
                  }
                }
                n1089 = Or(x=w3377, y=w3376) -> (x .or. y?=w3375:bool)
                n1090 = Select(t=State_Type_Definitions,_for_0.26g_versions_and_later_3."True Stop" ("Enum"), s=w3376, f=State_Type_Definitions,_for_0.26g_versions_and_later_3."Task 9M: SCAN BOX 3" ("Enum")) -> (s? t:f=w3378:T18)
                n1091 = Select(t=w3378, s=w3375, f=State_Type_Definitions,_for_0.26g_versions_and_later_3."Task 9L: MOVE RIGHT" ("Enum")) -> (s? t:f=w3384:T18)
              }
              frame "Exit" {
                n1092 = for {
                  shift-right: [w3404] -> w3401
                  shift-left: w3400 -> [w3405]
                  tunnel: string[] ["STOP", "RESET ENCODERS", "RESET YAW", "ARDUINO MODE 0"] -> [w3403] mode=indexing
                  n1093 = Enqueue Element(queue=w3405, element=w3403) -> (queue out=w3404:refnum<queue>)  [unwired: 2 in, 2 out]
                }
              }
            }
          }
          frame "Task 9M: SCAN BOX 3" {
            # ">>> Motor control cluster >>>"
            # ">>> yStepper command>>>"
            # ">> Item Selection Bias >>"
            n1094 = Dequeue Element(queue=w3415, timeout in ms (-1)=w3414, error in (no error)=w3413) -> (element=w3419:T10)  [unwired: 3 out]
            n1095 = call "Box Colour FGV.vi"("Init/R/W State"=Box_Colour_FGV_States."Read") -> ("Colour to detect (output)"=w3409:T2)  [unwired: 9 in, 1 out]
            n1096 = Equal?(x=w3408, y=w3409) -> (x = y?=w3407:bool)
            n1097 = case shown="\"Start Task 1\", Default" w3419 {
              tunnel: w3406 -> [w3427 _]
              tunnel: [w3434 State_Type_Definitions,_for_0.26g_versions_and_later_3."True Stop" ("Enum")] -> w3417
              tunnel: w3412 -> [w3423 _]
              tunnel: w3416 -> [w3433 w3450]
              tunnel: [w3432 w3451] -> w3411
              tunnel: [State_Type_Definitions,_for_0.26g_versions_and_later_3."Idle" ("Enum") State_Type_Definitions,_for_0.26g_versions_and_later_3."Shutdown" ("Enum")] -> w3418
              tunnel: w3407 -> [w3425 _]
              frame "Start Task 1", Default {
                n1098 = case shown="True" w3427 {
                  tunnel: w3433 -> [w3437 w3444]
                  tunnel: [w3438 w3443] -> w3432
                  frame False {
                    n1099 = for {
                      tunnel: string[] ["", "", "", ""] ("element") -> [w3439] mode=indexing
                      shift-right: [w3441] -> w3438
                      shift-left: w3437 -> [w3440]
                      n1100 = Enqueue Element(queue=w3440, element=w3439) -> (queue out=w3441:refnum<queue>)  [unwired: 2 in, 2 out]
                    }
                  }
                  frame True {
                    n1101 = for {
                      shift-right: [w3446] -> w3443
                      shift-left: w3444 -> [w3447]
                      tunnel: string[] ["STOP", "RESET ENCODERS", "RESET FLAGS", "RESET YAW", "", ""] -> [w3445] mode=indexing
                      n1102 = Enqueue Element(queue=w3447, element=w3445) -> (queue out=w3446:refnum<queue>)  [unwired: 2 in, 2 out]
                    }
                  }
                }
                n1103 = Or(x=w3427, y=w3423) -> (x .or. y?=w3426:bool)
                n1104 = Or(x=w3425, y=w3423) -> (x .or. y?=w3424:bool)
                n1105 = Select(t=State_Type_Definitions,_for_0.26g_versions_and_later_3."True Stop" ("Enum"), s=w3424, f=State_Type_Definitions,_for_0.26g_versions_and_later_3."Task 9N: MOVE RIGHT" ("Enum")) -> (s? t:f=w3428:T18)
                n1106 = Select(t=w3428, s=w3426, f=State_Type_Definitions,_for_0.26g_versions_and_later_3."Task 9M: SCAN BOX 3" ("Enum")) -> (s? t:f=w3434:T18)
              }
              frame "Exit" {
                n1107 = for {
                  shift-right: [w3454] -> w3451
                  shift-left: w3450 -> [w3455]
                  tunnel: string[] ["STOP", "RESET ENCODERS", "RESET YAW", "ARDUINO MODE 0"] -> [w3453] mode=indexing
                  n1108 = Enqueue Element(queue=w3455, element=w3453) -> (queue out=w3454:refnum<queue>)  [unwired: 2 in, 2 out]
                }
              }
            }
          }
          frame "Task 9N: MOVE RIGHT" {
            # ">> Item Selection Bias >>"
            n1109 = Dequeue Element(queue=w3460, timeout in ms (-1)=w3459, error in (no error)=w3458) -> (element=w3465:T10)  [unwired: 3 out]
            n1110 = case shown="\"Start Task 1\", Default" w3465 {
              tunnel: w3456 -> [w3471 _]
              tunnel: [w3478 State_Type_Definitions,_for_0.26g_versions_and_later_3."True Stop" ("Enum")] -> w3463
              tunnel: w3457 -> [w3470 _]
              tunnel: w3461 -> [w3477 w3494]
              tunnel: [w3476 w3495] -> w3462
              tunnel: [State_Type_Definitions,_for_0.26g_versions_and_later_3."Idle" ("Enum") State_Type_Definitions,_for_0.26g_versions_and_later_3."Shutdown" ("Enum")] -> w3464
              frame "Start Task 1", Default {
                n1111 = case shown="True" w3471 {
                  tunnel: w3477 -> [w3481 w3488]
                  tunnel: [w3482 w3487] -> w3476
                  frame False {
                    n1112 = for {
                      tunnel: string[] ["READ LINE SENSOR", "READ NAVX", "RIGHT", "READ ENCODERS"] ("element") -> [w3483] mode=indexing
                      shift-right: [w3485] -> w3482
                      shift-left: w3481 -> [w3484]
                      n1113 = Enqueue Element(queue=w3484, element=w3483) -> (queue out=w3485:refnum<queue>)  [unwired: 2 in, 2 out]
                    }
                  }
                  frame True {
                    n1114 = for {
                      shift-right: [w3490] -> w3487
                      shift-left: w3488 -> [w3491]
                      tunnel: string[] ["STOP", "RESET ENCODERS", "RESET YAW", "RESET FLAGS", "BOX COLOUR", ""] -> [w3489] mode=indexing
                      n1115 = Enqueue Element(queue=w3491, element=w3489) -> (queue out=w3490:refnum<queue>)  [unwired: 2 in, 2 out]
                    }
                  }
                }
                n1116 = Or(x=w3471, y=w3470) -> (x .or. y?=w3469:bool)
                n1117 = Select(t=State_Type_Definitions,_for_0.26g_versions_and_later_3."True Stop" ("Enum"), s=w3470, f=State_Type_Definitions,_for_0.26g_versions_and_later_3."Task 9O: SCAN BOX 4" ("Enum")) -> (s? t:f=w3472:T18)
                n1118 = Select(t=w3472, s=w3469, f=State_Type_Definitions,_for_0.26g_versions_and_later_3."Task 9N: MOVE RIGHT" ("Enum")) -> (s? t:f=w3478:T18)
              }
              frame "Exit" {
                n1119 = for {
                  shift-right: [w3498] -> w3495
                  shift-left: w3494 -> [w3499]
                  tunnel: string[] ["STOP", "RESET ENCODERS", "RESET YAW", "ARDUINO MODE 0"] -> [w3497] mode=indexing
                  n1120 = Enqueue Element(queue=w3499, element=w3497) -> (queue out=w3498:refnum<queue>)  [unwired: 2 in, 2 out]
                }
              }
            }
          }
          frame "Task 9O: SCAN BOX 4" {
            # ">>> Motor control cluster >>>"
            # ">>> yStepper command>>>"
            # ">> Item Selection Bias >>"
            n1121 = Dequeue Element(queue=w3510, timeout in ms (-1)=w3509, error in (no error)=w3508) -> (element=w3514:T10)  [unwired: 3 out]
            n1122 = call "Box Colour FGV.vi"("Init/R/W State"=Box_Colour_FGV_States."Read") -> ("Colour to detect (output)"=w3512:T2)  [unwired: 9 in, 1 out]
            n1123 = Equal?(x=w3502, y=w3512) -> (x = y?=w3511:bool)
            n1124 = case shown="\"Start Task 1\", Default" w3514 {
              tunnel: w3500 -> [w3521 _]
              tunnel: [w3528 State_Type_Definitions,_for_0.26g_versions_and_later_3."True Stop" ("Enum")] -> w3504
              tunnel: w3507 -> [w3517 _]
              tunnel: w3501 -> [w3527 w3544]
              tunnel: [w3526 w3545] -> w3505
              tunnel: [State_Type_Definitions,_for_0.26g_versions_and_later_3."Idle" ("Enum") State_Type_Definitions,_for_0.26g_versions_and_later_3."Shutdown" ("Enum")] -> w3503
              tunnel: w3511 -> [w3519 _]
              frame "Start Task 1", Default {
                n1125 = case shown="True" w3521 {
                  tunnel: w3527 -> [w3531 w3538]
                  tunnel: [w3532 w3537] -> w3526
                  frame False {
                    n1126 = for {
                      tunnel: string[] ["", "", "", ""] ("element") -> [w3533] mode=indexing
                      shift-right: [w3535] -> w3532
                      shift-left: w3531 -> [w3534]
                      n1127 = Enqueue Element(queue=w3534, element=w3533) -> (queue out=w3535:refnum<queue>)  [unwired: 2 in, 2 out]
                    }
                  }
                  frame True {
                    n1128 = for {
                      shift-right: [w3540] -> w3537
                      shift-left: w3538 -> [w3541]
                      tunnel: string[] ["STOP", "RESET ENCODERS", "RESET FLAGS", "RESET YAW", "", ""] -> [w3539] mode=indexing
                      n1129 = Enqueue Element(queue=w3541, element=w3539) -> (queue out=w3540:refnum<queue>)  [unwired: 2 in, 2 out]
                    }
                  }
                }
                n1130 = Or(x=w3521, y=w3517) -> (x .or. y?=w3520:bool)
                n1131 = Or(x=w3519, y=w3517) -> (x .or. y?=w3518:bool)
                n1132 = Select(t=State_Type_Definitions,_for_0.26g_versions_and_later_3."True Stop" ("Enum"), s=w3518, f=State_Type_Definitions,_for_0.26g_versions_and_later_3."True Stop" ("Enum")) -> (s? t:f=w3522:T18)
                n1133 = Select(t=w3522, s=w3520, f=State_Type_Definitions,_for_0.26g_versions_and_later_3."Task 9O: SCAN BOX 4" ("Enum")) -> (s? t:f=w3528:T18)
              }
              frame "Exit" {
                n1134 = for {
                  shift-right: [w3548] -> w3545
                  shift-left: w3544 -> [w3549]
                  tunnel: string[] ["STOP", "RESET ENCODERS", "RESET YAW", "ARDUINO MODE 0"] -> [w3547] mode=indexing
                  n1135 = Enqueue Element(queue=w3549, element=w3547) -> (queue out=w3548:refnum<queue>)  [unwired: 2 in, 2 out]
                }
              }
            }
          }
          frame "Task A1: RAISE ARM" {
            # ">>> Motor control cluster >>>"
            # ">> Stepper height reeached >>"
            # ">>> yStepper command>>>"
            # ">> Manual override >>"
            n1136 = Dequeue Element(queue=w3562, timeout in ms (-1)=w3557, error in (no error)=w3561) -> (element=w3564:T10)  [unwired: 3 out]
            n1137 = Equal?(x=w3559, y=u8 40) -> (x = y?=w3550:bool)
            n1138 = case shown="\"Start Task 1\", Default" w3564 {
              tunnel: [w3575 State_Type_Definitions,_for_0.26g_versions_and_later_3."True Stop" ("Enum")] -> w3555
              tunnel: [w3573 w3590] -> w3554
              tunnel: w3558 -> [w3572 _]
              tunnel: w3560 -> [w3566 _]
              tunnel: [State_Type_Definitions,_for_0.26g_versions_and_later_3."Idle" ("Enum") State_Type_Definitions,_for_0.26g_versions_and_later_3."Shutdown" ("Enum")] -> w3556
              tunnel: w3550 -> [w3565 _]
              frame "Start Task 1", Default {
                # ">> WIill proceed to part ii if not manual override >>"
                # ">>If ENABLE or Trigger is set to true>>"
                n1139 = Or(x=w3565, y=w3566) -> (x .or. y?=w3567:bool)
                n1140 = case shown="False" w3565 {
                  tunnel: [w3578 w3584] -> w3573
                  tunnel: w3572 -> [w3577 w3583]
                  frame False {
                    n1141 = for {
                      shift-right: [w3580] -> w3578
                      shift-left: w3577 -> [w3581]
                      tunnel: string[] ["Z STEPPER BOX HEIGHT", "READ STEPPER VALUES"] ("element") -> [w3579] mode=indexing
                      n1142 = Enqueue Element(queue=w3581, element=w3579) -> (queue out=w3580:refnum<queue>)  [unwired: 2 in, 2 out]
                    }
                  }
                  frame True {
                    n1143 = for {
                      shift-right: [w3586] -> w3584
                      shift-left: w3583 -> [w3587]
                      tunnel: string[] ["READ NAVX", "RESET FLAGS", "RESET YAW", "", "", ""] -> [w3585] mode=indexing
                      n1144 = Enqueue Element(queue=w3587, element=w3585) -> (queue out=w3586:refnum<queue>)  [unwired: 2 in, 2 out]
                    }
                  }
                }
                n1145 = Select(t=State_Type_Definitions,_for_0.26g_versions_and_later_3."True Stop" ("Enum"), s=w3566, f=State_Type_Definitions,_for_0.26g_versions_and_later_3."Task A2: ROTATE TO ANGLE" ("Enum")) -> (s? t:f=w3569:T18)
                n1146 = Select(t=w3569, s=w3567, f=State_Type_Definitions,_for_0.26g_versions_and_later_3."Task A1: RAISE ARM" ("Enum")) -> (s? t:f=w3575:T18)
              }
              frame "Exit" {
                n1147 = for {
                  shift-right: [w3593] -> w3590
                  shift-left: _ -> [w3594]
                  tunnel: string[] ["STOP", "RESET ENCODERS", "RESET YAW", ""] -> [w3592] mode=indexing
                  n1148 = Enqueue Element(queue=w3594, element=w3592) -> (queue out=w3593:refnum<queue>)  [unwired: 2 in, 2 out]
                }
              }
            }
          }
          frame "Task A2: ROTATE TO ANGLE" {
            # ">>> Motor control cluster >>>"
            # ">>> yStepper command>>>"
            n1149 = Dequeue Element(queue=w3608, timeout in ms (-1)=w3607, error in (no error)=w3606) -> (element=w3610:T10)  [unwired: 3 out]
            n1150 = In Range and Coerce(upper limit=65.0, x=w3600, lower limit=58.0) -> (In Range?=w3595:bool)  [unwired: 1 out]
            n1151 = case shown="\"Start Task 1\", Default" w3610 {
              tunnel: w3601 -> [w3613 _]
              tunnel: [w3621 State_Type_Definitions,_for_0.26g_versions_and_later_3."True Stop" ("Enum")] -> w3603
              tunnel: w3609 -> [w3619 w3637]
              tunnel: [w3618 w3636] -> w3602
              tunnel: [State_Type_Definitions,_for_0.26g_versions_and_later_3."Idle" ("Enum") State_Type_Definitions,_for_0.26g_versions_and_later_3."Shutdown" ("Enum")] -> w3604
              tunnel: w3595 -> [w3611 _]
              frame "Start Task 1", Default {
                n1152 = Or(x=w3611, y=w3613) -> (x .or. y?=w3612:bool)
                n1153 = case shown="True" w3611 {
                  tunnel: w3619 -> [w3624 w3630]
                  tunnel: [w3623 w3628] -> w3618
                  frame False {
                    n1154 = for {
                      shift-right: [w3626] -> w3623
                      shift-left: w3624 -> [w3627]
                      tunnel: string[] ["READ NAVX", "R-CW", ""] ("element") -> [w3625] mode=indexing
                      n1155 = Enqueue Element(queue=w3627, element=w3625) -> (queue out=w3626:refnum<queue>)  [unwired: 2 in, 2 out]
                    }
                  }
                  frame True {
                    n1156 = for {
                      shift-right: [w3632] -> w3628
                      shift-left: w3630 -> [w3633]
                      tunnel: string[] ["STOP", "RESET ENCODERS", "RESET YAW", "RESET FLAGS", ""] -> [w3631] mode=indexing
                      n1157 = Enqueue Element(queue=w3633, element=w3631) -> (queue out=w3632:refnum<queue>)  [unwired: 2 in, 2 out]
                    }
                  }
                }
                n1158 = Select(t=State_Type_Definitions,_for_0.26g_versions_and_later_3."True Stop" ("Enum"), s=w3613, f=State_Type_Definitions,_for_0.26g_versions_and_later_3."Task A3: MOVE TO BL BOX") -> (s? t:f=w3615:T18)
                n1159 = Select(t=w3615, s=w3612, f=State_Type_Definitions,_for_0.26g_versions_and_later_3."Task A2: ROTATE TO ANGLE" ("Enum")) -> (s? t:f=w3621:T18)
              }
              frame "Exit" {
                n1160 = for {
                  shift-right: [w3640] -> w3636
                  shift-left: w3637 -> [w3641]
                  tunnel: string[] ["STOP", "RESET ENCODERS", "RESET YAW", ""] -> [w3639] mode=indexing
                  n1161 = Enqueue Element(queue=w3641, element=w3639) -> (queue out=w3640:refnum<queue>)  [unwired: 2 in, 2 out]
                }
              }
            }
          }
          frame "Task A3: MOVE TO BL BOX" {
            # ">>> Motor control cluster >>>"
            # ">>Line Detected>>"
            # ">>Action Queue>>"
            # ">>> yStepper command>>>"
            n1162 = Dequeue Element(queue=w3653, timeout in ms (-1)=w3652, error in (no error)=w3651) -> (element=w3654:T10)  [unwired: 3 out]
            n1163 = case shown="\"Start Task 1\", Default" w3654 {
              tunnel: w3649 -> [w3655 _]
              tunnel: [w3665 State_Type_Definitions,_for_0.26g_versions_and_later_3."True Stop" ("Enum")] -> w3646
              tunnel: w3650 -> [w3663 w3681]
              tunnel: [w3662 w3680] -> w3645
              tunnel: [State_Type_Definitions,_for_0.26g_versions_and_later_3."Idle" ("Enum") State_Type_Definitions,_for_0.26g_versions_and_later_3."Shutdown" ("Enum")] -> w3648
              tunnel: w3642 -> [w3656 _]
              frame "Start Task 1", Default {
                n1164 = Or(x=w3655, y=w3656) -> (x .or. y?=w3657:bool)
                n1165 = case shown="True" w3656 {
                  tunnel: w3663 -> [w3668 w3674]
                  tunnel: [w3667 w3672] -> w3662
                  frame False {
                    n1166 = for {
                      shift-right: [w3670] -> w3667
                      shift-left: w3668 -> [w3671]
                      tunnel: string[] ["READ IR", "READ LINE SENSOR", "FORWARD", "READ NAVX"] ("element") -> [w3669] mode=indexing
                      n1167 = Enqueue Element(queue=w3671, element=w3669) -> (queue out=w3670:refnum<queue>)  [unwired: 2 in, 2 out]
                    }
                  }
                  frame True {
                    n1168 = for {
                      shift-right: [w3676] -> w3672
                      shift-left: w3674 -> [w3677]
                      tunnel: string[] ["STOP", "RESET ENCODERS", "RESET YAW", "RESET FLAGS", "ARDUINO - ULTRASONIC"] -> [w3675] mode=indexing
                      n1169 = Enqueue Element(queue=w3677, element=w3675) -> (queue out=w3676:refnum<queue>)  [unwired: 2 in, 2 out]
                    }
                  }
                }
                n1170 = Select(t=State_Type_Definitions,_for_0.26g_versions_and_later_3."True Stop" ("Enum"), s=w3655, f=State_Type_Definitions,_for_0.26g_versions_and_later_3."Task A4: MOVE FORWARD") -> (s? t:f=w3659:T18)
                n1171 = Select(t=w3659, s=w3657, f=State_Type_Definitions,_for_0.26g_versions_and_later_3."Task A3: MOVE TO BL BOX" ("Enum")) -> (s? t:f=w3665:T18)
              }
              frame "Exit" {
                n1172 = for {
                  shift-right: [w3684] -> w3680
                  shift-left: w3681 -> [w3685]
                  tunnel: string[] ["STOP", "RESET ENCODERS", "RESET YAW", ""] -> [w3683] mode=indexing
                  n1173 = Enqueue Element(queue=w3685, element=w3683) -> (queue out=w3684:refnum<queue>)  [unwired: 2 in, 2 out]
                }
              }
            }
          }
          frame "Task A4: MOVE FORWARD" {
            (unwired) u8 50 ("y")
            # "Use 20 low voltage\nUse 25 high voltage"
            # ">> Item Selection Bias >>"
            # ">> Manual override >>"
            # ">>> Motor control cluster >>>"
            # ">>Action Queue>>"
            # ">>> yStepper command>>>"
            n1174 = Dequeue Element(queue=w3699, timeout in ms (-1)=w3698, error in (no error)=w3697) -> (element=w3700:T10)  [unwired: 3 out]
            n1175 = Greater Or Equal?(x=w3688, y=80.0) -> (x >= y?=w3686:bool)
            n1176 = case shown="\"Start Task 1\", Default" w3700 {
              tunnel: w3695 -> [w3701 _]
              tunnel: [w3711 State_Type_Definitions,_for_0.26g_versions_and_later_3."True Stop" ("Enum")] -> w3692
              tunnel: w3696 -> [w3709 w3727]
              tunnel: [w3708 w3726] -> w3691
              tunnel: [State_Type_Definitions,_for_0.26g_versions_and_later_3."Idle" ("Enum") State_Type_Definitions,_for_0.26g_versions_and_later_3."Shutdown" ("Enum")] -> w3694
              tunnel: w3686 -> [w3702 _]
              frame "Start Task 1", Default {
                n1177 = Or(x=w3701, y=w3702) -> (x .or. y?=w3703:bool)
                n1178 = case shown="False" w3701 {
                  tunnel: w3709 -> [w3714 w3720]
                  tunnel: [w3713 w3718] -> w3708
                  frame False {
                    n1179 = for {
                      shift-right: [w3716] -> w3713
                      shift-left: w3714 -> [w3717]
                      tunnel: string[] ["READ IR", "FORWARD", "READ ENCODERS", "READ NAVX"] ("element") -> [w3715] mode=indexing
                      n1180 = Enqueue Element(queue=w3717, element=w3715) -> (queue out=w3716:refnum<queue>)  [unwired: 2 in, 2 out]
                    }
                  }
                  frame True {
                    n1181 = for {
                      shift-right: [w3722] -> w3718
                      shift-left: w3720 -> [w3723]
                      tunnel: string[] ["STOP", "RESET ENCODERS", "RESET YAW", "RESET FLAGS", "SET TIMER 1"] -> [w3721] mode=indexing
                      n1182 = Enqueue Element(queue=w3723, element=w3721) -> (queue out=w3722:refnum<queue>)  [unwired: 2 in, 2 out]
                    }
                  }
                }
                n1183 = Select(t=State_Type_Definitions,_for_0.26g_versions_and_later_3."True Stop" ("Enum"), s=w3701, f=State_Type_Definitions,_for_0.26g_versions_and_later_3."Task A5: Stop") -> (s? t:f=w3705:T18)
                n1184 = Select(t=w3705, s=w3703, f=State_Type_Definitions,_for_0.26g_versions_and_later_3."Task A4: MOVE FORWARD" ("Enum")) -> (s? t:f=w3711:T18)
              }
              frame "Exit" {
                n1185 = for {
                  shift-right: [w3730] -> w3726
                  shift-left: w3727 -> [w3731]
                  tunnel: string[] ["STOP", "RESET ENCODERS", "RESET YAW", ""] -> [w3729] mode=indexing
                  n1186 = Enqueue Element(queue=w3731, element=w3729) -> (queue out=w3730:refnum<queue>)  [unwired: 2 in, 2 out]
                }
              }
            }
          }
          frame "Task A5: Stop" {
            # ">>> Motor control cluster >>>"
            # ">>> yStepper command>>>"
            # "High battery voltage: -36\nMid voltage: -38 \nLow voltage: -40"
            # ">> Item Selection Bias >>"
            n1187 = Dequeue Element(queue=w3733, timeout in ms (-1)=w3734, error in (no error)=w3735) -> (element=w3741:T10)  [unwired: 3 out]
            n1188 = case shown="\"Start Task 1\", Default" w3741 {
              tunnel: [w3754 State_Type_Definitions,_for_0.26g_versions_and_later_3."True Stop" ("Enum")] -> w3738
              tunnel: w3736 -> [w3747 _]
              tunnel: w3740 -> [w3753 w3770]
              tunnel: [w3752 w3771] -> w3739
              tunnel: [State_Type_Definitions,_for_0.26g_versions_and_later_3."Idle" ("Enum") State_Type_Definitions,_for_0.26g_versions_and_later_3."Shutdown" ("Enum")] -> w3737
              tunnel: w3732 -> [w3746 _]
              frame "Start Task 1", Default {
                n1189 = Or(x=w3746, y=w3747) -> (x .or. y?=w3745:bool)
                n1190 = case shown="True" w3745 {
                  tunnel: w3753 -> [w3757 w3764]
                  tunnel: [w3758 w3763] -> w3752
                  frame False {
                    n1191 = for {
                      tunnel: string[] ["STOP", "RESET ENCODERS", "START TIMER", "READ ENCODERS"] ("element") -> [w3759] mode=indexing
                      shift-right: [w3761] -> w3758
                      shift-left: w3757 -> [w3760]
                      n1192 = Enqueue Element(queue=w3760, element=w3759) -> (queue out=w3761:refnum<queue>)  [unwired: 2 in, 2 out]
                    }
                  }
                  frame True {
                    n1193 = for {
                      shift-right: [w3766] -> w3763
                      shift-left: w3764 -> [w3767]
                      tunnel: string[] ["STOP", "RESET ENCODERS", "RESET YAW", "RESET FLAGS", "READ IR", ""] -> [w3765] mode=indexing
                      n1194 = Enqueue Element(queue=w3767, element=w3765) -> (queue out=w3766:refnum<queue>)  [unwired: 2 in, 2 out]
                    }
                  }
                }
                n1195 = Select(t=State_Type_Definitions,_for_0.26g_versions_and_later_3."True Stop" ("Enum"), s=w3747, f=State_Type_Definitions,_for_0.26g_versions_and_later_3."Task A6: ROTATE CW 90" ("Enum")) -> (s? t:f=w3748:T18)
                n1196 = Select(t=w3748, s=w3745, f=State_Type_Definitions,_for_0.26g_versions_and_later_3."Task A5: Stop" ("Enum")) -> (s? t:f=w3754:T18)
              }
              frame "Exit" {
                n1197 = for {
                  shift-right: [w3774] -> w3771
                  shift-left: w3770 -> [w3775]
                  tunnel: string[] ["STOP", "RESET ENCODERS", "RESET YAW", "ARDUINO MODE 0"] -> [w3773] mode=indexing
                  n1198 = Enqueue Element(queue=w3775, element=w3773) -> (queue out=w3774:refnum<queue>)  [unwired: 2 in, 2 out]
                }
              }
            }
          }
          frame "Task A6: ROTATE CW 90" {
            # ">>> Motor control cluster >>>"
            # ">>> yStepper command>>>"
            # "High battery voltage: -36\nMid voltage: -38 \nLow voltage: -40"
            # ">> Item Selection Bias >>"
            n1199 = Less Or Equal?(x=w3778, y=-38.0) -> (x <= y?=w3776:bool)
            n1200 = Dequeue Element(queue=w3779, timeout in ms (-1)=w3780, error in (no error)=w3781) -> (element=w3787:T10)  [unwired: 3 out]
            n1201 = case shown="\"Start Task 1\", Default" w3787 {
              tunnel: w3776 -> [w3793 _]
              tunnel: [w3800 State_Type_Definitions,_for_0.26g_versions_and_later_3."True Stop" ("Enum")] -> w3784
              tunnel: w3782 -> [w3792 _]
              tunnel: w3786 -> [w3799 w3816]
              tunnel: [w3798 w3817] -> w3785
              tunnel: [State_Type_Definitions,_for_0.26g_versions_and_later_3."Idle" ("Enum") State_Type_Definitions,_for_0.26g_versions_and_later_3."Shutdown" ("Enum")] -> w3783
              frame "Start Task 1", Default {
                n1202 = case shown="True" w3793 {
                  tunnel: w3799 -> [w3803 w3810]
                  tunnel: [w3804 w3809] -> w3798
                  frame False {
                    n1203 = for {
                      tunnel: string[] ["R-CW", "READ ENCODERS", "READ IR", "READ NAVX"] ("element") -> [w3805] mode=indexing
                      shift-right: [w3807] -> w3804
                      shift-left: w3803 -> [w3806]
                      n1204 = Enqueue Element(queue=w3806, element=w3805) -> (queue out=w3807:refnum<queue>)  [unwired: 2 in, 2 out]
                    }
                  }
                  frame True {
                    n1205 = for {
                      shift-right: [w3812] -> w3809
                      shift-left: w3810 -> [w3813]
                      tunnel: string[] ["STOP", "RESET ENCODERS", "RESET YAW", "RESET FLAGS", "READ IR", ""] -> [w3811] mode=indexing
                      n1206 = Enqueue Element(queue=w3813, element=w3811) -> (queue out=w3812:refnum<queue>)  [unwired: 2 in, 2 out]
                    }
                  }
                }
                n1207 = Or(x=w3793, y=w3792) -> (x .or. y?=w3791:bool)
                n1208 = Select(t=State_Type_Definitions,_for_0.26g_versions_and_later_3."True Stop" ("Enum"), s=w3792, f=State_Type_Definitions,_for_0.26g_versions_and_later_3."Task A7: FORWARD" ("Enum")) -> (s? t:f=w3794:T18)
                n1209 = Select(t=w3794, s=w3791, f=State_Type_Definitions,_for_0.26g_versions_and_later_3."Task A6: ROTATE CW 90" ("Enum")) -> (s? t:f=w3800:T18)
              }
              frame "Exit" {
                n1210 = for {
                  shift-right: [w3820] -> w3817
                  shift-left: w3816 -> [w3821]
                  tunnel: string[] ["STOP", "RESET ENCODERS", "RESET YAW", "ARDUINO MODE 0"] -> [w3819] mode=indexing
                  n1211 = Enqueue Element(queue=w3821, element=w3819) -> (queue out=w3820:refnum<queue>)  [unwired: 2 in, 2 out]
                }
              }
            }
          }
          frame "Task A7: FORWARD" {
            # ">>> yStepper command>>>"
            n1212 = Dequeue Element(queue=w3832, timeout in ms (-1)=w3833, error in (no error)=w3834) -> (element=w3836:T10)  [unwired: 3 out]
            n1213 = Greater Or Equal?(x=w3822, y=75.0) -> (x >= y?=w3823:bool)
            n1214 = case shown="\"Start Task 1\", Default" w3836 {
              tunnel: [w3846 State_Type_Definitions,_for_0.26g_versions_and_later_3."True Stop" ("Enum")] -> w3828
              tunnel: w3835 -> [w3839 _]
              tunnel: w3831 -> [w3845 w3862]
              tunnel: [w3844 w3863] -> w3827
              tunnel: [State_Type_Definitions,_for_0.26g_versions_and_later_3."Idle" ("Enum") State_Type_Definitions,_for_0.26g_versions_and_later_3."Shutdown" ("Enum")] -> w3829
              tunnel: w3823 -> [w3837 _]
              frame "Start Task 1", Default {
                n1215 = case shown="True" w3837 {
                  tunnel: w3845 -> [w3849 w3856]
                  tunnel: [w3850 w3855] -> w3844
                  frame False {
                    n1216 = for {
                      tunnel: string[] ["READ ENCODERS", "FORWARD", "READ NAVX"] ("element") -> [w3851] mode=indexing
                      shift-right: [w3853] -> w3850
                      shift-left: w3849 -> [w3852]
                      n1217 = Enqueue Element(queue=w3852, element=w3851) -> (queue out=w3853:refnum<queue>)  [unwired: 2 in, 2 out]
                    }
                  }
                  frame True {
                    n1218 = for {
                      shift-right: [w3858] -> w3855
                      shift-left: w3856 -> [w3859]
                      tunnel: string[] ["STOP", "RESET ENCODERS", "RESET YAW", "RESET FLAGS", "READ LINE SENSOR"] -> [w3857] mode=indexing
                      n1219 = Enqueue Element(queue=w3859, element=w3857) -> (queue out=w3858:refnum<queue>)  [unwired: 2 in, 2 out]
                    }
                  }
                }
                n1220 = Or(x=w3837, y=w3839) -> (x .or. y?=w3838:bool)
                n1221 = Select(t=State_Type_Definitions,_for_0.26g_versions_and_later_3."True Stop" ("Enum"), s=w3839, f=State_Type_Definitions,_for_0.26g_versions_and_later_3."Task A8: LEFT UNTIL LINE" ("Enum")) -> (s? t:f=w3840:T18)
                n1222 = Select(t=w3840, s=w3838, f=State_Type_Definitions,_for_0.26g_versions_and_later_3."Task A7: FORWARD" ("Enum")) -> (s? t:f=w3846:T18)
              }
              frame "Exit" {
                n1223 = for {
                  shift-right: [w3866] -> w3863
                  shift-left: w3862 -> [w3867]
                  tunnel: string[] ["STOP", "RESET ENCODERS", "RESET YAW", "ARDUINO MODE 0"] -> [w3865] mode=indexing
                  n1224 = Enqueue Element(queue=w3867, element=w3865) -> (queue out=w3866:refnum<queue>)  [unwired: 2 in, 2 out]
                }
              }
            }
          }
          frame "Task A8: LEFT UNTIL LINE" {
            # ">>> Motor control cluster >>>"
            # ">>> yStepper command>>>"
            n1225 = Dequeue Element(queue=w3875, timeout in ms (-1)=w3874, error in (no error)=w3873) -> (element=w3880:T10)  [unwired: 3 out]
            n1226 = case shown="\"Start Task 1\", Default" w3880 {
              tunnel: w3868 -> [w3883 _]
              tunnel: [w3890 State_Type_Definitions,_for_0.26g_versions_and_later_3."True Stop" ("Enum")] -> w3879
              tunnel: w3872 -> [w3882 _]
              tunnel: w3876 -> [w3889 w3906]
              tunnel: [w3888 w3907] -> w3878
              tunnel: [State_Type_Definitions,_for_0.26g_versions_and_later_3."Idle" ("Enum") State_Type_Definitions,_for_0.26g_versions_and_later_3."Shutdown" ("Enum")] -> w3877
              frame "Start Task 1", Default {
                n1227 = case shown="False" w3883 {
                  tunnel: w3889 -> [w3893 w3900]
                  tunnel: [w3894 w3899] -> w3888
                  frame False {
                    n1228 = for {
                      tunnel: string[] ["READ LINE SENSOR", "READ NAVX", "LEFT", ""] ("element") -> [w3895] mode=indexing
                      shift-right: [w3897] -> w3894
                      shift-left: w3893 -> [w3896]
                      n1229 = Enqueue Element(queue=w3896, element=w3895) -> (queue out=w3897:refnum<queue>)  [unwired: 2 in, 2 out]
                    }
                  }
                  frame True {
                    n1230 = for {
                      shift-right: [w3902] -> w3899
                      shift-left: w3900 -> [w3903]
                      tunnel: string[] ["RESET ENCODERS", "RESET YAW", "RESET FLAGS", "STOP", ""] -> [w3901] mode=indexing
                      n1231 = Enqueue Element(queue=w3903, element=w3901) -> (queue out=w3902:refnum<queue>)  [unwired: 2 in, 2 out]
                    }
                  }
                }
                n1232 = Or(x=w3883, y=w3882) -> (x .or. y?=w3881:bool)
                n1233 = Select(t=State_Type_Definitions,_for_0.26g_versions_and_later_3."True Stop" ("Enum"), s=w3882, f=State_Type_Definitions,_for_0.26g_versions_and_later_3."Task 8B: MOVE TO BOX" ("Enum")) -> (s? t:f=w3884:T18)
                n1234 = Select(t=w3884, s=w3881, f=State_Type_Definitions,_for_0.26g_versions_and_later_3."Task A8: LEFT UNTIL LINE" ("Enum")) -> (s? t:f=w3890:T18)
              }
              frame "Exit" {
                n1235 = for {
                  shift-right: [w3910] -> w3907
                  shift-left: w3906 -> [w3911]
                  tunnel: string[] ["STOP", "RESET ENCODERS", "RESET YAW", "ARDUINO MODE 0"] -> [w3909] mode=indexing
                  n1236 = Enqueue Element(queue=w3911, element=w3909) -> (queue out=w3910:refnum<queue>)  [unwired: 2 in, 2 out]
                }
              }
            }
          }
          frame "Task A9: REVERSE" {
            # ">>> Motor control cluster >>>"
            # ">>> yStepper command>>>"
            n1237 = Dequeue Element(queue=w3922, timeout in ms (-1)=w3923, error in (no error)=w3924) -> (element=w3926:T10)  [unwired: 3 out]
            n1238 = Less?(x=w3916, y=-100.0) -> (x < y?=w3912:bool)
            n1239 = case shown="\"Start Task 1\", Default" w3926 {
              tunnel: [w3936 State_Type_Definitions,_for_0.26g_versions_and_later_3."True Stop" ("Enum")] -> w3918
              tunnel: w3925 -> [w3929 _]
              tunnel: w3921 -> [w3935 w3952]
              tunnel: [w3934 w3953] -> w3917
              tunnel: [State_Type_Definitions,_for_0.26g_versions_and_later_3."Idle" ("Enum") State_Type_Definitions,_for_0.26g_versions_and_later_3."Shutdown" ("Enum")] -> w3919
              tunnel: w3912 -> [w3927 _]
              frame "Start Task 1", Default {
                n1240 = case shown="True" w3927 {
                  tunnel: w3935 -> [w3939 w3946]
                  tunnel: [w3940 w3945] -> w3934
                  frame False {
                    n1241 = for {
                      tunnel: string[] ["READ ENCODERS", "REVERSE", "READ NAVX"] ("element") -> [w3941] mode=indexing
                      shift-right: [w3943] -> w3940
                      shift-left: w3939 -> [w3942]
                      n1242 = Enqueue Element(queue=w3942, element=w3941) -> (queue out=w3943:refnum<queue>)  [unwired: 2 in, 2 out]
                    }
                  }
                  frame True {
                    n1243 = for {
                      shift-right: [w3948] -> w3945
                      shift-left: w3946 -> [w3949]
                      tunnel: string[] ["STOP", "ARDUINO - ULTRASONIC", "READ ULTRASONIC", "RESET ENCODERS"] -> [w3947] mode=indexing
                      n1244 = Enqueue Element(queue=w3949, element=w3947) -> (queue out=w3948:refnum<queue>)  [unwired: 2 in, 2 out]
                    }
                  }
                }
                n1245 = Or(x=w3927, y=w3929) -> (x .or. y?=w3928:bool)
                n1246 = Select(t=State_Type_Definitions,_for_0.26g_versions_and_later_3."True Stop" ("Enum"), s=w3929, f=State_Type_Definitions,_for_0.26g_versions_and_later_3."Task 9D: MOVE FORWARD" ("Enum")) -> (s? t:f=w3930:T18)
                n1247 = Select(t=w3930, s=w3928, f=State_Type_Definitions,_for_0.26g_versions_and_later_3."Task A9: REVERSE" ("Enum")) -> (s? t:f=w3936:T18)
              }
              frame "Exit" {
                n1248 = for {
                  shift-right: [w3956] -> w3953
                  shift-left: w3952 -> [w3957]
                  tunnel: string[] ["STOP", "RESET ENCODERS", "RESET YAW", "ARDUINO MODE 0"] -> [w3955] mode=indexing
                  n1249 = Enqueue Element(queue=w3957, element=w3955) -> (queue out=w3956:refnum<queue>)  [unwired: 2 in, 2 out]
                }
              }
            }
          }
          frame "Task A10: ROTATE TO ANGLE" {
            # ">>> Motor control cluster >>>"
            # ">>> yStepper command>>>"
            n1250 = Dequeue Element(queue=w3971, timeout in ms (-1)=w3970, error in (no error)=w3969) -> (element=w3973:T10)  [unwired: 3 out]
            n1251 = In Range and Coerce(upper limit=65.0, x=w3963, lower limit=58.0) -> (In Range?=w3958:bool)  [unwired: 1 out]
            n1252 = case shown="\"Start Task 1\", Default" w3973 {
              tunnel: w3964 -> [w3976 _]
              tunnel: [w3984 State_Type_Definitions,_for_0.26g_versions_and_later_3."True Stop" ("Enum")] -> w3966
              tunnel: w3972 -> [w3982 w4000]
              tunnel: [w3981 w3999] -> w3965
              tunnel: [State_Type_Definitions,_for_0.26g_versions_and_later_3."Idle" ("Enum") State_Type_Definitions,_for_0.26g_versions_and_later_3."Shutdown" ("Enum")] -> w3967
              tunnel: w3958 -> [w3974 _]
              frame "Start Task 1", Default {
                n1253 = Or(x=w3974, y=w3976) -> (x .or. y?=w3975:bool)
                n1254 = case shown="False" w3974 {
                  tunnel: w3982 -> [w3987 w3993]
                  tunnel: [w3986 w3991] -> w3981
                  frame False {
                    n1255 = for {
                      shift-right: [w3989] -> w3986
                      shift-left: w3987 -> [w3990]
                      tunnel: string[] ["READ NAVX", "R-ACW", ""] ("element") -> [w3988] mode=indexing
                      n1256 = Enqueue Element(queue=w3990, element=w3988) -> (queue out=w3989:refnum<queue>)  [unwired: 2 in, 2 out]
                    }
                  }
                  frame True {
                    n1257 = for {
                      shift-right: [w3995] -> w3991
                      shift-left: w3993 -> [w3996]
                      tunnel: string[] ["STOP", "RESET ENCODERS", "RESET YAW", "RESET FLAGS", ""] -> [w3994] mode=indexing
                      n1258 = Enqueue Element(queue=w3996, element=w3994) -> (queue out=w3995:refnum<queue>)  [unwired: 2 in, 2 out]
                    }
                  }
                }
                n1259 = Select(t=State_Type_Definitions,_for_0.26g_versions_and_later_3."True Stop" ("Enum"), s=w3976, f=State_Type_Definitions,_for_0.26g_versions_and_later_3."Task 9A: Raise Arm") -> (s? t:f=w3978:T18)
                n1260 = Select(t=w3978, s=w3975, f=State_Type_Definitions,_for_0.26g_versions_and_later_3."Task A10: ROTATE TO ANGLE" ("Enum")) -> (s? t:f=w3984:T18)
              }
              frame "Exit" {
                n1261 = for {
                  shift-right: [w4003] -> w3999
                  shift-left: w4000 -> [w4004]
                  tunnel: string[] ["STOP", "RESET ENCODERS", "RESET YAW", ""] -> [w4002] mode=indexing
                  n1262 = Enqueue Element(queue=w4004, element=w4002) -> (queue out=w4003:refnum<queue>)  [unwired: 2 in, 2 out]
                }
              }
            }
          }
          frame "Task A11: ARM DROP HEIGHT" {
            # ">>> Motor control cluster >>>"
            # ">>> yStepper command>>>"
            # ">> Manual override >>"
            n1263 = Dequeue Element(queue=w4015, timeout in ms (-1)=w4014, error in (no error)=w4016) -> (element=w4013:T10)  [unwired: 3 out]
            n1264 = Equal?(x=w4012, y=u8 133) -> (x = y?=w4010:bool)
            n1265 = case shown="\"Start Task 1\", Default" w4013 {
              tunnel: [w4026 State_Type_Definitions,_for_0.26g_versions_and_later_3."True Stop" ("Enum")] -> w4017
              tunnel: [w4029 w4046] -> w4018
              tunnel: [State_Type_Definitions,_for_0.26g_versions_and_later_3."Idle" ("Enum") State_Type_Definitions,_for_0.26g_versions_and_later_3."Shutdown" ("Enum")] -> w4019
              tunnel: w4010 -> [w4025 _]
              tunnel: w4009 -> [w4024 _]
              tunnel: w4008 -> [w4020 w4043]
              frame "Start Task 1", Default {
                # "Stays in Task 5_A until stepper reaches desired \nheight"
                # "T: Go back to idle, F: Continue with task\""
                # ">> Manual override >>"
                n1266 = case shown="False" w4025 {
                  tunnel: [w4033 w4039] -> w4029
                  tunnel: w4020 -> [w4031 w4037]
                  frame False {
                    n1267 = for {
                      tunnel: string[] ["Z STEPPER DROP HEIGHT", "READ STEPPER VALUES", "READ IR"] ("element") -> [w4034] mode=indexing
                      shift-right: [w4036] -> w4033
                      shift-left: w4031 -> [w4035]
                      n1268 = Enqueue Element(queue=w4035, element=w4034) -> (queue out=w4036:refnum<queue>)  [unwired: 2 in, 2 out]
                    }
                  }
                  frame True {
                    n1269 = for {
                      shift-right: [w4041] -> w4039
                      shift-left: w4037 -> [w4042]
                      tunnel: string[] ["RESET YAW", "RESET ENCODERS", "READ IR", "SET TIMER 1"] -> [w4040] mode=indexing
                      n1270 = Enqueue Element(queue=w4042, element=w4040) -> (queue out=w4041:refnum<queue>)  [unwired: 2 in, 2 out]
                    }
                  }
                }
                n1271 = Or(x=w4025, y=w4024) -> (x .or. y?=w4027:bool)
                n1272 = Select(t=State_Type_Definitions,_for_0.26g_versions_and_later_3."True Stop" ("Enum"), s=w4024, f=State_Type_Definitions,_for_0.26g_versions_and_later_3."Task A12: EXTEND ARM" ("Enum")) -> (s? t:f=w4021:T18)
                n1273 = Select(t=w4021, s=w4027, f=State_Type_Definitions,_for_0.26g_versions_and_later_3."Task A11: ARM DROP HEIGHT" ("Enum")) -> (s? t:f=w4026:T18)
              }
              frame "Exit" {
                n1274 = for {
                  shift-right: [w4049] -> w4046
                  shift-left: w4043 -> [w4050]
                  tunnel: string[] ["STOP", "RESET ENCODERS", "RESET YAW", "ARDUINO MODE 0"] -> [w4048] mode=indexing
                  n1275 = Enqueue Element(queue=w4050, element=w4048) -> (queue out=w4049:refnum<queue>)  [unwired: 2 in, 2 out]
                }
              }
            }
          }
          frame "Task A12: EXTEND ARM" {
            # ">>> yStepper command>>>"
            n1276 = To Unsigned Byte Integer(number=u8 40) -> (unsigned 8bit integer=w4055:u8)
            n1277 = Dequeue Element(queue=w4063, timeout in ms (-1)=w4064, error in (no error)=w4065) -> (element=w4067:T10)  [unwired: 3 out]
            n1278 = Equal?(x=w4056, y=w4055) -> (x = y?=w4054:bool)
            n1279 = case shown="\"Start Task 1\", Default" w4067 {
              tunnel: [w4074 State_Type_Definitions,_for_0.26g_versions_and_later_3."True Stop" ("Enum")] -> w4061
              tunnel: [w4077 w4094] -> w4059
              tunnel: [State_Type_Definitions,_for_0.26g_versions_and_later_3."Idle" ("Enum") State_Type_Definitions,_for_0.26g_versions_and_later_3."Shutdown" ("Enum")] -> w4060
              tunnel: w4066 -> [w4068 _]
              tunnel: w4062 -> [w4070 w4091]
              tunnel: w4054 -> [w4069 _]
              frame "Start Task 1", Default {
                # ">> T: Breaks out of state loop; F: Stays in loop>>"
                # ">> Manual override >>"
                # ">> Checks if time is up>>"
                # "Stays in Task 5D until the object is detected"
                # "T: Go back to idle, F: Continue with task\""
                # ">> Manual override >>"
                n1280 = case shown="False" w4069 {
                  tunnel: [w4081 w4087] -> w4077
                  tunnel: w4070 -> [w4079 w4085]
                  frame False {
                    n1281 = for {
                      tunnel: string[] ["READ STEPPER VALUES", "Y STEPPER CONTROL", ""] ("element") -> [w4082] mode=indexing
                      shift-right: [w4084] -> w4081
                      shift-left: w4079 -> [w4083]
                      n1282 = Enqueue Element(queue=w4083, element=w4082) -> (queue out=w4084:refnum<queue>)  [unwired: 2 in, 2 out]
                    }
                  }
                  frame True {
                    n1283 = for {
                      shift-right: [w4089] -> w4087
                      shift-left: w4085 -> [w4090]
                      tunnel: string[] ["DISPOSE BUFFERS", "READ STEPPER VALUES", ""] -> [w4088] mode=indexing
                      n1284 = Enqueue Element(queue=w4090, element=w4088) -> (queue out=w4089:refnum<queue>)  [unwired: 2 in, 2 out]
                    }
                  }
                }
                n1285 = Or(x=w4069, y=w4068) -> (x .or. y?=w4075:bool)
                n1286 = Select(t=State_Type_Definitions,_for_0.26g_versions_and_later_3."True Stop" ("Enum"), s=w4068, f=State_Type_Definitions,_for_0.26g_versions_and_later_3."Task A12: DROP" ("Enum")) -> (s? t:f=w4071:T18)
                n1287 = Select(t=w4071, s=w4075, f=State_Type_Definitions,_for_0.26g_versions_and_later_3."Task A12: EXTEND ARM" ("Enum")) -> (s? t:f=w4074:T18)
              }
              frame "Exit" {
                n1288 = for {
                  shift-right: [w4097] -> w4094
                  shift-left: w4091 -> [w4098]
                  tunnel: string[] ["STOP", "RESET ENCODERS", "RESET YAW", "ARDUINO MODE 0"] -> [w4096] mode=indexing
                  n1289 = Enqueue Element(queue=w4098, element=w4096) -> (queue out=w4097:refnum<queue>)  [unwired: 2 in, 2 out]
                }
              }
            }
            n1290 = Bundle By Name(cluster=w4058, "yStepper desired"=w4055) -> (w4057:T21)
          }
          frame "Task A12: DROP" {
            # ">>> yStepper command>>>"
            # ">> Manual override >>"
            n1291 = Dequeue Element(queue=w4109, timeout in ms (-1)=w4108, error in (no error)=w4107) -> (element=w4106:T10)  [unwired: 3 out]
            n1292 = case shown="\"Start Task 1\", Default" w4106 {
              tunnel: [w4118 State_Type_Definitions,_for_0.26g_versions_and_later_3."True Stop" ("Enum")] -> w4111
              tunnel: [w4121 w4138] -> w4104
              tunnel: [State_Type_Definitions,_for_0.26g_versions_and_later_3."Idle" ("Enum") State_Type_Definitions,_for_0.26g_versions_and_later_3."Shutdown" ("Enum")] -> w4103
              tunnel: w4105 -> [w4112 _]
              tunnel: w4110 -> [w4117 w4135]
              tunnel: w4101 -> [w4116 _]
              frame "Start Task 1", Default {
                # ">> Is time up? >>"
                # "Determines if object is in range to pick up"
                # ">> Manual override >>"
                n1293 = case shown="False" w4116 {
                  tunnel: [w4125 w4131] -> w4121
                  tunnel: w4117 -> [w4123 w4129]
                  frame False {
                    n1294 = for {
                      tunnel: string[] ["OPEN CLAW", "START TIMER"] ("element") -> [w4126] mode=indexing
                      shift-right: [w4128] -> w4125
                      shift-left: w4123 -> [w4127]
                      n1295 = Enqueue Element(queue=w4127, element=w4126) -> (queue out=w4128:refnum<queue>)  [unwired: 2 in, 2 out]
                    }
                  }
                  frame True {
                    n1296 = for {
                      shift-right: [w4133] -> w4131
                      shift-left: w4129 -> [w4134]
                      tunnel: string[] ["RESET YAW", "RESET ENCODERS", "RESET FLAGS"] -> [w4132] mode=indexing
                      n1297 = Enqueue Element(queue=w4134, element=w4132) -> (queue out=w4133:refnum<queue>)  [unwired: 2 in, 2 out]
                    }
                  }
                }
                n1298 = Or(x=w4116, y=w4112) -> (x .or. y?=w4119:bool)
                n1299 = Select(t=State_Type_Definitions,_for_0.26g_versions_and_later_3."True Stop" ("Enum"), s=w4112, f=State_Type_Definitions,_for_0.26g_versions_and_later_3."True Stop" ("Enum")) -> (s? t:f=w4114:T18)
                n1300 = Select(t=w4114, s=w4119, f=State_Type_Definitions,_for_0.26g_versions_and_later_3."Task A12: DROP" ("Enum")) -> (s? t:f=w4118:T18)
              }
              frame "Exit" {
                n1301 = for {
                  shift-right: [w4141] -> w4138
                  shift-left: w4135 -> [w4142]
                  tunnel: string[] ["STOP", "RESET ENCODERS", "RESET YAW", "ARDUINO MODE 0"] -> [w4140] mode=indexing
                  n1302 = Enqueue Element(queue=w4142, element=w4140) -> (queue out=w4141:refnum<queue>)  [unwired: 2 in, 2 out]
                }
              }
            }
          }
        }
        "Object Detection" <- w331
        "Ultrasonic sensors" <- w354
        "Encoder values" <- w343
        "Stepper position values" <- w327
        "NAVX Values" <- w325
        "IR Sensors" <- w317
        "Line sensors" <- w312
        "Time cluster" <- w323
        "Box Colour Detection" <- w305
      }
    }
    "Object recognition mode" <- w230
    "Front Ultrasonic obstruct" <- w227
    "Front IR obstruct" <- w226
    "Table IR obstruct" <- w225
    "Same colour?" <- w218
    n1303 = local write "Green LED"(w240) -> ()
  }
  n1304 = while {
    tunnel: w49 -> [w5107]
    tunnel: w48 -> [w5104]
    stop <- w5101 stop-if-true
    # "Status Loop for Action Queues"
    n1305 = Get Queue Status(queue=w5107, return elements? (F)=TRUE) -> (error out=w5103:errorcluster, # elements in queue=→"Action Queue Items":i32, elements=→"Action Queues items":string[])  [unwired: 1 in, 5 out]
    n1306 = Get Queue Status(queue=w5104, return elements? (F)=TRUE) -> (# pending remove=→"State Logic Queue Items":i32, error out=w5102:errorcluster, elements=→"elements":T10[])  [unwired: 1 in, 5 out]
    n1307 = Merge Errors(w5103, w5102) -> (w5101:errorcluster)
    n1308 = Wait (ms)(milliseconds to wait=u32 500) -> ()  [unwired: 1 out]
  }
  n1309 = call <vilib>:"DIO Close.vi"("error in (no error)"=w25, "DIO Info In"=w28) -> ()  [unwired: 9 in, 1 out]
  n1310 = call <vilib>:"DIO Close.vi"("error in (no error)"=w35, "DIO Info In"=w37) -> ()  [unwired: 9 in, 1 out]
  n1311 = call <vilib>:"NavX Close.vi"("error in (no error)"=w12, "NavX Info In"=w11) -> ()  [unwired: 9 in, 1 out]
  n1312 = call <vilib>:"DIO Close.vi"("error in (no error)"=w30, "DIO Info In"=w32) -> ()  [unwired: 9 in, 1 out]
  n1313 = call <vilib>:"DIO Close.vi"("error in (no error)"=w19, "DIO Info In"=w20) -> ()  [unwired: 9 in, 1 out]
  n1314 = call <vilib>:"DIO Close.vi"("error in (no error)"=w14, "DIO Info In"=w15) -> ()  [unwired: 9 in, 1 out]
  n1315 = Merge Errors "Merge Errors"(w65, w64) -> (w47:errorcluster)
  n1316 = Merge Errors(w51, w47) -> (w46:errorcluster)
  n1317 = Destroy User Event(user event=w69, error in=w46) -> ()  [unwired: 1 out]
  n1318 = Release Queue(queue=w42, error in (no error)=w46) -> (error out=→"Queue Errors":errorcluster)  [unwired: 1 in, 2 out]
  n1319 = Release Queue(queue=w59, error in (no error)=w46) -> ()  [unwired: 1 in, 3 out]
  n1320 = Destroy User Event(user event=w68, error in=w46) -> ()  [unwired: 1 out]
  n1321 = Unregister For Events(event registration refnum=w60, error in=w46) -> ()  [unwired: 1 out]
